vi "UHR-Fleezers Control (host) - 10.8MV_trial3.vi"() -> ()   [LabVIEW 2012]
uses:
  <vilib>/Utility/miscctls.llb/LVPoint32TypeDef.ctl
  <vilib>/Utility/miscctls.llb/LVMinMaxIncTypeDef.ctl
  <vilib>/userdefined/High Color/nirio_resource_hc.ctl
  <vilib>/Platform/TimedLoop/XDataNode/timing_clust.ctl
  <vilib>/Platform/TimedLoop/XDataNode/nitl_modes.ctl
  <vilib>/Platform/TimedLoop/XDataNode/wakeup.ctl
  <vilib>/FPGAPlugInAG/PCIe-7852R/niLvFpga_Open_PCIe-7852R.vi
  <vilib>/FPGAPlugInAG/PCIe-7852R/niLvFpga_Reset_PCIe-7852R.vi
  <vilib>/Utility/error.llb/Error Cluster From Error Code.vi
  <vilib>/rvi/errors/niLvFpgaAdjustHostInterfaceError.vi
  <vilib>/FPGAPlugInAG/PCIe-7852R/niLvFpga_Run_PCIe-7852R.vi
  <vilib>/Analysis/baseanly.llb/Mean (DBL).vi
  <vilib>/express/express analysis/Spectral/Block/exnSpectralBlock spectral measurements PSD poly.vi
  <vilib>/express/express analysis/Spectral/Block/exnSpectralBlock spectral measurements PSD WFM.vi
  <vilib>/Waveform/WDTOps.llb/WDT Append Waveforms DBL.vi
  <vilib>/FPGAPlugInAG/PCIe-7852R/niLvFpga_Abort_PCIe-7852R.vi
  <vilib>/FPGAPlugInAG/PCIe-7852R/niLvFpga_Close_PCIe-7852R.vi
  openfpgaref.8.6.ctl
  <vilib>/Platform/TimedLoop/XDataNode/XDataNode.xnode
  <vilib>/rvi/interface/nirviOpenFPGA/nirviOpenFPGA.xnode
  FPGA Bitfiles/UHR-FleezersInst_FPGATarget_UHR-FleezersCont_0F5B06C4.lvbitx
  UHR-Fleezers Control (fpga) - 10.3.vi
  <vilib>/rvi/interface/nirviMethod/nirviMethod.xnode
  <vilib>/rvi/interface/nirviReadWriteControl/nirviReadWriteControl.xnode
  <vilib>/express/express analysis/Spectral/XNode/ExpressSpectralMeasurementsBlockNode.xnode
  <vilib>/rvi/interface/nirviCloseFPGA/nirviCloseFPGA.xnode
  <vilib>/Analysis/NI_AALBase.lvlib
  <vilib>/Platform/TimedLoop/XDataNode/XDNodeRunTimeDep.lvlib
  <vilib>/vision/NI_Vision_Development_Module.lvlib
  NiFpgaLv.dll
  <vilib>/FPGAPlugInAG/PCIe-7852R/niLvFpga_ConfigureFifo_PCIe-7852R.vi
  <vilib>/rvi/errors/niLvFpgaMergeErrorWithErrorCode.vi
  <vilib>/FPGAPlugInAG/PCIe-7852R/niLvFpga_ReadFifo_PCIe-7852R.vi
panel:
  out "Location path":path=path "D:/UnifiedHighRes_VIs/Locations.txt"
  out "Location Matrix":string[][](array[string])=[["N.D.\r\n", "N.D.\r\n", "N.D.\r\n"], ["0.19233\r\n", "0.00156\r\n", "0.20615\r\n"], ["N.D.\r\n", "N.D.\r\n", "N.D.\r\n"], ["N.D.\r\n", "N.D.\r\n", "N.D.\r\n"]]
  in  "radius":i32=10 min=1 max=20
  in  "clear markers":bool
  in  "trap\nmarkers?":bool
  in  "Sample Channel Flow":bool
  in  "Pump 3 contents":string="Bottom: ADig beads" caption="contents"
  in  "Pump 1 contents":string="Top: DNA beads" caption="contents"
  in  "Scripts":T1(tab)
  in  "Take Stepping Data":bool
  in  "Got DNA bead":bool
  in  "Got ADig bead":bool
  in  "Cap 1 Flow ON":bool=TRUE
  in  "Move Cap. 1 (DNA Top)":bool
  in  "Cal/Data Acq. Spot":bool
  in  "Dump Beads":bool
  in  "Cap 1 T ON":bool=TRUE
  in  "Cap 1 Samp Flow ON":bool=TRUE
  in  "Offset 2 Set":dbl=2.0
  in  "Offset 1 Set":dbl=1.0
  in  "Cal @ (MHz)":dbl=20.0
  in  "W/ Offset 1":bool=TRUE
  in  "Offset 1 Start (MHz)":dbl=13.0
  in  "W/ Offset 2":bool
  in  "Offset 2 Start (MHz)":dbl=16.0
  in  "Pause at Closest Delta (s)":dbl
  in  "Move to Delta 2 (MHz)":dbl=41.0
  in  "Attempt Limit":dbl=30.0 caption="Limit"
  out "Attempts":dbl=1.0
  in  "Wait Before Save (s)":u32=1
  in  "Fish for Tether":bool
  in  "Closest Delta (MHz)":dbl=13.0 step=0.25
  in  "Stop F (pN)":dbl=10.0
  in  "Then...":string(combo)="2"
  in  "Move to Delta 1 (MHz)":dbl=15.0
  in  "Tether Alarm?":bool=TRUE
  out "Tether":bool
  in  "TA Cancel Save?":bool=TRUE
  in  "TA Green Off?":bool=TRUE
  in  "Raster Set Upon Tether":u32=1
  in  "Save at end (5, 6)":bool
  in  "N Steps":dbl=20.0
  in  "Step Size (nm)":dbl=0.34
  in  "Save ave factor":dbl=1.0
  in  "Dip Trap Delta 1 (MHz)":dbl=15.0
  in  "Move Trap Before?":bool
  in  "Save Data After?":bool
  in  "Green ON After?":bool
  in  "Dip Trap Delta 2 (MHz)":dbl=15.0
  in  "Move Trap After?":bool
  in  "Duration (s)":dbl=1.0
  in  "Dip for Protein":bool
  in  "APD to Watch":bool
  out "Duration (s)":dbl
  in  "Action":string(combo)="Yank"
  in  "Fl. Triggered...":bool
  in  "Fl. Delta Thresh. (kHz)":dbl=0.6
  out "Waiting":bool
  out "Fl. High":bool
  in  "N pts to average":u16=6
  in  "Yank Delay (s)":dbl=3.5
  in  "Yank to Delta Array (MHz)":dbl[](array[numeric])=[16.3, 15.85, 14.85]
  in  "N Array El":u8=3 min=1 step=1
  in  "Random Choice":bool=TRUE
  in  "Force Yank":bool
  in  "Force Reset":bool
  in  "Y change (mm)":dbl
  in  "Profile":bool
  out "Sigma/Mean 2":dbl=nan caption="Sigma/Mean" format="%#_2g"
  out "Rate sigma (Hz) 2":dbl caption="Sigma (Hz)" format="%0.2f"
  out "APD 2 Rate (Hz)":dbl format="%#_3p"
  out "Primary Video Display":T2(plugin-control)
  out "Waveform Graph":dbl[](graph) caption="APD Line Scan"
  in  "Inject Top":bool caption="Inject Pump 3"
  in  "Inject Bottom":bool caption="Inject Pump 1"
  out "Messages":string="7:59 AM\tUHR-Fleezers ready.\r"
  in  "APD Ave N":dbl=10.0
  out "Int. Time (s)":dbl=3.0
  in  "Stop All":bool=TRUE
  out "Sigma/Mean":dbl=nan format="%#_2g"
  out "Rate sigma (Hz)":dbl caption="Sigma (Hz)" format="%0.2f"
  in  "Tab Control 6":T3(tab)=enum."Imaging"
  in  "APD 2 Offset":dbl
  in  "APD 1 Offset":dbl
  out "RMS (Ang)":dbl=nan format="%_2g"
  in  "Bead Sep. Int. Time (s)":dbl=5.0 caption="Int. Time (s)"
  in  "Below (kHz)":dbl=0.5
  in  "Above (kHz)":dbl=2.0
  in  "Adjust Scale\nto Mean":bool
  in  "Rescale on Mean":bool
  in  "Offset (nm)":dbl
  out "Mean":dbl=nan caption="Mean (pN)" format="%#_3g"
  out "Force":waveform(dbl)[](graph)=[{"t0"=timestamp(12.90000000000001 s since 1904-01-01), "dt"=0.15, "Y"=[nan, nan], "attributes"=variant("NI_ChannelName"=variant(string "T1 X"))}, {"t0"=timestamp(12.90000000000001 s since 1904-01-01), "dt"=0.15, "Y"=[nan, nan], "attributes"=variant("NI_ChannelName"=variant(string "T2 X"))}]
  out "APD Chart":waveform(dbl)[](graph)=[{"t0"=timestamp(12.90000000000001 s since 1904-01-01), "dt"=0.02, "Y"=[0.0, 0.0, 0.0, 0.0, 0.0, 0.0, 0.0, 0.0, 0.0, 0.0, 0.0, 0.0, 0.0, 0.0, 0.0], "attributes"=variant("NI_ChannelName"=variant(string "APD 1"))}, {"t0"=timestamp(12.90000000000001 s since 1904-01-01), "dt"=0.02, "Y"=[0.0, 0.0, 0.0, 0.0, 0.0, 0.0, 0.0, 0.0, 0.0, 0.0, 0.0, 0.0, 0.0, 0.0, 0.0], "attributes"=variant("NI_ChannelName"=variant(string "APD 2"))}]
  in  "Calibration":u16(ring) items=["None", "Position", "Force"]
  out "T1 X":dbl=nan caption="T1 X (pN)" format="%0.2f"
  out "T2 X":dbl=nan caption="T2 X (pN)" format="%0.2f"
  out "Bead Separation":waveform(dbl)(graph)={"t0"=timestamp(12.90000000000001 s since 1904-01-01), "dt"=0.15, "Y"=[nan, nan], "attributes"=variant("NI_ChannelName"=variant(string "T1 X"))}
  in  "Amplitude (nm)":dbl=3.0
  out "Bead Mean (nm)":dbl=nan caption="Mean (nm)" format="%0.2f"
  out "Difference":dbl=nan caption="Difference (pN)" format="%.2g"
  in  "Take Detection Laser\nImage":bool
  out "APD 2":T2(plugin-control) caption="APD 2 (Cy5)"
  in  "Flip Green Filter":bool
  in  "Set X Only":bool
  in  "Set Y Only":bool
  out "APD 1":T2(plugin-control) caption="APD 1 (Cy3)"
  out "Detection Laser Y":T2(plugin-control)
  out "Pointer Y (V)":dbl format="%_3g"
  out "Pointer X (V)":dbl format="%_3g"
  in  "Set Confocal Spot (X-Y)":bool
  out "Detection Laser X":T2(plugin-control)
  out "Saved APD":dbl[][](graph) caption="Most Recent Time Trace"
  out "Trap Delta Graph":dbl[](graph) caption="Most Recent Time Trace"
  out "Save APD Deriv":dbl[][](graph) caption="Most Recent Time Trace"
  out "Delta Fl. 1":dbl
  out "Delta Fl. 2":dbl
  out "All Signals":waveform(dbl)[](graph)=[{"t0"=timestamp(12.90000000000001 s since 1904-01-01), "dt"=0.02, "Y"=[0.0, 0.0, 0.0, 0.0, 0.0, 0.0, 0.0, 0.0, 0.0, 0.0, 0.0, 0.0, 0.0, 0.0, 0.0], "attributes"=variant("NI_ChannelName"=variant(string "APD 1"))}, {"t0"=timestamp(12.90000000000001 s since 1904-01-01), "dt"=0.02, "Y"=[0.0, 0.0, 0.0, 0.0, 0.0, 0.0, 0.0, 0.0, 0.0, 0.0, 0.0, 0.0, 0.0, 0.0, 0.0], "attributes"=variant("NI_ChannelName"=variant(string "APD 2"))}, {"t0"=timestamp(12.90000000000001 s since 1904-01-01), "dt"=0.15, "Y"=[nan, nan], "attributes"=variant("NI_ChannelName"=variant(string "T1 Y"))}, {"t0"=timestamp(12.90000000000001 s since 1904-01-01), "dt"=0.15, "Y"=[nan, nan], "attributes"=variant("NI_ChannelName"=variant(string "T1 X"))}, {"t0"=timestamp(12.90000000000001 s since 1904-01-01), "dt"=0.15, "Y"=[-0.0004235663930173644, -0.0004722739341410556], "attributes"=variant("NI_ChannelName"=variant(string "T1 Sum"))}, {"t0"=timestamp(12.90000000000001 s since 1904-01-01), "dt"=0.15, "Y"=[nan, nan], "attributes"=variant("NI_ChannelName"=variant(string "T2 Y"))}, {"t0"=timestamp(12.90000000000001 s since 1904-01-01), "dt"=0.15, "Y"=[nan, nan], "attributes"=variant("NI_ChannelName"=variant(string "T2 X"))}, {"t0"=timestamp(12.90000000000001 s since 1904-01-01), "dt"=0.15, "Y"=[-0.0005883053071687949, -0.0006281319620349712], "attributes"=variant("NI_ChannelName"=variant(string "T2 Sum"))}, {"t0"=timestamp(12.90000000000001 s since 1904-01-01), "dt"=0.15, "Y"=[nan, nan], "attributes"=variant("NI_ChannelName"=variant(string "T1 FB X"))}, {"t0"=timestamp(12.90000000000001 s since 1904-01-01), "dt"=0.15, "Y"=[-0.0004680013428144157, -0.0005167699209570592], "attributes"=variant("NI_ChannelName"=variant(string "T2 FB Sum"))}, {"t0"=timestamp(12.90000000000001 s since 1904-01-01), "dt"=0.15, "Y"=[nan, nan], "attributes"=variant("NI_ChannelName"=variant(string "T2 FB X"))}, {"t0"=timestamp(12.90000000000001 s since 1904-01-01), "dt"=0.15, "Y"=[-0.0006226691488387671, -0.0006504715109714008], "attributes"=variant("NI_ChannelName"=variant(string "T2 FB Sum"))}, {"t0"=timestamp(12.90000000000001 s since 1904-01-01), "dt"=0.15, "Y"=[-0.0007901852473525123, -0.0008601641895809732], "attributes"=variant("NI_ChannelName"=variant(string "PSD Y"))}, {"t0"=timestamp(12.90000000000001 s since 1904-01-01), "dt"=0.15, "Y"=[0.00031556138798181086, 0.0002525101474044007], "attributes"=variant("NI_ChannelName"=variant(string "PSD X"))}, {"t0"=timestamp(12.90000000000001 s since 1904-01-01), "dt"=0.15, "Y"=[-0.00019678334910122974, -0.0002453993346964931], "attributes"=variant("NI_ChannelName"=variant(string "PSD Sum"))}]
  in  "Signals to Plot":i32(listbox)
  out "Trap Disp. Freq. (Hz)":dbl=6.666666666666667 caption="Freq. (Hz)" format="%#_6p"
  out "Display Period (s)":dbl=0.15 caption="Period (s)" format="%#_6p"
  in  "Trap Disp. Downsample":dbl=10000.0 caption="Downsample" max=20000.0
  in  "APD Disp. Scale":dbl=0.1 caption="Scale (Divide,\nfor above plot only)"
  in  "APD Disp. Downsample":dbl=2.0 caption="Integrate" min=1.0 max=30.0 step=1.0
  out "APD Display Freq. (Hz)":dbl=50.0 caption="Freq. (Hz)"
  out "APD Display Period (s)":dbl=0.02 caption="Period (s)"
  out "FFT 1":cluster{"f0":dbl, "df":dbl, "magnitude":dbl[]}[](graph)=[{"f0"=0.0, "df"=16.666666666666668, "magnitude"=[-331.1367572010275, -79.05506245821404, -86.61411242440559, -88.4728176091699, -90.3181253945935, -94.12566333707997, -92.52740723119955, -94.92192587982518, -99.60936585245742, -96.87568627870715, -94.02570383337763, -83.8058550151726, -97.57441397235512, -101.59968530846606, -101.523049255742, -103.35038532190343, -101.58594091014982, -102.96098031851216, -91.39759462745924, -103.75019963279499, -104.45030075054324, -103.04245334279298, -104.0720279134107, -106.06482372394834, -103.69131867828104, -104.40395035115309, -105.96420043276396, -107.6735556337804, -106.673030006608, -107.34889066208132, -108.05626565233933, -106.25659018850432, -105.29934513380842, -105.43096056709592, -108.3728498841465, -106.0555440144992, -105.78001282181421, -107.48741857324953, -108.67624970548897, -105.39976667156175, -105.91413119232612, -109.4222808198164, -107.0898971593174, -107.91164191890915, -108.26032038855709, -107.58332347164534, -108.23559688234297, -108.01271040303237, -107.66511723652701, -106.51901583170391, -109.27249501469946, -108.55647681594805, -107.93499259231463, -107.05068166453935, -109.13641475410455, -109.29679733781423, -108.19360835527803, -109.57747591546632, -109.58364591011674, -110.47061433372711, -109.8144340420426, -108.79067462293897, -107.54887553357234, -107.99559866705923, -108.85023923652685, -109.68733225238618, -108.51101278437793, -108.51620475114115, -108.22212402200637, -104.63726950302143, -110.2989919678048, -107.61796444414897, -108.68882962798736, -104.79193983043893, -103.59504263746938, -93.64633660288543, -101.9191640501395, -105.73717393151816, -108.92572458793902, -107.43962662800902, -107.79595323081325, -107.0923101993207, -108.17603277205289, -107.87074270713183, -109.20899066381877, -108.61832060412445, -109.10072003106593, -105.76480632823524, -108.60877649218978, -109.67541158970121, -110.2286232768028, -109.84952155309578, -109.33772024076384, -109.95251642394683, -110.14777282585466, -109.13825677905699, -110.05989365698167, -109.39359990189426, -110.56255614635295, -109.66477183197163, -108.9397158528824, -110.26529907650465, -109.20049464984628, -108.20183857013548, -109.09752250184418, -108.00440442238454, -108.35465963524055, -111.16774134451799, -110.34812550238405, -108.94506763426756, -108.72845542102493, -109.41512344014713, -112.44661664432377, -110.35437330889101, -111.32939440655925, -109.42989530434981, -110.98084669076195, -111.92160561143541, -108.57755551751093, -111.40042616180912, -110.15284955891853, -112.21455132279115, -111.40787773511747, -108.82949641635288, -110.13442122547907, -111.42229298204664, -112.06314940885191, -110.6015308813694, -109.51144097251623, -111.15989713761475, -110.25535755335385, -109.65868178057926, -110.51649885452997, -109.77194745285269, -108.4234206864394, -109.50892632093968, -109.46471287444389, -107.92241289271415, -109.72283805386196, -108.63426821579918, -110.37316681536255, -111.09713996884652, -110.32903619589223, -105.32012665515045, -107.36858557554393, -108.00382215905725, -110.06430686942338, -108.81666625979916, -110.01277074453823, -110.94194741225512, -109.65934609082873, -107.80979136006962, -112.81333866824724, -111.61474300955487, -109.83998277184975, -109.45953946904639, -109.79640584952526, -108.19172301667324, -109.28894656674316, -107.61471301278785, -108.83814006090513, -109.08866847726084, -108.20250571862371, -107.96222236861584, -107.03811197900873, -108.93533000393974, -107.74482548035408, -110.79811544577694, -111.1387476496877, -107.42970105883512, -109.18442281176472, -108.73546184641192, -108.71800246690864, -108.51945944378063, -108.06825856571285, -107.27210712368412, -108.12304695877637, -107.84933283677306, -109.73682373154998, -109.32284761503395, -109.31328817453769, -106.68762108642842, -109.79203616876461, -109.9020278896408, -110.27080024357275, -108.54152101558762, -111.00464391726017, -112.42244020766577, -110.82707315747889, -111.00344011890857, -109.90461839395674, -109.42877207451863, -109.73549298167016, -111.67494793393293, -108.85799077901427, -108.5348443278263, -109.803781083881, -108.30644755543659, -108.5079527456017, -111.2055351312823, -108.53089994340155, -108.01739789012176, -108.70360662855235, -107.95873456794631, -109.58297170693093, -108.9372401694271, -110.15921663527153, -109.22399119911955, -110.89883651739237, -108.92840112258382, -110.0545300523626, -109.05961065387005, -109.45831398589371, -108.61239387653227, -110.13001256174265, -108.80060224137931, -109.46327400696283, -108.0177965824709, -109.29727944627197, -110.3237255895986, -109.03258262543821, -110.97880178489321, -109.70034895077919, -111.16405638194153, -109.17324451464711, -109.65698250854277, -108.96750235822178, -112.00534231585624, -108.69274607723942, -108.98110446396657, -108.40723795464795, -111.44459094807324, -111.74799245277113, -111.1601960491512, -108.92048232753773, -110.30506377784799, -111.33145973979093, -110.91850998672503, -110.33684985776448, -108.90206518366908, -109.28458878227542, -108.98773986023751, -110.85813863075646, -109.00041591105906, -110.84543686681204, -109.84382395806176, -109.69722434763266, -108.50915601095721, -107.80829925826895, -110.59736107582401, -109.75377770317087, -109.3992084496136, -110.51151565846742, -112.49753959826434, -109.7299632589479, -109.54070743868353, -109.90314341132164, -111.05974202976806, -109.03766862152392, -109.46667095459878, -109.52800799036197, -111.3163121356807, -110.07817134522178, -108.69251657453547, -109.40472158898045, -109.71400709815576, -110.60534468715097, -109.46937396724682, -107.70342491418788, -109.86331122597839, -108.64971387994616, -110.90117371097081, -108.34928840565928, -110.04172889660904, -111.52979926554961, -110.34759300823305, -109.62712781837159, -109.24131154553284, -110.23196152450447, -108.68509612326807, -108.0246905483419, -106.61876139289784, -101.5519630114271, -80.57695480953835, -102.03744443354402, -107.1449217193017, -110.0695213407169, -106.61597783999268, -110.79221011808191, -109.58974545931426, -109.1149802216988, -109.20993813088597, -109.63768480465863, -110.10428394219181, -109.08445084271477, -108.83472375362581, -109.69508502050168, -108.05588796178941, -110.62586360101581, -109.95315261676905, -107.52208264977473, -108.80708007514875, -110.43484881098874, -110.45942171588936, -107.83804717866751, -109.98973910294193, -109.3496496054193, -108.425252911127, -110.94579264380809, -108.54181722177951, -108.67696070083541, -108.4150202151644, -109.24973583101504, -112.0454922608961, -111.29046597340738, -110.75018248960077, -109.38326363603683, -109.2033340336957, -109.45076170874889, -109.52878049853727, -109.32340869724774, -110.98123395128233, -110.75736340635505, -109.7218385823809, -107.97422606064993, -109.77313701758703, -110.95948744392717, -110.08996774172691, -108.51011830110778, -109.78063140243836, -110.65996628628228, -109.83684298615616, -110.33329049188029, -110.13755118968292, -110.3717925645783, -108.55302219178951, -106.86811628734195, -108.6302156589162, -108.75341391045045, -108.32589578384841, -108.70061474734084, -112.30742263527534, -109.16842570592085, -109.29767035534508, -108.87829025017463, -108.2255616391397, -108.4316108616088, -108.82995906929271, -110.40135575415563, -109.51623498946435, -109.79409808792403, -107.03832759632121, -108.36534528684132, -109.72010868372905, -107.90933028179892, -106.95643597294047, -111.29929166165778, -110.23001135794706, -108.98838015381585, -109.79115357104436, -108.18627479511115, -108.14988122174307, -109.12074063466532, -109.41904850488358, -111.40409873721113, -108.83156790193294, -108.77032248953847, -108.88363158686694, -108.47515048290681, -105.94172147874599, -109.38146940214403, -109.21277078848794, -108.11309390545507, -110.70840012427504, -109.5504457849329, -109.52330684534209, -110.06776026911132, -108.21949434182314, -111.21266686269992, -108.78581501170974, -108.43115799297222, -109.63260325780062, -109.84070220619535, -109.72041980780126, -110.29615941882527, -110.60316734262464, -108.79165446414692, -110.95840439895592, -109.64926233107009, -109.16526769544322, -108.65292362430982, -109.56113898129935, -109.85693046339026, -108.92316027325207, -109.79492493553914, -109.38157962945887, -110.24545136266825, -109.30031463492487, -109.0795429936869, -111.4091719525013, -108.63499083917162, -108.43863465339358, -109.23207864880891, -111.21947487191643, -109.24525201480154, -109.56842406077318, -109.46711940800672, -111.91389548262572, -108.15655736690546, -108.71882059966947, -111.26328503478568, -110.95027143873176, -108.4853106242357, -110.36902802777546, -109.9314203579182, -108.77686164101732, -108.71871020068312, -111.04829661168574, -109.95072655339462, -109.88221342875462, -109.53241732756136, -108.2625005404823, -108.00677030040697, -110.19659317581693, -108.93858924796267, -109.46817875483995, -110.78063992017232, -111.11066570318451, -110.78774336696706, -109.19199744617812, -108.54914256407436, -109.28414960420909, -110.64143585101183, -110.5855350821307, -109.47578632252726, -108.89705360836223, -109.89214013612292, -107.93271261027171, -109.32631601340563, -108.60274611341092, -109.40110159872573, -110.889237682208, -110.01391165813328, -109.99747108785071, -108.65542819213674, -110.37211847668736, -110.44656500845738, -110.8128133834973, -108.8909299260433, -110.19551227077532, -111.37647266643523, -110.83802189730321, -109.98519377913681, -110.52378970770522, -108.16970420057817, -110.70974729773344, -110.76836765494402, -110.26884275594577, -109.22041044268806, -109.87809744746195, -107.76823252107832, -109.12119474042969, -110.28066108731146, -108.55000033509207, -110.18152097767907, -110.73030521152278, -111.49470908029893, -110.2320929919509, -110.03370979233021, -109.79181668155233, -108.6673501209991, -109.86695766650877, -107.88926518046961, -110.95525003776572, -109.18130359755742, -110.42618009658618, -107.90341931158893, -111.44736855661769, -110.72634267386593, -109.29945988519303, -107.67889101961411, -108.81148059987765, -109.13375212757057, -109.8122873383549, -109.80176697684155, -109.96342275204768, -109.90406635707086, -108.75674342748256, -110.12362902701081, -109.82151095527837, -108.62543344241836, -110.09171852771195, -110.21434637862887, -109.97254504855631, -109.27043209093468, -111.35149588204125, -110.12399876776051, -111.65983675538546, -109.28788875768564, -110.86554069990251, -111.26990906470603, -108.60956517491746, -111.49613890850938, -111.79685722966795, -109.26269485364045, -110.38555615546439, -109.40641023162068, -110.966136593156, -108.78892524584494, -110.29340727375603, -111.44032043281035, -109.95212021173755, -109.79233511584334, -112.41184021118175, -109.73687851881148, -108.65493879781806, -110.76132988919045, -108.43230346094671, -110.32968175895853, -110.29890782023821, -108.77609076424456, -110.3298662333555, -109.47734504217333, -108.2677295732245, -109.21234363352882, -107.83278941978479, -108.85136784424789, -108.43241251530755, -109.76609391460555, -108.53204373005357, -110.9660641972934, -110.3152512161094, -110.72570499399905, -109.23877906286317, -111.72407743101837, -109.20311421918561, -108.06021800233717, -109.29288625761943, -108.78395253409145, -111.85250172876302, -108.78827588901797, -109.79775055719482, -109.12089297455859, -109.49896359356035, -110.34432647103819, -107.94700097960238, -109.30489238477631, -108.89170290869342, -108.82574563272509, -110.11024077194833, -107.37946433552314, -109.60167933458756, -107.80625057819019, -110.11489057210264, -107.35436859378505, -105.69819484613895, -109.11280625683739, -109.27770293057978, -107.7053735252589, -109.75022444894368, -109.3310543596577, -107.87683693707739, -108.19931495338068, -109.26462246191564, -106.71885779297867, -100.00018022217961, -92.54434511397295, -107.20472143807373, -107.39203415155283, -110.04461177268398, -108.48860496315312, -109.0057168110333, -108.37627790492552, -108.4108380728248, -109.65509454313073, -109.64243000632982, -97.04219069306761, -109.0928856629964, -107.9760697315632, -107.52611064047497, -108.87702814778996, -109.08437599027614, -110.70097118837974, -109.00969860961283, -110.38275386163214, -110.0699155421545, -106.91498895181175, -106.22178738309017, -109.36827866896039, -107.59953130968307, -109.19516217272808, -108.31502495393616, -109.384158926223, -107.11670654202719, -108.09436312738853, -110.14559230873704, -109.84997663447679, -107.83465335309926, -108.60947100624459, -108.9932479423645, -109.17174810371898, -108.79457339828916, -109.40909327982367, -109.6328723628302, -109.51081854476179, -107.63054408568418, -109.63728404010122, -108.51163794839918, -107.55002282725216, -108.97796212764939, -107.24648164623483, -112.21470452291085, -108.74294024554423, -109.62070777514892, -108.05768666239368, -109.8224946685739, -109.34575507446003, -108.53536952609525, -109.60789300457671, -107.56681538208278, -109.22777325016398, -108.79047910308894, -110.10332477250668, -108.00206387955672, -108.45604004720035, -109.00645795765472, -109.81039564269616, -108.92785144634745, -108.3978471520567, -107.94411095685999, -110.53486519304262, -108.8773780319227, -109.03345093296107, -107.30746693745031, -108.54277704832029, -108.77629108166091, -108.91111762599647, -107.74965195880401, -109.97375370738439, -109.76326492689246, -107.91717581777407, -109.0730556927617, -107.66804873204664, -110.40438871064791, -108.05794247751498, -108.80206615156494, -107.51329354700796, -108.83687012994949, -107.57713176895379, -107.94774159581414, -109.41894615439651, -107.10869425078764, -110.51480854078629, -108.92221367099775, -109.91358786461535, -110.1744263092835, -109.30795472883494, -107.91359710691006, -109.77888185049835, -109.52060975706438, -108.66686651982212, -108.71041801553639, -110.13619546359467, -108.87957097273856, -109.72150387215271, -109.00776068810654, -109.70251113927438, -110.75769213896399, -108.53234896741436, -109.69439526582246, -110.15412541604617, -108.25183374628219, -107.97402569656481, -110.34920156998648, -108.45106995186384, -108.82031145748209, -111.38690005057539, -107.01968459818563, -110.3044500039584, -110.8755481852125, -111.08915057663255, -107.94824988655199, -110.21669144934839, -109.90539774633154, -109.58985438756767, -110.12258796623348, -109.41689951612143, -109.31128210476795, -109.00258476567323, -109.11093063041056, -108.83347064311234, -108.32685287566952, -109.44770946560935, -108.40145063144861, -109.68448193892085, -108.76525439243828, -107.62837139034596, -107.39300298848994, -109.36993934990318, -109.2465218489418, -106.66307369796812, -110.15891092764934, -109.57151745419041, -108.92425698310808, -109.8036704717834, -108.79751146756549, -109.25926431818017, -108.46260574057584, -109.1967554647261, -110.63319560262356, -109.02343067385144, -111.22073171487528, -109.4731095097105, -109.69335000085164, -109.48782989577005, -107.95204227683271, -108.19468255763758, -111.36195112053247, -109.55696116543685, -110.3130767640534, -108.9621824253354, -109.99735074896789, -109.20198058456344, -108.12100614259485, -111.27227490807289, -110.09248554008288, -109.14395535060149, -110.80882692379708, -109.22632926901655, -108.64497210802793, -111.00030482190711, -111.1317849358033, -107.43140429257826, -107.9783302193555, -109.2639893652291, -108.97008485446163, -108.66556668859064, -108.12995785876932, -109.73001061107855, -108.09691302413727, -110.68391499215569, -112.78583642012705, -108.7093037763389, -110.67868795924797, -109.0190959349128, -108.36247198231372, -109.82829353258869, -108.24916379311045, -109.84154533905823, -108.55470160833775, -109.75438989348815, -108.82865632118325, -107.63622268162582, -111.00943492886312, -110.81824358463759, -109.46028423652966, -107.52479398900992, -108.99087806823736, -109.94494831750349, -110.26788355564504, -109.8954055022304, -106.9478122391182, -108.91705388158901, -107.76095584490312, -109.28456723055147, -109.7982307261767, -108.98552661346622, -109.98937979783426, -110.57907422426224, -108.68113463944836, -108.06257240208589, -110.0707224529617, -109.19515280354733, -109.35868842818849, -110.37311467065695, -109.0404734478992, -108.16686395270187, -108.61859220485148, -109.19986437876149, -108.19707189725302, -110.06564239663074, -108.87850403465154, -110.63824157544798, -107.36918104067212, -108.7008736325543, -110.9359398265406, -111.08529123080929, -108.44209934821818, -109.79529621208783, -108.38917887958179, -108.169117639508, -109.24332926356216, -110.50584058811704, -109.63592524002665, -109.32261039377495, -109.16720880524552, -109.3084314664462, -109.5812223978583, -107.70213196487856, -108.0557884982431, -110.67058020007828, -111.68459781023608, -109.66270627185824, -110.52536245663693, -109.70208409132103, -108.78645420809342, -109.23122088059863, -109.24601474121832, -111.25604763816514, -109.50225851581177, -107.32434217163818, -109.28548556764925, -107.59972621660836, -110.46928774723048, -109.25950101547609, -110.32016453935465, -107.78482761561703, -107.89462895091089, -107.51366154391481, -108.08036891159172, -109.53371809947035, -101.2452927166745, -109.32763325689056, -107.52166868423687, -109.89648659445174, -109.11350200980485, -109.81336712738089, -110.02799517445062, -108.02767143538516, -107.97850220501483, -109.50772934896838, -109.31069875721964, -108.49991657749598, -105.60880911233095, -109.79128597340213, -106.91084537903113, -107.84880087118997, -109.63628170511824, -109.03203967193224, -110.64186113413658, -110.98027990365594, -112.33841002907062, -111.01793075565425, -108.58025797022215, -110.4259296883756, -110.38643255981424, -108.93051671115133, -110.97544177116494, -108.63883100482677, -108.37581711765226, -108.90240163126536, -107.94688047875466, -109.9482937437732, -110.09097112364414, -110.09805032265376, -111.44307114024532, -109.15483789122554, -110.9713708217832, -107.8548737634672, -111.41418477109195, -109.45699779859628, -97.03595099331734, -109.16746744169623, -109.66209204485918, -112.57048704774604, -109.73989735035725, -108.16252575067017, -110.7546980664636, -108.91536673403449, -109.20509151422344, -111.0260632167785, -109.62924582406518, -110.45466277291722, -110.2973970018937, -109.67550222925419, -108.84481022020094, -107.23686414357573, -111.79004633370906, -109.85453094194085, -109.45617270081004, -110.73920606732504, -108.90879956851099, -109.67774425528265, -109.4745715721361, -110.18080454693559, -109.26079184315502, -109.41692499885505, -109.02240975088358, -107.80833423058168, -109.32657361431549, -107.87138278655101, -110.910364670719, -109.70067156846706, -108.55301754282077, -109.4243252157005, -109.77567725161107, -107.83737232063925, -110.36509412773016, -109.6371048811367, -109.49430894422814, -108.55509251499753, -108.03996302911446, -110.4385715838736, -110.08864436068788, -109.48922484379962, -109.90865554258562, -109.7491963238264, -110.04796094537969, -107.413043439116, -108.54229076126079, -108.2522516728666, -109.75464941327974, -110.26795832300996, -109.28073673851144, -108.62990200974927, -109.89408067552287, -109.09160284731726, -109.90740624925795, -109.92534708896517, -109.79578862362752, -109.97278346890566, -107.80679350393824, -112.81728446281548, -108.09689504419987, -109.89549991422173, -108.43930976031248, -109.95153099843282, -108.18277483720716, -111.89607792605433, -109.52567003805, -109.17125106979698, -109.64300739407085, -108.21045178846524, -109.64036472149706, -109.02324448538845, -109.039163008889, -110.41006510134076, -109.50289952116489, -110.4732620447796, -110.08777181504614, -110.15589511434341, -109.55705089158471, -109.2547682932589, -110.86823885471617, -109.96330502176939, -109.85995369810554, -110.63211290903473, -112.08007783432191, -110.24725218052279, -107.62861148917592, -110.08691795849435, -108.89793794632287, -111.07702220466341, -109.46946126482341, -109.19747345337464, -110.70018609416007, -109.66366205691908, -110.78032312133551, -108.05724200456513, -108.195661625627, -110.90724508408255, -110.08307674771669, -110.76863516643007, -110.46620425061583, -109.16986788877276, -109.61921294239114, -108.51159432329543, -109.96308336765689, -107.38178944242856, -111.95930944846394, -109.3329826827624, -109.59119636368249, -108.83148571828912, -110.46194288788257, -105.87694286145472, -107.985886302892, -109.2975019660806, -111.05138725716857, -109.60005889204612, -110.92871351729086, -110.73480546964537, -108.41587420326718, -109.84275465824477, -108.8249071047676, -107.65358887817105, -108.3254150042995, -111.47362100321767, -112.7287536850025, -108.8217125660507, -109.50232320231771, -110.29587061625348, -109.30644535112089, -107.69178032077258, -110.84522325672016, -109.3735891463141, -109.12506388923123, -109.65582307934665, -111.11427272192576, -112.19827973435466, -109.11306367925813, -108.19203577968261, -107.89831568266465, -108.85805249169313, -109.51100049661844, -111.71546684086955, -109.53880495724334, -107.07739286222231, -110.66836728754211, -111.5415170557177, -110.16051267940297, -110.6107546662698, -111.36389129556191, -107.77888179117923, -110.34160392509817, -109.61287125994414, -110.23791773883013, -111.00669159903549, -110.97165069538953, -109.43965413392434, -110.6813161690388, -110.31441293654314, -111.96129906273796, -108.15998218707462, -110.08095912053633, -109.41084567452768, -109.28774416263552, -110.80159950384204, -110.41956747809755, -108.85005186267244, -107.9069227847757, -108.84249369063123, -109.92569208845894, -109.34109797584448, -109.41334788055491, -108.76462023086997, -108.22069272136177, -107.0786679601274, -108.30206755098202, -108.57613406368954, -110.83330887636482, -111.93966942736989, -109.76373713473264, -108.25782074884941, -108.16490627215555, -109.93351470267982, -110.75525684428368, -108.22814762283093, -109.73442331991602, -107.53145627482685, -108.27195221226805, -110.33032779278457, -109.48951857415828, -108.12599093700939, -107.97627415508097, -108.81426859968796, -111.21764717894752, -109.80856212352333, -110.92658779118501, -109.71551885834796, -110.38682741010847, -108.87671328341361, -109.68368600774755, -108.35359806351899, -111.7519400010676, -109.89407081573103, -108.24301180922755, -110.00646944788126, -108.6685299083706, -107.52856885980722, -111.7622363038509, -111.0025144494897, -108.64719599357296, -110.62968467177518, -108.821509935539, -107.94915453463719, -111.53070432277694, -109.87282048586256, -110.71167589371663, -109.79225006081626, -109.96203471712074, -110.29921092232489, -110.10644439440416, -111.28815007382043, -111.19165661703703, -108.46024117100558, -110.22528296512183, -110.32184972386672, -110.05120383416072, -109.78792549362107, -109.00355659956696, -108.85989369286315, -113.00899556732638, -110.91756826567867, -111.25016866167897, -111.84225040552181, -110.54451635944174, -110.72722829912917, -109.60759702177283, -110.49362602516815, -108.74419542915284, -110.3379671069179, -109.66259088220754, -110.45956400953156, -109.13956157147233, -109.27130155486806, -110.83015602667983, -109.17970724944131, -109.09662765889193, -108.0447366108107, -108.9536269357457, -110.35663108940085, -108.73418835472056, -113.42965806805827, -111.81270536656905, -110.06155590173537, -108.76582224646269, -106.7488061675813, -108.5700320158723, -111.11038264410035, -110.41435767488723, -109.12763443489911, -109.30517580756394, -111.61251165371237, -109.8116632664339, -109.36845864976851, -109.00390009629231, -110.54359197165573, -109.52629258465976, -110.75932197632896, -109.50903215359567, -107.42652056246085, -107.81146496533543, -103.22224383145215, -108.53803076819163, -109.78623360072066, -109.66306634612869, -110.80245829141279, -111.87835085452016, -102.27372781471168, -111.27763038431458, -108.45838423437681, -108.79077917058028, -109.31951755762685, -110.05415097017186, -109.5535934823387, -111.62732254641111, -110.73478247119641, -109.9468722686683, -110.39698367573979, -109.30612942398305, -109.7578384694043, -109.34817295524313, -105.56944757301993, -110.1940418750125, -109.27076023513962, -111.03491935225027, -112.2980497521063, -110.65725497955563, -109.0567530102422, -110.31700596563523, -109.64508026365678, -109.6190471404421, -110.52566833759428, -109.68595899227789, -109.7431160985074, -110.4798230300751, -109.45506977604765, -110.69504157940786, -110.63067849573177, -108.06456949500138, -107.99354148885966, -108.11349194720599, -109.15944121207349, -110.61766925164031, -110.14145801314527, -110.67420842201165, -111.91532881806512, -112.15901550030345, -109.94774413630104, -109.2819568305201, -110.94623189179737, -110.17685430287735, -110.39082916961016, -109.53953238698966, -110.76940623620611, -109.89327922318515, -109.10275695043765, -110.21445972656734, -110.58968777252528, -110.57016757660259, -109.59208496373341, -109.07946946465374, -109.10762003745964, -110.36892993974607, -109.81864495218393, -112.12972189864566, -109.26185849434863, -111.56305819991357, -111.36019621828058, -110.3397604159226, -109.58675612753163, -110.58041217474447, -106.34739062044932, -108.6722699609389, -110.03906060709869, -109.16794717548382, -109.65012481802809, -109.35377624077988, -110.51889143862303, -110.03397458059777, -110.7981307056636, -110.56653507062292, -107.61367005067231, -109.99279736988825, -111.79875182878175, -108.60382315996031, -109.71381533228038, -108.60388131505613, -107.0933685540362, -107.86037690830757, -108.40980028847238, -108.83869602763895, -110.76921375395764, -109.96766364716046, -110.8256171465781, -110.13805084291067, -108.5349140035878, -110.57158437465219, -110.8920694413417, -108.71646695477324, -108.33274238445665, -108.96152108305608, -111.03750932994224, -109.48915027983756, -110.29725207211165, -110.79527247268442, -109.47969936716117, -109.79306701834035, -110.16840035577498, -110.29840230783668, -109.15306387075587, -110.72651274964761, -109.08881658764956, -110.8349724030761, -110.64653625576447, -111.40392562616867, -109.94581588927414, -108.85136340231294, -109.77228546607624, -111.48297395390018, -109.7334001251941, -109.30537415590783, -109.63937411233408, -109.69785848648013, -109.3523781030017, -112.04667421182404, -111.56311816195343, -108.18548447362308, -110.63388993686104, -111.39768634137992, -109.87157345395542, -108.6734208287271, -109.46213300216168, -111.75774769437145, -110.10245994173216, -109.52385139033495, -110.96513097775451, -111.8709319163154, -111.54948269614047, -110.29760900080463, -108.52168175904663, -111.09033925738258, -111.14752744054172, -108.83074523709202, -109.05704141259113, -111.74377805749482, -109.57200906899736, -108.84121318623825, -110.86657990204343, -109.54363603755047, -110.89448416316372, -109.58965570570145, -110.21012263847972, -110.4063470702923, -109.5021950342969, -110.33648801598177, -110.90551031296536, -109.69205870504638, -109.8648503154861, -110.28183391384131, -109.65970942950766, -108.43615680946908, -111.11790511866548, -110.89043476451553, -113.64898442872548, -113.08004494963895, -110.81525412051718, -113.91009875719509, -110.95802128672312, -110.40944585634135, -110.33464695414992, -109.98984645778987, -110.18795067005652, -110.62364351231234, -110.44029833291248, -109.01598585569788, -110.95430216511514, -109.77987141110621, -108.54452361812068, -111.41780266439777, -110.47172771858405, -109.06084635984516, -109.30794593246578, -108.8764083815745, -108.18222749506985, -110.31330487887435, -109.04176821738014, -108.8558386035048, -109.47888284507395, -110.01459604573937, -110.48596659065309, -112.6781342298378, -109.85522803775775, -109.0569534499285, -109.08991286548698, -110.89485727880403, -109.18715778948663, -111.50381433568144, -111.3545424730884, -110.07710926239977, -111.99977850157067, -109.47444853853723, -109.81605328527645, -110.74995213151195, -112.56834665925544, -108.52052472391404, -110.89121213995557, -112.02004142355113, -108.66413739656008, -111.10053848695652, -110.41241079991636, -111.80152991764473, -110.21746151515111, -110.63265128607344, -109.483042128511, -112.78639954059729, -109.47114195846122, -109.23309637902875, -108.97133643967169, -110.08909147812822, -111.01105271457081, -111.18602432128249, -110.04633990216801, -109.53453538673071, -108.81939452082017, -111.13486114285661, -111.65877073200598, -111.63763706753498, -112.14107810664572, -113.6231865196724, -109.31743865878806, -109.18551713085722, -108.74951309653638, -109.28206426212142, -112.36687029711229, -110.10933061193728, -111.29501093502684, -108.19021080564794, -109.34497312126749, -110.37228033937312, -108.63277512903049, -110.61033993911002, -111.2975761598062, -111.49780004751436, -109.91019436685814, -109.32789992989028, -111.4482538110117, -110.1538439123475, -110.66347034043578, -110.05055133068794, -108.53002033538341, -111.7522199783972, -113.49108651193104, -108.03793940563418, -110.07108694011555, -110.83958739865201, -109.62805629409038, -112.69637731014087, -109.57996950503268, -110.104850643722, -108.83376203949506, -108.69400304840181, -110.59434352922563, -110.69121011800921, -110.18694553784364, -111.90598571547098, -110.30230802494223, -109.66810649416752, -112.6017099000434, -111.00296745333219, -110.64462650261785, -111.4775358707403, -111.98753241268494, -112.26574909791167, -112.04796822399412, -110.65853064447325, -109.6623218025264, -109.40559579075378, -110.42174451813142, -109.18991987957241, -111.02050178263048, -112.77950487440032, -110.42443751566815, -111.35440372400903, -108.5263524245987, -105.07498063939795, -107.15444425741984, -110.4508720018025, -110.25163264819463, -111.1383261104107, -109.91171620173931, -110.52200560606038, -110.5299174299573, -109.34628087255733, -110.26101817411786, -109.65071853372183, -109.66953335961068, -110.83590602054682, -110.980546313788, -109.4110066989163, -111.47223607390256, -110.00281523859483, -109.4088722967626, -109.00401922839337, -109.59655302543185, -109.7359970854586, -111.46016206343049, -110.23478747568004, -109.29441275295858, -109.82941912510167, -110.43088525283673, -108.21649744751299, -108.70220592702613, -105.2334473604296, -110.60620657984927, -107.97533820921146, -110.7664079806058, -110.56406610911355, -111.76465470250328, -108.84172809688911, -111.03661078143631, -109.85351980370237, -110.70091167176791, -109.52380717508088, -108.4356492672842, -112.25498760397127, -110.69648730540193, -110.36748838594507, -109.99090797924349, -111.2678642544111, -110.42541694325627, -111.4575545259775, -109.3211175669008, -112.7465573314208, -109.56208667784249, -111.59733497772172, -109.42295730962105, -108.55804089331346, -108.71397903286748, -110.09188290952392, -108.90810063278326, -110.31333217069538, -109.69794714542728, -109.06210020835357, -112.42465112160288, -111.74630553904855, -109.99304310093493, -108.93867687355595, -113.1669287525049, -109.09193568851137, -109.27500368450697, -108.99643325722404, -110.53962759110647, -111.2052088429852, -110.05855563908841, -110.30763723153481, -110.03411001268613, -109.6161415052669, -110.6304714466923, -110.17116005754627, -109.0753171640551, -110.92564270851628, -109.60831770517053, -110.25913363817017, -107.76644895378317, -109.2619309023068, -107.64198246311884, -107.37056168314048, -107.31978563121643, -107.68171928702894, -104.57515288104209, -104.75187637758803, -105.27246893266054, -106.96524396060869, -105.93920355631757, -103.66449995825586, -104.08476660009461, -104.53081578265315, -103.0148493379086, -106.74751670818362, -104.92309629919443, -103.98320340724693, -104.81633219413234, -105.77996356028235, -107.12559309216644, -107.28196039053535, -108.84583578337953, -109.4494696919565, -109.15525441177898, -109.7634811359225, -110.79433338587495, -108.44440079452527, -108.79597700117748, -109.98590735173822, -110.72144284267539, -109.30550753718086, -109.70072152916897, -109.65801130162137, -109.65949265997646, -109.82238573025273, -110.30669821947491, -109.83394128869384, -108.90433312205332, -110.664046708231, -110.39926453734134, -110.37725911098757, -112.12508639032839, -110.26795666332589, -108.98741993218054, -107.76168841100478, -109.82334992872889, -110.83516363498563, -112.60649745671253, -111.1960726449926, -111.03919163866381, -112.05129034965563, -108.83187987662883, -109.57240688505179, -109.32857861150738, -109.54934849013647, -108.29359879300195, -111.5179112931669, -109.52702486426027, -109.95429980789645, -110.7011078611564, -109.43204524997455, -105.56031249677113, -107.70609254346495, -108.78303653454363, -108.11457060956113, -110.44215460317537, -110.78267897406572, -110.33119812901934, -109.34449539666907, -108.82636558484161, -107.1834151347969, -108.83808254322192, -108.2542825327446, -108.80298057862501, -107.59922121598055, -108.9131916496929, -109.51519107961856, -107.7704986323755, -108.79678029009878, -111.13791068210752, -110.402746275919, -111.31702623823912, -108.49812727557243, -110.63723264798182, -109.32890666586829, -110.29721723278237, -111.66560929315017, -111.04227698307153, -111.36927505376269, -112.5203298417673, -109.93967930487354, -110.14533835678606, -110.3868348991775, -110.85413569165249, -108.44519725537315, -107.93391978795047, -109.82778679299085, -109.79311153223738, -109.25261055399044, -111.47738679135526, -111.11775495397512, -108.65898844492045, -110.26505495390529, -111.02017977446526, -110.34817965403467, -107.55161094495372, -110.21667403085983, -112.43970497917284, -110.70535338255132, -110.79438078890512, -109.81809822502822, -108.99167960596515, -106.5556893069368, -97.51736665041192, -105.29926513345109, -108.72453297392224, -108.23203912463346, -109.50324111400698, -110.9939986929772, -108.05367524487318, -108.37339392211176, -109.8553291283933, -110.46179639493138, -112.48795697163695, -111.88145079973545, -110.8678969738583, -110.62677605624849, -111.83824818603244, -109.76798658735359, -109.6654742351465, -112.58543522753767, -110.3406716250781, -109.55013159400883, -108.00481229232405, -109.90793236599207, -111.28597960985334, -110.54144527494444, -110.14704702870655, -111.2652554338908, -110.97520848958668, -108.63647576273343, -110.52472680617548, -113.16137826273847, -109.62457037485827, -109.53869420402964, -110.71399284283449, -108.55435337782664, -108.09492728294455, -112.2373886856363, -110.3693019226993, -111.65116752865308, -111.3223986412311, -109.67734725401074, -111.36420709226297, -109.14293108556625, -110.5982939020188, -110.29596476096043, -112.69847120697035, -108.39052787054206, -109.06205229490357, -110.00045399262885, -110.71775009467346, -110.69530760167493, -112.54144940754935, -109.55755373438097, -107.88943697845929, -109.98578587243783, -110.14202980613851, -110.80051915904802, -109.11327182471621, -109.50637030500913, -109.77023677605327, -109.98552825925917, -110.40235854896, -109.37603004890141, -111.36989177909379, -110.8399811877331, -109.30394670937987, -112.2769814990538, -109.10893172594731, -109.17733972841754, -108.35968166480572, -112.64492569586005, -110.13779257328873, -110.64439690778532, -108.45446935516622, -108.97325006911116, -110.54637968933774, -110.66412364132371, -111.38627695224784, -109.8942998516069, -110.36392017322382, -109.92355133054227, -109.61886697310419, -109.71969465343778, -109.85627196259388, -112.1407808286419, -111.1013489416651, -110.70428953307596, -109.3454280179969, -110.22984684615578, -109.53826801613613, -107.83673208330934, -108.72742563398342, -109.5745872123195, -108.83031823548816, -110.89059911076627, -109.87842545384129, -109.21980161063786, -109.07140273870678, -109.04628915564135, -108.79255665097845, -105.20875397856382, -110.0838008881032, -109.68293832806683, -111.24644641302518, -110.01257579497496, -110.99281477454484, -108.99296184719546, -110.96495665514604, -110.70404386182749, -108.25078498739035, -100.77667501455139, -107.61479263900088, -110.06600976399395, -110.02035637581871, -111.45524052052504, -109.975541184397, -111.07333860975358, -108.4808974233161, -109.59513524582242, -110.74711589861774, -109.50005300854993, -105.23071652566294, -111.81094849223531, -109.0168079712372, -111.89029991620679, -109.90672274216391, -109.30959446424889, -108.23718655264584, -110.10868108588909, -109.21139771899594, -110.33333323577992, -110.25792318324204, -110.67825932924109, -112.33148517950511, -108.9724848367048, -110.78371843797613, -111.40913868573313, -110.2930522718577, -111.9538408094371, -108.63639312641844, -112.4462941079034, -110.40266356498321, -108.66617580940074, -109.44306834729083, -111.08962916641603, -110.52132608161017, -110.53757698855654, -111.5587344449704, -109.77722315102946, -110.40060629757771, -109.45395807961631, -108.77558572395142, -109.0151938598724, -109.80739619986889, -108.9332873172888, -112.49933978358132, -111.28667321897437, -110.40629082858706, -109.9829216820938, -108.85102919990373, -110.84179127037925, -110.27309817549309, -109.88857884367955, -112.24517967927224, -110.23377125710859, -111.26951227953063, -110.09782138347559, -109.77508406986834, -110.55359722398646, -110.09534729906368, -109.96333904888587, -110.29372855476366, -111.36651812163072, -109.97141184588116, -110.16701683369045, -112.8562627359291, -110.66651146857079, -108.78873821095968, -108.59208174618087, -110.31784275318834, -109.43177042415276, -112.80272887161644, -111.79874205007107, -111.08216899537892, -110.73699224045636, -111.04738767291953, -110.43395896705012, -111.62106163510778, -111.32599933330843, -110.29360981749807, -109.66562228449096, -109.21316193790335, -110.06363162177448, -110.54480468587292, -109.31791670875509, -112.65386492377107, -109.91857609999171, -110.57233605624137, -110.7597333064856, -111.49767138733276, -109.36548654843229, -112.34145274183716, -110.52831153822652, -111.55802243871352, -111.81399803046556, -110.17680125962372, -111.23811621944807, -110.48042049674514, -112.43786993562033, -109.56507357271987, -110.67030752598993, -110.86377249100713, -109.06001892813467, -111.37023727930494, -109.52881096984436, -112.95107295160436, -110.49467818026214, -109.29804210589607, -109.89270706931751, -109.46354468058833, -112.10350702955014, -111.06083529077077, -110.49996587015904, -111.1617248913634, -108.84725633199014, -111.42852695852422, -110.01433866707184, -109.11616968390972, -110.76961079765468, -111.80403513904453, -109.84442686379181, -109.65447921666167, -111.3378640555306, -110.8882647652338, -112.58014202075226, -109.67128881545659, -111.73429980763389, -110.82258070774773, -110.71895931098041, -112.5117489008152, -109.16182299471309, -109.71651258790612, -109.7770618808562, -111.94294809571427, -111.1629115541574, -109.57489224865171, -109.8402445779754, -111.17931450307283, -110.09045865447595, -109.23658206733491, -112.54929616847242, -110.5150381158864, -111.32296447909377, -111.64472156295191, -111.65832771066007, -111.03359562742956, -110.85303206770837, -110.80655337650862, -109.3712696310075, -110.57313454785879, -111.18525355670417, -111.67423695430561, -112.00829831274282, -111.08915434609605, -110.3298290221436, -108.68552957386795, -112.11377370993225, -110.80288297661977, -110.33640536217185, -109.5907971201988, -107.9195263775506, -108.50223113159429, -111.91191347156142, -110.29585599512956, -109.50902788911351, -110.76819145749467, -108.86899533416589, -112.09963049260891, -110.13374376572433, -110.15881393584463, -110.87392107947531, -109.18658540731009, -109.72734703956934, -110.18732487568724, -108.76554115185057, -109.94122289815374, -110.39583285609643, -111.09540935727229, -110.6618176357367, -111.6281345666718, -109.69686483639367, -110.31633402076315, -110.61246951748903, -111.73300235294965, -111.34221378834899, -109.46708370903485, -110.70412671997354, -110.7007891485379, -110.31685483435038, -111.03016917417074, -110.94517365625376, -109.46580797053619, -111.20935248224806, -109.20661126636224, -109.50147037097533, -110.14241781654353, -109.8510950344643, -111.3794198224028, -111.28966889207122, -110.43347441663424, -109.86759980279523, -111.92101892013198, -109.31594011390644, -112.92253433794441, -110.74000829597605, -110.3690783911604, -111.9386136764295, -111.04196305034188, -110.41800427558245, -110.94287511448232, -111.66035388807579, -107.53723747644062, -110.68014818358719, -111.86628806511304, -110.12097497430523, -109.69880468221378, -111.4312783987915, -109.18240866486639, -111.45649839248873, -110.1242345454651, -113.75911576151633, -112.71747598882953, -110.9614554157337, -110.92294419716129, -110.87229098694876, -111.09943759113875, -109.48107247947176, -108.62783006742795, -110.8108025857779, -111.63342408317932, -112.0221522906341, -109.96411229549527, -111.29821085030613, -110.04566676239914, -108.41674583097112, -107.50256474992416, -108.68086611003493, -110.3738906060137, -108.86763212826641, -109.81681043446049, -111.04539822346567, -111.73290882980949, -109.75238769150758, -110.55268275367449, -110.48423701377924, -112.1116140908134, -109.53952175199518, -108.538611608547, -111.3788321484912, -110.36378736224961, -110.37712171023523, -109.82150687920334, -109.17046632238393, -105.1169578108227, -110.84067642540583, -112.91626789016587, -111.32030958133453, -108.93375913686056, -112.44450956563915, -111.1596840012794, -110.17380444915341, -109.634859036508, -110.68819277718731, -110.0648098825346, -108.87385575091399, -111.99676414571755, -111.32585405719519, -110.59892045991457, -110.32589048340424, -111.1172696292077, -109.79946399891651, -110.10030723919304, -110.71841081343656, -112.23013150012054, -108.94400401141407, -109.71044551701596, -111.77560214164039, -109.68779520039777, -110.96119601299907, -113.66477058855787, -110.17794649102234, -110.30159876509862, -110.11953836266514]}, ...(2 in all)]
  out "FFT 2":cluster{"f0":dbl, "df":dbl, "magnitude":dbl[]}[](graph)=[{"f0"=0.0, "df"=16.666666666666668, "magnitude"=[-324.19011195451765, -78.1272953812706, -85.85545438627958, -89.30587144190069, -92.90590394398903, -93.63083388385274, -91.8644929119412, -95.26924857401164, -97.0710469181336, -98.01148078956652, -99.33043660296804, -95.58776817681839, -99.9570097527269, -101.45494093095093, -101.51838334751548, -101.00386616525799, -103.01963069818913, -103.20223925731209, -103.53783076500916, -103.48065647812659, -103.97797518531912, -104.58942778240602, -104.46991277190502, -104.59813972158683, -104.56685024229951, -104.69893799348945, -105.05669000016238, -106.17061117835001, -106.43303821862656, -107.39468286383597, -106.2899368267905, -105.7863846168199, -105.17170638885071, -104.53818172761852, -106.70340956723133, -106.55444321137247, -106.67654843051936, -107.79888413750199, -107.86424326005849, -106.09722609215336, -107.71648639013972, -107.79500725395155, -106.17330953637067, -105.43663624517525, -108.04970689199158, -109.92106271611999, -106.2505251183406, -110.60221373795562, -107.11377887451098, -108.4126937286195, -108.37794745021417, -113.22457316369011, -106.38281814065472, -107.55385617652075, -108.93026538982782, -106.19334142366085, -108.90462602264525, -107.63084712174981, -109.12192537022624, -107.90627042480016, -109.44472079190832, -108.91731458372392, -105.74102972706788, -105.74407510394178, -107.5989477192235, -106.2838630137392, -107.46190542725505, -107.38881299750702, -109.08024783239452, -104.97871836903269, -106.65424712290651, -107.04966019632134, -106.16202578092883, -102.98374199247179, -99.1568704142098, -87.07383781389657, -96.41471411313154, -102.65176579899618, -107.65674867775193, -102.85397890306213, -107.58658613411464, -104.79044898833125, -106.65282019869865, -108.65027966345534, -109.46169054950127, -108.69969979291741, -110.4048706652988, -108.81020193837274, -109.42808902484134, -108.85398463561398, -108.3849716744813, -109.1844457168716, -109.32787859535676, -111.01992124870878, -106.64843449415699, -108.9926343573667, -111.59837822080355, -110.57121677672183, -111.17280164669164, -110.68901970586144, -111.69013245592781, -109.90200577018311, -109.3554172126163, -110.7515368822992, -109.2863324212524, -109.66209701262974, -108.50795548698007, -110.58126481096504, -112.36093896766921, -109.78612141282203, -108.85120530917233, -109.91424431080952, -109.84698632196245, -110.93960894966105, -109.77214706089354, -110.30762971422381, -108.77791302937449, -110.79522659679036, -108.47242514643455, -111.20629758187835, -109.05996769621125, -111.13574821570619, -107.79388178889101, -111.5768481279296, -110.52058839597171, -111.58729762739313, -108.99000864386126, -111.6585121505227, -110.50715371958135, -108.87151956974363, -110.30486244367107, -108.32392040018144, -108.1769507919999, -110.43198471512189, -109.81454097966842, -110.26717009815644, -110.82924135076777, -110.34103661156989, -110.0692667126265, -109.34555682020833, -109.1694484721415, -109.9940980324044, -110.81940616215803, -108.21162003366862, -107.97087538330561, -107.55312461506225, -110.60339321606872, -110.09004629292225, -109.05860430198882, -113.1412749514818, -109.81628200948371, -108.62343219429849, -109.48172424209761, -110.85978755785311, -109.47778611557064, -108.81728552967951, -107.47864241666747, -107.61735128422292, -109.62511618983821, -110.32417726356636, -108.24287897478176, -108.60460879530194, -110.2181558494026, -107.95550802888957, -110.80234484950323, -111.09955733353904, -109.43923052503506, -108.98949130235951, -110.05778199870154, -110.36224432927585, -108.13523430027999, -110.681114579241, -110.49106131529867, -108.73493328004297, -110.07663907252234, -109.9968931372618, -112.10715231091008, -108.80994125105168, -111.63774865669372, -111.54355694032755, -111.64024217585788, -109.34986300492378, -108.88053713185408, -111.14370830146245, -111.17327416167232, -110.36311492990576, -109.99414559884396, -112.96912007380595, -111.43191437097785, -111.71327312809349, -108.77202323682606, -110.25970374932486, -112.59574277180732, -109.77247894866957, -110.09219852365874, -111.7197662726775, -109.85454092697009, -110.06789440397942, -110.38055758638309, -111.04251386932805, -111.54279434240568, -109.74385329575985, -110.98924544863415, -111.17898077762852, -110.98364252730245, -110.75024385843372, -109.24766708578407, -109.67753987004863, -110.6537235844391, -111.84436313010086, -109.12654337292446, -109.65519521121124, -111.1845162935778, -110.5009101465602, -110.22980642268818, -110.88540043278346, -110.29249073109453, -108.80459864528464, -107.49372141121728, -108.50353962704821, -110.00730069533373, -112.012876492648, -109.01283702976382, -109.07442203290057, -108.2961442983685, -111.60962842680907, -108.84312815413224, -108.6276642979969, -108.75132871638827, -109.30004903844721, -107.20359872252604, -109.12175943862074, -110.43914247337625, -109.55954680842791, -110.37116786618797, -108.55907813251434, -110.19249995041955, -106.95269845697632, -111.07027929458712, -110.1073996792702, -110.61729280468039, -109.6419175310234, -109.47995019876329, -109.66602827275211, -110.01953864498805, -108.45989120418268, -109.79778555296474, -109.94663827736616, -109.52410616839379, -110.58014441463794, -110.09182359045897, -111.0487262011397, -110.49609187214915, -110.6114701312941, -111.17752423063314, -109.74965389041003, -108.58973724447526, -108.84292130035902, -108.90689510645983, -110.69840140049361, -111.30494362640982, -111.00224390075273, -110.50848328538423, -111.59232911931113, -109.30826761863756, -108.44510893127558, -109.63744704504391, -108.95037574307332, -111.36486409910674, -112.74508631930381, -111.03952454593811, -110.57133212903979, -110.59969855145111, -108.25570461975128, -110.44617635200193, -110.32190307214704, -110.95204704643322, -112.0595421753479, -110.45342552693265, -112.50183987758867, -110.08217804938009, -108.90353583389084, -107.02032313792242, -88.3334978919524, -107.92027625495886, -109.83148570028482, -110.30427997450572, -110.92855407802753, -109.67404674397338, -111.03606345823586, -110.58277018943096, -109.77692362669393, -109.39170901729935, -110.20711662408928, -109.41601946806779, -110.34213214925832, -111.2283900972803, -111.51682597931386, -110.47069117801351, -110.93808974285523, -111.11277478000933, -112.50698886748012, -112.12918507523611, -110.46316790252011, -109.9387334819968, -109.78723249688426, -107.13037722044297, -108.16132376075751, -109.07255491017162, -108.85068428558272, -110.28038153100799, -107.77611023481016, -110.69754506886444, -110.09495581837979, -109.21214884561816, -112.62718526248648, -109.22048725312992, -109.17793923163308, -110.87372121410577, -109.71902632604333, -112.61041177225496, -109.6374750969677, -110.74738952366951, -108.93404661877067, -109.84938675700889, -112.25316361679832, -110.30788094875312, -109.26929069321925, -111.20853536783942, -110.05212566057608, -111.72448131932816, -111.55474439772887, -111.81988954424324, -108.44452452934028, -109.21897824914645, -109.55634869894358, -111.36318572800242, -110.05777399011298, -109.64458567712875, -108.73315084760529, -108.93332091319675, -108.4816455312154, -108.80120578498936, -108.1804470361839, -109.7177707524778, -109.31977709844544, -109.33603116022124, -111.46120546572519, -111.7480378245176, -109.17907150677627, -110.47970652472505, -109.73718750984082, -109.7935026884937, -110.40458408612054, -110.91781389491092, -108.39352075861481, -108.27512197925346, -109.59155075404814, -110.40183121737397, -109.25423373270381, -108.37769008625712, -107.91335995938509, -109.5576520703013, -107.27392145737491, -110.98592762117059, -108.41809950647861, -111.48163889400448, -109.70961684769624, -109.22952568656495, -109.76504719131209, -108.86928627177666, -107.97855299877004, -109.8412204399902, -109.6690048999326, -112.28329030175193, -111.54977099314607, -109.55689540119126, -107.93716711232997, -109.84247640855929, -111.5098351445789, -109.14317615215809, -110.28319116384824, -110.57901069942578, -107.2890252845352, -109.66754569546274, -110.15708115946433, -108.83782190109405, -111.60783857760667, -111.46884385151185, -109.21985333366634, -109.63605494317056, -110.87999187262697, -112.26992029775087, -111.05491095860552, -109.22795442529183, -108.99135781712076, -110.46475190704264, -109.35746113713218, -109.29125989270668, -107.40922407684049, -109.24391685563656, -110.41554602144217, -110.68952735085914, -110.62457364102458, -110.39856310555466, -108.84256124354566, -110.01614601335088, -109.8071306678428, -110.2804500736802, -108.76205061238203, -110.3962440297242, -108.98253716257014, -109.32990745926702, -111.17276766165281, -110.41113652364085, -110.36616199963426, -112.09767002991742, -108.43599666470733, -110.91876588140981, -109.05329272502944, -107.07198690769708, -108.72934463903034, -108.6666471996132, -108.97529973794413, -109.68895260146817, -109.2658844652487, -109.75690097249196, -109.38585024123027, -110.17593039468063, -107.87223111061134, -108.15261097418302, -110.09277437980633, -110.8665497655964, -108.43061614348413, -110.3052458526819, -109.22446919161898, -110.51909692711594, -110.06620699121913, -109.53439413051383, -110.31952463872884, -111.4732125902982, -110.41443606663168, -109.9579358088152, -109.930778061577, -108.5473214465574, -109.34719220288939, -109.16964653934396, -110.04824158176345, -109.42616539603762, -108.3556027482992, -110.62331917617789, -111.3652147859356, -110.12362012120938, -110.13175448595814, -111.20110099151856, -111.50643914621541, -108.11659117128028, -111.06037600347967, -109.03822892917451, -108.25678204604324, -110.82608024151122, -109.15887945314851, -109.88255674562845, -111.18322672526185, -110.95836040044516, -107.91535345885436, -110.66285812468733, -109.61906549925033, -109.58059721670746, -109.65198009505977, -109.65950565672951, -108.95264505276342, -109.23343669003113, -110.74308548011575, -106.39170014998685, -109.61471203101753, -108.24258770956924, -109.84609566640096, -107.83834185503922, -108.93052854090027, -107.55568820082641, -109.758551082242, -110.65892780872205, -111.99907420485852, -110.71043004141137, -110.62257237494617, -109.15610413532767, -106.87403836327807, -108.19175324576331, -110.27819583792918, -110.23918003777561, -108.29703377268754, -110.07182881114713, -109.60256111108491, -111.00394752430006, -110.30750337485472, -108.78309624082331, -109.24103013025798, -108.76979253891403, -109.91618737478264, -108.83915940855513, -110.92536150834754, -109.72250903746432, -108.96533939688658, -111.08949280651164, -109.20335070860871, -109.37826578362439, -109.77953166722301, -110.1867310744785, -110.07114559821346, -110.7003631567182, -107.86455899696074, -108.94113264174617, -109.35999427135138, -109.33627364788704, -108.96588828808375, -109.08716536982254, -108.73575375369026, -109.47770132070654, -109.83726171472907, -110.73516506891792, -110.56827134787686, -107.65667508354096, -109.30200115708924, -109.28406803847896, -110.55374624323233, -111.2017766725333, -108.50851279608973, -109.79494403619485, -109.08320018013063, -110.21850624918747, -108.4652936555984, -108.74837610538873, -108.81326140648238, -108.83830180036702, -108.785270477003, -110.01845876259073, -108.76030368637825, -108.57879884880157, -110.6610608456059, -108.74669367794318, -111.55956030460833, -110.22906685783455, -110.48411613865359, -109.48060880085136, -112.77556331479562, -108.2676071206087, -108.8571136162698, -108.56944905160177, -109.16406757131058, -111.42259299295839, -108.25216316582294, -110.48487127684025, -109.69532331373831, -108.13992755196784, -109.2987762526628, -109.82536192480795, -111.28650061088359, -109.12820736404241, -109.37960655471406, -108.96014976926716, -107.97535047619023, -112.31953123574708, -109.06198330523004, -107.52722515967098, -107.31555373665437, -99.89671790804692, -107.44442600896275, -110.6549218761941, -108.02265794322076, -109.63582761762919, -110.00574746987859, -109.51565124961209, -109.3550083591902, -110.4541529175301, -107.85799722437162, -105.1197113090786, -110.25038075579738, -110.39710812865657, -109.3618876098789, -107.6131301952152, -109.21529527621463, -108.7995754403799, -108.48347353145697, -106.45678488065816, -109.60427918561142, -110.81194387812535, -109.52215044127382, -109.88751598659705, -109.30205143590227, -110.74984456751768, -109.03952092986351, -110.69170786328897, -110.39236248162467, -108.65456161733339, -107.60439764386904, -109.97367926606955, -110.2754359970249, -108.81546418006434, -106.99691398176165, -108.42047325825182, -107.24499915944605, -109.28116135603187, -108.70650358781573, -108.05516916105047, -107.20893100196241, -112.07029265690055, -109.38099990478445, -111.53461820465232, -108.11312509555277, -108.76714028655223, -109.89565008459624, -107.71879172001115, -108.08434857420214, -108.79142773619792, -107.25153085963885, -110.05595039449301, -109.31604222314259, -109.94405791565286, -109.04715370361387, -108.89278831045846, -108.84682466376424, -110.0067927716526, -107.63768959294084, -108.98109382020348, -111.4720219575084, -110.76023788797733, -108.78599647633777, -106.59726674064618, -108.66715709719243, -107.99134359630926, -110.11396713841884, -107.21091759882775, -108.08576824949941, -108.80217666857972, -111.72949572713338, -107.33126296136014, -107.33731660097102, -108.04470462977443, -109.42963925921418, -111.03517778720736, -109.55293581015796, -107.99948151285162, -106.59480934999681, -107.63777243313498, -108.96490626068824, -108.8948210299064, -108.30870516747477, -109.13612869658097, -109.59971429402015, -110.2571461001396, -108.7655464686992, -109.81144209568883, -109.80796806645141, -109.20948481699544, -108.68653880881129, -109.26329796696166, -109.22428132233863, -110.12571678351438, -109.14615461144786, -107.08261621308327, -109.11338327144382, -107.75421565039201, -107.45291780756361, -109.00477000647248, -107.41031480478154, -109.98948062864928, -107.45953654921264, -106.37522884807879, -107.7786128523167, -108.03610987358499, -108.05926797128022, -108.59400205554164, -109.89620453365603, -109.03811240487515, -109.96909236705363, -109.28212981785472, -109.6772152101994, -108.26493868190678, -110.55558039199732, -106.6252818398841, -110.19075011176416, -109.56520012524705, -109.8023423576176, -111.2697570480663, -108.26752571816566, -112.00337375484828, -109.85709226796116, -109.36922081321148, -108.8424844298318, -111.2512302139209, -110.61775974680471, -110.22501328999012, -107.76874906708105, -110.71023653476604, -109.4025656165291, -107.66667684986125, -107.59759854092948, -107.94763263251238, -107.3888591871119, -108.62692803125044, -109.18012867988286, -107.78662871481455, -108.5072814073944, -109.50348958982907, -109.95177634938378, -107.78756251182895, -108.03865042797304, -110.1814993556385, -109.34937567548833, -109.52162025123161, -109.50819015441117, -108.20953105254624, -110.52154040214435, -109.3324404469266, -109.2696617050831, -109.54675609195674, -108.5940367000989, -109.40184828664549, -108.2518305610941, -108.55972691669434, -109.03647225394408, -108.48166656251695, -107.42023429066523, -109.42453054302521, -110.09532345960083, -108.78315822119662, -109.97508586102265, -108.22687406536997, -109.17110028890058, -110.15390449992647, -107.88577458651508, -108.28851074361447, -108.52030295163331, -110.03496861709483, -109.40014319167584, -107.73048113044877, -108.17571683963915, -110.34839852994926, -108.55894048192191, -108.74107339998285, -111.17734138993401, -110.22946440841412, -109.45511941802884, -108.0657300641843, -109.33797363184166, -106.95974095511333, -107.93068343723691, -109.78867669512647, -107.2087297624043, -109.542665021243, -110.05035859052961, -110.30235238883523, -109.20586170783808, -109.2796396673401, -109.14260673746566, -108.22019460542734, -109.99011886871159, -109.89103038547285, -110.36964772493243, -108.62340319923602, -109.06779821699769, -109.21830861066148, -107.7402395759509, -107.7178850938205, -113.45665085929117, -109.24039191621704, -109.30387033426037, -107.61849760982835, -109.41430582703529, -109.11482836392241, -111.89328423764577, -111.84653367963301, -109.00674896486915, -109.84488648739638, -109.41914760797953, -108.53442910169935, -109.66883322968232, -107.68762956301386, -109.82583101109167, -107.83405397804887, -108.78052031141966, -107.37842078941692, -105.40843158543845, -108.81430898189338, -109.57374640194516, -109.41111270322058, -108.82621700188898, -110.2552502368822, -110.23903890097205, -110.52171662278697, -108.21249857906324, -109.97268479379733, -108.20088823960992, -108.85682002802234, -110.11642849164285, -109.94087886999255, -111.63180946270296, -108.20899499456195, -106.73341567332112, -109.90003508676807, -110.14688274481229, -109.62259307329889, -107.57811196819495, -106.88584597822792, -109.16132624528932, -109.78677836397806, -108.59319344451784, -108.55877448618652, -109.46883711353044, -108.47309455543844, -108.09487065732198, -109.82219079158135, -109.63780237877428, -109.28348848877269, -107.62893405379826, -109.46986737961593, -108.03089712610223, -110.3931917410696, -106.06970126043262, -109.41866550703786, -105.31710372440419, -109.20218082282653, -108.28467118008108, -108.80026326744611, -107.40729224715713, -111.07322915141532, -107.1057186510818, -107.98286374205958, -108.51298722989311, -108.69632670891366, -107.96509231988331, -108.15882223414738, -106.85862416470376, -109.70705792539056, -108.64519930633055, -106.78708421443504, -109.43552377900174, -109.4474526498122, -109.10135248755788, -111.43316642580763, -109.33457343739448, -110.23547887071898, -108.95690647379442, -109.21159903769149, -108.12969562680841, -110.82751409340537, -108.55724349027832, -109.8796329603075, -108.50369978374582, -107.43145467247209, -108.60003323209516, -108.77155705999647, -109.33806063660796, -108.37500858898439, -109.65641721611547, -109.81905873737344, -108.03483220769625, -110.48028107566635, -108.60527372219985, -109.28768201151478, -99.8804125587218, -108.8913334544964, -108.23534920737794, -111.07646463287153, -108.59029790589766, -110.3405916586831, -107.66387718565608, -108.73793152614131, -110.61440166477816, -108.76211382544581, -110.23236978486065, -109.10669297094852, -109.15247609779597, -109.00539004923506, -110.14424353412238, -110.55445060661157, -109.48721312920799, -108.17040942305823, -108.77592227268228, -108.77130256578067, -107.82494496098512, -109.57266989523707, -108.75767497229612, -108.13688624150026, -107.8280716764963, -105.676279602552, -107.6370316684844, -109.73508547021689, -109.25365178573009, -108.86767843317584, -109.70969944273735, -108.91917504090888, -109.97734866522867, -112.17308993943783, -110.28356299479682, -110.7927103729386, -110.30837645846702, -107.56364161860179, -109.50188349731121, -109.36065627483853, -109.75389877587511, -109.81713476007774, -108.14524057525358, -109.43832376796216, -110.89342891210596, -108.15657882822792, -106.84106061627887, -107.83091759905821, -108.61794662682962, -109.57142366843581, -109.85402645528154, -110.12877022469837, -109.19414429724044, -110.56168468006764, -108.74720588273881, -107.90448559921305, -108.54421401507743, -105.06700039841249, -109.17937358052484, -108.94317576365822, -107.79410219455083, -109.24955437598658, -108.23334395173994, -108.98759227946937, -107.05986359444529, -107.20956512998849, -109.00295831471958, -109.43119556916457, -108.93348410522628, -108.99932477701081, -106.6448790859128, -109.06877251308666, -107.67053918439544, -109.15052780608639, -110.16878033319385, -106.55101141640301, -108.02811045752685, -111.52173447126572, -110.16854119242062, -110.93164036911654, -111.25979320890855, -108.82629030379024, -108.52004501839738, -107.09697056562636, -108.94233383169858, -107.37962568194772, -109.1239201710643, -108.93949898577122, -110.62573772949195, -110.09592372075662, -107.56136391005947, -110.45600430869621, -108.79481000016084, -109.41462449554598, -109.30248158488335, -108.70735295493108, -109.9174743694956, -109.94232543385962, -110.71725446170196, -110.0346196158573, -110.34814317845934, -110.6651078322521, -107.55409880424479, -108.71734776861287, -109.50902203986271, -110.40207542979611, -108.7847687630861, -111.10599488129682, -109.30824728923263, -108.20134064331717, -110.55959112431609, -107.77099734327174, -110.23862843385446, -108.48520797666865, -108.54205896654946, -107.79288769037599, -109.84022250170581, -108.02758364115576, -109.35132492327935, -108.87009749667932, -109.86905123364855, -109.19826752168308, -106.835240323691, -109.37910022114056, -110.80633973102931, -109.12703823829597, -111.07432699570984, -111.8064506085314, -110.09349947650527, -108.66467295777367, -108.75119108236053, -112.63983351316729, -110.90940743670113, -110.27973159222081, -109.57141664526549, -108.61645363771719, -109.31742355616147, -109.5839599160637, -110.01188998365383, -110.01923429741011, -108.94779759137936, -108.26169431000017, -109.24553201026085, -109.95709526422822, -110.68677343596859, -108.7678734483002, -110.47090469179284, -110.31604700116512, -110.10256600741997, -109.76634647265719, -110.8830805828562, -109.94609564072982, -109.20662382740542, -108.12492970530919, -110.5274435478767, -108.02351960398035, -110.6264936805739, -107.14559226383577, -109.13821777857531, -111.05324489472586, -110.15190797512811, -107.96366234783144, -110.03950681967147, -109.17476300510336, -110.41251816187909, -111.39219865477246, -111.32530426869943, -109.97369363558423, -108.98666403063845, -109.62049358645565, -109.58130494498671, -111.72738873188874, -110.39825891106616, -108.57430325757545, -111.28625510212446, -108.77421250595326, -109.75025415031793, -109.51948456745635, -108.82129398637998, -109.81362137198361, -107.86292494316123, -107.49318292857053, -109.66948564589373, -109.54288390056654, -107.99912445612077, -110.3497559614379, -108.00549349666127, -110.01361420523357, -108.4977916421456, -109.67078387286976, -109.85678367732866, -112.01237658746248, -108.4855625950998, -110.84880875737286, -110.9178674382154, -110.44187536727453, -108.75076921971127, -110.04946286646651, -109.99780941000827, -110.14242932305507, -109.56343773672316, -109.6278993388131, -108.77419573790174, -109.10543670530926, -109.7801848627463, -110.30733124104881, -113.13440550301436, -109.32709134514755, -109.74136656933283, -110.01525283266193, -109.43924662938396, -110.25325289253, -107.75460576671303, -110.60057027395933, -110.71458404922404, -110.15788509050662, -110.69167485018224, -110.96006652476157, -111.01156633983031, -111.6058448010008, -109.51364005052672, -109.76058205940885, -108.43421621088261, -109.47973949170208, -109.25533250208288, -109.47422603921065, -111.36411644613841, -107.27566171102698, -110.45098686173688, -109.93589296291184, -109.03803734663714, -110.53118128434016, -110.2408872254969, -110.0532234862915, -109.94185495614619, -110.2662004220774, -109.51094016962288, -108.5210104215432, -108.13691752270934, -110.18460088390265, -108.32609309150783, -109.89652230508281, -109.80923900768477, -109.01917388968883, -110.01248300968739, -109.43415605440147, -108.09823485138017, -107.40637725320931, -109.40632232658412, -111.97981999127656, -111.16609811629485, -111.64500793960192, -110.99793748693381, -109.55531276386903, -110.2535662621666, -108.17429802469516, -109.09425673355422, -110.23187110421917, -110.55358397926925, -109.93461124753053, -109.55604345832225, -109.44569510408274, -109.72185151080762, -109.52963702944834, -109.2303630328152, -109.74819502244243, -109.3932530349457, -109.17096788339686, -110.46153727064616, -113.1073731246639, -109.43753070459397, -108.13332547768168, -109.42294574929969, -108.45798401969856, -110.29453435046327, -112.66249403705643, -108.78314667434937, -105.9634478773668, -109.14327524669528, -108.50645190860273, -100.81571594994128, -104.4482859840643, -110.68926237051092, -109.12362553230196, -109.45234390564677, -107.91461416156068, -110.67788819353727, -110.05744935668449, -111.78333392154664, -106.83628914455993, -110.11115457346548, -109.13434608275826, -110.80006861194663, -110.35323502651462, -112.29149906501372, -109.01656376530778, -109.30871662948859, -109.79736315392456, -109.17848983603582, -108.09752397056482, -111.6039030763455, -109.27008844877828, -110.84475733314184, -109.72393917557073, -111.31060762894991, -110.78858793807466, -107.12841545099752, -109.54510865218204, -105.2805426080281, -106.28514149354733, -109.50656759582803, -110.14700878401054, -110.49737016725709, -109.19811547071924, -109.92527399676051, -110.7961615015146, -109.7447227818197, -109.49432012009893, -108.714081576733, -110.09766801550917, -109.08448507943001, -110.36154838733857, -109.86328656267403, -109.21144237434696, -112.4145136888034, -108.57567151011159, -109.66748589540896, -109.72985837578446, -109.29989238126763, -109.85868902806475, -111.01778182304162, -111.23625326328558, -110.01270868104203, -109.27067928081415, -109.71171312410247, -109.28697459293629, -110.67868067201007, -110.91353786857455, -111.21479955051575, -109.11315965407708, -109.40418681804496, -107.80511819596003, -107.37201025889816, -111.81969609169838, -109.89875624306032, -110.29328043898657, -109.74853280072202, -111.39527865400605, -109.47746221101964, -111.75141177452517, -109.31325306583483, -109.30117448911659, -109.3997781364162, -109.45356931295724, -109.60585285774386, -111.33951689512735, -107.74187210470228, -109.62706021606415, -108.72139655505221, -109.79552836110567, -110.64354037499807, -110.96138240913136, -110.02215059889615, -110.92978442698893, -110.0620778287114, -110.85019647293322, -111.77397403227091, -109.81257196800128, -109.15643451383403, -110.72777566469594, -108.7463769025616, -109.80959395914073, -111.24500986151126, -110.48863498350322, -110.30863780110901, -109.79331354195703, -110.34087081762074, -109.45183222569266, -109.6440990067103, -111.15034876658994, -112.14912485578341, -111.8886180186196, -110.57054820211916, -111.07556239924551, -110.5872832735073, -110.28912501038172, -108.91501133754849, -111.44575118962761, -109.90799859177967, -109.74421995550023, -108.70941446115883, -110.28822893097275, -109.70039554000401, -110.33701797570251, -110.79445894683306, -109.57694314608153, -108.816904416038, -109.66517126767175, -109.39501469321644, -110.85775022889956, -109.3689402795614, -112.09107318723095, -110.67985626248422, -110.32971146814747, -112.08166943494875, -109.93955548712543, -109.31722953035252, -110.2062913031861, -108.22565380081006, -110.680898028151, -111.95386604441454, -110.83354130587097, -108.5873626748948, -111.97536144124408, -109.23944159551515, -111.57859477689586, -110.80135186615524, -110.4800953731021, -110.14040729648133, -109.25873050390551, -108.87000960474569, -110.97091597211167, -110.15787270199012, -111.62434537618091, -108.5421625277294, -110.42258666403919, -110.96896115868603, -108.98253068925274, -109.54245055160168, -110.28051096122468, -109.48060498658319, -109.77618362117276, -111.64513838754992, -111.13945484239875, -110.18094280356001, -110.43757222770748, -110.81588360154201, -110.11656805555333, -108.47936291282355, -109.16476249859961, -109.3549985917136, -110.77753190334253, -111.46065694661178, -110.40387985996301, -109.95673803226478, -111.58660981285446, -108.59894875229345, -109.37333363882607, -110.26849699991793, -109.30500469266264, -109.23789020998296, -110.82000706486865, -109.25927538839868, -111.03285659417519, -111.08899832832414, -110.69361682858042, -109.45187168573815, -109.9614018482838, -109.70209527974106, -112.11903952100165, -109.59713611623246, -110.70292028698111, -110.12743849746808, -110.63315585514292, -108.60450276298175, -109.32832664986026, -109.99753023477764, -109.46644696130294, -109.1781290160558, -111.58830180575129, -111.67229040267557, -111.3750024136205, -108.33616679452298, -109.99797067800029, -110.50892429124391, -108.66074740829372, -111.17094662568759, -109.87538933985836, -109.152526628291, -110.44623159817101, -110.21603106403009, -110.64376935639365, -109.36897426842583, -108.67303022227141, -109.89327693080823, -111.50442955563923, -111.37532237834381, -109.38132821290205, -109.73509680539144, -110.53918379735906, -111.22869870340647, -109.39977573957616, -110.3674665334106, -110.5366125953241, -109.99025356764304, -109.97300035646616, -109.87631077033762, -109.64608829594286, -113.02486102973394, -108.26250283140733, -109.62234918138763, -111.18766216512655, -110.33666026406992, -110.5808115327039, -108.2971671321189, -110.10964334161903, -110.61254021379767, -109.89852549557533, -110.16562049054073, -109.41433790018287, -111.2453823439446, -110.45554802599901, -113.11454453784393, -110.7333866145056, -110.00858191882439, -108.54745315874294, -110.08430415376903, -111.9006972727596, -110.3031506154679, -110.26331790366497, -109.36797925566673, -109.04860552478912, -111.83514212681175, -111.38960737633833, -109.01429665187288, -110.96404839103826, -108.95488871107163, -109.09652004914592, -111.884304581971, -110.57566691021339, -111.95113404442795, -110.13677174050159, -108.10078686353354, -107.69442565416006, -112.42676605669463, -109.12681161784135, -109.23120766087519, -110.57649395555585, -110.22143082743162, -108.40065951773644, -109.46923168308618, -111.39095086729745, -110.46375658526013, -111.45145283328486, -112.22610823637353, -110.61090190564383, -112.22250292674809, -111.7379343196361, -110.18530386733481, -108.93867365671692, -111.89304844956082, -109.06146134986984, -110.98405731832798, -109.76366821333497, -108.08326795663608, -109.95041147835065, -112.94140614324155, -111.79814935135965, -108.07337559063119, -109.13733403265212, -111.74906646037496, -111.12228668433455, -110.02899450462209, -110.22237716929811, -109.0224776891049, -110.18135850497721, -113.32516073881047, -111.3576490243877, -110.60510094465171, -109.6935518470342, -110.36313473154901, -111.95933240129618, -109.49625308071019, -109.18827910216122, -110.54311407822692, -108.4811035913567, -112.81280225723607, -108.86530665787413, -110.85796435061886, -110.40059714639627, -108.19250716343407, -108.96956521802292, -108.61281798886506, -109.78061525370413, -111.58885511891798, -109.06279169160345, -111.43043988466789, -111.63169336321079, -109.54702536206447, -109.62860636296405, -109.47865811135546, -108.02265793654806, -109.97461304995515, -110.72549884050886, -111.57309413919933, -110.03317891949746, -110.39570411598524, -110.27606115470397, -110.63294457306095, -110.71821689302902, -110.38076268941819, -111.51223508887897, -110.40703572670697, -112.24933273737743, -109.74954300082398, -108.46020292937696, -111.05315219575881, -110.38635148390118, -109.58268303790976, -112.34211536832117, -108.45894118755307, -108.96463982695337, -110.56040438523046, -110.67803313671729, -111.07349872375121, -110.42184162876096, -111.82081126435692, -108.85923651136297, -112.57723799596502, -113.65690874668172, -112.62314325834605, -110.70357529341362, -110.959925221544, -111.26336183001875, -108.1350700630152, -107.94545932312926, -111.17610778209841, -110.20386728310686, -108.55646511121591, -109.8400922569145, -111.73466587035968, -110.47272877573613, -108.33011124048193, -107.93042857580332, -108.60928277989103, -109.25240966798974, -108.96403833602028, -106.94222615757475, -109.37086694261907, -106.72743097285155, -109.03160193412796, -107.3549903889451, -106.8543848510082, -107.83503929060929, -106.30745467433752, -108.36915807168845, -107.13065938379303, -107.84769200880969, -106.08004345082777, -108.15244601930225, -108.37254117816573, -106.57863034819223, -108.1283698227614, -108.19776505569902, -107.58283412238643, -108.17365133196301, -108.6794309781181, -107.91552140588759, -111.60122989270022, -107.04360635941174, -111.55535949001795, -109.39870426166594, -109.55937904851662, -111.81389508925734, -109.88957041098786, -110.84764586896561, -110.59130246272693, -111.15944135223884, -110.19496154041607, -111.51861903129362, -110.74798816525838, -111.37312965175558, -110.10842817220238, -110.73198099204856, -111.36708667993291, -110.30840247819665, -110.11744489669044, -110.55237850846444, -108.2073528237766, -112.70750856801911, -110.99917956040802, -109.84949484779976, -111.3403161887679, -110.08924435263565, -110.17749213365616, -112.10849123224503, -110.94270741299202, -109.29350963424746, -110.33477486966507, -112.19620157705627, -111.45484078395934, -111.86858843505124, -110.22491147345858, -108.96177661263177, -108.67862820579893, -107.55155410582937, -108.27984439169573, -108.72682528077233, -110.64231212183269, -109.32873093119183, -112.98564364754564, -110.78933114228725, -108.50921025910479, -107.91087245586935, -112.57350030929283, -111.75871577457525, -108.42095298945462, -112.31266064114303, -110.1295657579673, -109.67444664474456, -110.33749884929306, -109.16098218724147, -109.63554874360221, -109.15892392675141, -111.90580809179818, -108.81196712336858, -111.42223552606656, -109.90571484965518, -109.99739812086352, -111.64103850263211, -111.31463957090885, -110.61247447444549, -110.20960333715526, -110.1707327818923, -109.70412636554525, -110.97278093107532, -110.24386747740314, -109.81378546061525, -110.83784085086458, -109.77357954318757, -111.22663832948885, -111.14563050139252, -110.87152231402447, -110.34246044319893, -109.97174570657546, -110.23599592972218, -111.08206161770731, -110.0073315341242, -111.11748366902188, -112.04005964728601, -109.81290191679287, -109.68543639040858, -112.01143296194752, -110.13641850530031, -108.19348942447623, -109.7534468948808, -109.36697824644176, -97.56454580435337, -104.97829040517887, -108.1539132982256, -110.048991273122, -107.46172505860011, -110.49269280640675, -109.94209901400029, -109.38576869679022, -111.43699124347364, -110.89973083498887, -111.2994445418276, -109.25144782032437, -113.25676258473536, -110.82078737428088, -109.97779571182073, -113.36294799183014, -111.38584551238931, -112.17267897274873, -108.56430946159155, -112.06841286528645, -110.36822473102735, -109.54758527532016, -110.48190506674653, -110.03535695860182, -109.3951469796576, -112.41910682256774, -111.38124138857238, -109.37850389100952, -111.65544568836181, -111.55876881606889, -109.3029209617236, -109.20030046194076, -108.82610577621037, -110.53329453526098, -109.96090595542142, -109.67834229432077, -110.62303603007352, -109.8388817181171, -109.22430039793213, -108.92749786663613, -110.05794249283548, -109.58534943218437, -110.50493887507297, -109.96373022997366, -111.0645036323456, -111.28501675364454, -109.77386932343008, -108.8952247140968, -110.09242801628717, -112.90943444063141, -110.72299296247249, -109.39094335967056, -110.95165384057718, -109.59809519359453, -110.4978602309597, -109.67109981692639, -111.2489619905986, -110.0937750887109, -109.76771021128954, -108.32976315018955, -111.3058145792439, -111.09464974601362, -110.99797900696136, -109.174315000222, -109.630351559617, -110.26289147175856, -110.22688407202517, -109.96748050100612, -112.13247633583758, -110.59994952890855, -110.93023020153811, -109.22457750926695, -110.26162558926984, -110.09713110375579, -111.73858994918328, -109.78183160058515, -109.7603471824367, -110.96016892586911, -111.23309626937036, -109.83093663960678, -114.05354944347246, -111.58202863059464, -110.42281828744524, -110.9521484732059, -112.5120328206343, -111.614891937737, -109.84428787405484, -111.61119567831453, -110.43095563229411, -111.71833448430398, -110.01132196809407, -109.37558169247951, -109.14091380022785, -110.42663661754088, -110.3598013572826, -109.78207135281417, -109.94058843992468, -109.88210328447205, -108.6217811850147, -107.17834387173707, -110.6447226986756, -111.10704778101115, -111.24396771977769, -110.47849395539598, -110.75150631628034, -109.67662689396347, -109.23145032835053, -108.83780193265358, -109.43468321661163, -102.22521103859944, -106.90009867479111, -108.91580608784525, -109.58671397003187, -110.56692028436989, -108.75103142680105, -111.00795573084157, -110.75039085328763, -109.48222099288613, -111.8621134816908, -110.26507966786443, -108.885924716389, -109.30841399453053, -112.3188631425597, -111.05677697153163, -108.8268571902449, -109.63028152237679, -114.82339015806369, -107.03435216376964, -111.34847692589166, -109.61354114874855, -112.32687758049907, -109.59816404231358, -111.64248480241805, -111.84075757907273, -110.44017657636552, -110.15181635726277, -111.93813663582833, -109.11826378836209, -109.99779889778326, -109.927119030584, -109.4389650887841, -111.52448814187727, -111.38736268499642, -110.51920914917922, -108.64230614681055, -108.90307263595304, -110.57246891832371, -109.65575340646116, -109.80359672370373, -108.83368585528197, -111.09385004343437, -108.83430005497769, -112.37784208819113, -109.50005381621696, -109.67421750136593, -111.39664088797532, -109.70867599669316, -109.52498993629875, -111.12341349673187, -110.0484037026941, -109.55138667646308, -111.06614422098669, -109.4785941493091, -110.25724082617013, -110.93950616855716, -110.53487953881397, -111.45722057988401, -110.32393446412904, -110.34361936710438, -108.6610336097813, -109.53631603696368, -108.06930707969195, -107.68056561368934, -108.73860971027449, -108.87111384617579, -108.40433837098611, -110.55999576884835, -106.83832061167207, -108.28786975902513, -109.18482905697472, -107.81071696594883, -107.91047268802457, -108.79613111673706, -111.05361322310213, -109.97897453479862, -109.12920563729425, -111.20538391490288, -109.26286135293664, -111.31400407177502, -109.92167984752287, -110.70854322826071, -108.59406515713611, -109.69371333227458, -109.36664873267313, -110.35521729513704, -110.40667924006368, -112.0181844636846, -111.01529188207431, -110.59246505728431, -109.95068312717868, -110.75807466894047, -109.58596443762707, -111.12127793384956, -109.59041634463125, -111.56255571372793, -110.43405578864342, -108.39660324329928, -111.1420710307505, -113.64788483868595, -111.67645688353934, -111.36878760365944, -109.68523694561108, -110.11608766310304, -109.25670490330123, -110.73546181099229, -111.77855039399805, -107.9662794718261, -109.67483334602832, -109.891258579519, -110.24757768183042, -109.50202895993814, -110.07763831916637, -109.96891925839451, -110.97268925927641, -109.31698133827767, -112.27933593506792, -110.36206721075725, -109.47379463718867, -110.27836850941338, -110.63738280998388, -111.3611682777485, -110.72689155959884, -111.55480904927032, -111.16689658479412, -110.35555645743601, -111.56609319131051, -110.88279459952174, -114.73607246523177, -109.95813757295693, -107.64639932425493, -111.26486783320321, -112.03946356928121, -111.8915972448334, -110.35245920812773, -110.83155104803564, -110.67437747473863, -110.9959682920065, -110.7815352345103, -111.13722283763049, -112.54797265493127, -110.06894780898469, -111.65186554925783, -111.83545188116254, -110.65894756123697, -108.48458025065264, -112.43760714427981, -114.1368408201927, -110.40065777895025, -110.1066998945526, -108.60654239598591, -110.5716060205154, -110.74257357180736, -111.1136089342442, -111.53539811075092, -113.2559601458872, -109.2003227548348, -110.42285840441025, -111.4086884998834, -111.61503050693868, -110.8194303494779, -108.9701587059964, -112.58521089509063, -110.10873915265242, -112.43440038319561, -110.03468788439882, -111.57896603236308, -110.21939233582523, -109.03614470500777, -110.11738923539659, -109.55359574898291, -110.416473622654, -109.4626868574157, -111.17164025076731, -110.3579689035081, -109.04338716157822, -112.36157114517567, -109.32125615922843, -112.71105693789394, -110.11019129547768, -108.96439402555632, -111.107663418839, -111.48306369859839, -110.9317530461794, -107.98628540532181, -111.1636972328743, -110.47837837583148, -109.04649309175733, -110.27110334963734, -111.35803630614352, -110.77259078859605, -111.46352820533895, -111.16789261049541, -109.2376344776325, -111.6795794983659, -111.74292205167644, -109.40835022991612, -111.02163652600731, -108.79482078001607, -110.6718658416566, -111.08747067599332, -112.15383726791498, -109.47049126158717, -109.061574046483, -111.23993049318979, -111.02521156588335, -109.46012868444186, -110.13918914826291, -112.08180381836377, -110.61929875223015, -111.4424805369965, -111.43420275069585, -109.71347556238717, -110.24726273025648, -109.7860268673935, -109.94126895018422, -111.41948668868926, -108.90555991781676, -110.81242861886172, -109.65007052722677, -112.12672329335953, -110.01123170946096, -111.13980448279096, -113.92013682657084, -108.6000853867411, -110.66793592761913, -110.61237681642844, -110.00839105230496, -109.38083187034974, -109.46119372195675, -110.3708067287448, -108.55518656223285, -113.33935987443276, -111.92184778392033, -111.80820718236087, -107.36852757311246, -109.51077803361602, -110.066791721019, -108.756710558672, -107.91391289865918, -110.72851430959301, -111.39074956442978, -112.928843679455, -109.87348280521556, -112.21371750380071, -110.82495902297394, -109.94006136010094, -110.58757785050143, -110.2790091349881, -111.43884888223081, -108.09540986530712, -109.63783244641691, -110.19577975613292, -110.01690033746098, -112.75938920157155, -109.27158857362184, -111.19519821680541, -110.14381902425255, -110.45955291199236, -111.55660330002316, -110.75604254261134, -111.02122553784838, -111.6490091060193, -110.93362819419399, -110.49033159684308, -110.70789549836027, -110.41991882034145, -110.0264093421208, -109.18432746063652, -110.15292268755287, -112.40733942236504, -111.32869665965416, -110.95418667871114, -111.14291568823575, -111.75555369152653, -112.98146297069803, -109.73870744292117, -111.33806139459435, -110.18838799491355, -112.60408243005732, -110.26112648646833, -110.58257045107274, -109.75155437454112]}, ...(2 in all)]
  in  "FFT 1 Choice 1":u16(ring) items=["T1 Y", "T1 X", "T1 Sum", "T2 Y", "T2 X", "T2 Sum", "T1 FB X", "T1 FB Sum", "T2 FB X", "T2 FB Sum", "PSD Y", "PSD X", "PSD Y Sum", "none"]
  in  "FFT 2 Choice 1":u16(ring)=3 items=["T1 Y", "T1 X", "T1 Sum", "T2 Y", "T2 X", "T2 Sum", "T1 FB X", "T1 FB Sum", "T2 FB X", "T2 FB Sum", "PSD Y", "PSD X", "PSD Y Sum", "none"]
  in  "FFT 1 Choice 2":u16(ring)=1 items=["T1 Y", "T1 X", "T1 Sum", "T2 Y", "T2 X", "T2 Sum", "T1 FB X", "T1 FB Sum", "T2 FB X", "T2 FB Sum", "PSD Y", "PSD X", "PSD Y Sum", "none"]
  in  "FFT 2 Choice 2":u16(ring)=4 items=["T1 Y", "T1 X", "T1 Sum", "T2 Y", "T2 X", "T2 Sum", "T1 FB X", "T1 FB Sum", "T2 FB X", "T2 FB Sum", "PSD Y", "PSD X", "PSD Y Sum", "none"]
  in  "Compute FFT":bool
  in  "Reset FFT":bool
  in  "# Spectra to Ave.":dbl=25.0
  out "Ave. Time (s)":dbl=1.5
  out "1 Channel":waveform(dbl)(graph)={"t0"=timestamp(0 s since 1904-01-01), "dt"=1.4999999999999999e-05, "Y"=array[20000 elements], "attributes"=variant("NI_ChannelName"=variant(string "T1 Y"))}
  out "Slow mean":dbl=nan format="%0.2f"
  in  "Slow mean N ave.":dbl=1.0 min=1.0 step=1.0
  out "Mean Intensity":dbl=nan
  out "Sigma":dbl=nan
  out "Sigma/Mean":dbl=nan
  in  "Subtract mean":bool
  in  "High Res. Display":u16(ring) items=["T1 Y", "T1 X", "T1 Sum", "T2 Y", "T2 X", "T2 Sum", "T1 FB X", "T1 FB Sum", "T2 FB X", "T2 FB Sum", "PSD Y", "PSD X", "PSD Y Sum"]
  out "APD 1 Rate (Hz)":dbl format="%#_3p"
  in  "Tab Control":T4(tab)
  out "Stage Moving":bool
  in  "Read Cal":bool
  in  "Confocal Linescan":bool
  in  "Speed (nm/s)":dbl=100.0
  in  "Furthest Withdraw (MHz)":dbl=15.0
  in  "Confocal Image":bool
  in  "Round T1 X":bool caption="Round"
  in  "T1 offset_x (mV)":dbl=nan format="%#_2g"
  in  "T1 kappa_x (pN/nm)":dbl=nan min=0.0 step=0.001 format="%#_2g"
  out "Time (s)":dbl=6.12
  out "Total Time (s)":dbl=60.0
  in  "Start Saving":bool
  in  "Cal sets to save":u32=50 min=1 step=1
  in  "Comment (data description)":string="testing confocal setup"
  out "Calibrating Trap...":bool
  in  "Trap 2 (ON/OFF)":bool=TRUE
  in  "Trap 1 (ON/OFF)":bool=TRUE
  in  "Save Calibration":bool
  in  "N sets to save":u32=200 caption="N Sets"
  in  "Save N Sets":bool
  out "Save file name":path=path "C:/Data/110526/110526_022.dat"
  in  "Save ave N":dbl=500.0 caption="Averaging Factor"
  out "Saving...":bool
  in  "Stop Saving":bool
  out "Progress":u16(slide) scale=0.0..100.0
  out "Manipulating Trap":bool
  out "Buffer Status":dbl(slide) scale=0.0..1.0
  out "Overflow (data lost)":bool
  in  "Reset":bool
  out "Data Rate (Hz)":dbl=66666.66666666667 caption="Trap Data Rate (Hz)" format="%#_3p"
  out "Data Period (s)":dbl=1.4999999999999999e-05 caption="Trap Data Period (s)" format="%#_6p"
  out "Save Data Rate (Hz)":dbl=133.33333333333334 caption="Rate (Hz)" format="%#_6p"
  out "Save Data Period (s)":dbl=0.0075 caption="Period (s)" format="%#_6p"
  in  "T1 alpha_x (nm/V)":dbl=nan step=10.0 format="%#_3g"
  in  "T2 alpha_x (nm/V)":dbl=nan step=10.0 format="%#_3g"
  in  "T2 kappa_x (pN/nm)":dbl=nan min=0.0 step=0.001 format="%#_2g"
  in  "T2 offset_x (mV)":dbl=nan format="%#_2g"
  in  "BD 1 Frequency 2 (MHz)":dbl=80.0 caption="T2 X (MHz)" min=50.0 max=100.0 step=1.0 format="%#_6p"
  in  "Green Laser ON/Interlacing":bool=TRUE
  in  "Round T2 X":bool caption="Round"
  in  "AO1":dbl(slide) caption="Confocal Y (V)" min=0.0 max=10.0 step=0.01 scale=0.0..10.0 scale format="%_1f"
  in  "AO2":dbl(slide) caption="Confocal X (V)" min=0.0 max=10.0 step=0.01 scale=0.0..10.0 scale format="%_1f"
  in  "Trap Raster Scan":bool
  out "Raster Scanning...":bool
  in  "Trap Delta (MHz)":dbl=20.0 step=1.0
  in  "Trap Intensity\nSetpoints (V)":cluster{"Set 1":dbl, "Set 2":dbl}={"Set 1"=5.2, "Set 2"=6.6}
  in  "Index":dbl=1.0 caption="Save File Index" min=1.0 step=1.0
  in  "BD 1 Frequency 1 (MHz)":dbl=65.0 caption="T1 X (MHz)" min=50.0 max=100.0 step=1.0 format="%#_6p"
  out "Current Position":dbl[](array[numeric])=[4.2944, 4.91027471, 2.9278058] format="%7_7g"
  in  "Position Label 5":string="upper flow spot" caption="5"
  in  "Position 1 Label":string="Top capillary (SA beads)" caption="1"
  in  "Position 2 Label":string="Bottom capillary (AD) beads)" caption="2"
  in  "Position 3 Label":string="lower flow spot (ATP)" caption="3"
  in  "Position 4 Label":string="Dump beads" caption="4"
  out "Pump 3 cont disp":string="Left: ADig beads"
  out "Pump 1 cont disp":string="Right: DNA beads "
  in  "Ch 1 Inject Rate (ul/h)":dbl=50.0
  in  "Pump write delay (ms)":dbl=300.0
  in  "All Pump Parameters":T5={"Pump 1"={"Diameter (mm)"=4.61, "Units"=4.0, "Volume"=100.0, "Rate"=50.0}, "Pump 2"={"Diameter (mm)"=4.61, "Units"=3.0, "Volume"=0.0, "Rate"=0.0}, "Pump 3"={"Diameter (mm)"=4.61, "Units"=4.0, "Volume"=100.0, "Rate"=250.0}}
  in  "Ch 2 Inject Volume (uL)":dbl=100.0
  in  "Pump pause delay (ms)":u32
  in  "Ch 3 Inject Volume (uL)":dbl=100.0
  in  "Ch 3 Inject Rate (ul/h)":dbl=250.0
  in  "Flush Center Ch Volume (uL)":dbl=15.0
  in  "Flush Center Ch Rate (ul/m)":dbl=100.0
  in  "Inject Valve B":bool caption="Inject Pump 2\n(Flush Center)"
  in  "Total Volume\nFlushed (uL)":dbl
  in  "Tab Control 2":T6(tab)=enum."Feedback on Trap Intensity"
  in  "Restart RF":bool
  out "Total Counts (ticks)":u32=600
  in  "Trap ON/OFF X or Y Amp?":bool=TRUE
  in  "Oscillate Set 2":bool
  in  "Trap 1 ON":bool=TRUE
  in  "Number Interlace Sets":u8=3 min=1 max=3
  in  "DIO count 3 (ticks)":u32=200
  in  "DIO count 2 (ticks)":u32=200
  in  "DIO count 1 (ticks)":u32=200
  in  "BD 2 Amplitude 3 (%)":dbl min=0.0 max=75.0 step=1.0
  in  "BD 2 Amplitude 2 (%)":dbl min=0.0 max=75.0 step=1.0
  in  "BD 2 Amplitude 1 (%)":dbl min=0.0 max=75.0 step=1.0
  in  "BD 1 Amplitude 3 (%)":dbl min=0.0 max=75.0 step=1.0
  in  "BD 1 Amplitude 2 (%)":dbl=30.0 min=0.0 max=75.0 step=1.0
  in  "BD 1 Amplitude 1 (%)":dbl=30.0 min=0.0 max=75.0 step=1.0
  in  "BD 2 Frequency 3 (MHz)":dbl=26.0 min=50.0 max=100.0 step=1.0 format="%#_6p"
  in  "BD 1 Frequency 3 (MHz)":dbl=70.0 min=50.0 max=100.0 step=1.0 format="%#_6p"
  in  "BD 2 Frequency 2 (MHz)":dbl=26.0 min=50.0 max=100.0 step=1.0 format="%#_6p"
  in  "BD 2 Frequency 1 (MHz)":dbl=26.0 min=50.0 max=100.0 step=1.0 format="%#_6p"
  in  "Not-Interlacing Set":enum32{"Set 1", "Set 2", "Set 3"}(radio)
  in  "Interlace":bool=TRUE
  in  "Trap 2 ON":bool=TRUE
  in  "Trap 3 ON":bool
  in  "Scan axis 2":bool=TRUE
  in  "Osc. freq. (Hz)":dbl=0.25
  in  "Osc. amp. (MHz)":dbl=2.0 format="%1_3g"
  out "Coords":T7
  in  "Manipulation Scaling":cluster{"Horizontal":dbl, "Vertical":dbl}={"Horizontal"=0.075, "Vertical"=0.01}
  in  "Freq or Amp switch first":bool=TRUE
  in  "Swap F1 and F2":bool
  in  "Freq switch delay":u16
  in  "Amp switch delay":u16=5
  in  "Period":i64=2
  in  "MCL Step Increment (V_int)":dbl=3.0
  out "Time to Finish All (min)":dbl=0.122877 format="%#_2p"
  in  "Scan Speed (nm/s)":dbl=100.0
  in  "Scan Range (nm)":dbl=369.00000000000034
  in  "Step Size (nm)":dbl=1.0
  in  "MCL/AOM Scale Tweak":dbl=1.0
  in  "MCL Step Position Ratio":dbl=0.5
  in  "Move MCL Also?":bool=TRUE
  out "Final sep (nm)":dbl=4587.0
  out "Initial sep (nm)":dbl=4218.0
  out "Save index":dbl=22.0
  out "Final delta (MHz)":dbl=44.0
  out "Initial delta (MHz)":dbl=41.0
  out "Final freq. (MHz)":dbl=50.0
  out "Initial freq. (MHz)":dbl=53.0
  in  "Saved AOD Raster Scan Parameter Sets":T8(array[cluster])=[{"Scan Range AOD (nm) 2"=500.0, "Step Size AOD (nm) 2"=1.0, "Scan Speed AOD (nm/s) 2"=100.0, "Number of scans (AOD) 2"=1, "Label"="offset curve"}, {"Scan Range AOD (nm) 2"=420.0, "Step Size AOD (nm) 2"=1.0, "Scan Speed AOD (nm/s) 2"=100.0, "Number of scans (AOD) 2"=1, "Label"="hp raster check"}, {"Scan Range AOD (nm) 2"=6.8, "Step Size AOD (nm) 2"=0.34, "Scan Speed AOD (nm/s) 2"=0.34, "Number of scans (AOD) 2"=1, "Label"="3.4 kbp - 1 bp steps"}]
  in  "Load parameters":bool
  out "Scan Range (MHz)":dbl=-3.0000000000000027
  in  "Restart DMA? (AOD)":bool=TRUE caption="Restart DMA?"
  out "Incr. int (AOD)":i64=-7759651845
  out "Time/Scan (s) (AOD)":dbl=3.68631 format="%#_2p"
  out "Data points/scans":dbl=491508.0
  out "Data points/scan (f/b)":dbl=491508.0
  in  "Save scans":bool=TRUE
  out "AOD Scan I":u64 caption="Scan I"
  in  "Continuous AOD Scanning":bool caption="Continuous Scanning"
  in  "Abort AOD Scan":bool caption="Abort Scan"
  in  "Scan BD":bool=TRUE
  out "Cycles/step (AOD)":u64=666 format="%.3p"
  in  "Number of F/B Scans (AOD)":u16=1 min=1
  out "Scan steps (AOD)":u64=369
  out "Scan Increment (MHz)":dbl=-0.008152173913043485
  out "AOD Scanning":bool caption="Scanning"
  in  "Start AOD Scan":bool caption="Start Scan"
  out "N sets should be saved":dbl=24.5754
  out "Progress 2":u16(slide) caption="Progress" scale=0.0..100.0
  in  "Abort save 2":bool caption="Abort save"
  in  "Trap 1 Bead Size (nm)":dbl=2100.0
  in  "Trap 2 Bead Size (nm)":dbl=2100.0
  out "MCL Count":dbl=230502201.82069838
  in  "All FB On/Off":bool
  in  "AI2 to Setpoint":cluster{"Set 1":bool, "Set 2":bool}
  out "AI2 (V)":cluster{"Set 1":dbl, "Set 2":dbl}={"Set 1"=-0.0012207403790398877, "Set 2"=0.004577776421399579}
  in  "Reset Feedback":cluster{"Set 1":bool, "Set 2":bool}
  in  "PID Gains":T9={"Set 1"={"proportional gain (Kc)"=0, "integral gain (Kc*Ts/Ti)"=5, "derivative gain (Kc*Td/Ts)"=0}, "Set 2"={"proportional gain (Kc)"=0, "integral gain (Kc*Ts/Ti)"=5, "derivative gain (Kc*Td/Ts)"=0}}
  in  "Feedback On/Off":cluster{"Set 1":bool, "Set 2":bool}={"Set 1"=TRUE, "Set 2"=TRUE}
  in  "Set SP to Reading":bool
  out "Trap X (AI1)":T10={"Trap 1"=-1.0, "Trap 2"=0.899993896484375}
  in  "Trap Pos FB SP":fxp<+/-,16,1>=-0.092803955078125 caption="Setpoint"
  in  "Trap Pos. FB ON":bool
  in  "Reset Trap Pos. FB":bool
  out "Trap Positions":waveform(dbl)[](graph)=[{"t0"=timestamp(12.90000000000001 s since 1904-01-01), "dt"=0.15, "Y"=[-1.7479351299698465e-12, -1.7479351299698465e-12], "attributes"=variant("NI_ChannelName"=variant(string "Trap 1 Pos."))}, {"t0"=timestamp(12.90000000000001 s since 1904-01-01), "dt"=0.15, "Y"=[6.991740519879386e-12, 6.991740519879386e-12], "attributes"=variant("NI_ChannelName"=variant(string "Trap 2 Pos."))}]
  in  "Tab Control 8":enum32{"Main Setting", "Details"}(tab)
  in  "Trap Pos FB Int Count":u16=100
  in  "Trap Pos. FB Gains":T11={"proportional gain (Kc)"=10.0, "integral gain (Kc*Ts/Ti)"=10.0, "derivative gain (Kc*Td/Ts)"=0.0} {"proportional gain (Kc)" format="%.11g"; "integral gain (Kc*Ts/Ti)" format="%.11g"; "derivative gain (Kc*Td/Ts)" format="%.11g"}
  in  "Trap Pos. FB Offset Factor":i64
  in  "Trap Pos FB Negate Action":bool
  in  "Trap Pos. FB Mult Factor":i64=33554432
  in  "Trap Pos. AI1 X Pre-scale":u16
  in  "Trap Pos. FB Range":T12={"output high"=0.999969482421875, "output low"=-1.0}
  out "Trap Pos FB Int Signal":fxp<+/-,24,9> format="%.18g"
  out "Trap Pos FB Int-Norm Signal":fxp<+/-,16,1> format="%.16g"
  in  "Set SP Using...":bool
  in  "Trap Pos FB Monitor\nT1 or T2":bool
  out "Trap X AI1 (DMA)":T13={"Set 1"=0.999969482421875, "Set 2"=0.999969482421875}
  in  "N El. to Ave.":dbl=10000.0
  out "Trap Pos FB Action":i64
  out "Action (%)":dbl(knob) scale=-100.0..100.0
  in  "Trap Pos. FB Out Scale 2^n":u8=23 caption="Action Scale"
  out "Mean T1 Position (nm)":dbl=-1.7479351299698465e-12 caption="Mean T1 (nm)" format="%0.2f"
  out "Trap 1 Position RMS (A)":dbl caption="RMS (Ang)"
  in  "Tab Control 3":enum32{"Timing", "MCL Scan", "Analog Out"}(tab)
  out "APD 2 Gate Late Counter":u32
  out "APD 2 Gate Relative Phase":i16
  in  "Phase Adj. (APD 2 Gate)":i16=20
  in  "Initial Phase Adjustment (APD 2 Gate)":i16=55
  out "APD 1 Gate Late Counter":u32
  in  "- phase (APD 1 Gate)":bool
  in  "+ phase (APD 1 Gate)":bool
  out "APD 1 Gate Relative Phase":i16
  in  "Phase Adj. (APD 1 Gate)":i16=20
  in  "Initial Phase Adjustment (APD 1 Gate)":i16=60
  in  "Save APD Data\nwith Trap Data":bool=TRUE
  out "APD FIFO Elements Remaining":u32
  in  "- phase (APD Acq)":bool
  in  "+ phase (APD Acq)":bool
  out "APD Acq Late Counter":u32
  out "APD Acq Relative Phase":i16
  in  "Phase Adj. (APD Acq)":i16=20
  in  "Initial Phase Adjustment (APD Acq)":i16
  in  "Invert APD Gate":bool caption="Invert Gate"
  in  "APD Gate OFF Count":u32=450 caption="Gate OFF Count"
  in  "APD Gate ON Count":u32=150 caption="Gate ON Count"
  in  "APD Gate":enum32{"ON", "OFF", "Interlace"}(radio)=enum."Interlace"
  in  "APD Integration Time (s)":dbl=0.01 caption="Integration Time (s)"
  out "APD Acq Rate (Hz)":dbl=100.0 caption="Rate (Hz)"
  out "APD Samples/FIFO Acq.":dbl=30.0
  out "APD Elements/DMA read":u32=60
  out "APD Int. Count":u32=400000 format="%.0p"
  in  "+ phase (APD 2 Gate)":bool
  in  "- phase (APD 2 Gate)":bool
  in  "Tab Control 5":enum32{"PSD X", "PSD Y", "Other Data Channel"}(tab)
  out "Data map":dbl[][](graph)
  in  "Channel":i32=4
  in  "Abort MCL Scan":bool
  out "MCL Scan I":u64
  out "MCL Scanning":bool
  in  "Start MCL Scan":bool
  out "wait to reset values":bool
  in  "Tab Control 4":enum32{"Scan Settings", "MCL FPGA Loop Timing"}(tab)
  out "Total Time (s)":dbl=48.0
  in  "Scan lines (y)":u64=20
  in  "Fast Scan Dir":bool=TRUE
  in  "2D or 1D Scan":bool=TRUE
  out "Initial X":dbl
  out "Initial Y":dbl
  out "Time/f+b scan (s) (MCL)":dbl=2.4 caption="Time/scan (s)"
  in  "Number of scans (MCL)":u64=1 caption="Scans"
  in  "Scan steps (MCL)":u64=40 caption="Scan steps (x)"
  in  "N APD Samp/step":dbl=3.0
  in  "Scan Range (V)\n(of steps)":dbl=3.5
  in  "Restart DMA? (MCL)":bool=TRUE caption="Restart DMA?"
  in  "Continuous MCL Scanning":bool caption="Cont. Scanning"
  in  "Center Scan":bool=TRUE
  in  "Save Data (MCL)":bool=TRUE caption="Save Data"
  out "Actual Incr. int (MCL)":i16=294 caption="Incr. int"
  out "Desired incr (int)":dbl=294.0628205128205
  out "Desired Scan Incr (V)":dbl=0.08974358974358974
  out "N sets should be saved (MCL)":dbl=160.0 caption="N sets should be saved"
  out "Data points/scans (MCL)":dbl=4800.0 caption="Data points/scans"
  out "Data points/scan (f+b)":dbl=240.0 caption="points/scan (f+b)"
  out "Cycles/step (MCL)":u64=2000 caption="Cycles/step" format="%.0p"
  out "Actual MCL Inc (V)":dbl=0.08972441785943175
  in  "Phase adjust (MCL)":i16 caption="Phase adjust"
  out "Relative Phase (MCL)":i16 caption="Relative Phase"
  in  "Initial Phase Adj. (MCL)":i16 caption="Initial Phase Adj."
  in  "Update Count (MCL)":u32=600
  in  "+ phase (MCL)":bool
  in  "- phase (MCL)":bool
  out "MCL Late Counter":u32
  in  "APD 1 AO Mult.":i16=1 min=1
  in  "APD 2 AO Mult.":i16=1 min=1
  in  "Tab Control 7":enum32{"Green FB Signals", "Slow MCL Scan"}(tab)
  out "Green FB Plot":dbl(graph)=10.0
  out "MCL Scan 2":cluster{"Begin (V)":dbl, dbl, dbl[]}(graph)
  out "MCL Scan":cluster{"Begin (V)":dbl, dbl, dbl[]}(graph)
  in  "Green laser mode":enum32{"Laser ON", "Laser OFF", "Interlace"}(radio)
  in  "GI Frequency, ON count":u32=150 min=1 step=1
  in  "Invert GI":bool
  out "GI Late Counter":u32
  in  "Phase adj. (GI)":i16=5
  out "GI relative phase":i16
  in  "+ phase (GI)":bool
  in  "Initial Phase Adjustment (GI)":i16=19
  in  "GI Frequency, OFF count":u32=450 min=1 step=1
  in  "- phase (GI)":bool
  out "Green FB Signals (V)":cluster{"Y":dbl, "X":dbl, "Sum":dbl}={"Y"=1.0, "X"=1.0, "Sum"=10.0}
  out "Relative phase (Green FB)":i16
  in  "+ phase (Green FB)":bool
  in  "- phase (Green FB)":bool
  in  "Green FB Count":u32=600
  in  "Phase adj. (Green FB)":i16=10
  in  "Initial Phase Adjustment (Green FB)":i16=50
  in  "Green FB On/Off":bool
  in  "Current When FB OFF (%)":dbl=10.0 min=0.0 max=100.0 step=1.0
  in  "Green int current ON count adj":u32=150
  in  "Green FB Gains":T14={"proportional gain (Kc)"=10, "integral gain (Kc*Ts/Ti)"=5, "derivative gain (Kc*Td/Ts)"=0}
  in  "Green FB Setpoint (mV)":dbl=100.0
  in  "- phase (GI) 2":bool
  in  "Initial Phase Adjustment (GI) 2":i16=-100
  in  "+ phase (GI) 2":bool
  out "GI relative phase 2":i16
  in  "Phase adj. (GI) 2":i16=20
  out "GI Late Counter 2":u32
  in  "Trap Position FIFO Depth":u32=300000 format="%.0p"
  in  "# Samples/trap":u32=20000 format="%.0p"
  out "Trap AI Elements/DMA read":u32=320000 format="%.0p"
  out "Ave. Rate (Hz)":dbl=200000.0 format="%#_6p"
  out "Trap AI FIFO El. Rem.":u32 format="%.0p"
  in  "Phase adj. (AI1)":i16
  out "Relative phase (AI1)":i16
  in  "+ phase (AI1)":bool
  in  "- phase (AI1)":bool
  out "Late Counter (AI1)":u32
  in  "Initial Phase Adjustment (AI1)":i16=180
  out "AI rate (Hz)":dbl=200000.0 format="%#_6p"
  in  "AI Count (ticks)":u32=200
  out "# Samples/channel":u32=40000 format="%.0p"
  in  "Trap AI FIFO Depth":u32=340000 format="%.0p"
  in  "Detector Type":string(combo)="UCB Fleezers 052511"
  in  "N Acq Sets (Traps + Fl.)":i16=3
  in  "Sets to FIFO (Traps)":T15={"Set 1"=TRUE, "Set 2"=TRUE, "Set 3"=FALSE}
  in  "FPGA Ave.":dbl=1.0 min=1.0 step=1.0
  out "Ave. Period (s)":dbl=5e-06 format="%#_6p"
  out "DMA Update Period (s)":dbl=0.3
  out "FPGA Averaging":bool
  out "Trap Sets":u32=2
  out "Counts/DMA":dbl=12000000.0 format="%#_6p"
  out "Trap Pos FIFO El Remaining":u32=141
  out "Trap Pos Elements/DMA read":u32=120000 format="%.0p"
  out "Trap AI FIFO Timeout":u16
  out "Trap Pos FIFO Timeout":u16
  out "Waveform Chart":i32(graph)=320000
  out "error out 2":errorcluster
  in  "Lost Tether Alarm Threshold (pN)":dbl=0.5
  in  "AOM X Cal (nm/MHz)":dbl=168.33
  in  "MCL X Cal (nm/V)":dbl=1070.0
  out "X RF Amplitude Limits (%)":T16={"Minimum"=0.0, "Maximum"=50.0, "Increment"=1.0}
  out "X RF Frequency Limits (MHz)":T16={"Minimum"=50.0, "Maximum"=100.0, "Increment"=1.0}
  out "Y RF Frequency Limits (MHz)":T16={"Minimum"=50.0, "Maximum"=100.0, "Increment"=1.0}
  out "Y RF Amplitude Limits (%)":T16={"Minimum"=0.0, "Maximum"=50.0, "Increment"=1.0}
  in  "Manip. X?":bool=TRUE
  in  "Manip. Y?":bool
  in  "Force Manip Abort":bool
  out "Read cal error":errorcluster
  in  "DAQ Delay (ms)":u32=1000
  in  "Start Scan":bool
  in  "Scan axis":bool
  in  "Osc. amp. (V)":dbl=5.0
  in  "Osc. center (V)":dbl=5.0
  in  "Osc. freq. (Hz) 2":dbl=1.0
  in  "MCL Mode":u16(ring) items=["Manual Positioning", "Sinusoidal Wave", "Linear Scan"]
  in  "Begin (V)":dbl
  in  "End (V)":dbl=10.0
  in  "N Points":dbl=20.0
  in  "Delay to Interlace (s)":dbl
  in  "Delayed Interlace Start":bool
  in  "Read Lateness and Rel Phase":bool
  out "Vec Mean of T1 T2":dbl[](array[numeric])=[nan, nan]
  in  "Cal read wait (s)":u32=5
  out "Time tether formed":timestamp=timestamp(3371146929.513132 s since 1904-01-01)
  in  "Chemyx Syringe Pump Serial Port":refnum<visa-resource-name>="ASRL3::INSTR"
  in  "Limit Min (MHz)":dbl=10.0 caption="Min (MHz)"
  in  "Limit Max (MHz)":dbl=16.0 caption="Max (MHz)"
  in  "Limits Enable":bool=TRUE caption="Enable"
  out "AI labels":string[](array[string])=["T1 Y", "T1 X", "T1 Sum", "T2 Y", "T2 X", "T2 Sum", "T1 FB X", "T2 FB Sum", "T2 FB X", "T2 FB Sum", "PSD Y", "PSD X", "PSD Sum"]
  in  "Save Trap Pos. Data":bool=TRUE
  in  "ESP Port":refnum<visa-resource-name>="COM22"
  in  "Locations":i32(listbox)=1
  out "Selected Location":cluster{"x":string, "y":string, "z":string}={"x"="0.19233\r\n", "y"="0.00156\r\n", "z"="0.20615\r\n"}
  in  "Capture":bool
  in  "Save":bool
  in  "Goto Top (F6)":bool
  in  "Goto Exp (F8)":bool
  in  "Goto Bottom (F7)":bool
  in  "Axis 3":string="0.00500\r\n"
  in  "Axis 2":string="0.00500\r\n"
  in  "Axis 1":string="0.00500\r\n"
  in  "Axis 3":string="0.20000\r\n"
  in  "Axis 2":string="0.20000\r\n"
  in  "Axis 1":string="0.20000\r\n"
  in  "Activate Joystick":bool
  in  "ESP ZL-Limit":string="-0.09900"
  in  "ESP ZR-Limit":string="0.09900"
  out "Z Pos Pos":string="0.21899\r\n"
  out "Y Pos":string="0.00713\r\n"
  out "X Pos":string="0.20503\r\n"
  in  "error in":errorcluster
  out "error out":errorcluster
  out "Z motion":string
  out "Y Motion":string
  out "X Motion":string
  # "After"
  # "During"
  # "Trap On?"
  # "BD Flow ON?"
  # "Samp Flow ON?"
  # "1"
  # "2"
  # "Trap Display:"
  # "APD Display:"
  # "originally 10k"
  # "Trap Manipulation"
  # "DAQ"
  # "Data Saving"
  # "F9"
  # "Bead Calibration"
  # "F10"
  # "F4"
  # "Press F12 to move stage\nwith the mouse. F12 to cancel."
  # "F5"
  # "F6"
  # "F7"
  # "F8"
  # "Harvard Pump\n(sample channel for flow exp)"
  # "Chemyx Pump 2"
  # "Units: \n1 = ml/m\n2 = ml/h\n3 = ul/m\n4 = ul/h"
  # "Rate param is ul/h\nVolume param is ul"
  # "X"
  # "Y"
  # "Oscillate Set 2 freq. (debugging)"
  # "BD 1"
  # "BD 2"
  # "AOD Raster Scan"
  # "Approx. trap separations"
  # "X"
  # "Y"
  # "DON'T TURN ON\nUNTIL YOU CLOSE\nTHE LOOP"
  # "FPGA\nreading"
  # "DMA\ntransfer"
  # "APD Gates"
  # "APD 2"
  # "APD 1"
  # "X"
  # "2D"
  # "Y"
  # "1D"
  # "Green Laser Interlacing"
  # "Green FB Measurement"
  # "Digital Gate"
  # "Current Analog Control"
  # "was 87"
  # "originally 600k"
  # "Total AI Rates (NOT rates/trap)"
  # "originally 20k"
  # "(Samples/trap x Trap Sets)"
  # "(Samples/channel x\n8 if averaging (8 channels)\n4 if no averaging)"
  # "Trap 1"
  # "Trap 2"
  # "Flour./Trap 3"
  # "External Video Window"
  # "MCL Position Debugging"
  # "Temporary Control Storage\n(these used to be somewhere else, still want to keep them)"
  # "Y"
  # "X"
  # "Trap Position Difference Limits"
  # "Joystick Control"
  # "Setting Limit for the z-axis"
  # "Current Location"
  # "Save Positions of Cambers"
  # "Errors detected in determing Current Location"
  # "High Jog Velocity"
  # "Low Jog Velocity"
  # "Select the chamber to go to"
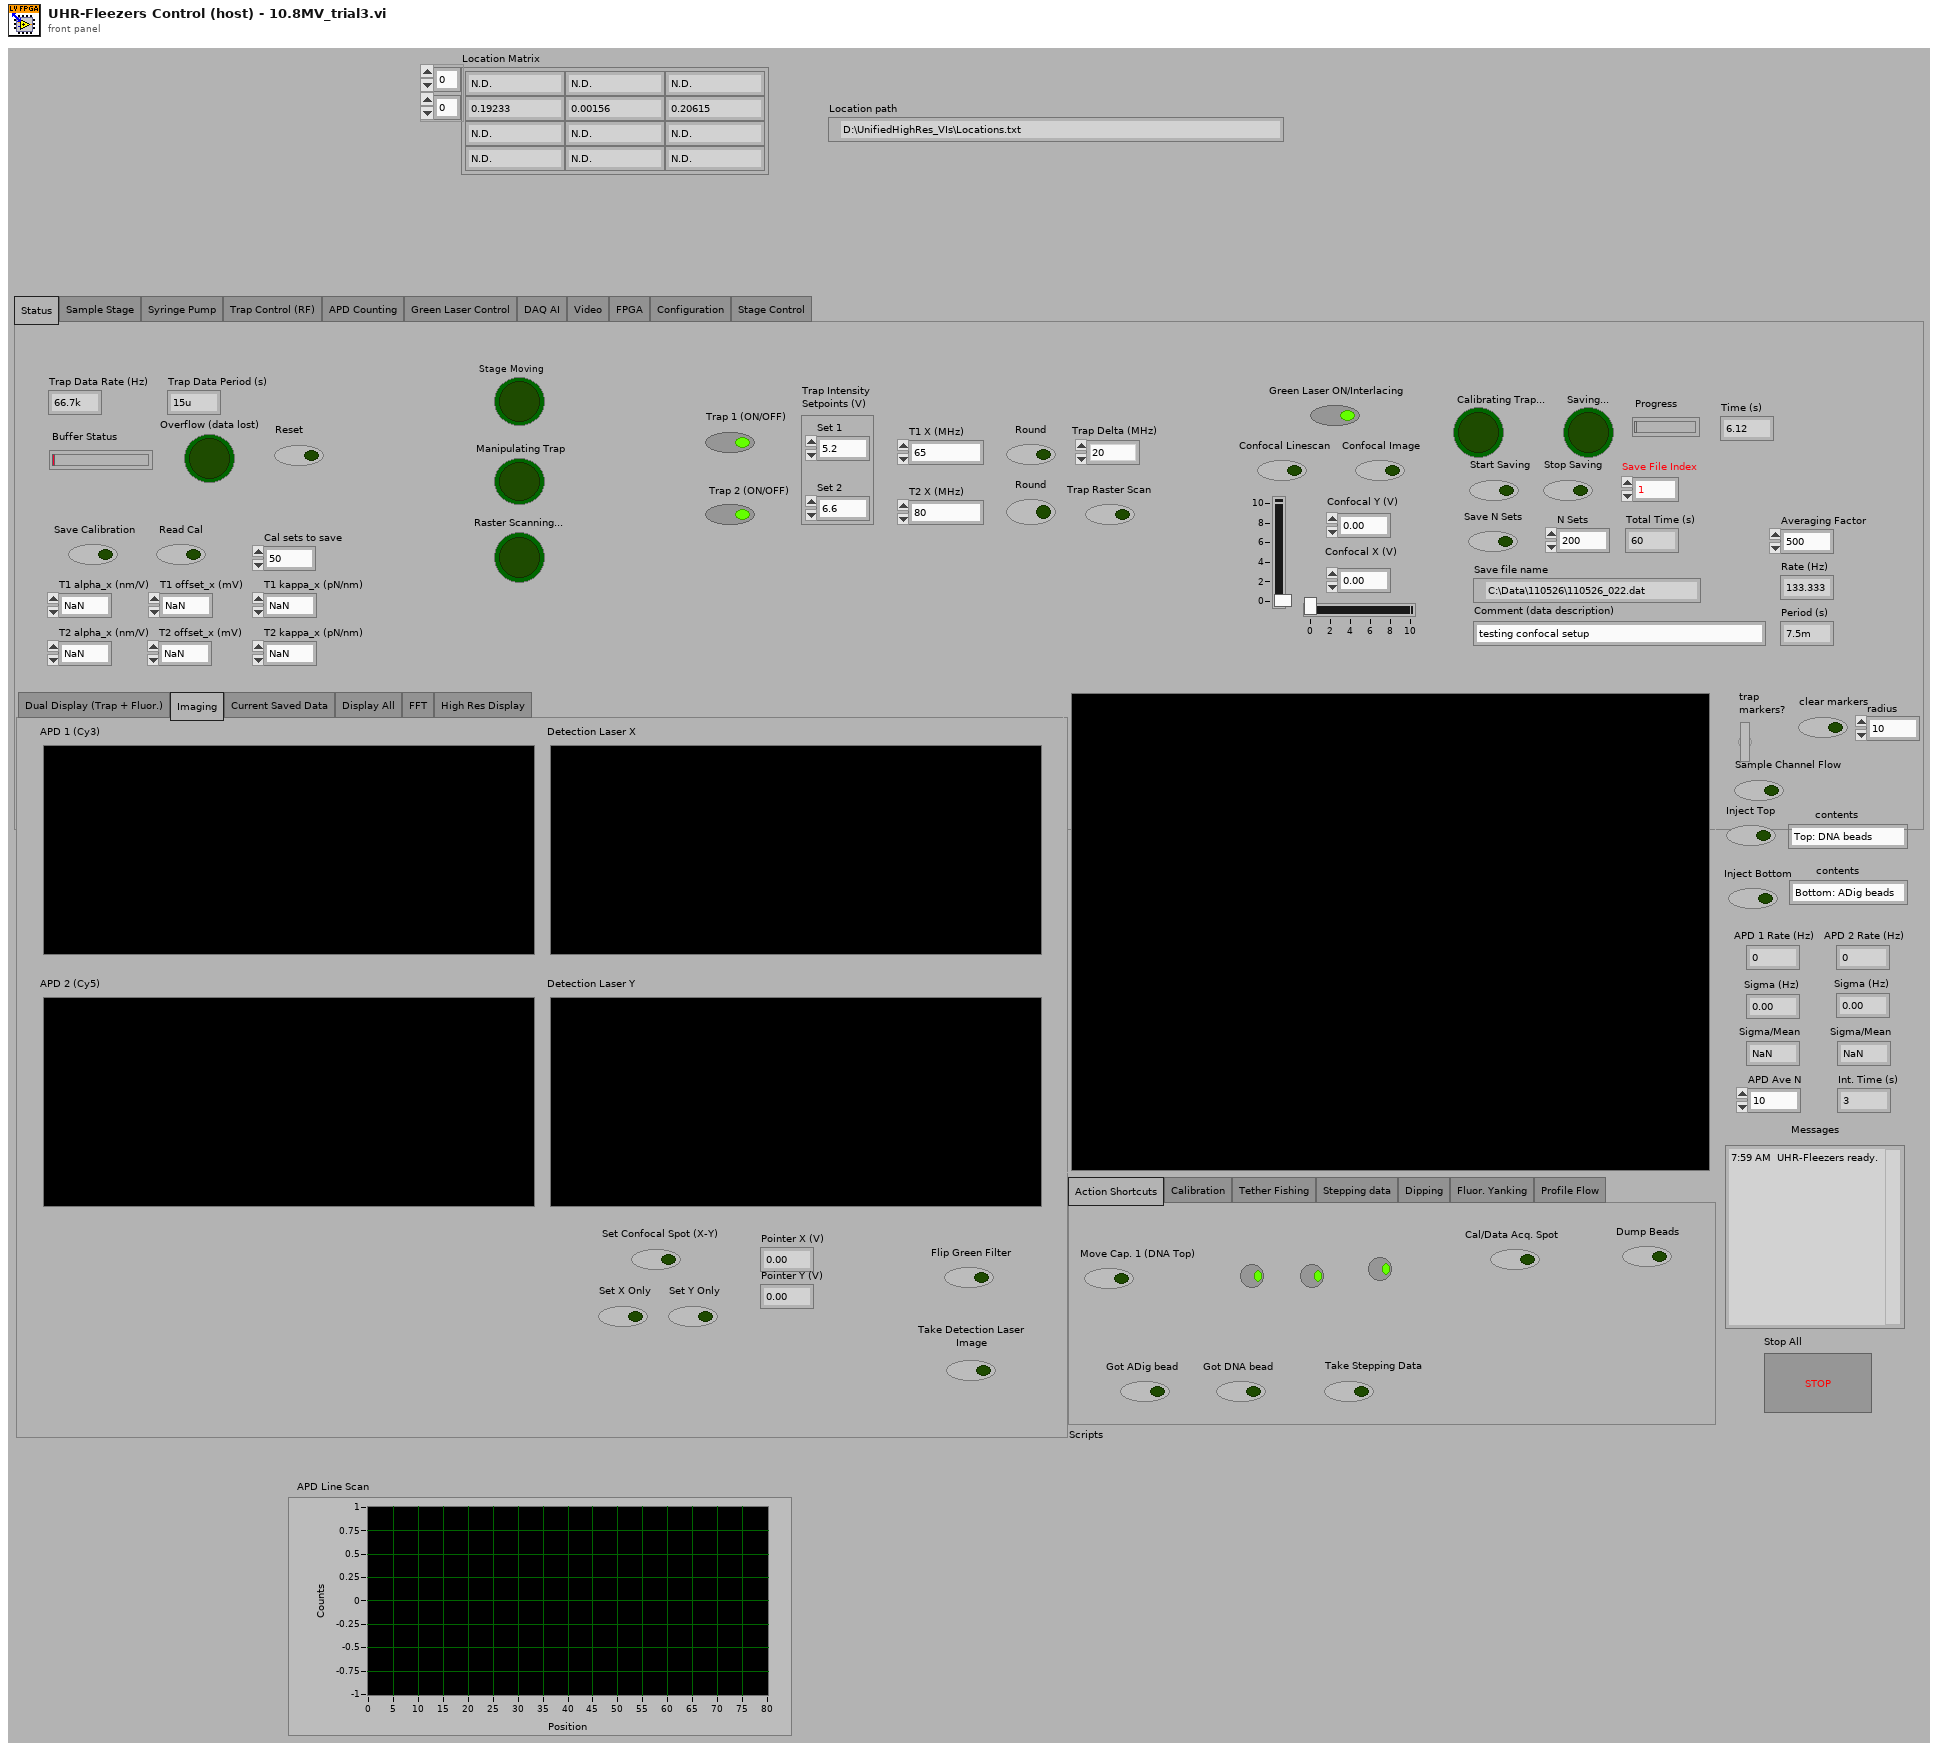
[diagram p1: front panel]
types:
  T1 = enum32{"Action Shortcuts", "Calibration", "Tether Fishing", "Stepping data", "Dipping", "Fluor. Yanking", "Profile Flow"}
  T2 = typedef "IMAQ Image.ctl" = refnum<image>
  T3 = enum32{"Dual Display (Trap + Fluor.)", "Imaging", "Current Saved Data", "Display All", "FFT", "High Res Display"}
  T4 = enum32{"Status", "Sample Stage", "Syringe Pump", "Trap Control (RF)", "APD Counting", "Green Laser Control", "DAQ AI", "Video", "FPGA", "Configuration", "Stage Control"}
  T5 = cluster{"Pump 1":cluster{"Diameter (mm)":dbl, "Units":dbl, "Volume":dbl, "Rate":dbl}, "Pump 2":cluster{"Diameter (mm)":dbl, "Units":dbl, "Volume":dbl, "Rate":dbl}, "Pump 3":cluster{"Diameter (mm)":dbl, "Units":dbl, "Volume":dbl, "Rate":dbl}}
  T6 = enum32{"IR Laser Interlacing (Direct RF Board Control Method)", "AOD Raster Scan", "Feedback on Trap Intensity", "Feedback on Trap Position"}
  T7 = typedef "LVPoint32TypeDef.ctl" = cluster{"Horizontal":i32, "Vertical":i32}
  T8 = cluster{"Scan Range AOD (nm) 2":dbl, "Step Size AOD (nm) 2":dbl, "Scan Speed AOD (nm/s) 2":dbl, "Number of scans (AOD) 2":u16, "Label":string}[]
  T9 = cluster{"Set 1":cluster{"proportional gain (Kc)":i16, "integral gain (Kc*Ts/Ti)":i16, "derivative gain (Kc*Td/Ts)":i16}, "Set 2":cluster{"proportional gain (Kc)":i16, "integral gain (Kc*Ts/Ti)":i16, "derivative gain (Kc*Td/Ts)":i16}}
  T10 = cluster{"Trap 1":fxp<+/-,16,1>, "Trap 2":fxp<+/-,16,1>}
  T11 = cluster{"proportional gain (Kc)":fxp<+/-,16,8>, "integral gain (Kc*Ts/Ti)":fxp<+/-,16,8>, "derivative gain (Kc*Td/Ts)":fxp<+/-,16,8>}
  T12 = cluster{"output high":fxp<+/-,16,1>, "output low":fxp<+/-,16,1>}
  T13 = cluster{"Set 1":fxp<+/-,16,1>, "Set 2":fxp<+/-,16,1>}
  T14 = cluster{"proportional gain (Kc)":i16, "integral gain (Kc*Ts/Ti)":i16, "derivative gain (Kc*Td/Ts)":i16}
  T15 = cluster{"Set 1":bool, "Set 2":bool, "Set 3":bool}
  T16 = typedef "LVMinMaxIncTypeDef.ctl" = cluster{"Minimum":dbl, "Maximum":dbl, "Increment":dbl}
  T17 = typedef "Image Type" = u32
  T18 = typedef "nirio_resource_hc.ctl" = tag
  T19 = typedef "openfpgaref.8.6.ctl" = refnum<k20>
  T20 = enum16{"CONNECT", "INITIALIZE VALVES", "DISCONNECT", "MOVE VALVE"}
  T21 = cluster{"New Image":T2, "New Image":T2, "New Image":T2, "New Image":T2}
  T22 = cluster{"Location Matrix[0]":string, "Location Matrix[1]":string, "Location Matrix[2]":string}
  T23 = enum16{"open", "replace", "create", "open or create", "replace or create", "replace or create with confirmation"}
  T24 = typedef "XDNodeRunTimeDep.lvlib/timing_clust.ctl" = cluster{"Expected End [f-1]":u64, "Actual End [f-1]":u64, "Finished Late? [f-1]":bool, "Expected End [i-1]":u64, "Actual End [i-1]":u64, "Finished Late? [i-1]":bool, "Expected Start [i]":u64, "Actual Start [i]":u64, "Expected Start [f]":u64, "Actual Start [f]":u64, "Source Name":string, "Structure Name":string, "Period":i64, "Deadline":i64, "Offset":i64, "Start":i64, "Priority":i32, "Timeout":i32, "Mode":T25, "Wakeup Reason":T26, "Error":errorcluster, "Source Type":string, "Secondary Source Type":string, "Global End Time":u64, "Global Start Time":u64, "Frame Duration":u64, "Iteration Duration":u64, "Assigned CPU":i32, "I/O Scan Engine Mode":u32}
  T25 = typedef "XDNodeRunTimeDep.lvlib/nitl_modes.ctl" = enum32{"No Change", "Process missed periods, maintain original phase", "Discard missed periods, maintain original phase", "Process missed periods, ignore original phase", "Discard missed periods, ignore original phase"}
  T26 = typedef "XDNodeRunTimeDep.lvlib/wakeup.ctl" = enum32{"Normal", "Aborted", "Asynchronous wakeup", "Timing source error", "Timed loop error", "Timeout"}
  T27 = cluster{"[0]":i32, "[1]":i32, "[2]":i32, "[3]":i32}
  T28 = cluster{"[0]":i32, "[1]":i32, "[2]":i32, "[3]":i32}[]
  T29 = enum16{"big-endian, network order", "native, host order", "little-endian"}
  T30 = cluster{"Scan Range AOD (nm) 2":dbl, "Step Size AOD (nm) 2":dbl, "Scan Speed AOD (nm/s) 2":dbl, "Number of scans (AOD) 2":u16, "Label":string}
  T31 = cluster{"[0]":dbl, "[1]":dbl, "[2]":dbl, "[3]":dbl, "[4]":dbl, "[5]":dbl}
  T32 = cluster{"Diameter (mm)":dbl, "Units":dbl, "Volume":dbl, "Rate":dbl}
  T33 = cluster{"Left":i32, "Top":i32, "Width":u32, "Height":u32}
  T34 = cluster{cluster{"Left":i32, "Top":i32, "Width":u32, "Height":u32}}[]
  T35 = enum32{"Normal Display", "Dual Display (APD)", "FFT", "High Res Display"}
  T36 = cluster{"Origin Pixel":cluster{"X":sgl, "Y":sgl}, "Angle Relative to Horizontal (deg)":sgl, "Axis Reference":u32}
  T37 = typedef "Simple Grid Descriptor" = cluster{"X Step":sgl, "Y Step":sgl, "Unit":T38}
  T38 = typedef "Image Unit" = enum32{"Undefined", "Angström", "Micrometer", "Millimeter", "Centimeter", "Meter", "Kilometer", "Microinch", "Inch", "Feet", "Nautical miles", "Standard miles", "Steps"}
  T39 = cluster{"averaging mode":u16, "weighting mode":u16, "number of averages":u32}
  T40 = cluster{"dB On (F)":bool, "unwrap phase (F)":bool, "convert to degree (F)":bool}
  T41 = cluster{string, string, string, string, string, string, string, string}
  T42 = cluster{string, string, string, string, string, string, string, string, string, string, string, string}
  T43 = cluster{string, string, string, string, string, string, string, string, string, string, string, string, string}
  T44 = cluster{string, string, string, string, string, string, string, string, string, string, string, string, string, string}
  T45 = cluster{"BD 1 Frequency 1 (MHz)":dbl, "BD 1 Frequency 2 (MHz)":dbl}
  T46 = cluster{"f0":dbl, "df":dbl, "magnitude":dbl[]}[][]
  T47 = cluster{"Green FB Ch 0":i16, "Green FB Ch 1":i16, "Green FB Ch 2":i16}
  T48 = cluster{"Green FB Ch 0":dbl, "Green FB Ch 1":dbl, "Green FB Ch 2":dbl}
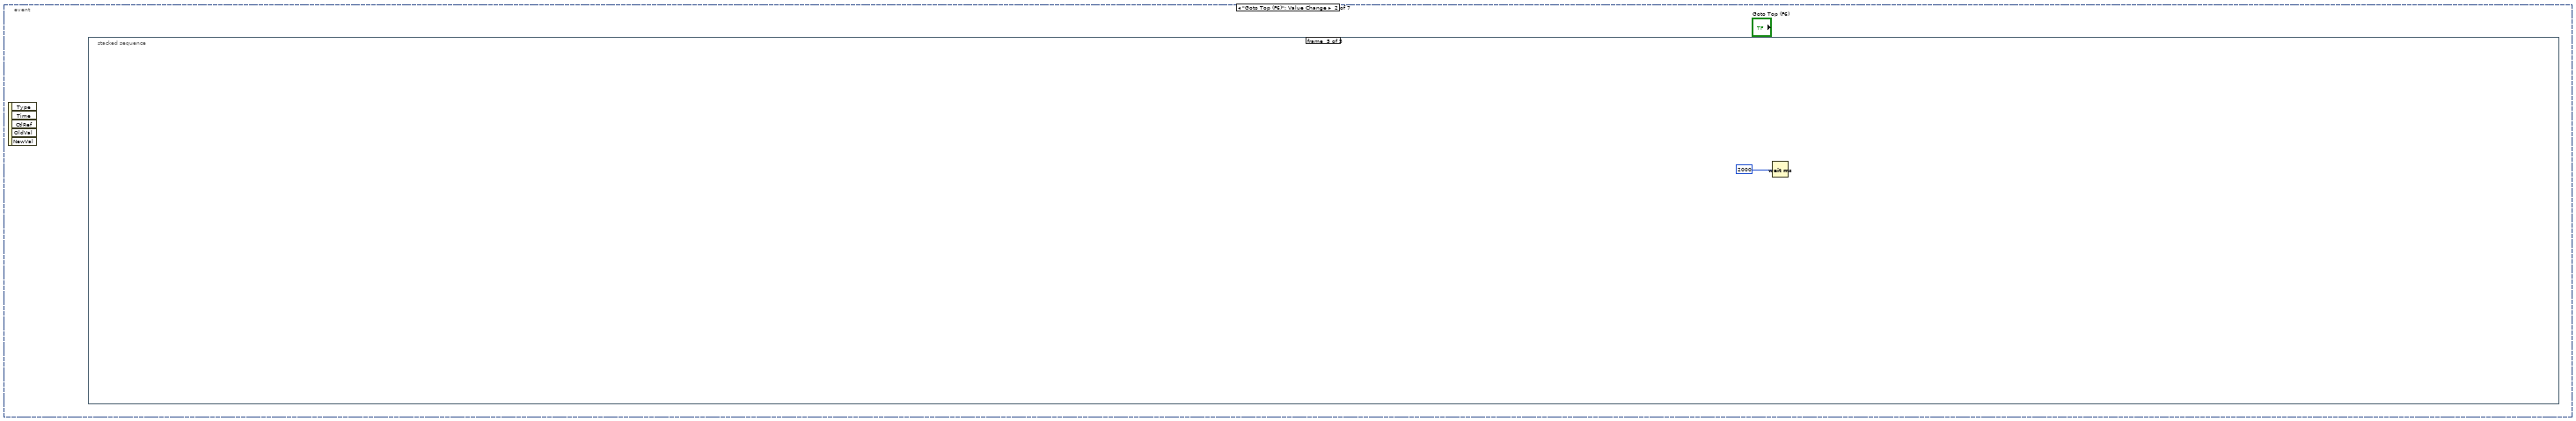
[diagram p4: hidden frame]
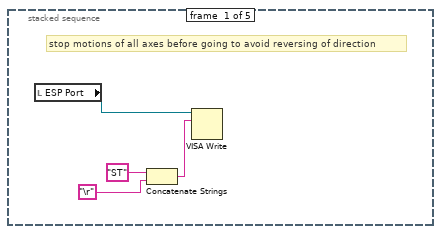
[diagram p5: hidden frame]
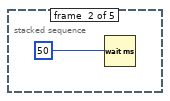
[diagram p6: hidden frame]
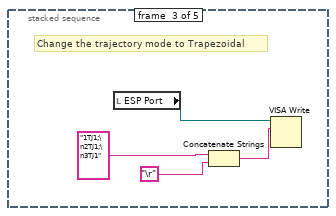
[diagram p7: hidden frame]
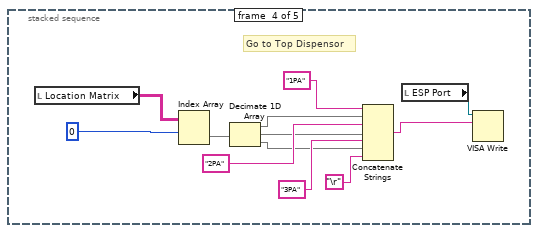
[diagram p8: hidden frame]
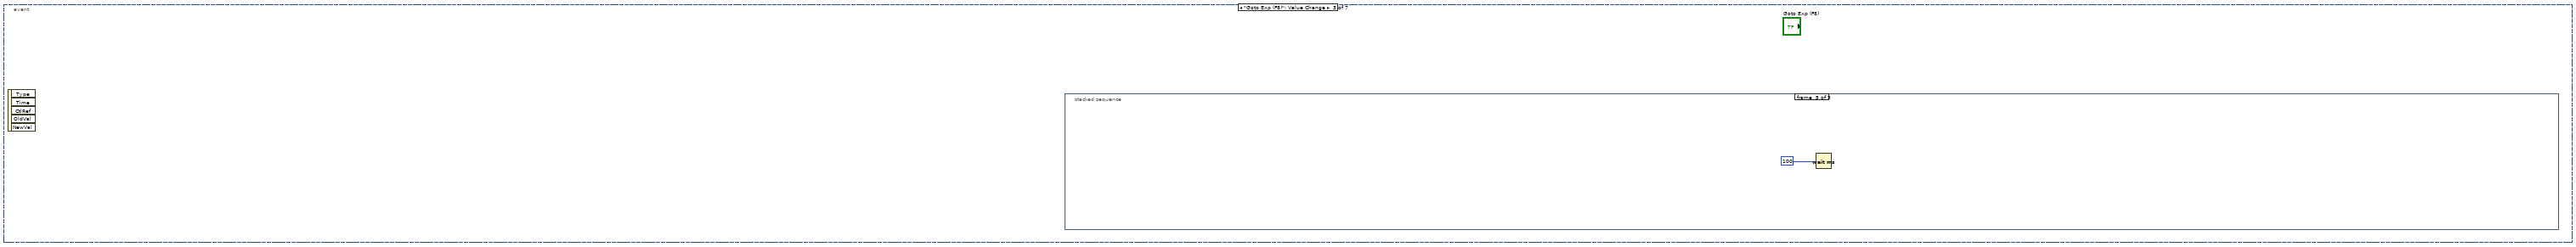
[diagram p9: hidden frame]
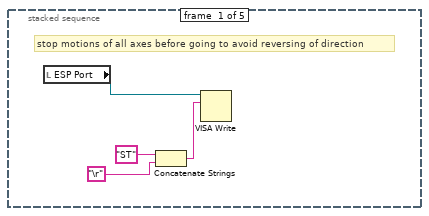
[diagram p10: hidden frame]
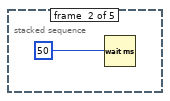
[diagram p11: hidden frame]
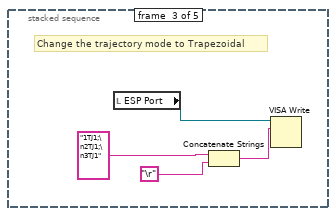
[diagram p12: hidden frame]
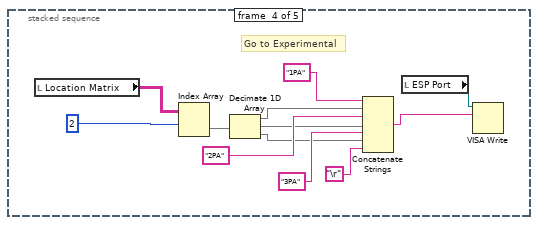
[diagram p13: hidden frame]
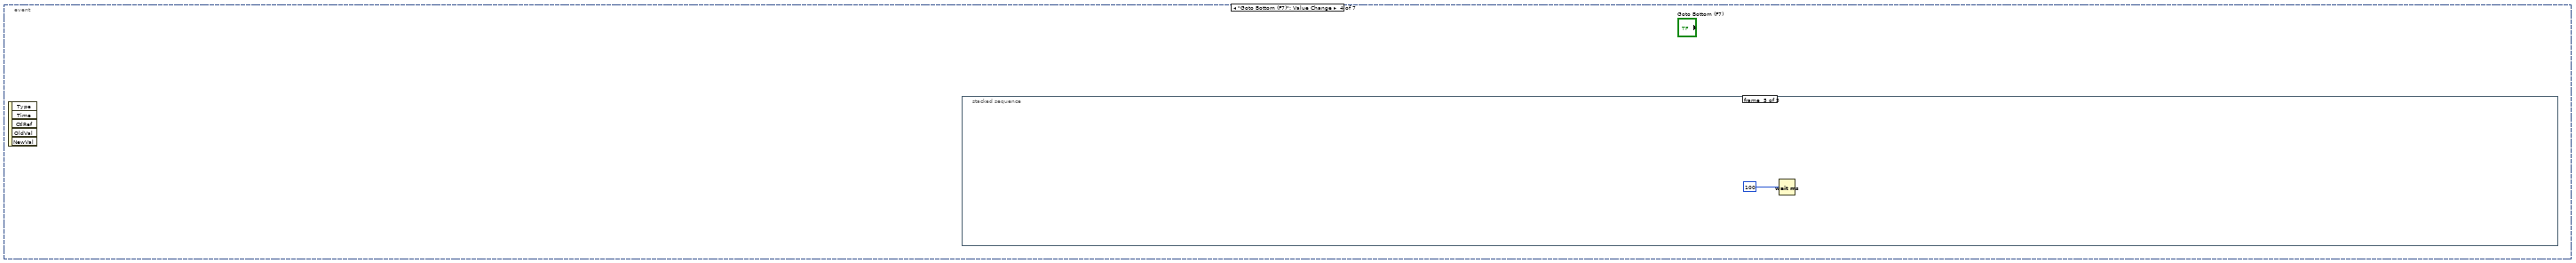
[diagram p14: hidden frame]
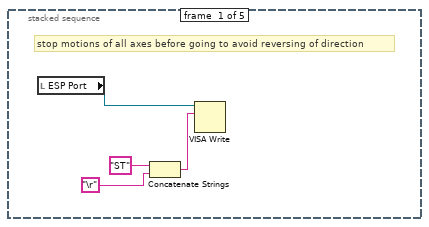
[diagram p15: hidden frame]
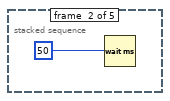
[diagram p16: hidden frame]
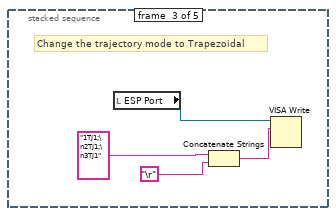
[diagram p17: hidden frame]
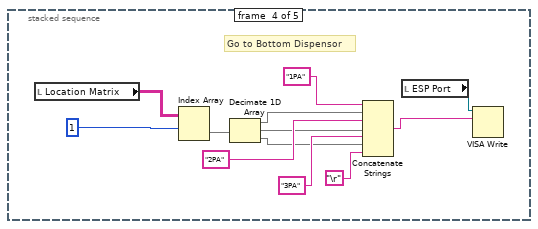
[diagram p18: hidden frame]
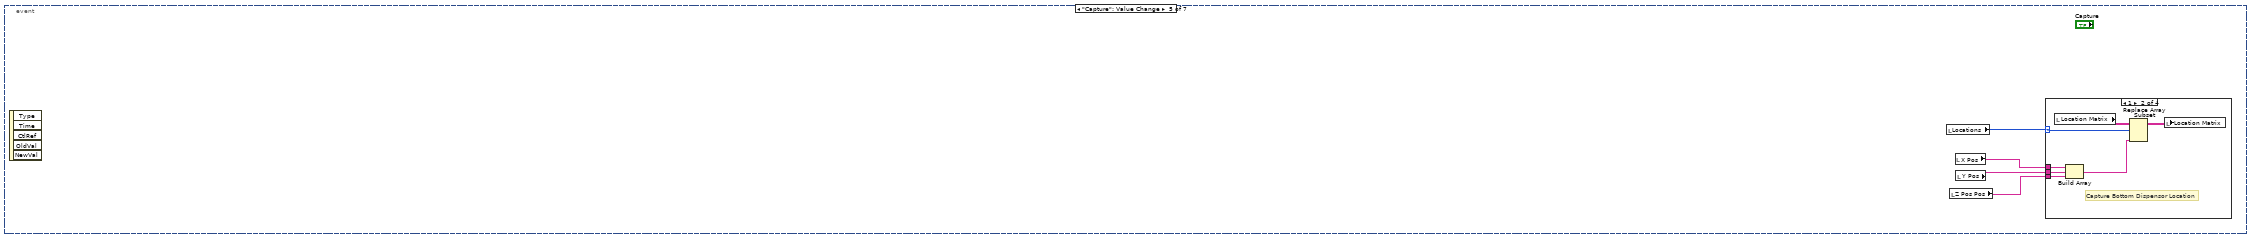
[diagram p19: hidden frame]
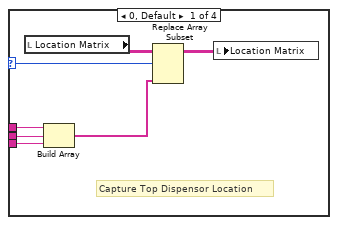
[diagram p20: hidden frame]
diagram:
  w64 = T17 2 items=["Grayscale (U8)", "Grayscale (I16)", "Grayscale (SGL)", "Complex (CSG)", "RGB (U32)", "HSL (U32)", "RGB (U64)", "Grayscale (U16)"] ("Image Type")
  w121 = cluster{"output high":i16, "output low":i16} {"output high"=3000, "output low"=0} ("FB output range 1")
  w196 = 10.0 ("y")
  w195 = 32767.0 ("y")
  w211 = 6.0  # clock mult.
  w212 = 49152000.0  # TCXO frequ.
  # "Initialize location matrix"
  n1 = Build Array("DIO count 1 (ticks)", "DIO count 2 (ticks)", "DIO count 3 (ticks)") -> (w110:u32[])
  n2 = Multiply(x="APD Integration Time (s)", y=40000000.0) -> (x*y=w128:dbl)
  n3 = Reciprocal(x="APD Integration Time (s)") -> (1/x=w125:dbl)
  n4 = local write "APD Acq Rate (Hz)"(w125) -> ()
  n5 = local read "AO1"() -> (w190:dbl)
  n6 = local read "AO2"() -> (w189:dbl)
  n7 = To Unsigned Long Integer(number=w128) -> (unsigned 32bit integer=w127:u32)
  "APD Int. Count" <- w127
  n8 = local read "Scan Increment (MHz)"() -> (w207:dbl)
  n9 = local read "Continuous MCL Scanning"() -> (w177:bool)
  n10 = local read "Fast Scan Dir"() -> (w176:bool)
  n11 = local read "Trap Intensity\nSetpoints (V)"() -> (w226:cluster{"Set 1":dbl, "Set 2":dbl})
  n12 = local read "Number of scans (MCL)"() -> (w178:u64)
  n13 = Multiply(x=w190, y=w195) -> (x*y=w192:dbl)
  n14 = Multiply(x=w189, y=w195) -> (x*y=w194:dbl)
  n15 = Divide(x=w192, y=w196) -> (x/y=w191:dbl)
  n16 = Divide(x=w194, y=w196) -> (x/y=w193:dbl)
  n17 = To Word Integer(number=w191) -> (16bit integer=w188:i16)
  n18 = To Word Integer(number=w193) -> (16bit integer=w187:i16)
  n19 = Not(x=w176) -> (.not. x?=w171:bool)
  n20 = local read "Cycles/step (MCL)"() -> (w179:u64)
  n21 = Multiply(x=w207, y=1000.0) -> (x*y=w214:dbl)
  n22 = local read "Scan steps (MCL)"() -> (w180:u64)
  n23 = local write "Trap Pos FIFO Timeout"(u16 0 ("Trap Pos FIFO Timeout")) -> ()
  n24 = local read "Desired Scan Incr (V)"() -> (w182:dbl)
  n25 = Scale By Power Of 2(n=48, x=w214) -> (x*2^n=w215:dbl)
  n26 = Multiply(x=w212, y=w211) -> (x*y=w210:dbl)
  n27 = Divide(x=w215, y=w210) -> (x/y=w209:dbl)
  n28 = local read "Number Interlace Sets"() -> (w103:u8)
  n29 = Split 1D Array(array=w110, index=w103) -> (first subarray=w112:u32[])  [unwired: 1 out]
  n30 = Add Array Elements(numeric array=w112) -> (sum=w111:u32)
  n31 = property on="AI Count (ticks)" class="DigNum (strict)"("Val(Sgnl)"="AI Count (ticks)") -> ()  [unwired: 2 in, 2 out]
  n32 = local read "# Samples/channel"() -> (w199:u32)
  n33 = local read "Number of F/B Scans (AOD)"() -> (w200:u16)
  n34 = To Quad Integer(1:w209) -> (0:w206:i64)
  n35 = local read "Not-Interlacing Set"() -> (w102:enum32{"Set 1", "Set 2", "Set 3"})
  n36 = To Unsigned Byte Integer(number=w102) -> (unsigned 8bit integer=w108:u8)
  n37 = Index Array(array=w110, index=w108) -> (element=w109:u32)
  n38 = local read "Feedback On/Off"() -> (w229:cluster{"Set 1":bool, "Set 2":bool})
  n39 = local read "PID Gains"() -> (w221:T9)
  n40 = Divide(x=40000000.0, y="AI Count (ticks)") -> (x/y=w168:dbl)
  n41 = Multiply(x=w182, y=32767.0) -> (x*y=w184:dbl)
  n42 = local read "Scan steps (AOD)"() -> (w205:u64)
  n43 = local read "All FB On/Off"() -> (w230:bool)
  n44 = local read "Cycles/step (AOD)"() -> (w204:u64)
  n45 = local write "AI rate (Hz)"(w168) -> ()
  n46 = Divide(x=w184, y=10.0) -> (x/y=w183:dbl)
  n47 = Multiply(x=w205, y=w204) -> (x*y=w203:u64)
  n48 = Multiply(x=3276.7, y=w226) -> (x*y=w225:cluster{"Set 1":dbl, "Set 2":dbl})
  n49 = To Word Integer(number=w183) -> (16bit integer=w181:i16)
  n50 = Multiply(x=w203, y=u64 2) -> (x*y=w201:u64)
  n51 = local read "Sets to FIFO (Traps)"() -> (w233:T15)
  n52 = Divide(x=w168, y="FPGA Ave.") -> (x/y=w169:dbl)
  n53 = To Word Integer(number=w225) -> (16bit integer=w224:cluster{"Set 1":i16, "Set 2":i16})
  n54 = xnode "Open FPGA VI Reference"("resource name"=T18 "750kHzDAQ") -> ("FPGA VI Reference Out"=w218:T19)  [unwired: 1 in, 1 out]
  n55 = Unbundle By Name(w221) -> ("Set 1"=w220:T14, "Set 2"=w219:T14)
  n56 = Multiply(x=w201, y=w200) -> (x*y=w198:u64)
  n57 = local write "Ave. Rate (Hz)"(w169) -> ()
  n58 = Divide(x=w198, y=w199) -> (x/y=w197:dbl)
  n59 = Unbundle By Name(w224) -> ("Set 1"=w223:i16, "Set 2"=w222:i16)
  n60 = local read "2D or 1D Scan"() -> (w122:bool)
  n61 = local write "Data points/scans"(w198) -> ()
  n62 = local read "Scan BD"() -> (w216:bool)
  n63 = And(x=w229, y=w230) -> (x .and. y?=w228:cluster{"Set 1":bool, "Set 2":bool})
  n64 = local write "Data points/scan (f/b)"(w201) -> ()
  n65 = Reciprocal(x=w169) -> (1/x=w170:dbl)
  n66 = local read "N Acq Sets (Traps + Fl.)"() -> (w161:i16)
  n67 = local write "N sets should be saved"(w197) -> ()
  n68 = Unbundle By Name(w228) -> ("Set 1"=w232:bool, "Set 2"=w231:bool)
  n69 = local read "Interlace"() -> (w104:bool)
  n70 = Select(t=w111, s=w104, f=w109) -> (s? t:f=w101:u32)
  n71 = local write "Update Count (MCL)"(w101) -> ()
  n72 = local write "Total Counts (ticks)"(w101) -> ()
  n73 = xnode "Invoke Method"("FPGA VI Reference In"=w218) -> ("FPGA VI Reference Out"=w120:T19, "error out"=w139:errorcluster)  [unwired: 1 in]
  n74 = local write "Ave. Period (s)"(w170) -> ()
  n75 = property on="2D or 1D Scan" class="Bool (strict)"("Val(Sgnl)"=w122) -> ()  [unwired: 2 in, 2 out]
  n76 = xnode "Read/Write Control"("FPGA VI Reference In"=w119, "error in"=w139, "ai count"="AI Count (ticks)", "Interlace ON/OFF"=w104, "Number Interlace Cycles"=w103, "AI1 Sets to FIFO"=w233, "FB On/Off Set 1"=w232, "FB On/Off Set 2"=w231, "Interlace Off Parameters"=w102, "FB Setpoint Set 1"=w223, "FB Setpoint Set 2"=w222, "FB Gains Set 1"=w220, "FB Gains Set 2"=w219, "FB output range 1"=w121, "FB output range 2"=w121, "Cycles per step"=w204, "Scan BD"=w216, "Number of scans"=w200, "Scan steps"=w205, "Scan freq.  increment"=w206, "AO1"=w188, "AO2"=w187, "Scan freq.  increment (MCL)"=w181, "Scan steps (MCL)"=w180, "Cycles per step (MCL)"=w179, "Number of scans (MCL)"=w178, "MCL count"=w101, "Cont. Scan (MCL)"=w177, "MCL Scan Axis"=w171, "1D or 2D Scan?"=w122, "N of AI1 Int Acq Sets"=w161, "Freq or Amp switch first"="Freq or Amp switch first", "Freq switch delay"="Freq switch delay", "Amp switch delay"="Amp switch delay", "Swap F1 and F2"="Swap F1 and F2", "APD Acq Rate Count"=w127, "APD to FIFO"=FALSE, "APD Gate Operating Mode"="APD Gate", "APD Gate ON Count"="APD Gate ON Count", "APD Gate OFF Count"="APD Gate OFF Count", "Invert APD Gate"="Invert APD Gate", "DIO count 1 (ticks)"="DIO count 1 (ticks)", "DIO count 2 (ticks)"="DIO count 2 (ticks)", "DIO count 3 (ticks)"="DIO count 3 (ticks)", "APD 1 AO scale factor"="APD 1 AO Mult.", "APD 2 AO scale factor"="APD 2 AO Mult.") -> ("FPGA VI Reference Out"=w96:T19, "error out"=w98:errorcluster)  [unwired: 1 in]
  n77 = local read "Green Laser ON/Interlacing"() -> (w99:bool)
  n78 = local read "Green laser mode"() -> (w100:enum32{"Laser ON", "Laser OFF", "Interlace"})
  n79 = local read "GI Frequency, OFF count"() -> (w92:u32)
  n80 = local read "GI Frequency, ON count"() -> (w91:u32)
  n81 = Multiply(x="Current When FB OFF (%)", y=655.35) -> (x*y=w82:dbl)
  n82 = local read "Green FB Count"() -> (w90:u32)
  n83 = Multiply(x="Green FB Setpoint (mV)", y=3.2767) -> (x*y=w79:dbl)
  n84 = To Unsigned Word Integer(number=w82) -> (unsigned 16bit integer=w80:u16)
  n85 = local read "Invert GI"() -> (w94:bool)
  n86 = To Word Integer(number=w79) -> (16bit integer=w77:i16)
  n87 = case shown="True" w99 {
    tunnel: w100 -> [_ w253]
    tunnel: [enum32{"Laser ON", "Laser OFF", "Interlace"}."Laser OFF" ("Green laser mode") w253] -> w93
    frame False {
    }
    frame True {
    }
  }
  n88 = local read "Trap Pos. AI1 X Pre-scale"() -> (w48:u16)
  n89 = local read "Trap Pos FB Monitor\nT1 or T2"() -> (w55:bool)
  n90 = local read "Trap Pos FB Int Count"() -> (w43:u16)
  n91 = local read "Trap Pos FB Negate Action"() -> (w54:bool)
  n92 = local read "Trap Pos. FB Offset Factor"() -> (w53:i64)
  n93 = local read "Trap Pos. FB Mult Factor"() -> (w52:i64)
  n94 = local read "Trap Pos. FB Gains"() -> (w50:T11)
  n95 = local read "Trap Pos. FB Range"() -> (w51:T12)
  n96 = xnode "Read/Write Control"("FPGA VI Reference In"=w96, "error in"=w98, "Green interlace ON count 2"=w91, "Green interlace OFF count 2"=w92, "Invert GI 2"=w94, "Operating Mode 2"=w93, "Green FB Gains"="Green FB Gains", "Green FB Setpoint"=w77, "Green FB On/Off"="Green FB On/Off", "Current Out"=w80, "Green int current ON count adj"="Green int current ON count adj", "Green FB Count"=w90, "Operating Mode"=w93, "Green interlace OFF count"=w92, "Green interlace ON count"=w91, "Invert GI"=w94, "Trap Pos FB Monitor T1 or T2"=w55, "Trap Pos FB Negate Action"=w54, "Trap Pos. FB Offset Factor"=w53, "Trap Pos. FB Mult Factor"=w52, "Trap Pos. FB Range"=w51, "Trap Pos. FB Gains"=w50, "Force feedback"=FALSE, "AI1 X Scale"=w48, "Trap Pos to FIFO"=TRUE, "Trap Pos FB Int Count"=w43) -> ("FPGA VI Reference Out"=w95:T19, "error out"=w97:errorcluster)
  n97 = xnode "Invoke Method"("FPGA VI Reference In"=w95, "error in"=w97, "Requested Depth"="Trap AI FIFO Depth") -> ("FPGA VI Reference Out"=w58:T19, "error out"=w57:errorcluster)  [unwired: 1 out]
  n98 = xnode "Invoke Method"("FPGA VI Reference In"=w58, "error in"=w57, "Requested Depth"="Trap Position FIFO Depth") -> ("FPGA VI Reference Out"=w45:T19, "error out"=w44:errorcluster)  [unwired: 1 out]
  n99 = flat-sequence {
    tunnel: w120 -> [w258]
    tunnel: [w258] -> w119
    tunnel: [w257] -> w118
    tunnel: [w256] -> w117
    tunnel: [w254] -> w115
    tunnel: [w255] -> w116
    frame #0 {
      w255 = T16 {"Minimum"=50.0, "Maximum"=100.0, "Increment"=1.0} ("Min Max Inc")
      w254 = T16 {"Minimum"=0.0, "Maximum"=75.0, "Increment"=1.0} ("Data Entry Limits")
      w257 = T16 {"Minimum"=50.0, "Maximum"=100.0, "Increment"=1.0} ("Min Max Inc")
      w256 = T16 {"Minimum"=0.0, "Maximum"=75.0, "Increment"=1.0} ("Data Entry Limits")
      n100 = property on="BD 2 Frequency 1 (MHz)" class="DigNum (strict)"("Data Range"=w255) -> ()  [unwired: 2 in, 2 out]
      n101 = property on="BD 2 Frequency 3 (MHz)" class="DigNum (strict)"("Data Range"=w255) -> ()  [unwired: 2 in, 2 out]
      n102 = property on="BD 2 Frequency 2 (MHz)" class="DigNum (strict)"("Data Range"=w255) -> ()  [unwired: 2 in, 2 out]
      n103 = property on="BD 1 Frequency 1 (MHz)" class="DigNum (strict)"("Data Range"=w257) -> ()  [unwired: 2 in, 2 out]
      n104 = property on="BD 1 Frequency 2 (MHz)" class="DigNum (strict)"("Data Range"=w257) -> ()  [unwired: 2 in, 2 out]
      n105 = property on="BD 1 Frequency 3 (MHz)" class="DigNum (strict)"("Data Range"=w257) -> ()  [unwired: 2 in, 2 out]
      n106 = property on="BD 2 Amplitude 1 (%)" class="DigNum (strict)"("Data Range"=w254) -> ()  [unwired: 2 in, 2 out]
      n107 = property on="BD 2 Amplitude 2 (%)" class="DigNum (strict)"("Data Range"=w254) -> ()  [unwired: 2 in, 2 out]
      n108 = property on="BD 2 Amplitude 3 (%)" class="DigNum (strict)"("Data Range"=w254) -> ()  [unwired: 2 in, 2 out]
      n109 = property on="BD 1 Amplitude 3 (%)" class="DigNum (strict)"("Data Range"=w256) -> ()  [unwired: 2 in, 2 out]
      n110 = property on="BD 1 Amplitude 2 (%)" class="DigNum (strict)"("Data Range"=w256) -> ()  [unwired: 2 in, 2 out]
      n111 = property on="BD 1 Amplitude 1 (%)" class="DigNum (strict)"("Data Range"=w256) -> ()  [unwired: 2 in, 2 out]
      "X RF Frequency Limits (MHz)" <- w257
      "X RF Amplitude Limits (%)" <- w256
      "Y RF Amplitude Limits (%)" <- w254
      "Y RF Frequency Limits (MHz)" <- w255
    }
  }
  n112 = xnode "Invoke Method"("FPGA VI Reference In"=w45, "error in"=w44) -> ("FPGA VI Reference Out"=w22:T19, "error out"=w21:errorcluster)  [unwired: 1 in]
  n113 = flat-sequence "Initial FPGA Loop Relative Phase Adjustment" {
    tunnel: "Initial Phase Adjustment (APD 2 Gate)" -> [w260]
    tunnel: "Initial Phase Adjustment (GI) 2" -> [w261]
    tunnel: "Initial Phase Adj. (MCL)" -> [w262]
    tunnel: w21 -> [w263]
    tunnel: w22 -> [w264]
    tunnel: "Initial Phase Adjustment (GI)" -> [w265]
    tunnel: "Initial Phase Adjustment (AI1)" -> [w266]
    tunnel: [w266] -> w31
    tunnel: [w265] -> w30
    tunnel: [w264] -> w29
    tunnel: [w263] -> w28
    tunnel: [w262] -> w27
    tunnel: [w261] -> w26
    tunnel: [w260] -> w25
    tunnel: [w278] -> w145
    tunnel: [w272] -> w143
    tunnel: "Initial Phase Adjustment (APD Acq)" -> [w271]
    tunnel: "Initial Phase Adjustment (APD 1 Gate)" -> [w270]
    tunnel: "Initial Phase Adjustment (Green FB)" -> [w269]
    tunnel: w31 -> [w277]
    tunnel: w30 -> [w276]
    tunnel: w29 -> [w275]
    tunnel: w28 -> [w274]
    tunnel: w27 -> [w273]
    tunnel: w26 -> [w268]
    tunnel: w25 -> [w267]
    tunnel: w145 -> [w280]
    tunnel: [w281] -> w144
    tunnel: w143 -> [w281]
    tunnel: [w280] -> w142
    tunnel: w144 -> [w284]
    tunnel: w142 -> [w283]
    tunnel: [w286] -> w141
    tunnel: [w285] -> w140
    tunnel: [w288] -> w20
    tunnel: [w289] -> w23
    tunnel: w141 -> [w289]
    tunnel: w140 -> [w288]
    frame #0 {
      n114 = Wait (ms)(milliseconds to wait=u32 1000) -> ()  [unwired: 1 out]
    }
    frame #1 {
      n115 = xnode "Read/Write Control"("FPGA VI Reference In"=w275, "error in"=w274, "Phase count adjustment"=w277, "Phase count adjustment (GI)"=w276, "Phase count adjustment (MCL)"=w273, "Phase Count Adjustment (APD Acq)"=w271, "Phase count adjustment (APD 1 Gate)"=w270, "Phase count adjustment (APD 2 Gate)"=w267, "Phase count adjustment (Green FB)"=w269, "Phase count adjustment (GI) 2"=w268) -> ("FPGA VI Reference Out"=w272:T19, "error out"=w278:errorcluster)
    }
    frame #2 {
      n116 = Wait (ms)(milliseconds to wait=u32 1000) -> ()  [unwired: 1 out]
    }
    frame #3 {
      w282 = TRUE
      n117 = xnode "Read/Write Control"("FPGA VI Reference In"=w284, "error in"=w283, "+ phase"=w282, "+ phase (GI)"=w282, "+ phase (MCL)"=w282, "+ phase (APD Acq)"=w282, "+ phase (APD 1 Gate)"=w282, "+ phase (APD 2 Gate)"=w282, "+ phase (Green FB)"=w282, "+ phase (GI) 2"=w282) -> ("FPGA VI Reference Out"=w285:T19, "error out"=w286:errorcluster)
    }
    frame #4 {
      n118 = Wait (ms)(milliseconds to wait=u32 1000) -> ()  [unwired: 1 out]
    }
  }
  n119 = local read "Phase adj. (Green FB)"() -> (w113:i16)
  n120 = local read "Phase adj. (GI) 2"() -> (w83:i16)
  n121 = local read "Phase adjust (MCL)"() -> (w172:i16)
  n122 = local read "Phase adj. (AI1)"() -> (w174:i16)
  n123 = local read "Phase adj. (GI)"() -> (w173:i16)
  n124 = xnode "Read/Write Control"("FPGA VI Reference In"=w20, "error in"=w23, "Phase count adjustment"=w174, "Phase count adjustment (GI)"=w173, "Phase count adjustment (MCL)"=w172, "Phase Count Adjustment (APD Acq)"="Phase Adj. (APD Acq)", "Phase count adjustment (APD 1 Gate)"="Phase Adj. (APD 1 Gate)", "Phase count adjustment (APD 2 Gate)"="Phase Adj. (APD 2 Gate)", "Phase count adjustment (Green FB)"=w113, "Phase count adjustment (GI) 2"=w83) -> ("FPGA VI Reference Out"=w19:T19, "error out"=w18:errorcluster)
  n125 = call "Initialize RF boards - interlace 3.vi"("error in"=w18, "FPGA VI Reference In"=w19) -> ("FPGA VI Reference Out"=w150:T19)  [unwired: 1 out]
  n126 = call "set RF board frequency - interlace.vi"("Board 2 Frequency Limits"=w116, "Board 1 Frequency Limits"=w118, "FPGA VI Reference In"=w150, "Board 2 Frequency 3 (MHz)"="BD 2 Frequency 3 (MHz)", "Board 1 Frequency 3 (MHz)"="BD 1 Frequency 3 (MHz)", "Board 2 Frequency 2 (MHz)"="BD 2 Frequency 2 (MHz)", "Board 2 Frequency 1 (MHz)"="BD 2 Frequency 1 (MHz)", "Board 1 Frequency 2 (MHz)"="BD 1 Frequency 2 (MHz)", "Board 1 Frequency 1  (MHz)"="BD 1 Frequency 1 (MHz)") -> ("error out"=w244:errorcluster, "FPGA VI Reference Out"=w245:T19)  [unwired: 1 in]
  n127 = call "set RF board amplitude - interlace.vi"("Board 2 Amplitude Limits"=w115, "Board 1 Amplitude Limits"=w117, "error in"=w244, "FPGA VI Reference In"=w245, "Board 2 Amplitude 3 (%)"="BD 2 Amplitude 3 (%)", "Board 1 Amplitude 3 (%)"="BD 1 Amplitude 3 (%)", "Board 2 Amplitude 2 (%)"="BD 2 Amplitude 2 (%)", "Board 2 Amplitude 1 (%)"="BD 2 Amplitude 1 (%)", "Board 1 Amplitude 2 (%)"="BD 1 Amplitude 2 (%)", "Board 1 Amplitude 1 (%)"="BD 1 Amplitude 1 (%)") -> ("error out"=w16:errorcluster, "FPGA VI Reference Out"=w17:T19)
  n128 = flat-sequence {
    tunnel: w17 -> [w298]
    tunnel: w16 -> [w297]
    tunnel: [w296] -> w237
    tunnel: [w295] -> w236
    tunnel: [w302] -> w235
    tunnel: w237 -> [w302]
    tunnel: [w301] -> w234
    tunnel: w236 -> [w301]
    tunnel: w235 -> [w311]
    tunnel: w234 -> [w310]
    tunnel: [w309] -> w12
    tunnel: [w304] -> w11
    tunnel: [w314] -> w40
    tunnel: [w318] -> w24
    tunnel: w12 -> [w318]
    tunnel: w11 -> [w313]
    frame #0 {
      n129 = local read "Trap 1 (ON/OFF)"() -> (w290:bool)
      n130 = xnode "Read/Write Control"("FPGA VI Reference In"=w298, "error in"=w297, "Direct RF Box  Communication"=FALSE) -> ("FPGA VI Reference Out"=w296:T19, "error out"=w295:errorcluster)
      n131 = local write "Saving..."(FALSE ("Saving Data")) -> ()
      n132 = local write "Stop All"(FALSE ("Stop All")) -> ()
      n133 = local write "Index"(1.0 ("Index")) -> ()
      n134 = property on="Trap 1 ON" class="Bool (strict)"("Value"=w290) -> ()  [unwired: 2 in, 2 out]
      "Manipulating Trap" <- FALSE ("Manipulating Trap")
    }
    frame #1 {
      n135 = local read "Trap 2 (ON/OFF)"() -> (w300:bool)
      n136 = Wait (ms)(milliseconds to wait=u32 50) -> ()  [unwired: 1 out]
      n137 = property on="Trap 2 ON" class="Bool (strict)"("Val(Sgnl)"=w300) -> ()  [unwired: 2 in, 2 out]
    }
    frame #2 {
      n138 = local read "Scan Range (nm)"() -> (w305:dbl)
      n139 = xnode "Read/Write Control"("FPGA VI Reference In"=w311, "error in"=w310, "FPGA Controls  RF Box"=TRUE ("Direct RF Box  Communication")) -> ("FPGA VI Reference Out"=w309:T19, "error out"=w304:errorcluster)
      n140 = call "Update messages.vi"("Message to add"="UHR-Fleezers ready.", "Old message string"="") -> ("New message string"=w308:string)
      n141 = local write "Messages"(w308) -> ()
      n142 = property on="Scan Range (nm)" class="DigNum (strict)"("Val(Sgnl)"=w305) -> ()  [unwired: 2 in, 2 out]
    }
    frame #3 {
      n143 = call "hamilton_controller.vi"("error in"=w313, "action"=T20."CONNECT") -> ("error out"=w315:errorcluster)  [unwired: 9 in]
      n144 = call "hamilton_controller.vi"("error in"=w315, "action"=T20."INITIALIZE VALVES") -> ("error out"=w314:errorcluster)  [unwired: 9 in]
    }
  }
  n145 = Subtract(x="BD 1 Frequency 1 (MHz)", y="BD 1 Frequency 2 (MHz)") -> (x-y=w160:dbl)
  n146 = Subtract(x="BD 2 Frequency 1 (MHz)", y="BD 2 Frequency 2 (MHz)") -> (x-y=w159:dbl)
  n147 = Square(x=w159) -> (x^2=w157:dbl)
  n148 = Square(x=w160) -> (x^2=w158:dbl)
  n149 = Add(x=w158, y=w157) -> (x+y=w156:dbl)
  n150 = Square Root(x=w156) -> (sqrt(x)=w155:dbl)
  n151 = local write "Trap Delta (MHz)"(w155) -> ()
  n152 = Current VI's Path() -> (path=w1:path)
  n153 = Strip Path(path=w1) -> (stripped path=w2:path)  [unwired: 1 out]
  n154 = Build Path(base path=w2, name or relative path="Locations.txt") -> (appended path=→"Location path":path)
  n155 = Concatenate Strings("N.D.", "\r\n") -> (w5:string)
  n156 = Initialize Array(w5, 4, 3) -> (w8:string[][])
  n157 = local write "Location Matrix"(w8) -> ()
  n158 = call "IMAQ Create"("Image Name"="APD 1 Image", "Image Type"=w64) -> ("New Image"=w63:T2)  [unwired: 3 in, 1 out]
  n159 = call "IMAQ Create"("Image Name"="APD 2 Image", "Image Type"=w64) -> ("New Image"=w62:T2)  [unwired: 3 in, 1 out]
  n160 = call "IMAQ Create"("Image Name"="Det. X Image", "Image Type"=w64) -> ("New Image"=w61:T2)  [unwired: 3 in, 1 out]
  n161 = call "IMAQ Create"("Image Name"="Det. Y Image", "Image Type"=w64) -> ("New Image"=w60:T2)  [unwired: 3 in, 1 out]
  n162 = Bundle("New Image"=w63, "New Image"=w62, "New Image"=w61, "New Image"=w60) -> (w59:T21)  [unwired: 1 in]
  n163 = while {
    stop <- w319 stop-if-true
    n164 = event shown="[0] Timeout" {
      selector: _ -> [_ _ _ _ _ _ _]
      dyn-events: _ -> [_ _ _ _ _ _ _]
      timeout: 10 -> [_ _ _ _ _ _ _]
      tunnel: [FALSE _ _ _ _ _ _] -> w319
      event Timeout {
        # "Query and display stage positions"
        # "Setting ESP300 left and right limits for Z-axis, input in mm"
        # "Display Selected Location"
        n165 = event-data() -> ()  [unwired: 1 in, 2 out]
        n166 = local read "ESP Port"() -> (w336:refnum<visa-resource-name>)
        n167 = Concatenate Strings("3SL" ("Substring"), "ESP ZL-Limit", ";3SR", "ESP ZR-Limit", "\r") -> (w335:string)
        n168 = VISA Write(VISA resource name=w336, write buffer=w335) -> ()  [unwired: 1 in, 3 out]
        n169 = disable-structure shown="Disabled" {
          frame Disabled {
            # "Change Low Jog Velocity"
            # "Change High Jog Velocity"
            n170 = Concatenate Strings("1JH" ("Substring"), "Axis 1", "2JH" ("Substring"), "Axis 2", "3JH" ("Substring"), "Axis 3", "\r") -> (w359:string)
            n171 = local read "ESP Port"() -> (w358:refnum<visa-resource-name>)
            n172 = VISA Write(VISA resource name=w358, write buffer=w359) -> ()  [unwired: 1 in, 3 out]
            n173 = Concatenate Strings("1JW" ("Substring"), "Axis 1", "2JW" ("Substring"), "Axis 2", "3JW" ("Substring"), "Axis 3", "\r") -> (w350:string)
            n174 = local read "ESP Port"() -> (w349:refnum<visa-resource-name>)
            n175 = VISA Write(VISA resource name=w349, write buffer=w350) -> ()  [unwired: 1 in, 3 out]
          }
          frame Enabled {
          }
        }
        n176 = local read "Location Matrix"() -> (w341:string[][])
        n177 = local read "Locations"() -> (w340:i32)
        n178 = Index Array(array=w341, index (row)=w340) -> (element=w339:string[])  [unwired: 1 in]
        n179 = Array To Cluster(array=w339) -> (cluster=w338:T22)
        n180 = local write "Selected Location"(w338) -> ()
        n181 = Concatenate Strings("1TP;\n2TP;\n3TP;\n1MD?;\n2MD?;\n3MD?" ("Substring"), "\r") -> (w324:string)
        n182 = local read "ESP Port"() -> (w327:refnum<visa-resource-name>)
        n183 = VISA Write(VISA resource name=w327, write buffer=w324, error in (no error)="error in") -> (VISA resource name out=w325:refnum<visa-resource-name>, error out=w323:errorcluster)  [unwired: 1 out]
        n184 = case shown="True" TRUE ("Case Constant\n(See Context Help)") {
          tunnel: w325 -> [_ w379]
          tunnel: w323 -> [w360 w378]
          tunnel: [w360 w362] -> w329
          frame False {
          }
          frame True {
            w372 = u16 10 items=["1.0"=10, "1.5"=15, "2.0"=20] ("Serial Settings:Stop Bits")
            w373 = u16 0 items=["None", "Odd", "Even", "Mark", "Space"] ("Serial Settings:Parity")
            n185 = property class="Instr"(reference=w379, error in=w378, "Baud"=u32 921600 ("Serial Settings:Baud Rate"), "Data Bits"=u16 8 ("Serial Settings:Data Bits"), "Parity"=w373, "Stop Bits"=w372) -> (reference out=w377:refnum<visa-resource-name>, error out=w376:errorcluster, "Bytes at Port"=w361:u32)
            n186 = Wait (ms)(milliseconds to wait=u32 10) -> ()  [unwired: 1 out]
            n187 = VISA Read(VISA resource name=w377, byte count=w361, error in (no error)=w376) -> (VISA resource name out=w385:refnum<visa-resource-name>, read buffer=→"X Pos":string, error out=w386:errorcluster)  [unwired: 1 out]
            n188 = VISA Read(VISA resource name=w385, byte count=w361, error in (no error)=w386) -> (VISA resource name out=w383:refnum<visa-resource-name>, read buffer=→"Y Pos":string, error out=w384:errorcluster)  [unwired: 1 out]
            n189 = VISA Read(VISA resource name=w383, byte count=w361, error in (no error)=w384) -> (VISA resource name out=w371:refnum<visa-resource-name>, read buffer=→"Z Pos Pos":string, error out=w370:errorcluster)  [unwired: 1 out]
            n190 = VISA Read(VISA resource name=w371, byte count=w361, error in (no error)=w370) -> (VISA resource name out=w367:refnum<visa-resource-name>, read buffer=→"X Motion":string, error out=w368:errorcluster)  [unwired: 1 out]
            n191 = VISA Read(VISA resource name=w367, byte count=w361, error in (no error)=w368) -> (VISA resource name out=w366:refnum<visa-resource-name>, read buffer=→"Y Motion":string, error out=w364:errorcluster)  [unwired: 1 out]
            n192 = VISA Read(VISA resource name=w366, byte count=w361, error in (no error)=w364) -> (read buffer=→"Z motion":string, error out=w362:errorcluster)  [unwired: 2 out]
          }
        }
        "error out" <- w329
      }
      event "Goto Top (F6)": Value Change {
        n193 = event-data() -> ()  [unwired: 1 in, 5 out]
        n194 = stacked-sequence {
          frame #0 {
            # "stop motions of all axes before going to avoid reversing of direction"
            n195 = local read "ESP Port"() -> (w391:refnum<visa-resource-name>)
            n196 = Concatenate Strings("ST" ("Substring"), "\r") -> (w388:string)
            n197 = VISA Write(VISA resource name=w391, write buffer=w388) -> ()  [unwired: 1 in, 3 out]
          }
          frame #1 {
            n198 = Wait (ms)(milliseconds to wait=u32 50) -> ()  [unwired: 1 out]
          }
          frame #2 {
            # "Change the trajectory mode to Trapezoidal"
            n199 = local read "ESP Port"() -> (w396:refnum<visa-resource-name>)
            n200 = Concatenate Strings("1TJ1;\n2TJ1;\n3TJ1" ("Substring"), "\r") -> (w393:string)
            n201 = VISA Write(VISA resource name=w396, write buffer=w393) -> ()  [unwired: 1 in, 3 out]
          }
          frame #3 {
            # "Go to Top Dispensor"
            n202 = local read "Location Matrix"() -> (w408:string[][])
            n203 = Index Array(array=w408, index (row)=0) -> (element=w404:string[])  [unwired: 1 in]
            n204 = Decimate 1D Array(w404) -> (w402:string[], w400:string[], w398:string[])
            n205 = Concatenate Strings("1PA" ("Substring"), w402, "2PA" ("Substring"), w400, "3PA" ("Substring"), w398, "\r") -> (w406:string)
            n206 = local read "ESP Port"() -> (w405:refnum<visa-resource-name>)
            n207 = VISA Write(VISA resource name=w405, write buffer=w406) -> ()  [unwired: 1 in, 3 out]
          }
          frame #4 {
            n208 = Wait (ms)(milliseconds to wait=u32 2000) -> ()  [unwired: 1 out]
          }
        }
      }
      event "Goto Exp (F8)": Value Change {
        n209 = event-data() -> ()  [unwired: 1 in, 5 out]
        n210 = stacked-sequence {
          frame #0 {
            # "stop motions of all axes before going to avoid reversing of direction"
            n211 = local read "ESP Port"() -> (w413:refnum<visa-resource-name>)
            n212 = Concatenate Strings("ST" ("Substring"), "\r") -> (w410:string)
            n213 = VISA Write(VISA resource name=w413, write buffer=w410) -> ()  [unwired: 1 in, 3 out]
          }
          frame #1 {
            n214 = Wait (ms)(milliseconds to wait=u32 50) -> ()  [unwired: 1 out]
          }
          frame #2 {
            # "Change the trajectory mode to Trapezoidal"
            n215 = local read "ESP Port"() -> (w418:refnum<visa-resource-name>)
            n216 = Concatenate Strings("1TJ1;\n2TJ1;\n3TJ1" ("Substring"), "\r") -> (w415:string)
            n217 = VISA Write(VISA resource name=w418, write buffer=w415) -> ()  [unwired: 1 in, 3 out]
          }
          frame #3 {
            # "Go to Experimental"
            n218 = local read "Location Matrix"() -> (w430:string[][])
            n219 = Index Array(array=w430, index (row)=2) -> (element=w426:string[])  [unwired: 1 in]
            n220 = Decimate 1D Array(w426) -> (w424:string[], w422:string[], w420:string[])
            n221 = Concatenate Strings("1PA" ("Substring"), w424, "2PA" ("Substring"), w422, "3PA" ("Substring"), w420, "\r") -> (w428:string)
            n222 = local read "ESP Port"() -> (w427:refnum<visa-resource-name>)
            n223 = VISA Write(VISA resource name=w427, write buffer=w428) -> ()  [unwired: 1 in, 3 out]
          }
          frame #4 {
            n224 = Wait (ms)(milliseconds to wait=u32 100) -> ()  [unwired: 1 out]
          }
        }
      }
      event "Goto Bottom (F7)": Value Change {
        n225 = event-data() -> ()  [unwired: 1 in, 5 out]
        n226 = stacked-sequence {
          frame #0 {
            # "stop motions of all axes before going to avoid reversing of direction"
            n227 = local read "ESP Port"() -> (w435:refnum<visa-resource-name>)
            n228 = Concatenate Strings("ST" ("Substring"), "\r") -> (w432:string)
            n229 = VISA Write(VISA resource name=w435, write buffer=w432) -> ()  [unwired: 1 in, 3 out]
          }
          frame #1 {
            n230 = Wait (ms)(milliseconds to wait=u32 50) -> ()  [unwired: 1 out]
          }
          frame #2 {
            # "Change the trajectory mode to Trapezoidal"
            n231 = local read "ESP Port"() -> (w440:refnum<visa-resource-name>)
            n232 = Concatenate Strings("1TJ1;\n2TJ1;\n3TJ1" ("Substring"), "\r") -> (w437:string)
            n233 = VISA Write(VISA resource name=w440, write buffer=w437) -> ()  [unwired: 1 in, 3 out]
          }
          frame #3 {
            # "Go to Bottom Dispensor"
            n234 = local read "Location Matrix"() -> (w452:string[][])
            n235 = Index Array(array=w452, index (row)=1) -> (element=w448:string[])  [unwired: 1 in]
            n236 = Decimate 1D Array(w448) -> (w446:string[], w444:string[], w442:string[])
            n237 = Concatenate Strings("1PA" ("Substring"), w446, "2PA" ("Substring"), w444, "3PA" ("Substring"), w442, "\r") -> (w450:string)
            n238 = local read "ESP Port"() -> (w449:refnum<visa-resource-name>)
            n239 = VISA Write(VISA resource name=w449, write buffer=w450) -> ()  [unwired: 1 in, 3 out]
          }
          frame #4 {
            n240 = Wait (ms)(milliseconds to wait=u32 100) -> ()  [unwired: 1 out]
          }
        }
      }
      event "Capture": Value Change {
        n241 = event-data() -> ()  [unwired: 1 in, 5 out]
        n242 = local read "Locations"() -> (w454:i32)
        n243 = local read "Z Pos Pos"() -> (w455:string)
        n244 = local read "X Pos"() -> (w457:string)
        n245 = local read "Y Pos"() -> (w456:string)
        n246 = case shown="1" w454 {
          selector: w454 -> [w461 w468 w475 w482]
          tunnel: w457 -> [w464 w471 w478 w485]
          tunnel: w456 -> [w463 w470 w477 w484]
          tunnel: w455 -> [w462 w469 w476 w483]
          frame 0, Default {
            # "Capture Top Dispensor Location"
            n247 = local read "Location Matrix"() -> (w460:string[][])
            n248 = Build Array(w464, w463, w462) -> (w459:string[])
            n249 = Replace Array Subset(array=w460, new element=w459, index (row)=w461) -> (w458:string[][])  [unwired: 1 in]
            n250 = local write "Location Matrix"(w458) -> ()
          }
          frame 1 {
            # "Capture Bottom Dispensor Location"
            n251 = local read "Location Matrix"() -> (w467:string[][])
            n252 = Build Array(w471, w470, w469) -> (w466:string[])
            n253 = Replace Array Subset(array=w467, new element=w466, index (row)=w468) -> (w465:string[][])  [unwired: 1 in]
            n254 = local write "Location Matrix"(w465) -> ()
          }
          frame 2 {
            # "Capture Experimental Region Location"
            n255 = local read "Location Matrix"() -> (w474:string[][])
            n256 = Build Array(w478, w477, w476) -> (w473:string[])
            n257 = Replace Array Subset(array=w474, new element=w473, index (row)=w475) -> (w472:string[][])  [unwired: 1 in]
            n258 = local write "Location Matrix"(w472) -> ()
          }
          frame 3 {
            # "Capture Other Location"
            n259 = local read "Location Matrix"() -> (w481:string[][])
            n260 = Build Array(w485, w484, w483) -> (w480:string[])
            n261 = Replace Array Subset(array=w481, new element=w480, index (row)=w482) -> (w479:string[][])  [unwired: 1 in]
            n262 = local write "Location Matrix"(w479) -> ()
          }
        }
      }
      event "Save": Value Change {
        # "reshape Location Matrix to 1-D array to write"
        n263 = event-data() -> ()  [unwired: 1 in, 5 out]
        n264 = local read "Location Matrix"() -> (w489:string[][])
        n265 = local read "Location path"() -> (w486:path)
        n266 = Reshape Array(w489, 12) -> (w487:string[])
        n267 = Write to Text File(file (use dialog)=w486, text=w487) -> ()  [unwired: 2 in, 3 out]
      }
      event "Activate Joystick": Value Change {
        n268 = event-data() -> ()  [unwired: 1 in, 5 out]
        n269 = case shown="True" "Activate Joystick" {
          frame False {
          }
          frame True {
            # "Change the trajectory mode to Jog"
            n270 = local read "ESP Port"() -> (w494:refnum<visa-resource-name>)
            n271 = Concatenate Strings("1TJ3;\n2TJ3;\n3TJ3" ("Substring"), "\r") -> (w491:string)
            n272 = VISA Write(VISA resource name=w494, write buffer=w491) -> ()  [unwired: 1 in, 3 out]
          }
        }
      }
    }
  }
  n273 = disable-structure shown="Disabled" {
    disable-tunnel: w24 -> [w523 _]
    frame Disabled {
      w518 = T17 0 items=["Grayscale (U8)", "Grayscale (I16)", "Grayscale (SGL)", "Complex (CSG)", "RGB (U32)", "HSL (U32)", "RGB (U64)", "Grayscale (U16)"] ("Image Type")
      n274 = call <vilib>:"IMAQ Init.vi"("Interface Name"="img0") -> ("error out"=w520:errorcluster, "IMAQ Session Out"=w522:refnum<k11>)  [unwired: 9 in]
      n275 = call <vilib>:"IMAQ Grab Setup.vi"("error in (no error)"=w520, "IMAQ Session In"=w522) -> ("error out"=w516:errorcluster, "IMAQ Session Out"=w517:refnum<k11>)  [unwired: 8 in]
      n276 = call "IMAQ Create"("Image Name"="untitled", "Image Type"=w518) -> ("New Image"=w515:T2)  [unwired: 3 in, 1 out]
      n277 = call <vilib>:"Application Directory.vi"() -> ("Application Directory"=w502:path)
      n278 = Build Path(base path=w502, name or relative path="_trap_screen_positions") -> (appended path=w510:path)
      n279 = Open/Create/Replace File(file path (use dialog)=w510, operation (0:open)=T23."open or create", access (0:read/write)=enum16{"read/write", "read-only", "write-only"}."read/write") -> (refnum out=w512:refnum<file>)  [unwired: 3 in, 2 out]
      n280 = local read "Trap Sets"() -> (w504:u32)
      n281 = for "Load trap positions on video screen from file." {
        N: w504 -> [_]
        tunnel: [w530] -> w505
        tunnel: w512 -> [w529]
        tunnel: [w526] -> w501 mode=indexing
        w528 = 4
        n282 = for {
          N: w528 -> [_]
          tunnel: [w534] -> w530
          tunnel: w529 -> [w533]
          tunnel: w528 -> [w532]
          tunnel: [w531] -> w527 mode=indexing
          n283 = Read from Binary File(5:w532, 11:w533) -> (2:w531:i32, 3:w534:refnum<file>)  [unwired: 4 in, 2 out]
        }
        n284 = Array To Cluster(array=w527) -> (cluster=w526:T27)
      }
      n285 = node-c288() -> (w525:T24)  [unwired: 4 in]
      n286 = timed-loop "acquire video and stage position" {
        timing: w525 -> [_]
        timing-out: [_] -> w524
        tunnel: w517 -> [w553]
        tunnel: w516 -> [w552]
        tunnel: w515 -> [w551]
        tunnel: [w550] -> w497
        tunnel: [w547] -> w498
        tunnel: [w548] -> w496
        tunnel: w523 -> [_]
        shift-right: [w544] -> w514
        shift-left: w501 -> [w545]
        tunnel: w504 -> [w542]
        stop <- w549 stop-if-true
        n287 = node-c288() -> ()  [unwired: 1 in, 1 out]
        n288 = event shown="[2] \"Primary Video Display\": Mouse Down" {
          selector: _ -> [_ _ _ _]
          dyn-events: _ -> [_ _ _ _]
          timeout: 10 -> [_ _ _ _]
          tunnel: w553 -> [w564 w579 w588 w607]
          tunnel: w552 -> [w563 w581 w586 w609]
          tunnel: w551 -> [w562 w580 w587 w608]
          tunnel: [w561 w579 w588 w607] -> w550
          tunnel: [w554 w583 FALSE FALSE] -> w549
          tunnel: [w558 w581 w586 w609] -> w548
          tunnel: [w557 w580 w587 w608] -> w547
          tunnel: "radius" -> [_ _ w593 _]
          tunnel: w545 -> [w555 w582 w591 _]
          tunnel: [w555 w582 w592 cluster{i32, i32, i32, i32}[] []] -> w544
          tunnel: w542 -> [_ _ w584 _]
          event Timeout {
            n289 = event-data() -> ()  [unwired: 1 in, 2 out]
            n290 = call <vilib>:"IMAQ Grab Acquire.vi"("error in (no error)"=w563, "Image In"=w562, "IMAQ Session In"=w564) -> ("error out"=w559:errorcluster, "Image Out"=w560:T2, "IMAQ Session Out"=w561:refnum<k11>)  [unwired: 5 in, 1 out]
            n291 = case shown="True" "trap\nmarkers?" {
              tunnel: w555 -> [_ w572]
              tunnel: w560 -> [w566 w571]
              tunnel: w559 -> [w565 w570]
              tunnel: [w565 w569] -> w558
              tunnel: [w566 w567] -> w557
              frame False {
              }
              frame True {
                n292 = for {
                  tunnel: w572 -> [w578] mode=indexing
                  shift-right: [w576] -> w567
                  shift-left: w571 -> [w577]
                  tunnel: w570 -> [w575]
                  tunnel: [w574] -> w569
                  tunnel: u32 16711680 ("Color") -> [w573]
                  n293 = call "IMAQ Overlay Oval"("Color"=w573, "error in (no error)"=w575, "Bounding Rectangle"=w578, "Image"=w577) -> ("error out"=w574:errorcluster, "Image Out"=w576:T2)  [unwired: 6 in]
                }
              }
            }
            "Primary Video Display" <- w557
            n294 = Unbundle By Name(w559) -> ("status"=w554:bool)
          }
          event "Stop All": Value Change {
            n295 = event-data() -> ()  [unwired: 1 in, 5 out]
            n296 = local read "Stop All"() -> (w583:bool)
          }
          event "Primary Video Display": Mouse Down {
            n297 = event-data() -> ()  [unwired: 1 in, 7 out]
            n298 = Array Size(array=w591) -> (size(s)=w590:i32)
            n299 = Less?(x=w590, y=w584) -> (x < y?=w589:bool)
            n300 = case shown="True" w589 {
              tunnel: w593 -> [_ w603]
              tunnel: w591 -> [w594 w597]
              tunnel: [w594 w596] -> w592
              frame False {
              }
              frame True {
                n301 = property on="Primary Video Display" class="ImageControl"() -> ("Last Mouse Position"=w595:cluster{"X":i32, "Y":i32})  [unwired: 2 in, 2 out]
                n302 = Unbundle By Name(w595) -> ("X"=w605:i32, "Y"=w604:i32)
                n303 = Add(x=w604, y=w603) -> (x+y=w601:i32)
                n304 = Subtract(x=w604, y=w603) -> (x-y=w599:i32)
                n305 = Add(x=w605, y=w603) -> (x+y=w600:i32)
                n306 = Subtract(x=w605, y=w603) -> (x-y=w602:i32)
                n307 = Bundle(w602, w601, w600, w599) -> (w598:cluster{i32, i32, i32, i32})  [unwired: 1 in]
                n308 = Build Array (concatenate)(w597, w598) -> (w596:T28)
              }
            }
          }
          event "clear markers": Value Change {
            n309 = event-data() -> ()  [unwired: 1 in, 5 out]
          }
        }
        n310 = node-c288() -> ()  [unwired: 1 in, 1 out]
      }
      n311 = node-c288(w524) -> ()  [unwired: 1 out]
      n312 = Set File Position(offset (in bytes) (0)=i64 0, refnum=w505, from (0:start)=enum16{"start", "end", "current"}."start") -> (refnum out=w506:refnum<file>)  [unwired: 1 in, 1 out]
      n313 = for "Write trap positions to file so they can be remembered\nwhen program is removed from memory" {
        tunnel: w514 -> [w538] mode=indexing
        tunnel: [w536] -> w513
        tunnel: w506 -> [w535]
        n314 = Cluster To Array(cluster=w538) -> (array=w537:i32[])
        n315 = for {
          tunnel: w537 -> [w541] mode=indexing
          tunnel: [w540] -> w536
          tunnel: w535 -> [w539]
          n316 = Write to Binary File(file (use dialog)=w539, data=w541) -> (refnum out=w540:refnum<file>)  [unwired: 4 in, 2 out]
        }
      }
      n317 = Close File(refnum=w513) -> ()  [unwired: 1 in, 2 out]
      n318 = call "IMAQ Dispose"("Image"=w498, "error in (no error)"=w496) -> ("error out"=w495:errorcluster)  [unwired: 4 in]
      n319 = call <vilib>:"IMAQ Stop.vi"("error in (no error)"=w495, "IMAQ Session In"=w497) -> ("error out"=w499:errorcluster, "IMAQ Session Out"=w500:refnum<k11>)  [unwired: 8 in]
      n320 = call <vilib>:"IMAQ Close.vi"("error in (no error)"=w499, "IMAQ Session In"=w500) -> ()  [unwired: 9 in, 1 out]
    }
    frame Enabled {
    }
  }
  n321 = node-c288(2 ("Processor")) -> (w15:T24)  [unwired: 3 in]
  n322 = node-c288() -> (w69:T24)  [unwired: 4 in]
  n323 = disable-structure shown="Enabled" {
    disable-tunnel: [w616 _] -> w35
    disable-tunnel: w24 -> [w615 _]
    frame Enabled {
      n324 = node-c288() -> (w618:T24)  [unwired: 4 out]
      n325 = timed-loop "Rough control of MCL mirror stage (debugging)" {
        tunnel: w615 -> [w621]
        tunnel: [w620] -> w616
        timing: w618 -> [_]
        timing-out: [_] -> w617
        stop <- w620 stop-if-true
        n326 = node-c288() -> ()  [unwired: 2 out]
        n327 = case shown="1" "MCL Mode" {
          tunnel: w621 -> [_ w624 w671]
          frame 0, Default {
            # "manual positioning"
          }
          frame 1 {
            # "sinusoidal wave"
            n328 = node-c288() -> (w626:T24)  [unwired: 4 out]
            n329 = timed-loop "Oscillate MCL mirror" {
              timing: w626 -> [_]
              timing-out: [_] -> w625
              tunnel: w624 -> [w665]
              i -> [w664]
              stop <- w627 stop-if-true
              n330 = node-c288() -> (w663:i64)  [unwired: 1 out]
              n331 = Multiply(x="AO1", y=32767.0) -> (x*y=w659:dbl)
              n332 = Multiply(x="AO2", y=32767.0) -> (x*y=w654:dbl)
              n333 = Divide(x=w659, y=10.0) -> (x/y=w660:dbl)
              n334 = Divide(x=w654, y=10.0) -> (x/y=w655:dbl)
              n335 = To Word Integer(number=w660) -> (16bit integer=w652:i16)
              n336 = To Word Integer(number=w655) -> (16bit integer=w651:i16)
              n337 = Divide(x=w663, y=i64 1000) -> (x/y=w634:dbl)
              n338 = Multiply(x=w634, y=w664) -> (x*y=w645:dbl)
              n339 = Multiply(x="Osc. freq. (Hz) 2", y=6.283185307179586) -> (x*y=w646:dbl)
              n340 = Multiply(x=w646, y=w645) -> (x*y=w644:dbl)
              n341 = Sine(x=w644) -> (sin(x)=w643:dbl)
              n342 = Multiply(x=w643, y="Osc. amp. (V)") -> (x*y=w641:dbl)
              n343 = Add(x=w641, y="Osc. center (V)") -> (x+y=w639:dbl)
              n344 = Divide(x=w639, y=10.0) -> (x/y=w637:dbl)
              n345 = Multiply(x=w637, y=32767.0) -> (x*y=w632:dbl)
              n346 = Select(t=w632, s="Scan axis", f=w652) -> (s? t:f=w650:dbl)
              n347 = Select(t=w651, s="Scan axis", f=w632) -> (s? t:f=w649:dbl)
              n348 = local read "MCL Mode"() -> (w631:u16)
              n349 = Not Equal?(x=w631, y=u16 1) -> (x != y?=w628:bool)
              n350 = local read "Stop All"() -> (w629:bool)
              n351 = xnode "Read/Write Control"("FPGA VI Reference In"=w665, "AO1"=w650, "AO2"=w649) -> ()  [unwired: 1 in, 2 out]
              n352 = Compound Arithmetic op=OR(w629, w628) -> (w627:bool)
              n353 = node-c288() -> ()  [unwired: 2 out]
            }
            n354 = node-c288(w625) -> ()  [unwired: 1 out]
          }
          frame 2 {
            # "linear scan"
            n355 = case shown="True" "Start Scan" {
              tunnel: w671 -> [_ w683]
              frame False {
              }
              frame True {
                n356 = Subtract(x="End (V)", y="Begin (V)") -> (x-y=w679:dbl)
                n357 = Decrement(x="N Points") -> (x-1=w678:dbl)
                n358 = Divide(x=w679, y=w678) -> (x/y=w676:dbl)
                n359 = for {
                  N: "N Points" -> [_]
                  tunnel: "Begin (V)" -> [w696]
                  tunnel: w683 -> [w688]
                  tunnel: [w687] -> w682 mode=indexing
                  tunnel: w676 -> [w686]
                  tunnel: [w684] -> w675 mode=indexing
                  i -> [w695]
                  n360 = Multiply(x=w686, y=w695) -> (x*y=w694:dbl)
                  n361 = Add(x=w696, y=w694) -> (x+y=w691:dbl)
                  n362 = local read "Scan axis"() -> (w685:bool)
                  n363 = local read "AO1"() -> (w693:dbl)
                  n364 = local read "AO2"() -> (w692:dbl)
                  n365 = Select(t=w691, s=w685, f=w693) -> (s? t:f=w690:dbl)
                  n366 = Select(t=w692, s=w685, f=w691) -> (s? t:f=w689:dbl)
                  n367 = flat-sequence {
                    tunnel: w690 -> [w700]
                    tunnel: w689 -> [w699]
                    tunnel: w688 -> [w697]
                    tunnel: [w710] -> w687
                    tunnel: [w709] -> w684
                    frame #0 {
                      w703 = 10.0 ("y")
                      w698 = 32767.0 ("y")
                      n368 = Multiply(x=w700, y=w698) -> (x*y=w706:dbl)
                      n369 = Multiply(x=w699, y=w698) -> (x*y=w704:dbl)
                      n370 = Divide(x=w706, y=w703) -> (x/y=w707:dbl)
                      n371 = Divide(x=w704, y=w703) -> (x/y=w705:dbl)
                      n372 = To Word Integer(number=w707) -> (16bit integer=w701:i16)
                      n373 = To Word Integer(number=w705) -> (16bit integer=w702:i16)
                      n374 = xnode "Read/Write Control"("FPGA VI Reference In"=w697, "AO1"=w701, "AO2"=w702) -> ()  [unwired: 1 in, 2 out]
                    }
                    frame #1 {
                      n375 = Wait (ms)(milliseconds to wait="DAQ Delay (ms)") -> ()  [unwired: 1 out]
                    }
                    frame #2 {
                      n376 = local read "Slow mean"() -> (w710:dbl)
                      n377 = local read "Sigma"() -> (w709:dbl)
                    }
                  }
                }
                n378 = Bundle("Begin (V)"="Begin (V)", w676, w682) -> (→"MCL Scan":cluster{"Begin (V)":dbl, dbl, dbl[]})  [unwired: 1 out]
                n379 = Bundle("Begin (V)"="Begin (V)", w676, w675) -> (→"MCL Scan 2":cluster{"Begin (V)":dbl, dbl, dbl[]})  [unwired: 1 out]
              }
            }
          }
        }
        n380 = local read "Stop All"() -> (w620:bool)
        n381 = node-c288() -> ()  [unwired: 2 out]
      }
      n382 = node-c288(w617) -> ()  [unwired: 1 out]
    }
    frame Disabled {
    }
  }
  n383 = timed-loop "Control parameters (event loop)" {
    tunnel: w24 -> [w716]
    shift-right: [w715] -> _
    shift-left: errorcluster {"status"=FALSE, "code"=0, "source"=""} ("error out") -> [w714]
    tunnel: [w713] -> w37
    timing: w15 -> [_]
    timing-out: [_] -> w14
    stop <- w713 stop-if-true
    n384 = node-c288() -> ()  [unwired: 1 in, 1 out]
    n385 = event shown="[6] \"BD 1 Frequency 1 (MHz)\", \"BD 1 Frequency 2 (MHz)\", \"BD 1 Frequency 3 (MHz)\", \"BD 2 Frequency 1 (MHz)\", \"BD 2 Frequency 2 (MHz)\", \"BD 2 Frequency 3 (MHz)\", \"Trap Delta (MHz)\": Value Change" {
      selector: _ -> [_ _ _ _ _ _ _ _ _ _ _ _ _ _ _ _ _ _ _ _ _ _ _ _ _ _ _ _ _ _ _ _ _ _ _ _ _ _ _ _ _ _ _ _ _ _ _ _ _ _ _ _ _ _ _]
      dyn-events: _ -> [_ _ _ _ _ _ _ _ _ _ _ _ _ _ _ _ _ _ _ _ _ _ _ _ _ _ _ _ _ _ _ _ _ _ _ _ _ _ _ _ _ _ _ _ _ _ _ _ _ _ _ _ _ _ _]
      timeout: _ -> [_ _ _ _ _ _ _ _ _ _ _ _ _ _ _ _ _ _ _ _ _ _ _ _ _ _ _ _ _ _ _ _ _ _ _ _ _ _ _ _ _ _ _ _ _ _ _ _ _ _ _ _ _ _ _]
      tunnel: w716 -> [w754 _ _ _ w791 _ w813 _ w877 _ _ _ w920 _ _ w963 w969 w974 w980 w1016 w1034 w1041 w1059 w1070 w1081 w1092 w1103 w1114 w1132 w1138 w1232 _ w1241 w1279 _ w1314 w1318 w1329 w1333 w1337 _ w1345 _ _ _ _ w1479 _ w1496 w1499 w1508 w1511 w1515 _ w1532]
      tunnel: [w753 _ _ _ w781 _ w812 _ w840 _ w885 _ w899 _ _ w962 w965 w971 w977 w1015 w1032 w1040 w1053 w1064 w1075 w1086 w1097 w1108 w1130 w1137 w1230 _ w1239 w1277 _ w1312 w1316 w1319 w1331 w1335 _ w1343 _ _ _ _ w1477 _ _ _ _ _ _ _ _] -> w715
      tunnel: w714 -> [w752 _ _ _ w790 _ w811 _ w872 _ w885 _ w919 _ _ w961 w964 w970 w976 w1014 w1033 w1039 w1058 w1069 w1080 w1091 w1102 w1113 w1131 w1136 w1231 _ w1240 w1278 _ w1313 w1317 w1328 w1332 w1336 _ w1344 _ _ _ _ w1478 _ w1495 w1498 w1507 w1510 w1514 _ w1531]
      tunnel: [_ _ _ _ _ _ _ _ _ _ w884 _ _ _ _ _ _ _ _ _ _ _ _ _ _ _ _ _ _ _ _ _ _ _ _ _ _ _ _ _ _ _ _ _ _ _ _ _ _ _ _ _ _ _ _] -> w713
      tunnel: [_ _ _ _ _ _ _ "Round T1 X" _ _ _ _ _ _ _ _ _ _ _ _ _ _ _ _ _ _ _ _ _ _ _ _ _ _ _ _ _ _ _ _ _ _ _ _ _ _ _ _ _ _ _ _ _ _ _] -> _
      tunnel: [_ _ _ "Adjust Scale\nto Mean" _ _ _ _ _ _ _ _ _ _ _ _ _ _ _ _ _ _ _ _ _ _ _ _ _ _ _ _ _ _ _ _ _ _ _ _ _ _ _ _ _ _ _ _ _ _ _ _ "Set SP to Reading" _ _] -> _
      tunnel: [_ _ _ _ _ _ _ _ _ "Round T2 X" _ "Delayed Interlace Start" _ _ _ _ _ _ _ _ _ _ _ _ _ _ _ _ _ _ _ _ _ _ _ _ _ _ _ _ _ _ _ _ _ _ _ _ _ _ _ _ _ _ _] -> _
      event "AI Count (ticks)", "Sets to FIFO (Traps)", "Save ave N", "FPGA Ave.", "# Samples/channel", "N sets to save": Value Change {
        # "So that if 'Save ave N' is updated, the AOD scanning code updates too."
        n386 = event-data() -> ()  [unwired: 6 out]
        n387 = local read "AI Count (ticks)"() -> (w734:u32)
        n388 = Boolean To (0,1)(Boolean="Sets to FIFO (Traps)") -> (0, 1=w744:cluster{"Set 1":i16, "Set 2":i16, "Set 3":i16})
        n389 = xnode "Read/Write Control"("FPGA VI Reference In"=w754, "error in"=w752, "ai count"=w734, "AI1 Sets to FIFO"="Sets to FIFO (Traps)", "N of AI1 Int Acq Sets"="N Acq Sets (Traps + Fl.)") -> ("error out"=w753:errorcluster)  [unwired: 1 out]
        n390 = Cluster To Array(cluster=w744) -> (array=w743:i16[])
        n391 = To Unsigned Long Integer(number=w743) -> (unsigned 32bit integer=w723:u32[])
        n392 = local read "Scan steps (AOD)"() -> (w745:u64)
        n393 = Multiply(x=w734, y="N Acq Sets (Traps + Fl.)") -> (x*y=w732:u32)
        n394 = Divide(x=40000000.0, y=w734) -> (x/y=w726:dbl)
        "AI rate (Hz)" <- w726
        "Ave. Rate (Hz)" <- w726
        n395 = Add Array Elements(numeric array=w723) -> (sum=w735:u32)
        "Trap Sets" <- w735
        n396 = Reciprocal(x=w726) -> (1/x=→"Ave. Period (s)":dbl)
        n397 = property on="Scan steps (AOD)" class="DigNum (strict)"("Val(Sgnl)"=w745) -> ()  [unwired: 2 in, 2 out]
        n398 = Divide(x=w726, y="N Acq Sets (Traps + Fl.)") -> (x/y=w749:dbl)
        "Data Rate (Hz)" <- w749
        n399 = Reciprocal(x=w749) -> (1/x=→"Data Period (s)":dbl)
        n400 = local read "Save ave N"() -> (w748:dbl)
        n401 = Divide(x=w749, y=w748) -> (x/y=w747:dbl)
        "Save Data Rate (Hz)" <- w747
        n402 = Reciprocal(x=w747) -> (1/x=→"Save Data Period (s)":dbl)
        n403 = Multiply(x=w732, y="# Samples/trap") -> (x*y=w730:u32)
        "Counts/DMA" <- w730
        n404 = property on="Trap Disp. Downsample" class="DigNum (strict)"("Maximum"="# Samples/trap") -> ()  [unwired: 2 in, 2 out]
        n405 = Multiply(x=w735, y="# Samples/trap") -> (x*y=w724:u32)
        "# Samples/channel" <- w724
        n406 = Multiply(x=w724, y=u32 8) -> (x*y=→"Trap AI Elements/DMA read":u32)
        n407 = local read "APD Int. Count"() -> (w731:u32)
        n408 = Multiply(x=w724, y=u32 3) -> (x*y=→"Trap Pos Elements/DMA read":u32)
        n409 = Divide(x=w730, y=w731) -> (x/y=w721:dbl)
        "APD Samples/FIFO Acq." <- w721
        n410 = Divide(x=w730, y=40000000.0) -> (x/y=w728:dbl)
        "DMA Update Period (s)" <- w728
        n411 = Multiply(x=2.0, y=w721) -> (x*y=→"APD Elements/DMA read":dbl)
        n412 = property on="APD Disp. Downsample" class="DigNum (strict)"("Maximum"=w721) -> ()  [unwired: 2 in, 2 out]
        n413 = local read "N sets to save"() -> (w741:u32)
        n414 = Multiply(x=w728, y=w741) -> (x*y=→"Total Time (s)":dbl)
        "FPGA Averaging" <- FALSE ("FPGA Averaging")
      }
      event "Rescale on Mean": Value Change {
        n415 = event-data() -> ()  [unwired: 7 out]
        n416 = And(x=FALSE, y="Rescale on Mean") -> (x .and. y?=w756:bool)
        n417 = local write "Rescale on Mean"(w756) -> ()
        n418 = local read "Bead Mean (nm)"() -> (w761:dbl)
        n419 = Add(x="Amplitude (nm)", y=w761) -> (x+y=w759:dbl)
        n420 = Subtract(x=w761, y="Amplitude (nm)") -> (x-y=w758:dbl)
        n421 = property on="Bead Separation" class="WFChart (strict)"("YScale.Minimum"=w758) -> ()  [unwired: 2 in, 2 out]
        n422 = property on="Bead Separation" class="WFChart (strict)"("YScale.Maximum"=w759) -> ()  [unwired: 2 in, 2 out]
      }
      event "Detector Type": Value Change {
        n423 = event-data() -> ()  [unwired: 7 out]
        n424 = local read "AI labels"() -> (w762:string[])
        n425 = property on="High Res. Display" class="Ring (strict)"("Strings []"=w762) -> ()  [unwired: 2 in, 2 out]
        n426 = Build Array (concatenate)(w762, "none") -> (w763:string[])
        n427 = property on="FFT 1 Choice 1" class="Ring (strict)"("Strings []"=w763) -> ()  [unwired: 2 in, 2 out]
        n428 = property on="FFT 1 Choice 2" class="Ring (strict)"("Strings []"=w763) -> ()  [unwired: 2 in, 2 out]
        n429 = property on="FFT 2 Choice 1" class="Ring (strict)"("Strings []"=w763) -> ()  [unwired: 2 in, 2 out]
        n430 = property on="FFT 2 Choice 2" class="Ring (strict)"("Strings []"=w763) -> ()  [unwired: 2 in, 2 out]
        n431 = Bundle("APD 1", "APD 2") -> (w766:cluster{string, string})  [unwired: 1 out]
        n432 = Cluster To Array(cluster=w766) -> (array=w764:string[])
        n433 = Build Array (concatenate)(w764, w763) -> (w768:string[])
        n434 = Array Size(array=w768) -> (size(s)=w769:i32)
        n435 = property on="Signals to Plot" class="LstBox (strict)"("Item Names"=w768) -> ()  [unwired: 2 in, 2 out]
        n436 = property on="Signals to Plot" class="LstBox (strict)"("Number of Rows"=w769) -> ()  [unwired: 2 in, 2 out]
        n437 = property on="All Signals" class="WFChart (strict)"("LegNumRows"=w769) -> ()  [unwired: 2 in, 2 out]
      }
      event "Adjust Scale\nto Mean": Value Change {
        n438 = event-data() -> ()  [unwired: 7 out]
        n439 = local read "APD 1 Rate (Hz)"() -> (w778:dbl)
        n440 = Multiply(x=1000.0, y="Above (kHz)") -> (x*y=w776:dbl)
        n441 = Multiply(x=1000.0, y="Below (kHz)") -> (x*y=w774:dbl)
        n442 = Add(x=w776, y=w778) -> (x+y=w771:dbl)
        n443 = Subtract(x=w778, y=w774) -> (x-y=w772:dbl)
        n444 = property on="APD Chart" class="WFChart (strict)"("YScale.Minimum"=w772) -> ()  [unwired: 2 in, 2 out]
        n445 = property on="APD Chart" class="WFChart (strict)"("YScale.Maximum"=w771) -> ()  [unwired: 2 in, 2 out]
      }
      event "Phase adj. (AI1)", "+ phase (AI1)", "- phase (AI1)": Value Change {
        n446 = event-data() -> ()  [unwired: 7 out]
        n447 = Negate(x="Phase adj. (AI1)") -> (-x=w788:i16)
        n448 = Select(t=w788, s="- phase (AI1)", f="Phase adj. (AI1)") -> (s? t:f=w787:i16)
        n449 = xnode "Read/Write Control"("FPGA VI Reference In"=w791, "error in"=w790, "Phase count adjustment"=w787) -> ("FPGA VI Reference Out"=w786:T19, "error out"=w785:errorcluster)
        n450 = Or(x="- phase (AI1)", y="+ phase (AI1)") -> (x .or. y?=w782:bool)
        n451 = xnode "Read/Write Control"("FPGA VI Reference In"=w786, "error in"=w785, "+ phase"=w782) -> ("error out"=w781:errorcluster)  [unwired: 1 out]
      }
      event "Signals to Plot": Double Click {
        w794 = u32 9868950 ("Color Box")
        n452 = event-data() -> ("Row"=w796:i32)  [unwired: 9 out]
        n453 = property on="All Signals" class="WFChart (strict)"("Active Plot"=w796) -> (error out=w807:errorcluster)  [unwired: 2 in, 1 out]
        n454 = property on="All Signals" class="WFChart (strict)" props=["Plot", "Visible?", "Plot", "Plot Color"](error in=w807) -> (error out=w806:errorcluster, "Plot.Visible?"=w805:bool)  [unwired: 1 in, 2 out]
        n455 = Select(t=FALSE ("Plot.Visible"), s=w805, f=TRUE ("Plot.Visible")) -> (s? t:f=w800:bool)
        n456 = property on="All Signals" class="WFChart (strict)"(error in=w806, "Plot.Visible?"=w800) -> (error out=w802:errorcluster)  [unwired: 1 in, 1 out]
        n457 = property on="All Signals" class="WFChart (strict)"(error in=w802) -> (error out=w797:errorcluster, "Plot.Plot Color"=w801:u32)  [unwired: 1 in, 1 out]
        n458 = property on="Signals to Plot" class="LstBox (strict)"(error in=w797, "Active Row"=w796) -> (error out=w795:errorcluster)  [unwired: 1 in, 1 out]
        n459 = Select(t=w801, s=w800, f=u32 0) -> (s? t:f=w798:u32)
        n460 = property on="Signals to Plot" class="LstBox (strict)"(error in=w795, "CellFontColor"=w798, "SelColor"=w794, "CellBG"=w794, "CellFontSize"=u32 20 ("Active Row:Cell Font:Size"), "CellFontBold"=TRUE ("Active Row:Cell Font:Bold")) -> ()  [unwired: 1 in, 2 out]
      }
      event "BD 1 Frequency 1 (MHz)", "BD 1 Frequency 2 (MHz)", "BD 1 Frequency 3 (MHz)", "BD 2 Frequency 1 (MHz)", "BD 2 Frequency 2 (MHz)", "BD 2 Frequency 3 (MHz)", "Trap Delta (MHz)": Value Change {
        # "anytime one of the frequencies is changed, write it to the RF board UNLESS Set 2 is being oscillated. The oscillation\nscript writes the frequencies to the RF board."
        n461 = event-data() -> ("CtlRef"=w810:refnum<vi>)  [unwired: 6 out]
        n462 = control-ref of="Trap Delta (MHz)"() -> (w809:refnum<vi>)
        n463 = Equal?(x=w809, y=w810) -> (x = y?=w808:bool)
        n464 = case shown="False" "Oscillate Set 2" {
          tunnel: w813 -> [w833 _]
          tunnel: [w832 w836] -> w812
          tunnel: w811 -> [w831 w836]
          tunnel: w808 -> [w817 _]
          frame False {
            n465 = local read "BD 1 Frequency 1 (MHz)"() -> (w815:dbl)
            n466 = local read "BD 1 Frequency 2 (MHz)"() -> (w819:dbl)
            n467 = Add(x=w815, y="Trap Delta (MHz)") -> (x+y=w818:dbl)
            n468 = Select(t=w818, s=w817, f=w819) -> (s? t:f=w816:dbl)
            n469 = local read "Y RF Frequency Limits (MHz)"() -> (w821:T16)
            n470 = local read "X RF Frequency Limits (MHz)"() -> (w822:T16)
            n471 = local read "BD 1 Frequency 3 (MHz)"() -> (w834:dbl)
            n472 = local write "BD 1 Frequency 2 (MHz)"(w816) -> ()
            n473 = local read "BD 2 Frequency 1 (MHz)"() -> (w825:dbl)
            n474 = local read "BD 2 Frequency 2 (MHz)"() -> (w824:dbl)
            n475 = local read "BD 2 Frequency 3 (MHz)"() -> (w835:dbl)
            n476 = call "set RF board frequency - interlace.vi"("Board 2 Frequency Limits"=w821, "Board 1 Frequency Limits"=w822, "error in"=w831, "FPGA VI Reference In"=w833, "Board 2 Frequency 3 (MHz)"=w835, "Board 1 Frequency 3 (MHz)"=w834, "Board 2 Frequency 2 (MHz)"=w824, "Board 2 Frequency 1 (MHz)"=w825, "Board 1 Frequency 2 (MHz)"=w816, "Board 1 Frequency 1  (MHz)"=w815) -> ("error out"=w832:errorcluster)  [unwired: 1 out]
            n477 = Subtract(x=w825, y=w824) -> (x-y=w829:dbl)
            n478 = Subtract(x=w816, y=w815) -> (x-y=w830:dbl)
            n479 = Square(x=w829) -> (x^2=w827:dbl)
            n480 = Square(x=w830) -> (x^2=w828:dbl)
            n481 = Add(x=w828, y=w827) -> (x+y=w826:dbl)
            n482 = Square Root(x=w826) -> (sqrt(x)=w823:dbl)
            n483 = local write "Trap Delta (MHz)"(w823) -> ()
            n484 = property on="Initial delta (MHz)" class="DigNum (strict)"("Val(Sgnl)"=w823) -> ()  [unwired: 2 in, 2 out]
          }
          frame True {
          }
        }
      }
      event "Round T1 X": Value Change {
        n485 = event-data() -> ()  [unwired: 7 out]
        n486 = local read "BD 1 Frequency 1 (MHz)"() -> (w839:dbl)
        n487 = Round To Nearest(number=w839) -> (nearest integer value=w838:dbl)
        n488 = property on="BD 1 Frequency 1 (MHz)" class="DigNum (strict)"("Val(Sgnl)"=w838) -> ()  [unwired: 2 in, 2 out]
      }
      event "Restart RF": Value Change {
        n489 = event-data() -> ()  [unwired: 7 out]
        n490 = xnode "Read/Write Control"("FPGA VI Reference In"=w877, "error in"=w872, "FPGA Controls  RF Box"=FALSE) -> ("FPGA VI Reference Out"=w876:T19, "error out"=w871:errorcluster)
        n491 = local read "Y RF Amplitude Limits (%)"() -> (w852:T16)
        n492 = local read "X RF Amplitude Limits (%)"() -> (w853:T16)
        n493 = local read "X RF Frequency Limits (MHz)"() -> (w855:T16)
        n494 = local read "Y RF Frequency Limits (MHz)"() -> (w854:T16)
        n495 = xnode "Read/Write Control"("FPGA VI Reference In"=w876, "error in"=w871, "Direct RF Box  Communication"=TRUE) -> ("FPGA VI Reference Out"=w875:T19, "error out"=w870:errorcluster)
        n496 = local read "BD 2 Frequency 3 (MHz)"() -> (w862:dbl)
        n497 = local read "BD 2 Frequency 2 (MHz)"() -> (w863:dbl)
        n498 = local read "BD 1 Frequency 3 (MHz)"() -> (w866:dbl)
        n499 = local read "BD 1 Frequency 1 (MHz)"() -> (w867:dbl)
        n500 = local read "BD 2 Frequency 1 (MHz)"() -> (w864:dbl)
        n501 = local read "BD 1 Frequency 2 (MHz)"() -> (w865:dbl)
        n502 = call "Initialize RF boards - interlace 3.vi"("error in"=w870, "FPGA VI Reference In"=w875) -> ("error out"=w869:errorcluster, "FPGA VI Reference Out"=w874:T19)
        n503 = local read "BD 2 Amplitude 2 (%)"() -> (w857:dbl)
        n504 = local read "BD 2 Amplitude 1 (%)"() -> (w858:dbl)
        n505 = local read "BD 2 Amplitude 3 (%)"() -> (w856:dbl)
        n506 = local read "BD 1 Amplitude 3 (%)"() -> (w861:dbl)
        n507 = local read "BD 1 Amplitude 1 (%)"() -> (w860:dbl)
        n508 = local read "BD 1 Amplitude 2 (%)"() -> (w859:dbl)
        n509 = call "set RF board frequency - interlace.vi"("Board 2 Frequency Limits"=w854, "Board 1 Frequency Limits"=w855, "error in"=w869, "FPGA VI Reference In"=w874, "Board 2 Frequency 3 (MHz)"=w862, "Board 1 Frequency 3 (MHz)"=w866, "Board 2 Frequency 2 (MHz)"=w863, "Board 2 Frequency 1 (MHz)"=w864, "Board 1 Frequency 2 (MHz)"=w865, "Board 1 Frequency 1  (MHz)"=w867) -> ("error out"=w868:errorcluster, "FPGA VI Reference Out"=w873:T19)
        n510 = call "set RF board amplitude - interlace.vi"("Board 2 Amplitude Limits"=w852, "Board 1 Amplitude Limits"=w853, "error in"=w868, "FPGA VI Reference In"=w873, "Board 2 Amplitude 3 (%)"=w856, "Board 1 Amplitude 3 (%)"=w861, "Board 2 Amplitude 2 (%)"=w857, "Board 2 Amplitude 1 (%)"=w858, "Board 1 Amplitude 2 (%)"=w859, "Board 1 Amplitude 1 (%)"=w860) -> ("error out"=w845:errorcluster, "FPGA VI Reference Out"=w849:T19)
        n511 = xnode "Read/Write Control"("FPGA VI Reference In"=w849, "error in"=w845, "Direct RF Box  Communication"=FALSE) -> ("FPGA VI Reference Out"=w848:T19, "error out"=w847:errorcluster)
        n512 = flat-sequence {
          tunnel: w847 -> [w878]
          tunnel: [w878] -> w846
          frame #0 {
            n513 = Wait (ms)(milliseconds to wait=u32 50) -> ()  [unwired: 1 out]
          }
        }
        n514 = xnode "Read/Write Control"("FPGA VI Reference In"=w848, "error in"=w846, "FPGA Controls  RF Box"=TRUE) -> ("error out"=w841:errorcluster)  [unwired: 1 out]
        n515 = property on="Restart RF" class="Bool (strict)"(error in=w841, "Value"=FALSE ("Restart RF")) -> (error out=w840:errorcluster)  [unwired: 1 in, 1 out]
      }
      event "Round T2 X": Value Change {
        n516 = event-data() -> ()  [unwired: 7 out]
        n517 = local read "BD 1 Frequency 2 (MHz)"() -> (w881:dbl)
        n518 = Round To Nearest(number=w881) -> (nearest integer value=w880:dbl)
        n519 = property on="BD 1 Frequency 2 (MHz)" class="DigNum (strict)"("Val(Sgnl)"=w880) -> ()  [unwired: 2 in, 2 out]
      }
      event "Stop All": Value Change {
        n520 = event-data() -> ()  [unwired: 7 out]
        n521 = call "hamilton_controller.vi"("action"=T20."DISCONNECT") -> ()  [unwired: 10 in, 1 out]
        n522 = local read "Stop All"() -> (w884:bool)
      }
      event "Delayed Interlace Start": Value Change {
        n523 = event-data() -> ()  [unwired: 7 out]
        n524 = flat-sequence {
          frame #0 {
            n525 = Multiply(x="Delay to Interlace (s)", y=1000.0) -> (x*y=w887:dbl)
            n526 = Wait (ms)(milliseconds to wait=w887) -> ()  [unwired: 1 out]
          }
          frame #1 {
            n527 = property on="Green laser mode" class="RadioBtnsControl (strict)"("Val(Sgnl)"=enum32{"Laser ON", "Laser OFF", "Interlace"}."Interlace" ("Value (Signaling)")) -> ()  [unwired: 2 in, 2 out]
          }
        }
      }
      event "BD 1 Amplitude 1 (%)", "BD 1 Amplitude 2 (%)", "BD 1 Amplitude 3 (%)", "BD 2 Amplitude 1 (%)", "BD 2 Amplitude 2 (%)", "BD 2 Amplitude 3 (%)", "Trap 1 ON", "Trap 2 ON", "Trap 3 ON", "Feedback On/Off", "All FB On/Off": Value Change {
        w911 = i16 1 ("f")
        n528 = event-data() -> ()  [unwired: 7 out]
        n529 = local write "Trap 1 (ON/OFF)"("Trap 1 ON") -> ()
        n530 = local write "Trap 2 (ON/OFF)"("Trap 2 ON") -> ()
        n531 = Boolean To (0,1)(Boolean="Trap 3 ON") -> (0, 1=w912:i16)
        n532 = Boolean To (0,1)(Boolean="Trap 1 ON") -> (0, 1=w913:i16)
        n533 = Boolean To (0,1)(Boolean="Trap 2 ON") -> (0, 1=w914:i16)
        n534 = Select(t=w914, s="Trap ON/OFF X or Y Amp?", f=w911) -> (s? t:f=w909:i16)
        n535 = Select(t=w913, s="Trap ON/OFF X or Y Amp?", f=w911) -> (s? t:f=w910:i16)
        n536 = Select(t=w912, s="Trap ON/OFF X or Y Amp?", f=w911) -> (s? t:f=w908:i16)
        n537 = Select(t=w911, s="Trap ON/OFF X or Y Amp?", f=w914) -> (s? t:f=w906:i16)
        n538 = Select(t=w911, s="Trap ON/OFF X or Y Amp?", f=w913) -> (s? t:f=w907:i16)
        n539 = Select(t=w911, s="Trap ON/OFF X or Y Amp?", f=w912) -> (s? t:f=w905:i16)
        n540 = And(x="All FB On/Off", y="Feedback On/Off") -> (x .and. y?=w903:cluster{"Set 1":bool, "Set 2":bool})
        n541 = local read "BD 1 Amplitude 1 (%)"() -> (w923:dbl)
        n542 = local read "BD 1 Amplitude 2 (%)"() -> (w922:dbl)
        n543 = local read "BD 1 Amplitude 3 (%)"() -> (w921:dbl)
        n544 = Unbundle By Name(w903) -> ("Set 1"=w898:bool, "Set 2"=w895:bool)
        n545 = local read "Y RF Amplitude Limits (%)"() -> (w891:T16)
        n546 = local read "X RF Amplitude Limits (%)"() -> (w892:T16)
        n547 = local read "BD 2 Amplitude 1 (%)"() -> (w924:dbl)
        n548 = local read "BD 2 Amplitude 2 (%)"() -> (w925:dbl)
        n549 = local read "BD 2 Amplitude 3 (%)"() -> (w926:dbl)
        n550 = And(x="Trap 2 ON", y=w895) -> (x .and. y?=w893:bool)
        n551 = And(x="Trap 1 ON", y=w898) -> (x .and. y?=w896:bool)
        n552 = Multiply(x=w910, y=w923) -> (x*y=w918:dbl)
        n553 = Multiply(x=w922, y=w909) -> (x*y=w916:dbl)
        n554 = Multiply(x=w921, y=w908) -> (x*y=w917:dbl)
        n555 = Multiply(x=w924, y=w907) -> (x*y=w927:dbl)
        n556 = Multiply(x=w925, y=w906) -> (x*y=w928:dbl)
        n557 = Multiply(x=w926, y=w905) -> (x*y=w929:dbl)
        n558 = call "set RF board amplitude - interlace.vi"("Board 2 Amplitude Limits"=w891, "Board 1 Amplitude Limits"=w892, "error in"=w919, "FPGA VI Reference In"=w920, "Board 2 Amplitude 3 (%)"=w929, "Board 1 Amplitude 3 (%)"=w917, "Board 2 Amplitude 2 (%)"=w928, "Board 2 Amplitude 1 (%)"=w927, "Board 1 Amplitude 2 (%)"=w916, "Board 1 Amplitude 1 (%)"=w918) -> ("error out"=w900:errorcluster, "FPGA VI Reference Out"=w901:T19)
        n559 = xnode "Read/Write Control"("FPGA VI Reference In"=w901, "error in"=w900, "FB On/Off Set 1"=w896, "FB On/Off Set 2"=w893) -> ("error out"=w899:errorcluster)  [unwired: 1 out]
      }
      event "Load parameters": Value Change {
        n560 = event-data() -> ()  [unwired: 7 out]
        n561 = property on="Saved AOD Raster Scan Parameter Sets" class="Arr (strict)"() -> ("Index Values"=w940:u32[])  [unwired: 2 in, 2 out]
        n562 = Index Array(array=w940, index=0) -> (element=w937:u32)
        n563 = local write "Load parameters"(FALSE ("Load parameters")) -> ()
        n564 = Index Array(array="Saved AOD Raster Scan Parameter Sets", index=w937) -> (element=w936:T30)
        n565 = Unbundle By Name(w936) -> ("Scan Range AOD (nm) 2"=w935:dbl, "Step Size AOD (nm) 2"=w934:dbl, "Scan Speed AOD (nm/s) 2"=w933:dbl, "Number of scans (AOD) 2"=w932:u16)
        n566 = flat-sequence {
          tunnel: w935 -> [w943]
          tunnel: w934 -> [w942]
          tunnel: w933 -> [w941]
          tunnel: w932 -> [w944]
          frame #0 {
            n567 = local write "Scan Speed (nm/s)"(w941) -> ()
            n568 = local write "Scan Range (nm)"(w943) -> ()
            n569 = local write "Step Size (nm)"(w942) -> ()
          }
          frame #1 {
            n570 = property on="Number of F/B Scans (AOD)" class="DigNum (strict)"("Val(Sgnl)"=w944) -> ()  [unwired: 2 in, 2 out]
          }
        }
      }
      event "Trap 1 (ON/OFF)", "Trap 2 (ON/OFF)": Value Change {
        n571 = event-data() -> ()  [unwired: 7 out]
        n572 = property on="Trap 2 ON" class="Bool (strict)"("Val(Sgnl)"="Trap 2 (ON/OFF)") -> ()  [unwired: 2 in, 2 out]
        n573 = property on="Trap 1 ON" class="Bool (strict)"("Val(Sgnl)"="Trap 1 (ON/OFF)") -> ()  [unwired: 2 in, 2 out]
      }
      event "DIO count 1 (ticks)", "DIO count 2 (ticks)", "DIO count 3 (ticks)", "Interlace", "Number Interlace Sets", "Not-Interlacing Set": Value Change {
        n574 = event-data() -> ()  [unwired: 7 out]
        n575 = local read "DIO count 3 (ticks)"() -> (w957:u32)
        n576 = local read "DIO count 1 (ticks)"() -> (w959:u32)
        n577 = local read "DIO count 2 (ticks)"() -> (w958:u32)
        n578 = To Unsigned Byte Integer(number="Not-Interlacing Set") -> (unsigned 8bit integer=w948:u8)
        n579 = Add(x=w948, y=u8 1) -> (x+y=w952:u8)
        n580 = xnode "Read/Write Control"("FPGA VI Reference In"=w963, "error in"=w961, "DIO count 1 (ticks)"=w959, "DIO count 2 (ticks)"=w958, "DIO count 3 (ticks)"=w957, "Interlace ON/OFF"="Interlace", "Number Interlace Cycles"="Number Interlace Sets", "Interlace Off Parameters"=w952) -> ("error out"=w962:errorcluster)  [unwired: 1 out]
        n581 = Build Array(w959, w958, w957) -> (w950:u32[])
        n582 = Split 1D Array(array=w950, index="Number Interlace Sets") -> (first subarray=w960:u32[])  [unwired: 1 out]
        n583 = Index Array(array=w950, index=w948) -> (element=w949:u32)
        n584 = Add Array Elements(numeric array=w960) -> (sum=w954:u32)
        n585 = Select(t=w954, s="Interlace", f=w949) -> (s? t:f=→"Total Counts (ticks)":u32)
      }
      event "Reset Feedback": Value Change {
        n586 = event-data() -> ()  [unwired: 7 out]
        n587 = Unbundle By Name("Reset Feedback") -> ("Set 1"=w967:bool, "Set 2"=w966:bool)
        n588 = xnode "Read/Write Control"("FPGA VI Reference In"=w969, "error in"=w964, "FB Reset Set 1"=w967, "FB Reset Set 2"=w966) -> ("error out"=w965:errorcluster)  [unwired: 1 out]
      }
      event "PID Gains": Value Change {
        n589 = event-data() -> ()  [unwired: 7 out]
        n590 = Unbundle By Name("PID Gains") -> ("Set 1"=w973:T14, "Set 2"=w972:T14)
        n591 = xnode "Read/Write Control"("FPGA VI Reference In"=w974, "error in"=w970, "FB Gains Set 1"=w973, "FB Gains Set 2"=w972) -> ("error out"=w971:errorcluster)  [unwired: 1 out]
      }
      event "AI2 to Setpoint", "Trap Intensity\nSetpoints (V)": Value Change {
        n592 = event-data() -> ()  [unwired: 7 out]
        n593 = xnode "Read/Write Control"("FPGA VI Reference In"=w980, "error in"=w976) -> ("FPGA VI Reference Out"=w979:T19, "error out"=w978:errorcluster, "AI2 Y Sum Set 1"=w987:i16, "AI2 Y Sum Set 2"=w986:i16)
        n594 = Cluster To Array(cluster="AI2 to Setpoint") -> (array=w990:bool[])
        n595 = local read "AI2 (V)"() -> (w988:cluster{"Set 1":dbl, "Set 2":dbl})
        n596 = Or Array Elements(Boolean array=w990) -> (logical OR=w991:bool)
        n597 = Bundle By Name(cluster=w988, "Set 1"=w987, "Set 2"=w986) -> (w985:cluster{"Set 1":dbl, "Set 2":dbl})
        n598 = Divide(x=w985, y=3276.7) -> (x/y=w984:cluster{"Set 1":dbl, "Set 2":dbl})
        "AI2 (V)" <- w984
        n599 = case shown="True" w991 {
          tunnel: [w994 w1011] -> w983
          tunnel: "AI2 to Setpoint" -> [_ w1007]
          tunnel: "Trap Intensity\nSetpoints (V)" -> [w995 w1010]
          tunnel: w984 -> [_ w1004]
          frame False {
            n600 = Multiply(x=3276.7, y=w995) -> (x*y=w996:cluster{"Set 1":dbl, "Set 2":dbl})
            n601 = To Word Integer(number=w996) -> (16bit integer=w994:cluster{"Set 1":i16, "Set 2":i16})
          }
          frame True {
            n602 = Unbundle By Name(w1004) -> ("Set 1"=w1003:dbl, "Set 2"=w1002:dbl)
            n603 = Unbundle By Name(w1010) -> ("Set 1"=w1009:dbl, "Set 2"=w1008:dbl)
            n604 = Unbundle By Name(w1007) -> ("Set 1"=w1006:bool, "Set 2"=w1005:bool)
            n605 = Select(t=w1003, s=w1006, f=w1009) -> (s? t:f=w1001:dbl)
            n606 = Select(t=w1002, s=w1005, f=w1008) -> (s? t:f=w1000:dbl)
            n607 = Bundle By Name(cluster=w1010, "Set 1"=w1001, "Set 2"=w1000) -> (w998:cluster{"Set 1":dbl, "Set 2":dbl})
            n608 = local write "Trap Intensity\nSetpoints (V)"(w998) -> ()
            n609 = Multiply(x=3276.7, y=w998) -> (x*y=w999:cluster{"Set 1":dbl, "Set 2":dbl})
            n610 = To Word Integer(number=w999) -> (16bit integer=w1011:cluster{"Set 1":i16, "Set 2":i16})
          }
        }
        n611 = Unbundle By Name(w983) -> ("Set 1"=w982:i16, "Set 2"=w981:i16)
        n612 = xnode "Read/Write Control"("FPGA VI Reference In"=w979, "error in"=w978, "FB Setpoint Set 1"=w982, "FB Setpoint Set 2"=w981) -> ("error out"=w977:errorcluster)  [unwired: 1 out]
      }
      event "Invert GI": Value Change {
        n613 = event-data() -> ()  [unwired: 7 out]
        n614 = xnode "Read/Write Control"("FPGA VI Reference In"=w1016, "error in"=w1014, "Invert GI"="Invert GI", "Invert GI 2"="Invert GI") -> ("error out"=w1015:errorcluster)  [unwired: 1 out]
      }
      event "Green FB Setpoint (mV)", "Green FB Gains", "Green FB On/Off", "Current When FB OFF (%)", "Green int current ON count adj": Value Change {
        n615 = event-data() -> ()  [unwired: 7 out]
        n616 = local read "Green FB Setpoint (mV)"() -> (w1023:dbl)
        n617 = local read "Current When FB OFF (%)"() -> (w1026:dbl)
        n618 = Multiply(x=w1023, y=3.2767) -> (x*y=w1022:dbl)
        n619 = Multiply(x=w1026, y=655.35) -> (x*y=w1027:dbl)
        n620 = To Unsigned Word Integer(number=w1027) -> (unsigned 16bit integer=w1025:u16)
        n621 = local read "Green int current ON count adj"() -> (w1030:u32)
        n622 = local read "Green FB Gains"() -> (w1029:T14)
        n623 = local read "Green Laser ON/Interlacing"() -> (w1020:bool)
        n624 = local read "Green laser mode"() -> (w1019:enum32{"Laser ON", "Laser OFF", "Interlace"})
        n625 = local read "Green FB On/Off"() -> (w1031:bool)
        n626 = Equal?(x=w1019, y=enum32{"Laser ON", "Laser OFF", "Interlace"}."Interlace") -> (x = y?=w1017:bool)
        n627 = Compound Arithmetic op=AND(w1017, w1031, w1020) -> (w1021:bool)
        n628 = xnode "Read/Write Control"("FPGA VI Reference In"=w1034, "error in"=w1033, "Green FB Setpoint"=w1022, "Green FB On/Off"=w1021, "Current Out"=w1025, "Green int current ON count adj"=w1030, "Green FB Gains"=w1029) -> ("error out"=w1032:errorcluster)  [unwired: 1 out]
      }
      event "Green laser mode", "Green Laser ON/Interlacing": Value Change {
        n629 = event-data() -> ()  [unwired: 7 out]
        n630 = case shown="True" "Green Laser ON/Interlacing" {
          tunnel: "Green laser mode" -> [_ w1048]
          tunnel: [enum32{"Laser ON", "Laser OFF", "Interlace"}."Laser OFF" ("Green laser mode") w1048] -> w1036
          tunnel: [FALSE w1044] -> w1035
          frame False {
          }
          frame True {
            n631 = local read "Green FB On/Off"() -> (w1045:bool)
            n632 = Equal?(x=w1048, y=enum32{"Laser ON", "Laser OFF", "Interlace"}."Interlace") -> (x = y?=w1046:bool)
            n633 = And(x=w1046, y=w1045) -> (x .and. y?=w1044:bool)
          }
        }
        n634 = xnode "Read/Write Control"("FPGA VI Reference In"=w1041, "error in"=w1039, "Operating Mode"=w1036, "Operating Mode 2"=w1036, "Green FB On/Off"=w1035) -> ("error out"=w1040:errorcluster)  [unwired: 1 out]
      }
      event "- phase (APD 1 Gate)", "+ phase (APD 1 Gate)": Value Change {
        n635 = event-data() -> ()  [unwired: 7 out]
        n636 = local read "Phase Adj. (APD 1 Gate)"() -> (w1049:i16)
        n637 = Negate(x=w1049) -> (-x=w1057:i16)
        n638 = Select(t=w1057, s="- phase (APD 1 Gate)", f=w1049) -> (s? t:f=w1056:i16)
        n639 = Or(x="- phase (APD 1 Gate)", y="+ phase (APD 1 Gate)") -> (x .or. y?=w1052:bool)
        n640 = xnode "Read/Write Control"("FPGA VI Reference In"=w1059, "error in"=w1058, "Phase count adjustment (APD 1 Gate)"=w1056) -> ("FPGA VI Reference Out"=w1054:T19, "error out"=w1055:errorcluster)
        n641 = xnode "Read/Write Control"("FPGA VI Reference In"=w1054, "error in"=w1055, "+ phase (APD 1 Gate)"=w1052) -> ("error out"=w1053:errorcluster)  [unwired: 1 out]
      }
      event "+ phase (APD 2 Gate)", "- phase (APD 2 Gate)": Value Change {
        n642 = event-data() -> ()  [unwired: 7 out]
        n643 = local read "Phase Adj. (APD 2 Gate)"() -> (w1060:i16)
        n644 = Negate(x=w1060) -> (-x=w1068:i16)
        n645 = Select(t=w1068, s="- phase (APD 2 Gate)", f=w1060) -> (s? t:f=w1067:i16)
        n646 = Or(x="- phase (APD 2 Gate)", y="+ phase (APD 2 Gate)") -> (x .or. y?=w1063:bool)
        n647 = xnode "Read/Write Control"("FPGA VI Reference In"=w1070, "error in"=w1069, "Phase count adjustment (APD 2 Gate)"=w1067) -> ("FPGA VI Reference Out"=w1065:T19, "error out"=w1066:errorcluster)
        n648 = xnode "Read/Write Control"("FPGA VI Reference In"=w1065, "error in"=w1066, "+ phase (APD 2 Gate)"=w1063) -> ("error out"=w1064:errorcluster)  [unwired: 1 out]
      }
      event "Phase Adj. (APD Acq)", "+ phase (APD Acq)", "- phase (APD Acq)": Value Change {
        n649 = event-data() -> ()  [unwired: 7 out]
        n650 = local read "Phase Adj. (APD Acq)"() -> (w1073:i16)
        n651 = Negate(x=w1073) -> (-x=w1079:i16)
        n652 = Select(t=w1079, s="+ phase (APD Acq)", f=w1073) -> (s? t:f=w1078:i16)
        n653 = Or(x="+ phase (APD Acq)", y="- phase (APD Acq)") -> (x .or. y?=w1074:bool)
        n654 = xnode "Read/Write Control"("FPGA VI Reference In"=w1081, "error in"=w1080, "Phase Count Adjustment (APD Acq)"=w1078) -> ("FPGA VI Reference Out"=w1076:T19, "error out"=w1077:errorcluster)
        n655 = xnode "Read/Write Control"("FPGA VI Reference In"=w1076, "error in"=w1077, "+ phase (APD Acq)"=w1074) -> ("error out"=w1075:errorcluster)  [unwired: 1 out]
      }
      event "Phase adj. (GI)", "+ phase (GI)", "- phase (GI)": Value Change {
        n656 = event-data() -> ()  [unwired: 7 out]
        n657 = Negate(x="Phase adj. (GI)") -> (-x=w1090:i16)
        n658 = Select(t=w1090, s="+ phase (GI)", f="Phase adj. (GI)") -> (s? t:f=w1089:i16)
        n659 = Or(x="+ phase (GI)", y="- phase (GI)") -> (x .or. y?=w1085:bool)
        n660 = xnode "Read/Write Control"("FPGA VI Reference In"=w1092, "error in"=w1091, "Phase count adjustment (GI)"=w1089) -> ("FPGA VI Reference Out"=w1087:T19, "error out"=w1088:errorcluster)
        n661 = xnode "Read/Write Control"("FPGA VI Reference In"=w1087, "error in"=w1088, "+ phase (GI)"=w1085) -> ("error out"=w1086:errorcluster)  [unwired: 1 out]
      }
      event "Phase adj. (GI) 2", "+ phase (GI) 2", "- phase (GI) 2": Value Change {
        n662 = event-data() -> ()  [unwired: 7 out]
        n663 = Negate(x="Phase adj. (GI) 2") -> (-x=w1101:i16)
        n664 = Select(t=w1101, s="+ phase (GI) 2", f="Phase adj. (GI) 2") -> (s? t:f=w1100:i16)
        n665 = Or(x="+ phase (GI) 2", y="- phase (GI) 2") -> (x .or. y?=w1096:bool)
        n666 = xnode "Read/Write Control"("FPGA VI Reference In"=w1103, "error in"=w1102, "Phase count adjustment (GI) 2"=w1100) -> ("FPGA VI Reference Out"=w1098:T19, "error out"=w1099:errorcluster)
        n667 = xnode "Read/Write Control"("FPGA VI Reference In"=w1098, "error in"=w1099, "+ phase (GI) 2"=w1096) -> ("error out"=w1097:errorcluster)  [unwired: 1 out]
      }
      event "Phase adj. (Green FB)", "- phase (Green FB)", "+ phase (Green FB)": Value Change {
        n668 = event-data() -> ()  [unwired: 7 out]
        n669 = Negate(x="Phase adj. (Green FB)") -> (-x=w1112:i16)
        n670 = Select(t=w1112, s="+ phase (Green FB)", f="Phase adj. (Green FB)") -> (s? t:f=w1111:i16)
        n671 = Or(x="+ phase (Green FB)", y="- phase (Green FB)") -> (x .or. y?=w1107:bool)
        n672 = xnode "Read/Write Control"("FPGA VI Reference In"=w1114, "error in"=w1113, "Phase count adjustment (Green FB)"=w1111) -> ("FPGA VI Reference Out"=w1109:T19, "error out"=w1110:errorcluster)
        n673 = xnode "Read/Write Control"("FPGA VI Reference In"=w1109, "error in"=w1110, "+ phase (Green FB)"=w1107) -> ("error out"=w1108:errorcluster)  [unwired: 1 out]
      }
      event "Invert APD Gate", "APD Gate ON Count", "APD Gate OFF Count", "APD Gate", "APD Integration Time (s)", "APD 1 AO Mult.", "APD 2 AO Mult.": Value Change {
        n674 = event-data() -> ()  [unwired: 7 out]
        n675 = local read "APD Integration Time (s)"() -> (w1115:dbl)
        n676 = local read "APD Gate ON Count"() -> (w1128:u32)
        n677 = local read "APD Gate OFF Count"() -> (w1127:u32)
        n678 = local read "Invert APD Gate"() -> (w1129:bool)
        n679 = local read "APD Gate"() -> (w1126:enum32{"ON", "OFF", "Interlace"})
        n680 = Multiply(x=w1115, y=40000000.0) -> (x*y=w1124:dbl)
        n681 = Reciprocal(x=w1115) -> (1/x=→"APD Acq Rate (Hz)":dbl)
        n682 = To Unsigned Long Integer(number=w1124) -> (unsigned 32bit integer=w1123:u32)
        n683 = local read "DMA Update Period (s)"() -> (w1116:dbl)
        n684 = Divide(x=w1116, y=w1115) -> (x/y=w1119:dbl)
        n685 = local read "APD 1 AO Mult."() -> (w1121:i16)
        n686 = local read "APD 2 AO Mult."() -> (w1120:i16)
        n687 = Multiply(x=2.0, y=w1119) -> (x*y=w1118:dbl)
        n688 = local write "APD Samples/FIFO Acq."(w1119) -> ()
        n689 = local write "APD Elements/DMA read"(w1118) -> ()
        n690 = xnode "Read/Write Control"("FPGA VI Reference In"=w1132, "error in"=w1131, "Invert APD Gate"=w1129, "APD Gate ON Count"=w1128, "APD Gate OFF Count"=w1127, "APD Acq Rate Count"=w1123, "APD Gate Operating Mode"=w1126, "APD 1 AO scale factor"=w1121, "APD 2 AO scale factor"=w1120) -> ("error out"=w1130:errorcluster)  [unwired: 1 out]
      }
      event "GI Frequency, ON count", "Green FB Count", "GI Frequency, OFF count": Value Change {
        n691 = event-data() -> ()  [unwired: 7 out]
        n692 = xnode "Read/Write Control"("FPGA VI Reference In"=w1138, "error in"=w1136, "Green interlace ON count"="GI Frequency, ON count", "Green interlace OFF count"="GI Frequency, OFF count", "Green interlace ON count 2"="GI Frequency, ON count", "Green interlace OFF count 2"="GI Frequency, OFF count", "Green FB Count"="Green FB Count") -> ("error out"=w1137:errorcluster)  [unwired: 1 out]
      }
      event "Number of F/B Scans (AOD)", "Scan Speed (nm/s)", "Scan BD", "Initial delta (MHz)", "Step Size (nm)", "Scan Range (nm)": Value Change {
        w1200 = 123.0  # AOM cal (nm/MHz)
        n693 = event-data() -> ()  [unwired: 7 out]
        n694 = local read "BD 1 Frequency 1 (MHz)"() -> (w1183:dbl)
        n695 = local read "AOM X Cal (nm/MHz)"() -> (w1175:dbl)
        n696 = local read "X RF Frequency Limits (MHz)"() -> (w1187:T16)
        n697 = local read "Y RF Frequency Limits (MHz)"() -> (w1184:T16)
        n698 = local read "BD 2 Frequency 1 (MHz)"() -> (w1189:dbl)
        n699 = Negate(x="Scan Range (nm)") -> (-x=w1153:dbl)
        n700 = Divide(x=w1153, y=w1175) -> (x/y=w1157:dbl)
        n701 = Select(t=w1187, s="Scan BD", f=w1184) -> (s? t:f=w1186:T16)
        n702 = Select(t=w1183, s="Scan BD", f=w1189) -> (s? t:f=w1188:dbl)
        n703 = Unbundle By Name(w1186) -> ("Maximum"=w1195:dbl, "Minimum"=w1194:dbl)
        n704 = Add(x=w1157, y=w1188) -> (x+y=w1192:dbl)
        n705 = Divide(x=w1153, y="Step Size (nm)") -> (x/y=w1172:dbl)
        n706 = Divide(x="Step Size (nm)", y=w1175) -> (x/y=w1181:dbl)
        n707 = Absolute Value(x=w1172) -> (abs(x)=w1156:dbl)
        n708 = Sign(1:w1153) -> (0:w1154:dbl)
        n709 = In Range and Coerce(upper limit=w1195, x=w1192, lower limit=w1194) -> (coerced(x)=w1191:dbl, In Range?=w1193:bool)
        n710 = To Unsigned Quad Integer(1:w1156) -> (0:w1171:u64)
        "Scan steps (AOD)" <- w1171
        n711 = call "IR AOM freq to word.vi"("Frequency In (MHz)"=w1181) -> ("Frequency Word Out (double)"=w1178:dbl)
        n712 = Multiply(x=w1154, y=w1178) -> (x*y=w1155:dbl)
        n713 = Subtract(x=w1192, y=w1191) -> (x-y=w1190:dbl)
        n714 = To Quad Integer(1:w1155) -> (0:w1177:i64)
        "Incr. int (AOD)" <- w1177
        n715 = Subtract(x=w1157, y=w1190) -> (x-y=w1176:dbl)
        "Scan Range (MHz)" <- w1176
        n716 = Select(t=w1157, s=w1193, f=w1176) -> (s? t:f=w1196:dbl)
        n717 = Multiply(x=w1176, y=w1175) -> (x*y=w1174:dbl)
        n718 = Decrement(x=w1171) -> (x-1=w1224:u64)
        n719 = Negate(x=w1174) -> (-x=w1170:dbl)
        n720 = local write "Scan Range (nm)"(w1170) -> ()
        n721 = Divide(x=w1196, y=w1224) -> (x/y=w1180:dbl)
        "Scan Increment (MHz)" <- w1180
        n722 = call "IR AOM freq to word.vi"("Frequency In (MHz)"=w1180) -> ("Frequency Word Out (double)"=w1179:dbl)
        n723 = Divide(x="Step Size (nm)", y="Scan Speed (nm/s)") -> (x/y=w1167:dbl)
        n724 = To Quad Integer(1:w1179) -> ()  [unwired: 1 out]
        n725 = local read "Number Interlace Sets"() -> (w1151:u8)
        n726 = local read "AI Count (ticks)"() -> (w1152:u32)
        n727 = local read "Total Counts (ticks)"() -> (w1150:u32)
        n728 = local read "# Samples/trap"() -> (w1182:u32)
        n729 = Multiply(x=w1152, y=w1151) -> (x*y=w1149:u32)
        n730 = Divide(x=w1150, y=w1149) -> (x/y=w1148:dbl)
        n731 = Select(t=w1183, s="Scan BD", f=w1189) -> (s? t:f=w1221:dbl)
        "Initial freq. (MHz)" <- w1221
        n732 = Add(x=w1196, y=w1221) -> (x+y=→"Final freq. (MHz)":dbl)
        n733 = Divide(x=w1150, y=40000000.0) -> (x/y=w1166:dbl)
        n734 = Divide(x=w1167, y=w1166) -> (x/y=w1165:dbl)
        n735 = To Unsigned Quad Integer(1:w1165) -> (0:w1140:u64)
        n736 = Quotient & Remainder(x=w1140, y=u64 2) -> (x-y*floor(x/y)=w1144:u64)  [unwired: 1 out]
        n737 = Equal?(x=w1144, y=u64 0) -> (x = y?=w1142:bool)
        n738 = Decrement(x=w1140) -> (x-1=w1141:u64)
        n739 = Select(t=w1140, s=w1142, f=w1141) -> (s? t:f=w1139:u64)
        "Cycles/step (AOD)" <- w1139
        n740 = xnode "Read/Write Control"("FPGA VI Reference In"=w1232, "error in"=w1231, "Scan steps"=w1171, "Number of scans"="Number of F/B Scans (AOD)", "Cycles per step"=w1139, "Scan freq.  increment"=w1177, "Scan BD"="Scan BD") -> ("error out"=w1230:errorcluster)  [unwired: 1 out]
        n741 = Multiply(x=w1171, y=w1139) -> (x*y=w1225:u64)
        n742 = Multiply(x=w1225, y=u64 2) -> (x*y=w1147:u64)
        n743 = Multiply(x=w1148, y=w1147) -> (x*y=w1146:dbl)
        "Data points/scan (f/b)" <- w1146
        n744 = Multiply(x=w1146, y="Number of F/B Scans (AOD)") -> (x*y=w1228:dbl)
        "Data points/scans" <- w1228
        n745 = Divide(x=w1228, y=w1182) -> (x/y=→"N sets should be saved":dbl)
        n746 = Multiply(x=w1225, y=w1166) -> (x*y=w1164:dbl)
        "Time/Scan (s) (AOD)" <- w1164
        n747 = Select(t=w1196, s="Scan BD", f=0.0) -> (s? t:f=w1222:dbl)
        n748 = Select(t=0.0, s="Scan BD", f=w1196) -> (s? t:f=w1218:dbl)
        n749 = local read "BD 2 Frequency 2 (MHz)"() -> (w1214:dbl)
        n750 = local read "BD 1 Frequency 2 (MHz)"() -> (w1217:dbl)
        n751 = Add(x=w1218, y=w1189) -> (x+y=w1215:dbl)
        n752 = Add(x=w1183, y=w1222) -> (x+y=w1216:dbl)
        n753 = Multiply(x=w1164, y=2.0) -> (x*y=w1163:dbl)
        n754 = Multiply(x=w1163, y="Number of F/B Scans (AOD)") -> (x*y=w1160:dbl)
        n755 = Divide(x=w1160, y=60.0) -> (x/y=→"Time to Finish All (min)":dbl)
        n756 = Add(x="Trap 2 Bead Size (nm)", y="Trap 1 Bead Size (nm)") -> (x+y=w1204:dbl)
        n757 = local read "Initial delta (MHz)"() -> (w1201:dbl)
        n758 = Divide(x=w1204, y=2.0) -> (x/y=w1198:dbl)
        n759 = Subtract(x=w1215, y=w1214) -> (x-y=w1212:dbl)
        n760 = Subtract(x=w1216, y=w1217) -> (x-y=w1213:dbl)
        n761 = Square(x=w1212) -> (x^2=w1211:dbl)
        n762 = Square(x=w1213) -> (x^2=w1210:dbl)
        n763 = Add(x=w1210, y=w1211) -> (x+y=w1209:dbl)
        n764 = Square Root(x=w1209) -> (sqrt(x)=w1208:dbl)
        "Final delta (MHz)" <- w1208
        n765 = Multiply(x=w1200, y=w1208) -> (x*y=w1207:dbl)
        n766 = Multiply(x=w1201, y=w1200) -> (x*y=w1199:dbl)
        n767 = Subtract(x=w1199, y=w1198) -> (x-y=→"Initial sep (nm)":dbl)
        n768 = Subtract(x=w1207, y=w1198) -> (x-y=→"Final sep (nm)":dbl)
      }
      event "Raster Scanning...": Value Change {
        n769 = event-data() -> ("NewVal"=w1233:bool)  [unwired: 6 out]
        n770 = case shown="True" w1233 {
          frame False {
          }
          frame True {
            n771 = property on="BD 1 Frequency 1 (MHz)" class="DigNum (strict)"("Val(Sgnl)"=65.0 ("Value (Signaling)")) -> ()  [unwired: 2 in, 2 out]
          }
        }
      }
      event "Freq or Amp switch first", "Swap F1 and F2", "Freq switch delay", "Amp switch delay": Value Change {
        n772 = event-data() -> ()  [unwired: 7 out]
        n773 = local read "Freq or Amp switch first"() -> (w1235:bool)
        n774 = local read "Amp switch delay"() -> (w1236:u16)
        n775 = local read "Freq switch delay"() -> (w1238:u16)
        n776 = local read "Swap F1 and F2"() -> (w1237:bool)
        n777 = xnode "Read/Write Control"("FPGA VI Reference In"=w1241, "error in"=w1240, "Freq switch delay"=w1238, "Swap F1 and F2"=w1237, "Amp switch delay"=w1236, "Freq or Amp switch first"=w1235) -> ("error out"=w1239:errorcluster)  [unwired: 1 out]
      }
      event "Scan steps (MCL)", "Number of scans (MCL)", "Scan Range (V)\n(of steps)", "2D or 1D Scan", "N APD Samp/step", "Fast Scan Dir", "Continuous MCL Scanning", "Scan lines (y)": Value Change {
        w1243 = 32767.0 ("y")
        n778 = event-data() -> ()  [unwired: 7 out]
        n779 = Select(t="Scan lines (y)", s="2D or 1D Scan", f="Number of scans (MCL)") -> (s? t:f=w1248:u64)
        n780 = Decrement(x="Scan steps (MCL)") -> (x-1=w1264:u64)
        n781 = Divide(x="Scan Range (V)\n(of steps)", y=w1264) -> (x/y=w1263:dbl)
        "Desired Scan Incr (V)" <- w1263
        n782 = local read "APD Integration Time (s)"() -> (w1256:dbl)
        n783 = Multiply(x=w1263, y=w1243) -> (x*y=w1272:dbl)
        n784 = Divide(x=w1272, y=10.0) -> (x/y=w1262:dbl)
        "Desired incr (int)" <- w1262
        n785 = local read "Update Count (MCL)"() -> (w1268:u32)
        n786 = Round Toward -Infinity(1:w1262) -> (0:w1271:dbl)
        n787 = To Word Integer(number=w1271) -> (16bit integer=w1246:i16)
        "Actual Incr. int (MCL)" <- w1246
        n788 = Multiply(x=w1256, y=40000000.0) -> (x*y=w1269:dbl)
        n789 = Divide(x=w1269, y=w1268) -> (x/y=w1267:dbl)
        n790 = Multiply(x=i16 10, y=w1246) -> (x*y=w1244:i16)
        n791 = Multiply(x="N APD Samp/step", y=w1267) -> (x*y=w1266:dbl)
        "Cycles/step (MCL)" <- w1266
        n792 = Divide(x=w1244, y=w1243) -> (x/y=→"Actual MCL Inc (V)":dbl)
        n793 = Multiply(x="N APD Samp/step", y="Scan steps (MCL)") -> (x*y=w1258:dbl)
        n794 = local read "APD Samples/FIFO Acq."() -> (w1255:dbl)
        n795 = Multiply(x=w1258, y=u64 2) -> (x*y=w1257:dbl)
        "Data points/scan (f+b)" <- w1257
        n796 = Multiply(x=w1257, y=w1248) -> (x*y=w1275:dbl)
        "Data points/scans (MCL)" <- w1275
        n797 = Multiply(x=w1256, y=w1257) -> (x*y=w1249:dbl)
        "Time/f+b scan (s) (MCL)" <- w1249
        n798 = Divide(x=w1275, y=w1255) -> (x/y=→"N sets should be saved (MCL)":dbl)
        n799 = Multiply(x=w1249, y=w1248) -> (x*y=→"Total Time (s)":dbl)
        n800 = Not(x="Fast Scan Dir") -> (.not. x?=w1253:bool)
        n801 = xnode "Read/Write Control"("FPGA VI Reference In"=w1279, "error in"=w1278, "Scan steps (MCL)"="Scan steps (MCL)", "Number of scans (MCL)"=w1248, "Cycles per step (MCL)"=w1266, "Scan freq.  increment (MCL)"=w1246, "1D or 2D Scan?"="2D or 1D Scan", "MCL Scan Axis"=w1253, "Cont. Scan (MCL)"="Continuous MCL Scanning") -> ("error out"=w1277:errorcluster)  [unwired: 1 out]
      }
      event "Read Cal": Value Change {
        w1281 = 1000.0 ("y")
        n802 = event-data() -> ()  [unwired: 7 out]
        n803 = local read "Save file name"() -> (w1306:path)
        n804 = local write "Read Cal"(FALSE ("Read Cal")) -> ()
        n805 = Strip Path(path=w1306) -> (stripped path=w1305:path)  [unwired: 1 out]
        n806 = Path To String(path=w1305) -> (string=w1304:string)
        n807 = Concatenate Strings(w1304, "\\current.cal" ("string")) -> (w1302:string)
        n808 = String To Path(string=w1302) -> (path=w1301:path)
        n809 = Open/Create/Replace File(file path (use dialog)=w1301, operation (0:open)=T23."open", access (0:read/write)=enum16{"read/write", "read-only", "write-only"}."read-only") -> (refnum out=w1309:refnum<file>, error out=w1295:errorcluster)  [unwired: 1 in, 3 out]
        n810 = Deny Access(4:w1295, 7:w1309) -> (0:w1294:errorcluster, 3:w1300:refnum<file>)  [unwired: 1 out]
        n811 = Read from Binary File(5:0.0, 8:w1294, 9:T29."big-endian, network order" ("byte order (0:big-endian, network order)"), 10:-1 ("count (1)"), 11:w1300) -> (0:w1293:errorcluster, 2:w1291:dbl[], 3:w1296:refnum<file>)  [unwired: 2 out]
        n812 = Array To Cluster(array=w1291) -> (cluster=w1290:T31)
        n813 = Unbundle(w1290) -> ("[0]"=w1289:dbl, "[1]"=w1288:dbl, "[2]"=w1287:dbl, "[3]"=w1286:dbl, "[4]"=w1285:dbl, "[5]"=w1284:dbl)
        n814 = Close File(refnum=w1296, error in=w1293) -> (error out=→"Read cal error":errorcluster)  [unwired: 1 out]
        n815 = Multiply(x=w1284, y=w1281) -> (x*y=w1282:dbl)
        n816 = local write "T2 kappa_x (pN/nm)"(w1286) -> ()
        n817 = local write "T1 kappa_x (pN/nm)"(w1287) -> ()
        n818 = local write "T1 alpha_x (nm/V)"(w1289) -> ()
        n819 = local write "T2 alpha_x (nm/V)"(w1288) -> ()
        n820 = Multiply(x=w1285, y=w1281) -> (x*y=w1283:dbl)
        n821 = local write "T1 offset_x (mV)"(w1283) -> ()
        n822 = local write "T2 offset_x (mV)"(w1282) -> ()
      }
      event "Abort MCL Scan": Value Change {
        n823 = event-data() -> ()  [unwired: 7 out]
        n824 = local write "MCL Scanning"(FALSE ("MCL Scanning")) -> ()
        n825 = xnode "Read/Write Control"("FPGA VI Reference In"=w1314, "error in"=w1313, "Abort scan (MCL)"="Abort MCL Scan") -> ("error out"=w1312:errorcluster)  [unwired: 1 out]
      }
      event "Update Count (MCL)": Value Change {
        n826 = event-data() -> ()  [unwired: 7 out]
        n827 = xnode "Read/Write Control"("FPGA VI Reference In"=w1318, "error in"=w1317, "MCL count"="Update Count (MCL)") -> ("error out"=w1316:errorcluster)  [unwired: 1 out]
      }
      event "Phase adjust (MCL)", "+ phase (MCL)", "- phase (MCL)": Value Change {
        n828 = event-data() -> ()  [unwired: 7 out]
        n829 = Negate(x="Phase adjust (MCL)") -> (-x=w1327:i16)
        n830 = Select(t=w1327, s="- phase (MCL)", f="Phase adjust (MCL)") -> (s? t:f=w1325:i16)
        n831 = Or(x="- phase (MCL)", y="+ phase (MCL)") -> (x .or. y?=w1320:bool)
        n832 = xnode "Read/Write Control"("FPGA VI Reference In"=w1329, "error in"=w1328, "Phase count adjustment (MCL)"=w1325) -> ("FPGA VI Reference Out"=w1321:T19, "error out"=w1322:errorcluster)
        n833 = xnode "Read/Write Control"("FPGA VI Reference In"=w1321, "error in"=w1322, "+ phase (MCL)"=w1320) -> ("error out"=w1319:errorcluster)  [unwired: 1 out]
      }
      event "Abort AOD Scan": Value Change {
        n834 = event-data() -> ()  [unwired: 7 out]
        n835 = xnode "Read/Write Control"("FPGA VI Reference In"=w1333, "error in"=w1332, "Abort scan"="Abort AOD Scan") -> ("error out"=w1331:errorcluster)  [unwired: 1 out]
      }
      event "Continuous AOD Scanning": Value Change {
        n836 = event-data() -> ()  [unwired: 7 out]
        n837 = xnode "Read/Write Control"("FPGA VI Reference In"=w1337, "error in"=w1336, "Cont. Scan"="Continuous AOD Scanning") -> ("error out"=w1335:errorcluster)  [unwired: 1 out]
      }
      event "Index": Value Change {
        n838 = event-data() -> ()  [unwired: 7 out]
        n839 = call "Create new save file.vi"("Insert"="", "Ext"=".dat" ("string"), "Index In"="Index") -> ("Path Out"=→"Save file name":path, "Index Out"=w1338:dbl)
        "Save index" <- w1338
        n840 = local write "Index"(w1338) -> ()
      }
      event "AO1", "AO2": Value Change {
        w1353 = 10.0 ("y")
        w1352 = 32767.0 ("y")
        n841 = event-data() -> ()  [unwired: 7 out]
        n842 = local read "AO2"() -> (w1351:dbl)
        n843 = local read "AO1"() -> (w1348:dbl)
        n844 = Multiply(x=w1348, y=w1352) -> (x*y=w1347:dbl)
        n845 = Multiply(x=w1351, y=w1352) -> (x*y=w1350:dbl)
        n846 = Divide(x=w1347, y=w1353) -> (x/y=w1346:dbl)
        n847 = Divide(x=w1350, y=w1353) -> (x/y=w1349:dbl)
        n848 = To Word Integer(number=w1346) -> (16bit integer=w1354:i16)
        n849 = To Word Integer(number=w1349) -> (16bit integer=w1355:i16)
        n850 = xnode "Read/Write Control"("FPGA VI Reference In"=w1345, "error in"=w1344, "AO1"=w1354, "AO2"=w1355) -> ("error out"=w1343:errorcluster)  [unwired: 1 out]
      }
      event "Inject Bottom": Value Change {
        n851 = event-data() -> ()  [unwired: 7 out]
        n852 = disable-structure shown="Enabled" {
          disable-tunnel: "Inject Bottom" -> [w1357 w1397]
          frame Disabled {
            n853 = local read "Chemyx Syringe Pump Serial Port"() -> (w1358:refnum<visa-resource-name>)
            n854 = local read "Pump write delay (ms)"() -> (w1359:dbl)
            n855 = case shown="True" w1357 {
              tunnel: w1359 -> [w1365 w1379]
              tunnel: w1358 -> [w1362 w1378]
              frame False {
                n856 = flat-sequence {
                  tunnel: w1362 -> [w1366]
                  tunnel: [w1366] -> w1363
                  tunnel: w1365 -> [_]
                  tunnel: [w1369] -> w1364
                  tunnel: w1363 -> [w1369]
                  tunnel: w1364 -> [w1370]
                  tunnel: [w1370] -> w1360
                  tunnel: [w1372] -> w1361
                  tunnel: w1360 -> [w1372]
                  tunnel: w1361 -> [w1374]
                  frame #0 {
                    n857 = call "Write to pump.vi"("string"="enter pump1", "VISA resource name"=w1366) -> ()  [unwired: 1 out]
                  }
                  frame #1 {
                    n858 = Wait (ms)(milliseconds to wait="Pump pause delay (ms)") -> ()  [unwired: 1 out]
                  }
                  frame #2 {
                    n859 = call "Write to pump.vi"("string"="stop", "VISA resource name"=w1370) -> ()  [unwired: 1 out]
                  }
                  frame #3 {
                    n860 = Wait (ms)(milliseconds to wait=u32 500) -> ()  [unwired: 1 out]
                  }
                  frame #4 {
                    n861 = call "Write to pump.vi"("string"="stop", "VISA resource name"=w1374) -> ()  [unwired: 1 out]
                  }
                }
              }
              frame True {
                n862 = flat-sequence {
                  tunnel: w1378 -> [w1388]
                  tunnel: w1379 -> [w1383]
                  tunnel: w1379 -> [w1390]
                  tunnel: w1378 -> [w1391]
                  tunnel: [w1391] -> w1376
                  tunnel: [w1393] -> w1377
                  tunnel: w1376 -> [w1393]
                  tunnel: w1377 -> [w1395]
                  frame #0 {
                    n863 = local read "All Pump Parameters"() -> (w1382:T5)
                    n864 = Unbundle By Name(w1382) -> ("Pump 1"=w1389:T32)
                    n865 = call "Set pump parameters.vi"("Pump write delay (ms)"=w1383, "Volume (uL)"="Ch 2 Inject Volume (uL)", "Rate (uL/h)"="Ch 1 Inject Rate (ul/h)", "Units"=4.0, "Pump #"=1.0, "Pump Parameters In"=w1389, "VISA resource name"=w1388) -> ("Pump Parameters Out"=w1381:T32)  [unwired: 3 in]
                    n866 = Bundle By Name(cluster=w1382, "Pump 1"=w1381) -> (w1380:T5)
                    n867 = local write "All Pump Parameters"(w1380) -> ()
                  }
                  frame #1 {
                    n868 = Wait (ms)(milliseconds to wait=w1390) -> ()  [unwired: 1 out]
                  }
                  frame #2 {
                    n869 = call "Write to pump.vi"("string"="start", "VISA resource name"=w1391) -> ()  [unwired: 1 out]
                  }
                  frame #3 {
                    n870 = Wait (ms)(milliseconds to wait=u32 500) -> ()  [unwired: 1 out]
                  }
                  frame #4 {
                    n871 = call "Write to pump.vi"("string"="start", "VISA resource name"=w1395) -> ()  [unwired: 1 out]
                  }
                }
              }
            }
          }
          frame Enabled {
            n872 = call "hamilton_controller.vi"("Open?"=w1397, "valve"=enum16{"A", "B", "C", "D", "ALL"}."B", "action"=T20."MOVE VALVE") -> ()  [unwired: 8 in, 1 out]
          }
        }
      }
      event "Inject Top": Value Change {
        n873 = event-data() -> ()  [unwired: 7 out]
        n874 = disable-structure shown="Disabled" {
          disable-tunnel: "Inject Top" -> [_ w1441]
          frame Disabled {
            n875 = local read "Pump write delay (ms)"() -> (w1402:dbl)
            n876 = case shown="False" w1403 {
              tunnel: w1402 -> [w1409 w1423]
              tunnel: "Chemyx Syringe Pump Serial Port" -> [w1406 w1422]
              frame False {
                n877 = flat-sequence {
                  tunnel: w1406 -> [w1410]
                  tunnel: [w1410] -> w1407
                  tunnel: w1409 -> [_]
                  tunnel: [w1413] -> w1408
                  tunnel: w1407 -> [w1413]
                  tunnel: w1408 -> [w1414]
                  tunnel: [w1414] -> w1404
                  tunnel: [w1416] -> w1405
                  tunnel: w1404 -> [w1416]
                  tunnel: w1405 -> [w1418]
                  frame #0 {
                    n878 = call "Write to pump.vi"("string"="enter pump3", "VISA resource name"=w1410) -> ()  [unwired: 1 out]
                  }
                  frame #1 {
                    n879 = local read "Pump pause delay (ms)"() -> (w1412:u32)
                    n880 = Wait (ms)(milliseconds to wait=w1412) -> ()  [unwired: 1 out]
                  }
                  frame #2 {
                    n881 = call "Write to pump.vi"("string"="stop", "VISA resource name"=w1414) -> ()  [unwired: 1 out]
                  }
                  frame #3 {
                    n882 = Wait (ms)(milliseconds to wait=u32 0) -> ()  [unwired: 1 out]
                  }
                  frame #4 {
                    n883 = call "Write to pump.vi"("string"="stop", "VISA resource name"=w1418) -> ()  [unwired: 1 out]
                  }
                }
              }
              frame True {
                n884 = flat-sequence {
                  tunnel: w1422 -> [w1432]
                  tunnel: w1423 -> [w1427]
                  tunnel: w1423 -> [w1434]
                  tunnel: w1422 -> [w1435]
                  tunnel: [w1435] -> w1420
                  tunnel: [w1438] -> w1421
                  tunnel: w1420 -> [w1438]
                  tunnel: w1421 -> [w1439]
                  frame #0 {
                    n885 = local read "All Pump Parameters"() -> (w1426:T5)
                    n886 = Unbundle By Name(w1426) -> ("Pump 3"=w1433:T32)
                    n887 = call "Set pump parameters.vi"("Pump write delay (ms)"=w1427, "Volume (uL)"="Ch 3 Inject Volume (uL)", "Rate (uL/h)"="Ch 3 Inject Rate (ul/h)", "Units"=4.0, "Pump #"=3.0, "Pump Parameters In"=w1433, "VISA resource name"=w1432) -> ("Pump Parameters Out"=w1425:T32)  [unwired: 3 in]
                    n888 = Bundle By Name(cluster=w1426, "Pump 3"=w1425) -> (w1424:T5)
                    n889 = local write "All Pump Parameters"(w1424) -> ()
                  }
                  frame #1 {
                    n890 = Wait (ms)(milliseconds to wait=w1434) -> ()  [unwired: 1 out]
                  }
                  frame #2 {
                    n891 = call "Write to pump.vi"("string"="start", "VISA resource name"=w1435) -> ()  [unwired: 1 out]
                  }
                  frame #3 {
                    n892 = Wait (ms)(milliseconds to wait=u32 500) -> ()  [unwired: 1 out]
                  }
                  frame #4 {
                    n893 = call "Write to pump.vi"("string"="start", "VISA resource name"=w1439) -> ()  [unwired: 1 out]
                  }
                }
              }
            }
          }
          frame Enabled {
            n894 = call "hamilton_controller.vi"("Open?"=w1441, "valve"=enum16{"A", "B", "C", "D", "ALL"}."A", "action"=T20."MOVE VALVE") -> ()  [unwired: 8 in, 1 out]
          }
        }
      }
      event "Inject Valve B": Value Change {
        n895 = event-data() -> ()  [unwired: 7 out]
        n896 = disable-structure shown="Enabled" {
          disable-tunnel: "Inject Valve B" -> [w1445 w1465]
          frame Disabled {
            n897 = local read "Pump write delay (ms)"() -> (w1447:dbl)
            n898 = flat-sequence {
              tunnel: w1446 -> [w1460]
              tunnel: w1447 -> [w1456]
              tunnel: w1445 -> [_]
              tunnel: w1447 -> [w1462]
              tunnel: w1446 -> [w1463]
              frame #0 {
                n899 = local read "All Pump Parameters"() -> (w1455:T5)
                n900 = Multiply(x=60.0, y="Flush Center Ch Rate (ul/m)") -> (x*y=w1452:dbl)
                n901 = Unbundle By Name(w1455) -> ("Pump 2"=w1461:T32)
                n902 = call "Set pump parameters.vi"("Pump write delay (ms)"=w1456, "Volume (uL)"="Flush Center Ch Volume (uL)", "Rate (uL/h)"=w1452, "Units"=3.0, "Pump #"=2.0, "Pump Parameters In"=w1461, "VISA resource name"=w1460) -> ("Pump Parameters Out"=w1454:T32)  [unwired: 3 in]
                n903 = Bundle By Name(cluster=w1455, "Pump 2"=w1454) -> (w1453:T5)
                n904 = local write "All Pump Parameters"(w1453) -> ()
                n905 = Add(x="Flush Center Ch Volume (uL)", y="Total Volume\nFlushed (uL)") -> (x+y=w1449:dbl)
                n906 = local write "Total Volume\nFlushed (uL)"(w1449) -> ()
              }
              frame #1 {
                n907 = Wait (ms)(milliseconds to wait=w1462) -> ()  [unwired: 1 out]
              }
              frame #2 {
                n908 = call "Write to pump.vi"("string"="start", "VISA resource name"=w1463) -> ()  [unwired: 1 out]
              }
            }
            n909 = local read "Chemyx Syringe Pump Serial Port"() -> (w1446:refnum<visa-resource-name>)
          }
          frame Enabled {
            n910 = call "hamilton_controller.vi"("Open?"=w1465, "valve"=enum16{"A", "B", "C", "D", "ALL"}."B", "action"=T20."MOVE VALVE") -> ()  [unwired: 8 in, 1 out]
          }
        }
      }
      event "Sample Channel Flow": Value Change {
        n911 = event-data() -> ()  [unwired: 7 out]
        n912 = call "hamilton_controller.vi"("Open?"="Sample Channel Flow", "valve"=enum16{"A", "B", "C", "D", "ALL"}."C", "action"=T20."MOVE VALVE") -> ()  [unwired: 8 in, 1 out]
      }
      event "Flip Green Filter": Value Change {
        n913 = event-data() -> ()  [unwired: 7 out]
        n914 = Not(x="Flip Green Filter") -> (.not. x?=w1471:bool)
        n915 = local write "Flip Green Filter"(w1471) -> ()
        n916 = flat-sequence {
          tunnel: w1479 -> [w1484]
          tunnel: w1478 -> [w1483]
          tunnel: [w1481] -> w1476
          tunnel: [w1480] -> w1475
          tunnel: [w1486] -> w1474
          tunnel: w1476 -> [w1486]
          tunnel: [w1485] -> w1473
          tunnel: w1475 -> [w1485]
          tunnel: w1474 -> [w1490]
          tunnel: w1473 -> [w1489]
          tunnel: [w1488] -> w1477
          frame #0 {
            n917 = xnode "Read/Write Control"("FPGA VI Reference In"=w1484, "error in"=w1483, "Green Filter Flipper"=TRUE) -> ("FPGA VI Reference Out"=w1481:T19, "error out"=w1480:errorcluster)
          }
          frame #1 {
            n918 = Wait (ms)(milliseconds to wait=u32 100) -> ()  [unwired: 1 out]
          }
          frame #2 {
            n919 = xnode "Read/Write Control"("FPGA VI Reference In"=w1490, "error in"=w1489, "Green Filter Flipper"=FALSE) -> ("error out"=w1488:errorcluster)  [unwired: 1 out]
          }
        }
      }
      event "Pump 1 contents", "Pump 3 contents": Value Change {
        n920 = event-data() -> ()  [unwired: 7 out]
        n921 = local read "Pump 1 contents"() -> (→"Pump 1 cont disp":string)
        n922 = local read "Pump 3 contents"() -> (→"Pump 3 cont disp":string)
      }
      event "Reset Trap Pos. FB": Value Change {
        n923 = event-data() -> ()  [unwired: 7 out]
        n924 = xnode "Read/Write Control"("FPGA VI Reference In"=w1496, "error in"=w1495, "Trap Pos. FB Reset"="Reset Trap Pos. FB") -> ()  [unwired: 2 out]
      }
      event "Trap Pos. FB ON": Value Change {
        n925 = event-data() -> ()  [unwired: 7 out]
        n926 = xnode "Read/Write Control"("FPGA VI Reference In"=w1499, "error in"=w1498, "Force feedback"="Trap Pos. FB ON") -> ()  [unwired: 2 out]
      }
      event "Trap Pos. FB Range", "Trap Pos. FB Gains", "Trap Pos. FB Mult Factor", "Trap Pos. FB Offset Factor", "Trap Pos FB Negate Action", "Trap Pos FB Monitor\nT1 or T2": Value Change {
        n927 = event-data() -> ()  [unwired: 7 out]
        n928 = xnode "Read/Write Control"("FPGA VI Reference In"=w1508, "error in"=w1507, "Trap Pos. FB Range"="Trap Pos. FB Range", "Trap Pos. FB Gains"="Trap Pos. FB Gains", "Trap Pos. FB Mult Factor"="Trap Pos. FB Mult Factor", "Trap Pos. FB Offset Factor"="Trap Pos. FB Offset Factor", "Trap Pos FB Negate Action"="Trap Pos FB Negate Action", "Trap Pos FB Monitor T1 or T2"="Trap Pos FB Monitor\nT1 or T2", "AI1 X Scale"="Trap Pos. AI1 X Pre-scale") -> ()  [unwired: 2 out]
      }
      event "Trap Pos FB SP": Value Change {
        n929 = event-data() -> ()  [unwired: 7 out]
        n930 = xnode "Read/Write Control"("FPGA VI Reference In"=w1511, "error in"=w1510, "Trap Pos. FB SP"="Trap Pos FB SP") -> ()  [unwired: 2 out]
      }
      event "Set SP to Reading": Value Change {
        n931 = event-data() -> ()  [unwired: 7 out]
        n932 = local read "Trap Pos FB Monitor\nT1 or T2"() -> (w1519:bool)
        n933 = local read "Trap X AI1 (DMA)"() -> (w1522:T13)
        n934 = local read "Trap X (AI1)"() -> (w1525:T10)
        n935 = Unbundle By Name(w1525) -> ("Trap 1"=w1524:fxp<+/-,16,1>, "Trap 2"=w1523:fxp<+/-,16,1>)
        n936 = Unbundle By Name(w1522) -> ("Set 1"=w1521:fxp<+/-,16,1>, "Set 2"=w1520:fxp<+/-,16,1>)
        n937 = Select(t=w1524, s=w1519, f=w1523) -> (s? t:f=w1518:fxp<+/-,16,1>)
        n938 = Select(t=w1521, s=w1519, f=w1520) -> (s? t:f=w1517:fxp<+/-,16,1>)
        n939 = Not(x="Set SP Using...") -> (.not. x?=w1512:bool)
        n940 = Select(t=w1518, s=w1512, f=w1517) -> (s? t:f=w1513:fxp<+/-,16,1>)
        n941 = xnode "Read/Write Control"("FPGA VI Reference In"=w1515, "error in"=w1514, "Trap Pos. FB SP"=w1513) -> ()  [unwired: 2 out]
        n942 = local write "Trap Pos FB SP"(w1513) -> ()
      }
      event "Trap Pos. FB Out Scale 2^n": Value Change {
        n943 = event-data() -> ()  [unwired: 7 out]
        n944 = Scale By Power Of 2(n="Trap Pos. FB Out Scale 2^n", x=ext 1.0) -> (x*2^n=w1527:ext)
        n945 = property on="Trap Pos. FB Mult Factor" class="DigNum (strict)"("Val(Sgnl)"=w1527) -> ()  [unwired: 2 in, 2 out]
      }
      event "Trap Pos FB Int Count": Value Change {
        n946 = event-data() -> ()  [unwired: 7 out]
        n947 = xnode "Read/Write Control"("FPGA VI Reference In"=w1532, "error in"=w1531, "Trap Pos FB Int Count"="Trap Pos FB Int Count") -> ()  [unwired: 2 out]
      }
    }
    "error out 2" <- w715
    n948 = node-c288() -> ()  [unwired: 1 in, 1 out]
  }
  n949 = timed-loop "Run Scripts, including: stage motion" {
    timing: w69 -> [_]
    timing-out: [_] -> w68
    tunnel: w24 -> [_]
    stop <- w1534 stop-if-true
    n950 = node-c288() -> ()  [unwired: 1 in, 1 out]
    n951 = event shown="[8] \"Take Stepping Data\": Value Change" {
      selector: _ -> [_ _ _ _ _ _ _ _ _ _ _ _]
      dyn-events: _ -> [_ _ _ _ _ _ _ _ _ _ _ _]
      timeout: 50 -> [_ _ _ _ _ _ _ _ _ _ _ _]
      tunnel: ["Move Cap. 1 (DNA Top)" _ "Cal/Data Acq. Spot" "Dump Beads" "Dip for Protein" _ "Got ADig bead" "Got DNA bead" "Take Stepping Data" _ "Take Detection Laser\nImage" _] -> _
      tunnel: [_ _ _ _ _ _ _ _ _ _ _ w1742] -> w1534
      event "Move Cap. 1 (DNA Top)": Value Change {
        n952 = event-data() -> ()  [unwired: 1 in, 5 out]
        n953 = local write "Move Cap. 1 (DNA Top)"(FALSE ("Move Cap. 1 (DNA Right)")) -> ()
        n954 = flat-sequence {
          tunnel: "Cap 1 Samp Flow ON" -> [w1540]
          frame #0 {
            n955 = local write "Stage Moving"(FALSE ("Stage Moving")) -> ()
            n956 = case "stop flow" shown="True" w1540 {
              frame False {
              }
              frame True {
                n957 = call "hamilton_controller.vi"("Open?"=FALSE, "valve"=enum16{"A", "B", "C", "D", "ALL"}."C", "action"=T20."MOVE VALVE") -> ()  [unwired: 8 in, 1 out]
              }
            }
            n958 = case shown="True" TRUE {
              tunnel: "Cap 1 T ON" -> [w1549 w1550]
              frame False {
                n959 = property on="Trap 1 (ON/OFF)" class="Bool (strict)"("Val(Sgnl)"=w1549) -> ()  [unwired: 2 in, 2 out]
              }
              frame True {
                n960 = property on="Trap 2 (ON/OFF)" class="Bool (strict)"("Val(Sgnl)"=w1550) -> ()  [unwired: 2 in, 2 out]
              }
            }
            n961 = call <vilib>:"Beep.vi"() -> ()  [unwired: 3 in, 9 out]
            n962 = case shown="True" "Cap 1 Flow ON" {
              frame False {
              }
              frame True {
                n963 = property on="Inject Top" class="Bool (strict)"("Val(Sgnl)"=TRUE ("Value (Signaling)")) -> ()  [unwired: 2 in, 2 out]
              }
            }
          }
        }
      }
      event Timeout {
        n964 = event-data() -> ()  [unwired: 1 in, 2 out]
      }
      event "Cal/Data Acq. Spot": Value Change {
        # "wait for calibration file\nto be written"
        # "signal save cal true\nthis tells the data \nacquisition loop to\nstart sending the data\nto a calibration file"
        # "separate traps to\nthe desired trap delta"
        # "move stage to data acquisition spot"
        # "CHANGE FISH FOR TETHER BACK\nTO TRUE VALUE HERE."
        n965 = event-data() -> ()  [unwired: 1 in, 5 out]
        n966 = local write "Cal/Data Acq. Spot"(FALSE ("Cal/Data Acq. Spot")) -> ()
        n967 = flat-sequence {
          tunnel: ["Cal @ (MHz)"] -> w1551
          tunnel: w1551 -> [w1561]
          tunnel: w1551 -> [w1582]
          frame #0 {
            n968 = property on="Trap Delta (MHz)" class="DigNum (strict)"("Val(Sgnl)"="Cal @ (MHz)") -> ()  [unwired: 2 in, 2 out]
            n969 = call <vilib>:"Beep.vi"() -> ()  [unwired: 3 in, 9 out]
          }
          frame #1 {
            n970 = Wait (ms)(milliseconds to wait=u32 100) -> ()  [unwired: 1 out]
          }
          frame #2 {
            n971 = property on="Save Calibration" class="Bool (strict)"("Val(Sgnl)"=TRUE ("Value (Signaling)")) -> ()  [unwired: 2 in, 2 out]
          }
          frame #3 {
            n972 = Wait (ms)(milliseconds to wait=u32 4000) -> ()  [unwired: 1 out]
          }
          frame #4 {
            n973 = while {
              stop <- w1558 stop-if-true
              n974 = local read "Saving..."() -> (w1559:bool)
              n975 = Wait (ms)(milliseconds to wait=u32 100) -> ()  [unwired: 1 out]
              n976 = Not(x=w1559) -> (.not. x?=w1558:bool)
            }
          }
          frame #5 {
            n977 = case shown="True" "W/ Offset 1" {
              tunnel: w1561 -> [_ w1563]
              frame False {
              }
              frame True {
                n978 = stacked-sequence {
                  tunnel: w1563 -> [_ _ _ _ _ _ _ w1580]
                  frame #0 {
                    n979 = Replace Array Subset(array=u32[] [0] ("Index Values"), new element="Offset 1 Set", index=0) -> (w1564:u32[])
                    n980 = property on="Saved AOD Raster Scan Parameter Sets" class="Arr (strict)"("Index Values"=w1564) -> ()  [unwired: 2 in, 2 out]
                    n981 = property on="Trap Delta (MHz)" class="DigNum (strict)"("Val(Sgnl)"="Offset 1 Start (MHz)") -> ()  [unwired: 2 in, 2 out]
                  }
                  frame #1 {
                    n982 = Wait (ms)(milliseconds to wait=u32 200) -> ()  [unwired: 1 out]
                  }
                  frame #2 {
                    n983 = property on="Load parameters" class="Bool (strict)"("Val(Sgnl)"=TRUE ("Value (Signaling)")) -> ()  [unwired: 2 in, 2 out]
                  }
                  frame #3 {
                    n984 = Wait (ms)(milliseconds to wait=u32 200) -> ()  [unwired: 1 out]
                  }
                  frame #4 {
                    n985 = property on="Trap Raster Scan" class="Bool (strict)"("Val(Sgnl)"=TRUE ("Value (Signaling)")) -> ()  [unwired: 2 in, 2 out]
                  }
                  frame #5 {
                    n986 = Wait (ms)(milliseconds to wait=u32 2000) -> ()  [unwired: 1 out]
                  }
                  frame #6 {
                    n987 = while {
                      stop <- w1577 stop-if-true
                      n988 = local read "Raster Scanning..."() -> (w1579:bool)
                      n989 = local read "Saving..."() -> (w1575:bool)
                      n990 = Wait (ms)(milliseconds to wait=u32 100) -> ()  [unwired: 1 out]
                      n991 = Not(x=w1575) -> (.not. x?=w1574:bool)
                      n992 = Not(x=w1579) -> (.not. x?=w1576:bool)
                      n993 = And(x=w1576, y=w1574) -> (x .and. y?=w1577:bool)
                    }
                  }
                  frame #7 {
                    n994 = property on="Trap Delta (MHz)" class="DigNum (strict)"("Val(Sgnl)"=w1580) -> ()  [unwired: 2 in, 2 out]
                  }
                }
              }
            }
          }
          frame #6 {
            n995 = local read "Save ave N"() -> (w1581:dbl)
            n996 = case shown="True" "W/ Offset 2" {
              tunnel: w1582 -> [_ w1588]
              tunnel: w1581 -> [_ w1587]
              frame False {
                n997 = Multiply(x="Cal read wait (s)", y=u32 1000 ("milliseconds to wait")) -> (x*y=w1585:u32)
                n998 = Wait (ms)(milliseconds to wait=w1585) -> ()  [unwired: 1 out]
              }
              frame True {
                n999 = stacked-sequence {
                  tunnel: w1588 -> [_ _ _ _ _ _ _ _ _ w1609 _ _]
                  tunnel: w1587 -> [_ _ _ _ _ _ _ _ _ w1607 _ _]
                  frame #0 {
                    n1000 = property on="Save ave N" class="DigNum (strict)"("Val(Sgnl)"=1.0 ("Value (Signaling)")) -> ()  [unwired: 2 in, 2 out]
                  }
                  frame #1 {
                    n1001 = Wait (ms)(milliseconds to wait=u32 500) -> ()  [unwired: 1 out]
                  }
                  frame #2 {
                    n1002 = property on="Trap Delta (MHz)" class="DigNum (strict)"("Val(Sgnl)"="Offset 2 Start (MHz)") -> ()  [unwired: 2 in, 2 out]
                    n1003 = Replace Array Subset(array=u32[] [0] ("Index Values"), new element="Offset 2 Set", index=0) -> (w1593:u32[])
                    n1004 = property on="Saved AOD Raster Scan Parameter Sets" class="Arr (strict)"("Index Values"=w1593) -> ()  [unwired: 2 in, 2 out]
                  }
                  frame #3 {
                    n1005 = Wait (ms)(milliseconds to wait=u32 500) -> ()  [unwired: 1 out]
                  }
                  frame #4 {
                    n1006 = property on="Load parameters" class="Bool (strict)"("Val(Sgnl)"=TRUE ("Value (Signaling)")) -> ()  [unwired: 2 in, 2 out]
                  }
                  frame #5 {
                    n1007 = Wait (ms)(milliseconds to wait=u32 500) -> ()  [unwired: 1 out]
                  }
                  frame #6 {
                    n1008 = property on="Trap Raster Scan" class="Bool (strict)"("Val(Sgnl)"=TRUE ("Value (Signaling)")) -> ()  [unwired: 2 in, 2 out]
                  }
                  frame #7 {
                    n1009 = Wait (ms)(milliseconds to wait=u32 2000) -> ()  [unwired: 1 out]
                  }
                  frame #8 {
                    n1010 = while {
                      stop <- w1602 stop-if-true
                      n1011 = local read "Raster Scanning..."() -> (w1605:bool)
                      n1012 = local read "Saving..."() -> (w1603:bool)
                      n1013 = Wait (ms)(milliseconds to wait=u32 100) -> ()  [unwired: 1 out]
                      n1014 = Not(x=w1603) -> (.not. x?=w1601:bool)
                      n1015 = Not(x=w1605) -> (.not. x?=w1604:bool)
                      n1016 = And(x=w1604, y=w1601) -> (x .and. y?=w1602:bool)
                    }
                  }
                  frame #9 {
                    n1017 = property on="Trap Delta (MHz)" class="DigNum (strict)"("Val(Sgnl)"=w1609) -> ()  [unwired: 2 in, 2 out]
                    n1018 = property on="Saved AOD Raster Scan Parameter Sets" class="Arr (strict)"("Index Values"=u32[] [0]) -> ()  [unwired: 2 in, 2 out]
                    n1019 = property on="Save ave N" class="DigNum (strict)"("Val(Sgnl)"=w1607) -> ()  [unwired: 2 in, 2 out]
                  }
                  frame #10 {
                    n1020 = Wait (ms)(milliseconds to wait=u32 500) -> ()  [unwired: 1 out]
                  }
                  frame #11 {
                    n1021 = property on="Load parameters" class="Bool (strict)"("Val(Sgnl)"=TRUE ("Value (Signaling)")) -> ()  [unwired: 2 in, 2 out]
                  }
                }
              }
            }
          }
          frame #7 {
            n1022 = property on="Read Cal" class="Bool (strict)"("Val(Sgnl)"=TRUE ("Value (Signaling)")) -> ()  [unwired: 2 in, 2 out]
          }
          frame #8 {
            n1023 = Wait (ms)(milliseconds to wait=u32 500) -> ()  [unwired: 1 out]
          }
          frame #9 {
            n1024 = property on="Fish for Tether" class="Bool (strict)"("Val(Sgnl)"=FALSE ("Value (Signaling)")) -> ()  [unwired: 2 in, 2 out]
          }
        }
      }
      event "Dump Beads": Value Change {
        # "SCRIPT TO REMOVE BOTH BEADS FROM THE TRAPS. TURNS ON LIGHT WHICH INDICATES THAT STAGE IS MOVING. THEN STOPS SAVING DATA. \nSETS Sample Channel Flow TO TRUE. STOPS INTERLACING GREEN FLUORESCENCE. TURNS OFF Tether INDICATOR BECAUSE WE ARE THROWING IT\nAWAY. SHUTS OFF TRAP POSITION FEEDBACK."
        n1025 = event-data() -> ()  [unwired: 1 in, 5 out]
        n1026 = flat-sequence {
          frame #0 {
            w1616 = FALSE ("Fl. Triggered...")
            w1617 = TRUE ("Stage Moving")
            n1027 = local read "Saving..."() -> (w1618:bool)
            n1028 = local write "Fl. Triggered..."(w1616) -> ()
            n1029 = local write "Stage Moving"(w1617) -> ()
            n1030 = local write "Tether"(w1616) -> ()
            n1031 = property on="Green Laser ON/Interlacing" class="Bool (strict)"("Val(Sgnl)"=w1616) -> ()  [unwired: 2 in, 2 out]
            n1032 = property on="Trap Pos. FB ON" class="Bool (strict)"("Val(Sgnl)"=w1616) -> ()  [unwired: 2 in, 2 out]
            n1033 = property on="Sample Channel Flow" class="Bool (strict)"("Val(Sgnl)"=w1617) -> ()  [unwired: 2 in, 2 out]
            n1034 = local write "Stop Saving"(w1618) -> ()
          }
          frame #1 {
            w1619 = FALSE ("Value (Signaling)")
            # "TURNS TRAPS OFF SO THAT\nBEADS REMAIN AT DUMP \nBEADS POSITION"
            n1035 = property on="Trap 1 (ON/OFF)" class="Bool (strict)"("Val(Sgnl)"=w1619) -> ()  [unwired: 2 in, 2 out]
            n1036 = property on="Trap 2 (ON/OFF)" class="Bool (strict)"("Val(Sgnl)"=w1619) -> ()  [unwired: 2 in, 2 out]
            n1037 = call <vilib>:"Beep.vi"() -> ()  [unwired: 3 in, 9 out]
          }
          frame #2 {
            n1038 = property on="Goto Bottom (F7)" class="Bool (strict)"("Val(Sgnl)"=TRUE ("Value (Signaling)")) -> ()  [unwired: 2 in, 2 out]
          }
          frame #3 {
            n1039 = Wait (ms)(milliseconds to wait=u32 8000) -> ()  [unwired: 1 out]
          }
          frame #4 {
            n1040 = property on="Trap Delta (MHz)" class="DigNum (strict)"("Val(Sgnl)"=20.0 ("Value (Signaling)")) -> ()  [unwired: 2 in, 2 out]
          }
          frame #5 {
            n1041 = property on="Trap 2 (ON/OFF)" class="Bool (strict)"("Val(Sgnl)"=TRUE ("Value (Signaling)")) -> ()  [unwired: 2 in, 2 out]
          }
          frame #6 {
            n1042 = property on="Sample Channel Flow" class="Bool (strict)"("Val(Sgnl)"=FALSE ("Value (Signaling)")) -> ()  [unwired: 2 in, 2 out]
          }
        }
      }
      event "Dip for Protein": Value Change {
        n1043 = event-data() -> ()  [unwired: 1 in, 5 out]
        n1044 = flat-sequence {
          frame #0 {
            n1045 = case shown="True" "Move Trap Before?" {
              frame False {
              }
              frame True {
                n1046 = property on="Trap Delta (MHz)" class="DigNum (strict)"("Val(Sgnl)"="Dip Trap Delta 1 (MHz)") -> ()  [unwired: 2 in, 2 out]
              }
            }
          }
          frame #1 {
            n1047 = Multiply(x="Duration (s)", y=1000.0) -> (x*y=w1628:dbl)
            n1048 = Wait (ms)(milliseconds to wait=w1628) -> ()  [unwired: 1 out]
          }
          frame #2 {
            n1049 = case shown="True" "Move Trap After?" {
              frame False {
              }
              frame True {
                n1050 = property on="Trap Delta (MHz)" class="DigNum (strict)"("Val(Sgnl)"="Dip Trap Delta 2 (MHz)") -> ()  [unwired: 2 in, 2 out]
              }
            }
          }
          frame #3 {
            n1051 = case shown="True" "Green ON After?" {
              frame False {
              }
              frame True {
                n1052 = property on="Green Laser ON/Interlacing" class="Bool (strict)"("Val(Sgnl)"=TRUE ("Value (Signaling)")) -> ()  [unwired: 2 in, 2 out]
              }
            }
          }
          frame #4 {
            n1053 = Wait (ms)(milliseconds to wait=u32 500) -> ()  [unwired: 1 out]
          }
          frame #5 {
            n1054 = case shown="True" "Save Data After?" {
              frame False {
              }
              frame True {
                n1055 = property on="Start Saving" class="Bool (strict)"("Val(Sgnl)"=TRUE ("Value (Signaling)")) -> ()  [unwired: 2 in, 2 out]
              }
            }
          }
        }
      }
      event "Profile": Value Change {
        n1056 = event-data() -> ()  [unwired: 1 in, 5 out]
        n1057 = flat-sequence {
          frame #0 {
            w1638 = 0.0 ("element")
            n1058 = Build Array(w1638, "Y change (mm)", w1638) -> ()  [unwired: 1 out]
          }
          frame #1 {
            # "stop saving"
            n1059 = local write "Stop Saving"(TRUE ("Stop Saving")) -> ()
            n1060 = local write "Stage Moving"(FALSE ("Stage Moving")) -> ()
          }
        }
      }
      event "Got ADig bead": Value Change {
        n1061 = event-data() -> ()  [unwired: 1 in, 5 out]
        n1062 = property on="Move Cap. 1 (DNA Top)" class="Bool (strict)"("Val(Sgnl)"=TRUE ("Value (Signaling)")) -> ()  [unwired: 2 in, 2 out]
        n1063 = property on="Inject Bottom" class="Bool (strict)"("Val(Sgnl)"=FALSE ("Value (Signaling)")) -> ()  [unwired: 2 in, 2 out]
      }
      event "Got DNA bead": Value Change {
        n1064 = event-data() -> ()  [unwired: 1 in, 5 out]
        n1065 = property on="Cal/Data Acq. Spot" class="Bool (strict)"("Val(Sgnl)"=TRUE ("Value (Signaling)")) -> ()  [unwired: 2 in, 2 out]
        n1066 = property on="Inject Top" class="Bool (strict)"("Val(Sgnl)"=FALSE ("Value (Signaling)")) -> ()  [unwired: 2 in, 2 out]
      }
      event "Take Stepping Data": Value Change {
        n1067 = event-data() -> ()  [unwired: 1 in, 5 out]
        n1068 = local read "Save ave N"() -> (w1656:dbl)
        n1069 = flat-sequence {
          tunnel: w1656 -> [w1658]
          tunnel: [w1658] -> w1651
          tunnel: [w1660] -> w1652
          tunnel: w1651 -> [w1660]
          tunnel: [w1662] -> w1653
          tunnel: w1652 -> [w1662]
          tunnel: [w1665] -> w1654
          tunnel: w1653 -> [w1665]
          tunnel: [w1667] -> w1655
          tunnel: w1654 -> [w1667]
          tunnel: [w1669] -> w1649
          tunnel: w1655 -> [w1669]
          tunnel: w1649 -> [w1672]
          tunnel: [w1672] -> w1648
          tunnel: w1648 -> [w1673]
          tunnel: [w1673] -> w1650
          tunnel: w1650 -> [w1679]
          frame #0 {
            n1070 = property on="Save ave N" class="DigNum (strict)"("Val(Sgnl)"="Save ave factor") -> ()  [unwired: 2 in, 2 out]
          }
          frame #1 {
            n1071 = Wait (ms)(milliseconds to wait=u32 100) -> ()  [unwired: 1 out]
          }
          frame #2 {
            n1072 = local read "Offset 2 Start (MHz)"() -> (w1664:dbl)
            n1073 = property on="Saved AOD Raster Scan Parameter Sets" class="Arr (strict)"("Index Values"=u32[] [2]) -> ()  [unwired: 2 in, 2 out]
            n1074 = property on="Trap Delta (MHz)" class="DigNum (strict)"("Val(Sgnl)"=w1664) -> ()  [unwired: 2 in, 2 out]
          }
          frame #3 {
            n1075 = property on="Load parameters" class="Bool (strict)"("Val(Sgnl)"=TRUE ("Value (Signaling)")) -> ()  [unwired: 2 in, 2 out]
          }
          frame #4 {
            n1076 = Wait (ms)(milliseconds to wait=u32 100) -> ()  [unwired: 1 out]
          }
          frame #5 {
            n1077 = property on="Trap Raster Scan" class="Bool (strict)"("Val(Sgnl)"=TRUE ("Value (Signaling)")) -> ()  [unwired: 2 in, 2 out]
          }
          frame #6 {
            n1078 = Wait (ms)(milliseconds to wait=u32 1000) -> ()  [unwired: 1 out]
          }
          frame #7 {
            n1079 = while {
              stop <- w1676 stop-if-true
              n1080 = local read "Raster Scanning..."() -> (w1678:bool)
              n1081 = local read "Saving..."() -> (w1677:bool)
              n1082 = Not(x=w1677) -> (.not. x?=w1674:bool)
              n1083 = Not(x=w1678) -> (.not. x?=w1675:bool)
              n1084 = And(x=w1675, y=w1674) -> (x .and. y?=w1676:bool)
            }
          }
          frame #8 {
            n1085 = property on="Save ave N" class="DigNum (strict)"("Val(Sgnl)"=w1679) -> ()  [unwired: 2 in, 2 out]
          }
        }
      }
      event "Step Size (nm)": Value Change {
        n1086 = event-data() -> ()  [unwired: 1 in, 5 out]
        n1087 = flat-sequence {
          frame #0 {
            n1088 = property on="Saved AOD Raster Scan Parameter Sets" class="Arr (strict)"("Index Values"=u32[] [1]) -> ()  [unwired: 2 in, 2 out]
          }
          frame #1 {
            n1089 = Multiply(x="N Steps", y="Step Size (nm)") -> (x*y=w1681:dbl)
            n1090 = property on="Scan Speed AOD (nm/s) 2" class="DigNum (strict)"("Value"="Step Size (nm)") -> ()  [unwired: 2 in, 2 out]
            n1091 = property on="Step Size AOD (nm) 2" class="DigNum (strict)"("Value"="Step Size (nm)") -> ()  [unwired: 2 in, 2 out]
            n1092 = property on="Scan Range AOD (nm) 2" class="DigNum (strict)"("Value"=w1681) -> ()  [unwired: 2 in, 2 out]
          }
        }
      }
      event "Take Detection Laser\nImage": Value Change {
        n1093 = event-data() -> ()  [unwired: 1 in, 5 out]
        n1094 = flat-sequence {
          tunnel: [w1709] -> w1699
          tunnel: [w1708] -> w1692
          tunnel: [w1707] -> w1684
          tunnel: [w1712] -> w1700
          tunnel: w1699 -> [w1712]
          tunnel: [w1711] -> w1693
          tunnel: w1692 -> [w1711]
          tunnel: [w1710] -> w1685
          tunnel: w1684 -> [w1710]
          tunnel: [w1716] -> w1701
          tunnel: w1700 -> [w1716]
          tunnel: [w1715] -> w1694
          tunnel: w1693 -> [w1715]
          tunnel: [w1714] -> w1686
          tunnel: w1685 -> [w1714]
          tunnel: [w1722] -> w1702
          tunnel: w1701 -> [w1722]
          tunnel: [w1721] -> w1695
          tunnel: w1694 -> [w1721]
          tunnel: [w1720] -> w1687
          tunnel: w1686 -> [w1720]
          tunnel: [w1726] -> w1703
          tunnel: w1702 -> [w1726]
          tunnel: [w1725] -> w1696
          tunnel: w1695 -> [w1725]
          tunnel: [w1724] -> w1688
          tunnel: w1687 -> [w1724]
          tunnel: [w1730] -> w1704
          tunnel: w1703 -> [w1730]
          tunnel: [w1729] -> w1697
          tunnel: w1696 -> [w1729]
          tunnel: [w1728] -> w1689
          tunnel: w1688 -> [w1728]
          tunnel: [w1734] -> w1705
          tunnel: w1704 -> [w1734]
          tunnel: [w1733] -> w1698
          tunnel: w1697 -> [w1733]
          tunnel: [w1732] -> w1690
          tunnel: w1689 -> [w1732]
          tunnel: w1705 -> [w1740]
          tunnel: w1698 -> [w1739]
          tunnel: [w1737] -> w1691
          tunnel: w1690 -> [w1737]
          tunnel: w1691 -> [w1741]
          frame #0 {
            n1095 = local read "Green Laser ON/Interlacing"() -> (w1709:bool)
            n1096 = local read "Green laser mode"() -> (w1708:enum32{"Laser ON", "Laser OFF", "Interlace"})
            n1097 = local read "Green FB On/Off"() -> (w1707:bool)
          }
          frame #1 {
            n1098 = property on="Green FB On/Off" class="Bool (strict)"("Val(Sgnl)"=FALSE ("Value (Signaling)")) -> ()  [unwired: 2 in, 2 out]
          }
          frame #2 {
            n1099 = property on="Green Laser ON/Interlacing" class="Bool (strict)"("Val(Sgnl)"=TRUE ("Value (Signaling)")) -> ()  [unwired: 2 in, 2 out]
            n1100 = property on="Flip Green Filter" class="Bool (strict)"("Val(Sgnl)"=TRUE ("Value (Signaling)")) -> ()  [unwired: 2 in, 2 out]
            n1101 = property on="Green laser mode" class="RadioBtnsControl (strict)"("Val(Sgnl)"=enum32{"Laser ON", "Laser OFF", "Interlace"}."Laser ON" ("Value (Signaling)")) -> ()  [unwired: 2 in, 2 out]
          }
          frame #3 {
            n1102 = Wait (ms)(milliseconds to wait=u32 500) -> ()  [unwired: 1 out]
          }
          frame #4 {
            n1103 = property on="Confocal Image" class="Bool (strict)"("Val(Sgnl)"=TRUE ("Value (Signaling)")) -> ()  [unwired: 2 in, 2 out]
          }
          frame #5 {
            n1104 = Wait (ms)(milliseconds to wait=u32 2000) -> ()  [unwired: 1 out]
          }
          frame #6 {
            n1105 = while {
              stop <- w1735 stop-if-true
              n1106 = local read "Saving..."() -> (w1736:bool)
              n1107 = Not(x=w1736) -> (.not. x?=w1735:bool)
            }
          }
          frame #7 {
            n1108 = property on="Flip Green Filter" class="Bool (strict)"("Val(Sgnl)"=TRUE ("Value (Signaling)")) -> ()  [unwired: 2 in, 2 out]
            n1109 = property on="Green Laser ON/Interlacing" class="Bool (strict)"("Val(Sgnl)"=w1740) -> ()  [unwired: 2 in, 2 out]
            n1110 = property on="Green laser mode" class="RadioBtnsControl (strict)"("Val(Sgnl)"=w1739) -> ()  [unwired: 2 in, 2 out]
          }
          frame #8 {
            n1111 = property on="Green FB On/Off" class="Bool (strict)"("Val(Sgnl)"=w1741) -> ()  [unwired: 2 in, 2 out]
          }
        }
      }
      event "Stop All": Value Change {
        n1112 = event-data() -> ()  [unwired: 1 in, 5 out]
        n1113 = local read "Stop All"() -> (w1742:bool)
      }
    }
    n1114 = node-c288() -> ()  [unwired: 1 in, 1 out]
  }
  n1115 = node-c288() -> (w76:T24)  [unwired: 4 out]
  n1116 = timed-loop "Mouse control: trap position (AOM deflection), set confocal spot from image" {
    tunnel: [w1744] -> w34
    tunnel: w24 -> [w1743]
    timing: w76 -> [_]
    timing-out: [_] -> w75
    stop <- w1744 stop-if-true
    n1117 = node-c288() -> ()  [unwired: 2 out]
    n1118 = event shown="[0] \"Pane\": Mouse Down" {
      selector: _ -> [_ _]
      dyn-events: _ -> [_ _]
      timeout: _ -> [_ _]
      tunnel: w1743 -> [w1747 _]
      event Mouse Down {
        n1119 = event-data() -> ("Time"=w1749:u32, "Coords"=w1748:T7, "Button"=w1750:u16)  [unwired: 6 out]
        n1120 = case shown="1" w1750 {
          tunnel: w1749 -> [_ _ w1853]
          tunnel: w1748 -> [_ w1787 w1851]
          tunnel: w1747 -> [_ _ w1849]
          frame 0, Default {
          }
          frame 1 {
            n1121 = property on="APD 2" class="ImageControl"() -> ("Displayed Image Position"=w1757:cluster{"Left":i32, "Top":i32})  [unwired: 2 in, 2 out]
            n1122 = property on="APD 1" class="ImageControl"() -> ("Displayed Image Position"=w1786:cluster{"Left":i32, "Top":i32})  [unwired: 2 in, 2 out]
            n1123 = property on="Detection Laser X" class="ImageControl"() -> ("Displayed Image Position"=w1783:cluster{"Left":i32, "Top":i32})  [unwired: 2 in, 2 out]
            n1124 = property on="Detection Laser Y" class="ImageControl"() -> ("Displayed Image Position"=w1782:cluster{"Left":i32, "Top":i32})  [unwired: 2 in, 2 out]
            n1125 = property on="APD 2" class="ImageControl"() -> ("Displayed Image Size"=w1756:cluster{"Width":u32, "Height":u32})  [unwired: 2 in, 2 out]
            n1126 = property on="APD 1" class="ImageControl"() -> ("Displayed Image Size"=w1784:cluster{"Width":u32, "Height":u32})  [unwired: 2 in, 2 out]
            n1127 = property on="Detection Laser X" class="ImageControl"() -> ("Displayed Image Size"=w1785:cluster{"Width":u32, "Height":u32})  [unwired: 2 in, 2 out]
            n1128 = property on="Detection Laser Y" class="ImageControl"() -> ("Displayed Image Size"=w1781:cluster{"Width":u32, "Height":u32})  [unwired: 2 in, 2 out]
            n1129 = Unbundle By Name(w1756) -> ("Width"=w1753:u32, "Height"=w1752:u32)
            n1130 = Unbundle By Name(w1757) -> ("Left"=w1755:i32, "Top"=w1754:i32)
            n1131 = Unbundle By Name(w1784) -> ("Width"=w1778:u32, "Height"=w1777:u32)
            n1132 = Unbundle By Name(w1785) -> ("Width"=w1774:u32, "Height"=w1773:u32)
            n1133 = Unbundle By Name(w1781) -> ("Width"=w1770:u32, "Height"=w1769:u32)
            n1134 = Unbundle By Name(w1786) -> ("Left"=w1780:i32, "Top"=w1779:i32)
            n1135 = Unbundle By Name(w1783) -> ("Left"=w1776:i32, "Top"=w1775:i32)
            n1136 = Unbundle By Name(w1782) -> ("Left"=w1772:i32, "Top"=w1771:i32)
            n1137 = Bundle("Left"=w1755, "Top"=w1754, "Width"=w1753, "Height"=w1752) -> (w1751:T33)  [unwired: 1 in]
            n1138 = Bundle("Left"=w1780, "Top"=w1779, "Width"=w1778, "Height"=w1777) -> (w1768:T33)  [unwired: 1 in]
            n1139 = Bundle("Left"=w1776, "Top"=w1775, "Width"=w1774, "Height"=w1773) -> (w1767:T33)  [unwired: 1 in]
            n1140 = Bundle("Left"=w1772, "Top"=w1771, "Width"=w1770, "Height"=w1769) -> (w1766:T33)  [unwired: 1 in]
            n1141 = Build Cluster Array(w1751, w1768, w1767, w1766) -> (w1765:T34)
            n1142 = for {
              tunnel: w1787 -> [w1798]
              tunnel: w1765 -> [w1799] mode=indexing
              shift-right: [w1796] -> w1763
              shift-left: TRUE -> [w1797]
              shift-right: [w1795] -> w1761
              shift-left: _ -> [w1791]
              shift-right: [w1794] -> w1760
              shift-left: _ -> [w1790]
              shift-right: [w1793] -> w1759
              shift-left: _ -> [w1789]
              shift-right: [w1792] -> w1758
              shift-left: _ -> [w1788]
              n1143 = case shown="True" w1797 {
                selector: w1797 -> [w1804 _]
                tunnel: w1799 -> [_ w1813]
                tunnel: w1798 -> [_ w1811]
                tunnel: [w1804 w1809] -> w1796
                tunnel: [w1803 w1808] -> w1795
                tunnel: [w1802 w1807] -> w1794
                tunnel: [w1801 w1806] -> w1793
                tunnel: [w1800 w1805] -> w1792
                tunnel: w1791 -> [w1803 _]
                tunnel: w1790 -> [w1802 _]
                tunnel: w1789 -> [w1801 _]
                tunnel: w1788 -> [w1800 _]
                frame False {
                }
                frame True {
                  n1144 = Unbundle(w1813) -> (w1812:T33)
                  n1145 = call "isclickinwindow.vi"("Image Param"=w1812, "Point32"=w1811) -> ("4 Y"=w1805:i32, "3 Height"=w1806:i32, "2 X"=w1807:i32, "1 Width"=w1808:i32, "In image?"=w1810:bool)  [unwired: 1 in]
                  n1146 = Not(x=w1810) -> (.not. x?=w1809:bool)
                }
              }
            }
            n1147 = Not(x=w1763) -> (.not. x?=w1762:bool)
            n1148 = case shown="True" w1762 {
              tunnel: w1760 -> [_ w1826]
              tunnel: w1758 -> [_ w1825]
              tunnel: w1761 -> [_ w1824]
              tunnel: w1759 -> [_ w1823]
              frame False {
              }
              frame True {
                w1819 = FALSE ("Get Point")
                n1149 = local read "Scan lines (y)"() -> (w1828:u64)
                n1150 = local read "Actual MCL Inc (V)"() -> (w1820:dbl)
                n1151 = local read "Scan steps (MCL)"() -> (w1827:u64)
                n1152 = Divide "Y Pix/step"(x=w1823, y=w1828) -> (x/y=w1835:dbl)
                n1153 = Divide "Y V/pix"(x=w1820, y=w1835) -> (x/y=w1834:dbl)
                n1154 = Divide "Y half step offset"(x=w1820, y=2.0) -> (x/y=w1836:dbl)
                n1155 = Divide "X pix/step"(x=w1824, y=w1827) -> (x/y=w1833:dbl)
                n1156 = Negate(x=w1836) -> (-x=w1837:dbl)
                n1157 = local read "Initial Y"() -> (w1843:dbl)
                n1158 = Multiply(x=w1825, y=w1834) -> (x*y=w1844:dbl)
                n1159 = Divide "X half step offset"(x=w1820, y=2.0) -> (x/y=w1830:dbl)
                n1160 = Divide "X V/pix"(x=w1820, y=w1833) -> (x/y=w1832:dbl)
                n1161 = Multiply(x=w1820, y=w1827) -> (x*y=w1839:dbl)
                n1162 = Compound Arithmetic op=ADD(w1837, w1844, w1843) -> (w1821:dbl)
                "Pointer Y (V)" <- w1821
                n1163 = Multiply(x=w1832, y=w1826) -> (x*y=w1841:dbl)
                n1164 = Negate(x=w1830) -> (-x=w1829:dbl)
                n1165 = local read "Initial X"() -> (w1842:dbl)
                n1166 = Negate(x=w1841) -> (-x=w1840:dbl)
                n1167 = Compound Arithmetic op=ADD(w1829, w1839, w1842, w1840) -> (w1822:dbl)
                "Pointer X (V)" <- w1822
                n1168 = Or(x="Set X Only", y="Set Confocal Spot (X-Y)") -> (x .or. y?=w1815:bool)
                n1169 = Or(x="Set Confocal Spot (X-Y)", y="Set Y Only") -> (x .or. y?=w1814:bool)
                n1170 = case shown="True" w1815 {
                  tunnel: w1822 -> [_ w1845]
                  frame False {
                  }
                  frame True {
                    n1171 = property on="AO2" class="Slide (strict)"("Val(Sgnl)"=w1845) -> ()  [unwired: 2 in, 2 out]
                  }
                }
                n1172 = case shown="True" w1814 {
                  tunnel: w1821 -> [_ w1846]
                  frame False {
                  }
                  frame True {
                    n1173 = property on="AO1" class="Slide (strict)"("Val(Sgnl)"=w1846) -> ()  [unwired: 2 in, 2 out]
                  }
                }
                n1174 = local write "Set Confocal Spot (X-Y)"(w1819) -> ()
                n1175 = local write "Set X Only"(w1819) -> ()
                n1176 = local write "Set Y Only"(w1819) -> ()
              }
            }
          }
          frame 3 {
            n1177 = local read "BD 2 Frequency 1 (MHz)"() -> (w1847:dbl)
            n1178 = local read "BD 1 Frequency 1 (MHz)"() -> (w1848:dbl)
            n1179 = local write "Manipulating Trap"(TRUE ("Manipulating Trap")) -> ()
            n1180 = local write "Coords"(T7 {"Horizontal"=0, "Vertical"=0} ("Coords")) -> ()
            n1181 = while {
              tunnel: w1853 -> [w1858]
              tunnel: w1851 -> [w1857]
              tunnel: w1849 -> [w1856]
              tunnel: w1848 -> [w1855]
              tunnel: w1847 -> [w1854]
              stop <- w1859 stop-if-true
              n1182 = event shown="[0] \"Pane\": Mouse Move" {
                selector: _ -> [_ _]
                dyn-events: _ -> [_ _]
                timeout: _ -> [_ _]
                tunnel: ["Force Manip Abort" w1923] -> w1859
                tunnel: w1858 -> [w1866 _]
                tunnel: w1857 -> [w1864 _]
                tunnel: w1856 -> [w1863 _]
                tunnel: w1855 -> [w1862 _]
                tunnel: w1854 -> [w1861 _]
                event Mouse Move {
                  n1183 = event-data() -> ("Time"=w1867:u32, "Coords"=w1868:T7)  [unwired: 3 out]
                  n1184 = Less?(x=w1867, y=w1866) -> (x < y?=w1865:bool)
                  n1185 = case "Makes sure old motion events prior to mouse click aren't used" shown="False" w1865 {
                    tunnel: w1868 -> [w1910 _]
                    tunnel: w1864 -> [w1911 _]
                    tunnel: w1863 -> [w1888 _]
                    tunnel: w1862 -> [w1884 _]
                    tunnel: w1861 -> [w1883 _]
                    frame False {
                      n1186 = Subtract(x=w1910, y=w1911) -> (x-y=w1909:T7)
                      "Coords" <- w1909
                      n1187 = local read "Y RF Frequency Limits (MHz)"() -> (w1869:T16)
                      n1188 = To Double Precision Float(number=w1909) -> (double precision float=w1908:cluster{"Horizontal":dbl, "Vertical":dbl})
                      n1189 = Multiply(x=cluster{"Horizontal":dbl, "Vertical":dbl} {"Horizontal"=-1.0, "Vertical"=1.0}, y="Manipulation Scaling") -> (x*y=w1904:cluster{"Horizontal":dbl, "Vertical":dbl})
                      n1190 = local read "X RF Frequency Limits (MHz)"() -> (w1870:T16)
                      n1191 = Multiply(x=w1908, y=w1904) -> (x*y=w1906:cluster{"Horizontal":dbl, "Vertical":dbl})
                      n1192 = Unbundle By Name(w1906) -> ("Horizontal"=w1901:dbl, "Vertical"=w1905:dbl)
                      n1193 = Unbundle By Name(w1869) -> ("Maximum"=w1872:dbl, "Minimum"=w1871:dbl)
                      n1194 = Boolean To (0,1)(Boolean="Manip. X?") -> (0, 1=w1899:i16)
                      n1195 = Boolean To (0,1)(Boolean="Manip. Y?") -> (0, 1=w1896:i16)
                      n1196 = local read "BD 1 Frequency 2 (MHz)"() -> (w1886:dbl)
                      n1197 = Multiply(x=w1905, y=w1896) -> (x*y=w1898:dbl)
                      n1198 = Multiply(x=w1899, y=w1901) -> (x*y=w1902:dbl)
                      n1199 = local read "BD 2 Frequency 2 (MHz)"() -> (w1885:dbl)
                      n1200 = Unbundle By Name(w1870) -> ("Maximum"=w1874:dbl, "Minimum"=w1873:dbl)
                      n1201 = Add(x=w1883, y=w1898) -> (x+y=w1876:dbl)
                      n1202 = Add(x=w1884, y=w1902) -> (x+y=w1878:dbl)
                      n1203 = In Range and Coerce(upper limit=w1874, x=w1878, lower limit=w1873) -> (coerced(x)=w1877:dbl)  [unwired: 1 out]
                      n1204 = In Range and Coerce(upper limit=w1872, x=w1876, lower limit=w1871) -> (coerced(x)=w1875:dbl)  [unwired: 1 out]
                      n1205 = Subtract(x=w1877, y=w1886) -> (x-y=w1895:dbl)
                      n1206 = Subtract(x=w1875, y=w1885) -> (x-y=w1894:dbl)
                      n1207 = Square(x=w1895) -> (x^2=w1893:dbl)
                      n1208 = Square(x=w1894) -> (x^2=w1892:dbl)
                      n1209 = Add(x=w1893, y=w1892) -> (x+y=w1891:dbl)
                      n1210 = Square Root(x=w1891) -> (sqrt(x)=w1887:dbl)
                      n1211 = In Range and Coerce(upper limit="Limit Max (MHz)", x=w1887, lower limit="Limit Min (MHz)") -> (In Range?=w1880:bool)  [unwired: 1 out]
                      n1212 = Not(x="Limits Enable") -> (.not. x?=w1879:bool)
                      n1213 = Or(x=w1880, y=w1879) -> (x .or. y?=w1881:bool)
                      n1214 = case shown="True" w1881 {
                        tunnel: w1888 -> [_ w1921]
                        tunnel: w1887 -> [_ w1912]
                        tunnel: w1877 -> [_ w1919]
                        tunnel: w1886 -> [_ w1918]
                        tunnel: w1875 -> [_ w1917]
                        tunnel: w1885 -> [_ w1916]
                        tunnel: w1870 -> [_ w1914]
                        tunnel: w1869 -> [_ w1913]
                        frame False {
                        }
                        frame True {
                          n1215 = local read "BD 1 Frequency 3 (MHz)"() -> (w1920:dbl)
                          n1216 = local read "BD 2 Frequency 3 (MHz)"() -> (w1915:dbl)
                          n1217 = local write "Trap Delta (MHz)"(w1912) -> ()
                          n1218 = property on="Initial delta (MHz)" class="DigNum (strict)"("Val(Sgnl)"=w1912) -> ()  [unwired: 2 in, 2 out]
                          n1219 = call "set RF board frequency - interlace.vi"("Board 2 Frequency Limits"=w1913, "Board 1 Frequency Limits"=w1914, "FPGA VI Reference In"=w1921, "Board 2 Frequency 3 (MHz)"=w1915, "Board 1 Frequency 3 (MHz)"=w1920, "Board 2 Frequency 2 (MHz)"=w1916, "Board 2 Frequency 1 (MHz)"=w1917, "Board 1 Frequency 2 (MHz)"=w1918, "Board 1 Frequency 1  (MHz)"=w1919) -> ()  [unwired: 1 in, 2 out]
                          n1220 = local write "BD 2 Frequency 1 (MHz)"(w1917) -> ()
                          n1221 = local write "BD 1 Frequency 1 (MHz)"(w1919) -> ()
                        }
                      }
                    }
                    frame True {
                    }
                  }
                }
                event Mouse Up {
                  n1222 = event-data() -> ("Button"=w1922:u16)  [unwired: 8 out]
                  n1223 = case shown="3" w1922 {
                    tunnel: [FALSE TRUE] -> w1923
                    frame 0, Default {
                    }
                    frame 3 {
                      n1224 = local write "Manipulating Trap"(FALSE ("Manipulating Trap")) -> ()
                    }
                  }
                }
              }
            }
          }
        }
      }
      event Mouse Move {
        n1225 = event-data() -> ()  [unwired: 6 out]
      }
    }
    n1226 = local read "Stop All"() -> (w1744:bool)
    n1227 = node-c288() -> ()  [unwired: 2 out]
  }
  n1228 = node-c288(i64 1 ("Period"), 1 ("Processor")) -> (w164:T24)  [unwired: 2 out]
  n1229 = timed-loop "Acquire Data" {
    tunnel: w24 -> [w2181]
    tunnel: w40 -> [w2180]
    tunnel: [w2211] -> w33
    tunnel: [w2205] -> w32
    timing: w164 -> [_]
    timing-out: [_] -> w163
    tunnel: w59 -> [w2009]
    stop <- "Stop All" stop-if-true
    (unwired) u32 0 ("Number of Elements")
    w1996 = "NI_ChannelName" ("name")
    n1230 = node-c288() -> ()  [unwired: 2 out]
    n1231 = First Call?() -> (First Call?: T/F=w1962:bool)
    n1232 = Or(x="Reset", y=w1962) -> (x .or. y?=w1963:bool)
    n1233 = case "Reset data stream" shown="True" w1963 {
      tunnel: w2181 -> [w2227 w2235]
      tunnel: w2180 -> [w2226 w2234]
      tunnel: [w2227 w2229] -> w2176
      tunnel: [w2226 w2228] -> w2175
      frame False {
      }
      frame True {
        w2232 = TRUE ("AI to FIFO")
        n1234 = local write "Overflow (data lost)"(FALSE ("Overflow (data lost)")) -> ()
        n1235 = call "reset FPGA DMA.vi"("error in"=w2234, "FPGA VI Reference In"=w2235) -> ("error out"=w2230:errorcluster, "FPGA VI Reference Out"=w2231:T19)
        n1236 = xnode "Read/Write Control"("FPGA VI Reference In"=w2231, "error in"=w2230, "AI to FIFO"=w2232, "APD to FIFO"=w2232) -> ("FPGA VI Reference Out"=w2229:T19, "error out"=w2228:errorcluster)
      }
    }
    n1237 = Or(x="Start AOD Scan", y="Trap Raster Scan") -> (x .or. y?=w2126:bool)
    n1238 = case "Start AOM raster scan" shown="True" w2126 {
      tunnel: w2176 -> [w2964 w2974]
      tunnel: w2175 -> [w2963 w2973]
      tunnel: [w2964 w2967] -> w2174
      tunnel: [w2963 w2966] -> w2173
      frame False {
      }
      frame True {
        n1239 = case shown="True" "Restart DMA? (AOD)" {
          tunnel: [w3012 w3014] -> w2968
          tunnel: [w3011 w3013] -> w2969
          tunnel: w2974 -> [w3012 w3016]
          tunnel: w2973 -> [w3011 w3015]
          frame False {
          }
          frame True {
            n1240 = local write "Overflow (data lost)"(FALSE ("Overflow (data lost)")) -> ()
            n1241 = call "reset FPGA DMA.vi"("error in"=w3015, "FPGA VI Reference In"=w3016) -> ("error out"=w3013:errorcluster, "FPGA VI Reference Out"=w3014:T19)
          }
        }
        n1242 = local write "Trap Raster Scan"(FALSE ("Trap Raster Scan")) -> ()
        n1243 = case shown="False" "Move MCL Also?" {
          tunnel: w2969 -> [w2977 w3006]
          tunnel: w2968 -> [w2978 w3007]
          tunnel: [w2976 w3010] -> w2967
          tunnel: [w2975 w3009] -> w2966
          frame False {
            w2979 = TRUE ("AI to FIFO")
            n1244 = xnode "Read/Write Control"("FPGA VI Reference In"=w2978, "error in"=w2977, "AI to FIFO"=w2979, "APD to FIFO"=w2979, "Start scan"=w2979) -> ("FPGA VI Reference Out"=w2976:T19, "error out"=w2975:errorcluster)
          }
          frame True {
            w3003 = FALSE ("1D or 2D Scan?")
            w3008 = TRUE ("AI to FIFO")
            # "Count for MCL loop"
            # "N total cycles"
            # "N steps"
            # "V_int"
            n1245 = local read "Scan Range (nm)"() -> (w2985:dbl)
            n1246 = local read "Number of F/B Scans (AOD)"() -> (w3002:u16)
            n1247 = Sign(1:w2985) -> (0:w2984:dbl)
            n1248 = Compound Arithmetic op=MULTIPLY(w2985, "MCL Step Position Ratio", "MCL/AOM Scale Tweak") -> (w2989:dbl)
            n1249 = Negate(x=w2984) -> (-x=w2981:dbl)
            n1250 = Multiply(x=w2981, y="MCL Step Increment (V_int)") -> (x*y=w2983:dbl)
            n1251 = Divide(x=w2989, y="MCL X Cal (nm/V)") -> (x/y=w2995:dbl)
            n1252 = Multiply(x=32767.0 ("y"), y=w2995) -> (x*y=w3001:dbl)
            n1253 = local read "Total Counts (ticks)"() -> (w2986:u32)
            n1254 = local read "Cycles/step (AOD)"() -> (w2997:u64)
            n1255 = local read "Scan steps (AOD)"() -> (w2998:u64)
            n1256 = Divide(x=w3001, y=10.0) -> (x/y=w2994:dbl)
            n1257 = Divide(x=w2994, y="MCL Step Increment (V_int)") -> (x/y=w2992:dbl)
            n1258 = Absolute Value(x=w2992) -> (abs(x)=w2980:dbl)
            n1259 = Compound Arithmetic op=MULTIPLY(w2998, w2997, w2986) -> (w2993:u64)
            n1260 = local write "wait to reset values"(w3008) -> ()
            n1261 = local write "MCL Scanning"(w3008) -> ()
            n1262 = Divide(x=w2993, y=w2980) -> (x/y=w2990:dbl)
            "MCL Count" <- w2990
            n1263 = xnode "Read/Write Control"("FPGA VI Reference In"=w3007, "error in"=w3006, "Scan steps (MCL)"=w2980, "Number of scans (MCL)"=w3002, "Cycles per step (MCL)"=u64 1, "Scan freq.  increment (MCL)"=w2983, "1D or 2D Scan?"=w3003, "MCL Scan Axis"=w3003, "Cont. Scan (MCL)"=w3003, "MCL count"=w2990) -> ("FPGA VI Reference Out"=w3005:T19, "error out"=w3004:errorcluster)
            n1264 = xnode "Read/Write Control"("FPGA VI Reference In"=w3005, "error in"=w3004, "AI to FIFO"=w3008, "APD to FIFO"=w3008, "Start scan"=w3008, "Start scan (MCL)"=w3008) -> ("FPGA VI Reference Out"=w3010:T19, "error out"=w3009:errorcluster)
          }
        }
        "Raster Scanning..." <- TRUE ("Scanning...")
      }
    }
    n1265 = And(x="Save scans", y=w2126) -> (x .and. y?=w2172:bool)
    n1266 = Compound Arithmetic op=OR("Start MCL Scan", "Confocal Image", "Confocal Linescan") -> (w2124:bool)
    n1267 = And(x="Save Data (MCL)", y=w2124) -> (x .and. y?=w2171:bool)
    n1268 = case "Start MCL raster scan" shown="True" w2124 {
      tunnel: w2174 -> [w2518 w2533]
      tunnel: w2173 -> [w2517 w2532]
      tunnel: [w2518 w2528] -> w1931
      tunnel: [w2517 w2527] -> w1930
      tunnel: [FALSE w2526] -> w2157
      tunnel: "Start MCL Scan" -> [_ w2521]
      tunnel: "Confocal Image" -> [_ w2520]
      tunnel: "Confocal Linescan" -> [_ _]
      frame False {
      }
      frame True {
        w2526 = TRUE
        n1269 = case shown="True" "Restart DMA? (MCL)" {
          tunnel: [w2578 w2580] -> w2531
          tunnel: [w2577 w2579] -> w2530
          tunnel: w2533 -> [w2578 w2583]
          tunnel: w2532 -> [w2577 w2582]
          frame False {
          }
          frame True {
            n1270 = call "reset FPGA DMA.vi"("error in"=w2582, "FPGA VI Reference In"=w2583) -> ("error out"=w2579:errorcluster, "FPGA VI Reference Out"=w2580:T19)
            n1271 = local write "Overflow (data lost)"(FALSE ("Overflow (data lost)")) -> ()
          }
        }
        n1272 = case shown="False" w2521 {
          selector: w2521 -> [_ w2537]
          tunnel: w2520 -> [w2536 _]
          tunnel: [w2536 w2537] -> w2519
          frame False {
            n1273 = property on="2D or 1D Scan" class="Bool (strict)"("Val(Sgnl)"=w2536) -> ()  [unwired: 2 in, 2 out]
            n1274 = property on="Confocal Image" class="Bool (strict)"("Value"=FALSE ("Start Confocal Map")) -> ()  [unwired: 2 in, 2 out]
          }
          frame True {
          }
        }
        n1275 = local write "MCL Scanning"(w2526) -> ()
        n1276 = local read "AO1"() -> (w2523:dbl)
        n1277 = local read "AO2"() -> (w2522:dbl)
        n1278 = case shown="True" "Center Scan" {
          tunnel: w2531 -> [w2544 w2576]
          tunnel: w2530 -> [w2543 w2575]
          tunnel: [w2542 w2574] -> w2528
          tunnel: [w2541 w2573] -> w2527
          tunnel: [w2539 w2560] -> w2525
          tunnel: [w2538 w2559] -> w2524
          tunnel: w2523 -> [w2539 w2565]
          tunnel: w2522 -> [w2538 w2568]
          tunnel: w2519 -> [_ _]
          frame False {
            w2540 = TRUE ("AI to FIFO")
            n1279 = xnode "Read/Write Control"("FPGA VI Reference In"=w2544, "error in"=w2543, "AI to FIFO"=w2540, "APD to FIFO"=w2540, "Start scan (MCL)"=w2540) -> ("FPGA VI Reference Out"=w2542:T19, "error out"=w2541:errorcluster)
          }
          frame True {
            w2572 = TRUE ("AI to FIFO")
            n1280 = local read "Scan steps (MCL)"() -> (w2551:u64)
            n1281 = local read "Scan lines (y)"() -> (w2547:u64)
            n1282 = local read "Fast Scan Dir"() -> (w2558:bool)
            n1283 = local read "Actual MCL Inc (V)"() -> (w2548:dbl)
            n1284 = Decrement(x=w2547) -> (x-1=w2546:u64)
            n1285 = Decrement(x=w2551) -> (x-1=w2550:u64)
            n1286 = Multiply(x=w2548, y=w2546) -> (x*y=w2545:dbl)
            n1287 = Divide(x=w2545, y=2.0) -> (x/y=w2555:dbl)
            n1288 = Multiply(x=w2548, y=w2550) -> (x*y=w2549:dbl)
            n1289 = Divide(x=w2549, y=2.0) -> (x/y=w2554:dbl)
            n1290 = Select(t=w2554, s=w2558, f=w2555) -> (s? t:f=w2553:dbl)
            n1291 = Select(t=w2555, s=w2558, f=w2554) -> (s? t:f=w2557:dbl)
            n1292 = Subtract(x=w2565, y=w2557) -> (x-y=w2556:dbl)
            n1293 = Subtract(x=w2568, y=w2553) -> (x-y=w2552:dbl)
            n1294 = local read "2D or 1D Scan"() -> (w2570:bool)
            n1295 = Not(x=w2558) -> (.not. x?=w2564:bool)
            n1296 = Not(x=w2570) -> (.not. x?=w2566:bool)
            n1297 = And(x=w2558, y=w2566) -> (x .and. y?=w2567:bool)
            n1298 = And(x=w2566, y=w2564) -> (x .and. y?=w2569:bool)
            n1299 = Select(t=w2568, s=w2569, f=w2552) -> (s? t:f=w2559:dbl)
            n1300 = Select(t=w2565, s=w2567, f=w2556) -> (s? t:f=w2560:dbl)
            n1301 = call "Volt to I16.vi"("Voltage In"=w2560) -> ("I16 Voltage Out"=w2563:i16)
            n1302 = call "Volt to I16.vi"("Voltage In"=w2559) -> ("I16 Voltage Out"=w2562:i16)
            n1303 = xnode "Read/Write Control"("FPGA VI Reference In"=w2576, "error in"=w2575, "AI to FIFO"=w2572, "APD to FIFO"=w2572, "Start scan (MCL)"=w2572, "AO1"=w2563, "AO2"=w2562) -> ("FPGA VI Reference Out"=w2574:T19, "error out"=w2573:errorcluster)
          }
        }
        "Initial Y" <- w2525
        "Initial X" <- w2524
        "wait to reset values" <- w2526
      }
    }
    n1304 = local read "Trap Pos Elements/DMA read"() -> (w2005:u32)
    n1305 = local read "Trap AI Elements/DMA read"() -> (w1929:u32)
    n1306 = local read "APD Elements/DMA read"() -> (w2048:u32)
    n1307 = local read "Trap AI FIFO Depth"() -> (w2221:u32)
    n1308 = xnode "Invoke Method"("FPGA VI Reference In"=w1931, "error in"=w1930, "Number of Elements"=w2005, "Timeout (ms)"=-1) -> ("Data"=w1969:u16[], "Elements Remaining"=→"Trap Pos FIFO El Remaining":u32)  [unwired: 2 out]
    n1309 = xnode "Invoke Method"("FPGA VI Reference In"=w1931, "error in"=w1930, "Number of Elements"=w1929, "Timeout (ms)"=-1 ("Timeout")) -> ("FPGA VI Reference Out"=w1933:T19, "error out"=w1932:errorcluster, "Data"=w1928:i16[], "Elements Remaining"=w1934:u32)
    "Trap AI FIFO El. Rem." <- w1934
    n1310 = xnode "Get APD Data"("FPGA VI Reference In"=w1931, "error in"=w1930, "Number of Elements"=w2048, "Timeout (ms)"=-1) -> ("Data"=w2047:u32[], "Elements Remaining"=→"APD FIFO Elements Remaining":u32)  [unwired: 2 out]
    n1311 = Subtract(x=w2221, y=w1929) -> (x-y=w2220:u32)
    n1312 = Decimate 1D Array(w1969) -> (w1966:u16[], w1968:u16[], w1967:u16[])
    n1313 = Divide(x=w1934, y=w2220) -> (x/y=w2219:dbl)
    "Buffer Status" <- w2219
    n1314 = To Unsigned Long Integer(number=w1966) -> (unsigned 32bit integer=w1965:u32[])
    n1315 = Join Numbers(hi=w1968, lo=w1967) -> ((hi.lo)=w1964:u32[])
    n1316 = Equal?(x=w2219, y=1.0) -> (x = y?=w2217:bool)
    n1317 = Join Numbers(hi=w1965, lo=w1964) -> ((hi.lo)=w1958:u64[])
    n1318 = call "IR AOM word to freq - vec.vi"("Frequency Word In (double vec)"=w1958) -> ("Frequency Out"=w2004:dbl[])
    n1319 = case "Alert buffer overflow" shown="True" w2217 {
      frame False {
      }
      frame True {
        n1320 = call <vilib>:"Beep.vi"() -> ()  [unwired: 3 in, 9 out]
        "Overflow (data lost)" <- TRUE ("Overflow (data lost)")
      }
    }
    n1321 = Decimate 1D Array(w2004) -> (w2003:dbl[], w2002:dbl[])
    n1322 = Array Size(array=w1928) -> (size(s)=→"Waveform Chart":i32)
    n1323 = Build Array(w2003, w2002) -> (w2001:dbl[][])
    n1324 = local read "Trap Sets"() -> (w2085:u32)
    n1325 = case "Deinterlace trap data, average down PSD" shown="2" w2085 {
      tunnel: w1928 -> [w2613 w2678]
      tunnel: [w2610 w2675] -> w2078
      tunnel: [w2613 w2677] -> w1961
      tunnel: "Detector Type" -> [w2612 w2673]
      tunnel: [w2611 w2676] -> w2077
      tunnel: [w2609 w2674] -> w2192
      frame 1, Default {
        n1326 = Divide(x=w2613, y=3276.7) -> (x/y=w2614:dbl[])
        n1327 = Decimate 1D Array(w2614) -> (w2623:dbl[], w2622:dbl[], w2621:dbl[], w2620:dbl[], w2619:dbl[], w2618:dbl[], w2617:dbl[], w2616:dbl[])
        n1328 = case shown="\"IR-QPD + PSD + FB-QPD position\"" w2612 {
          tunnel: w2623 -> [w2647 w2672]
          tunnel: w2622 -> [w2646 w2671]
          tunnel: w2621 -> [w2631 w2649]
          tunnel: w2620 -> [w2632 w2659]
          tunnel: w2619 -> [w2645 w2670]
          tunnel: w2618 -> [w2644 w2669]
          tunnel: w2617 -> [w2628 w2650]
          tunnel: w2616 -> [w2627 w2648]
          tunnel: [w2626 w2656] -> w2611
          tunnel: [w2625 w2655] -> w2610
          tunnel: [w2624 w2654] -> w2609
          frame "IR-QPD + PSD + FB-QPD", Default {
            w2624 = 0  # Channel pattern
            n1329 = Divide(x=w2647, y=w2632) -> (x/y=w2634:dbl[])
            n1330 = Divide(x=w2646, y=w2632) -> (x/y=w2633:dbl[])
            n1331 = Divide(x=w2645, y=w2628) -> (x/y=w2630:dbl[])
            n1332 = Divide(x=w2644, y=w2627) -> (x/y=w2629:dbl[])
            n1333 = Build Array(w2634, w2633, w2632, w2631, w2630, w2629, w2628, w2627) -> (w2625:dbl[][])
            n1334 = Bundle("T1 Y", "T1 X", "T1 Sum", "FB Sum", "PSD Y", "PSD X", "PSD Y Sum", "PSD X Sum") -> (w2643:T41)  [unwired: 1 out]
            n1335 = Cluster To Array(cluster=w2643) -> (array=w2626:string[])
          }
          frame "IR-QPD + PSD + FB-QPD position" {
            w2654 = 3  # Channel pattern
            n1336 = Negate(x=w2650) -> (-x=w2651:dbl[])
            n1337 = Divide(x=w2672, y=w2659) -> (x/y=w2661:dbl[])
            n1338 = Divide(x=w2671, y=w2659) -> (x/y=w2660:dbl[])
            n1339 = Divide(x=w2670, y=w2650) -> (x/y=w2658:dbl[])
            n1340 = Divide(x=w2669, y=w2651) -> (x/y=w2657:dbl[])
            n1341 = Build Array(w2661, w2660, w2659, w2648, w2649, w2658, w2657, w2650) -> (w2655:dbl[][])
            n1342 = Bundle("T1 Y", "T1 X", "T1 Sum", "FB X", "FB Sum", "PSD Y", "PSD X", "PSD Y Sum") -> (w2668:T41)  [unwired: 1 out]
            n1343 = Cluster To Array(cluster=w2668) -> (array=w2656:string[])
          }
        }
      }
      frame 2 {
        n1344 = case shown="\"UCB Fleezers 052511\"" w2673 {
          tunnel: w2678 -> [w2740 w2807 w2835 w2942]
          tunnel: [w2679 w2799 w2830 w2873] -> w2677
          tunnel: [w2706 w2790 w2832 w2920] -> w2676
          tunnel: [w2705 w2754 w2809 w2887] -> w2675
          tunnel: [w2699 w2789 w2872 w2918] -> w2674
          frame "IR-QPD + PSD + FB-QPD", Default {
            w2699 = 1  # Channel pattern
            # "time average x2 the 4th signal and the 4 psd signals (detection laser)"
            # "deinterlace 3 signals from qpd"
            n1345 = Decimate 1D Array(w2740) -> (w2739:i16[], w2738:i16[], w2704:i16[], w2737:i16[], w2727:i16[], w2725:i16[], w2724:i16[], w2722:i16[])
            n1346 = call "downsample 1D array - double.vi"("Ave N"=2.0, "Array In"=w2727) -> ("Array Out"=w2726:dbl[])  [unwired: 1 out]
            n1347 = call "downsample 1D array - double.vi"("Ave N"=2.0, "Array In"=w2722) -> ("Array Out"=w2721:dbl[])  [unwired: 1 out]
            n1348 = call "downsample 1D array - double.vi"("Ave N"=2.0, "Array In"=w2724) -> ("Array Out"=w2723:dbl[])  [unwired: 1 out]
            n1349 = call "downsample 1D array - double.vi"("Ave N"=2.0, "Array In"=w2725) -> ("Array Out"=w2707:dbl[])  [unwired: 1 out]
            n1350 = Decimate 1D Array(w2739) -> (w2736:i16[], w2708:i16[])
            n1351 = Decimate 1D Array(w2738) -> (w2735:i16[], w2733:i16[])
            n1352 = Decimate 1D Array(w2737) -> (w2734:i16[], w2732:i16[])
            n1353 = Decimate 1D Array(w2704) -> (w2703:i16[], w2702:i16[])
            n1354 = Interleave 1D Arrays(w2736, w2735, w2734, w2708, w2733, w2732, w2703, w2702, w2726, w2707, w2723, w2721) -> (w2720:dbl[])
            n1355 = To Word Integer(number=w2720) -> (16bit integer=w2679:i16[])
            n1356 = Divide(x=w2720, y=3276.7) -> (x/y=w2719:dbl[])
            n1357 = Decimate 1D Array(w2719) -> (w2718:dbl[], w2717:dbl[], w2716:dbl[], w2715:dbl[], w2714:dbl[], w2713:dbl[], w2701:dbl[], w2700:dbl[], w2712:dbl[], w2711:dbl[], w2710:dbl[], w2709:dbl[])
            n1358 = Divide(x=w2718, y=w2716) -> (x/y=w2686:dbl[])
            n1359 = Divide(x=w2717, y=w2716) -> (x/y=w2685:dbl[])
            n1360 = Divide(x=w2715, y=w2713) -> (x/y=w2684:dbl[])
            n1361 = Divide(x=w2714, y=w2713) -> (x/y=w2683:dbl[])
            n1362 = Divide(x=w2712, y=w2710) -> (x/y=w2682:dbl[])
            n1363 = Divide(x=w2711, y=w2709) -> (x/y=w2681:dbl[])
            n1364 = Bundle("T1 Y", "T1 X", "T1 Sum", "T2 Y", "T2 X", "T2 Sum", "T1 FB Sum", "T2 FB Sum", "PSD Y", "PSD X", "PSD Y Sum", "PSD X Sum") -> (w2687:T42)  [unwired: 1 out]
            n1365 = Build Array(w2686, w2685, w2716, w2684, w2683, w2713, w2701, w2700, w2682, w2681, w2710, w2709) -> (w2705:dbl[][])
            n1366 = Cluster To Array(cluster=w2687) -> (array=w2706:string[])
          }
          frame "IR-QPD + PSD + FB-QPD X position" {
            w2789 = 2  # Channel pattern
            # "convert\nADC numbers\nto volts"
            # "time average x2 the 3 psd signals (detection laser)"
            # "deinterlace 3 signals from qpds"
            n1367 = Decimate 1D Array(w2807) -> (w2806:i16[], w2805:i16[], w2742:i16[], w2743:i16[], w2752:i16[], w2749:i16[], w2746:i16[], w2777:i16[])
            n1368 = Decimate 1D Array(w2806) -> (w2804:i16[], w2791:i16[])
            n1369 = call "downsample 1D array - I16.vi"("Ave N"=2.0, "Array In"=w2752) -> ("Array Out"=w2750:i16[])  [unwired: 1 in]
            n1370 = call "downsample 1D array - I16.vi"("Ave N"=2.0, "Array In"=w2749) -> ("Array Out"=w2747:i16[])  [unwired: 1 in]
            n1371 = Decimate 1D Array(w2805) -> (w2803:i16[], w2801:i16[])
            n1372 = Decimate 1D Array(w2743) -> (w2802:i16[], w2800:i16[])
            n1373 = Decimate 1D Array(w2777) -> (w2776:i16[], w2774:i16[])
            n1374 = Decimate 1D Array(w2742) -> (w2775:i16[], w2773:i16[])
            n1375 = call "downsample 1D array - I16.vi"("Ave N"=2.0, "Array In"=w2746) -> ("Array Out"=w2744:i16[])  [unwired: 1 in]
            n1376 = Interleave 1D Arrays(w2804, w2803, w2802, w2791, w2801, w2800, w2776, w2775, w2774, w2773, w2750, w2747, w2744) -> (w2799:i16[])
            n1377 = Divide(x=w2799, y=3276.7) -> (x/y=w2798:dbl[])
            n1378 = Decimate 1D Array(w2798) -> (w2797:dbl[], w2796:dbl[], w2795:dbl[], w2794:dbl[], w2793:dbl[], w2792:dbl[], w2765:dbl[], w2763:dbl[], w2762:dbl[], w2760:dbl[], w2759:dbl[], w2758:dbl[], w2755:dbl[])
            n1379 = Divide(x=w2797, y=w2795) -> (x/y=w2781:dbl[])
            n1380 = Divide(x=w2796, y=w2795) -> (x/y=w2780:dbl[])
            n1381 = Divide(x=w2794, y=w2792) -> (x/y=w2779:dbl[])
            n1382 = Divide(x=w2793, y=w2792) -> (x/y=w2778:dbl[])
            n1383 = Divide(x=w2765, y=w2763) -> (x/y=w2764:dbl[])
            n1384 = Divide(x=w2762, y=w2760) -> (x/y=w2761:dbl[])
            n1385 = Divide(x=w2759, y=w2755) -> (x/y=w2757:dbl[])
            n1386 = Negate(x=w2755) -> (-x=w2753:dbl[])
            n1387 = Divide(x=w2758, y=w2753) -> (x/y=w2756:dbl[])
            n1388 = Bundle("T1 Y", "T1 X", "T1 Sum", "T2 Y", "T2 X", "T2 Sum", "T1 FB X", "T1 FB Sum", "T2 FB X", "T2 FB Sum", "PSD Y", "PSD X", "PSD Y Sum") -> (w2782:T43)  [unwired: 1 out]
            n1389 = Build Array(w2781, w2780, w2795, w2779, w2778, w2792, w2764, w2763, w2761, w2760, w2757, w2756, w2755) -> (w2754:dbl[][])
            n1390 = Cluster To Array(cluster=w2782) -> (array=w2790:string[])
          }
          frame "UCB Fleezers 052511" {
            w2872 = 2  # Channel pattern
            n1391 = Decimate 1D Array(w2835) -> (w2870:i16[], w2869:i16[], w2834:i16[], w2833:i16[], w2827:i16[], w2824:i16[], w2823:i16[], w2822:i16[])
            n1392 = Decimate 1D Array(w2870) -> (w2868:i16[], w2853:i16[])
            n1393 = Decimate 1D Array(w2869) -> (w2867:i16[], w2865:i16[])
            n1394 = Decimate 1D Array(w2834) -> (w2866:i16[], w2864:i16[])
            n1395 = Decimate 1D Array(w2833) -> (w2829:i16[], w2828:i16[])
            n1396 = Decimate 1D Array(w2827) -> (w2826:i16[], w2825:i16[])
            n1397 = call "downsample 1D array - I16.vi"("Ave N"=2.0, "Array In"=w2824) -> ("Array Out"=w2821:i16[])  [unwired: 1 in]
            n1398 = call "downsample 1D array - I16.vi"("Ave N"=2.0, "Array In"=w2823) -> ("Array Out"=w2820:i16[])  [unwired: 1 in]
            n1399 = call "downsample 1D array - I16.vi"("Ave N"=2.0, "Array In"=w2822) -> ("Array Out"=w2819:i16[])  [unwired: 1 in]
            n1400 = Interleave 1D Arrays(w2868, w2867, w2866, w2853, w2865, w2864, w2829, w2826, w2828, w2825, w2821, w2820, w2819) -> (w2830:i16[])
            n1401 = Divide(x=w2830, y=3276.7) -> (x/y=w2860:dbl[])
            n1402 = Decimate 1D Array(w2860) -> (w2859:dbl[], w2858:dbl[], w2857:dbl[], w2856:dbl[], w2855:dbl[], w2854:dbl[], w2818:dbl[], w2816:dbl[], w2815:dbl[], w2813:dbl[], w2812:dbl[], w2811:dbl[], w2810:dbl[])
            n1403 = Divide(x=w2859, y=w2857) -> (x/y=w2840:dbl[])
            n1404 = Divide(x=w2858, y=w2857) -> (x/y=w2839:dbl[])
            n1405 = Divide(x=w2856, y=w2854) -> (x/y=w2838:dbl[])
            n1406 = Divide(x=w2855, y=w2854) -> (x/y=w2837:dbl[])
            n1407 = Divide(x=w2818, y=w2816) -> (x/y=w2817:dbl[])
            n1408 = Divide(x=w2815, y=w2813) -> (x/y=w2814:dbl[])
            n1409 = Bundle("T1 Y", "T1 X", "T1 Sum", "T2 Y", "T2 X", "T2 Sum", "T1 FB X", "T2 FB Sum", "T2 FB X", "T2 FB Sum", "PSD Y", "PSD X", "PSD Sum") -> (w2841:T43)  [unwired: 1 out]
            n1410 = Build Array(w2840, w2839, w2857, w2838, w2837, w2854, w2817, w2816, w2814, w2813, w2812, w2811, w2810) -> (w2809:dbl[][])
            n1411 = Cluster To Array(cluster=w2841) -> (array=w2832:string[])
          }
          frame "IR-QPD + PSD + FB-QPD XY positions" {
            w2918 = 4  # Channel pattern
            # "time average x2 the 3 psd signals (detection laser)"
            # "deinterlace 3 signals from qpds"
            n1412 = Decimate 1D Array(w2942) -> (w2941:i16[], w2940:i16[], w2919:i16[], w2939:i16[], w2885:i16[], w2931:i16[], w2930:i16[], w2907:i16[])
            n1413 = Decimate 1D Array "QPD Y"(w2941) -> (w2938:i16[], w2921:i16[])
            n1414 = call "downsample 1D array - double.vi"("Ave N"=2.0, "Array In"=w2931) -> ("Array Out"=w2906:dbl[])  [unwired: 1 out]
            n1415 = call "downsample 1D array - double.vi"("Ave N"=2.0, "Array In"=w2930) -> ("Array Out"=w2905:dbl[])  [unwired: 1 out]
            n1416 = Decimate 1D Array "Feedback Sum"(w2919) -> (w2903:i16[], w2901:i16[])
            n1417 = Decimate 1D Array "Feedback Y"(w2885) -> (w2884:i16[], w2883:i16[])
            n1418 = Decimate 1D Array "Feedback X"(w2907) -> (w2904:i16[], w2902:i16[])
            n1419 = Decimate 1D Array "QPD Sum"(w2939) -> (w2936:i16[], w2934:i16[])
            n1420 = Decimate 1D Array "QPD X"(w2940) -> (w2937:i16[], w2935:i16[])
            n1421 = Interleave 1D Arrays(w2938, w2937, w2936, w2921, w2935, w2934, w2884, w2904, w2903, w2883, w2902, w2901, w2906, w2905) -> (w2929:dbl[])
            n1422 = To Word Integer(number=w2929) -> (16bit integer=w2873:i16[])
            n1423 = Divide(x=w2929, y=3276.7) -> (x/y=w2928:dbl[])
            n1424 = Decimate 1D Array(w2928) -> (w2927:dbl[], w2926:dbl[], w2925:dbl[], w2924:dbl[], w2923:dbl[], w2922:dbl[], w2880:dbl[], w2894:dbl[], w2878:dbl[], w2879:dbl[], w2892:dbl[], w2876:dbl[], w2890:dbl[], w2888:dbl[])
            n1425 = Divide(x=w2927, y=w2925) -> (x/y=w2911:dbl[])
            n1426 = Divide(x=w2926, y=w2925) -> (x/y=w2910:dbl[])
            n1427 = Divide(x=w2924, y=w2922) -> (x/y=w2909:dbl[])
            n1428 = Divide(x=w2923, y=w2922) -> (x/y=w2908:dbl[])
            n1429 = Divide(x=w2880, y=w2878) -> (x/y=w2877:dbl[])
            n1430 = Divide(x=w2894, y=w2878) -> (x/y=w2893:dbl[])
            n1431 = Divide(x=w2879, y=w2876) -> (x/y=w2875:dbl[])
            n1432 = Divide(x=w2892, y=w2876) -> (x/y=w2891:dbl[])
            n1433 = Negate(x=w2888) -> (-x=w2886:dbl[])
            n1434 = Divide(x=w2890, y=w2886) -> (x/y=w2889:dbl[])
            n1435 = Bundle("T1 Y", "T1 X", "T1 Sum", "T2 Y", "T2 X", "T2 Sum", "T1 FB Y", "T1 FB X", "T1 FB Sum", "T2 FB Y", "T2 FB X", "T2 FB Sum", "PSD X", "PSD Y Sum") -> (w2874:T44)  [unwired: 1 out]
            n1436 = Build Array(w2911, w2910, w2925, w2909, w2908, w2922, w2877, w2893, w2878, w2875, w2891, w2876, w2889, w2888) -> (w2887:dbl[][])
            n1437 = Cluster To Array(cluster=w2874) -> (array=w2920:string[])
          }
        }
      }
    }
    "AI labels" <- w2077
    n1438 = Decimate 1D Array(w2047) -> (w2075:u32[], w2011:u32[])
    n1439 = local read "DMA Update Period (s)"() -> (w2086:dbl)
    n1440 = local read "BD 1 Frequency 2 (MHz)"() -> (w1953:dbl)
    n1441 = local read "BD 1 Frequency 1 (MHz)"() -> (w1954:dbl)
    n1442 = Build Array(w2075, w2011) -> (w2154:u32[][])
    n1443 = local read "Data Period (s)"() -> (w2060:dbl)
    n1444 = Decimate 1D Array(w1961) -> (w1984:i16[], w1983:i16[], w1981:i16[], w1980:i16[])  [unwired: 9 out]
    n1445 = To Double Precision Float(number=w2154) -> (double precision float=w2155:dbl[][])
    n1446 = local read "APD Integration Time (s)"() -> (w2024:dbl)
    n1447 = Divide(x=w1984, y=w1983) -> (x/y=w1985:dbl[])
    n1448 = Divide(x=w1981, y=w1980) -> (x/y=w1982:dbl[])
    n1449 = feedback #1(0.0) -> (w1998:dbl)
    n1450 = Add(x=w2086, y=w1998) -> (x+y=w2194:dbl)
    n1451 = feedback-in #1(w2194) -> ()
    n1452 = local read "AOM X Cal (nm/MHz)"() -> (w1951:dbl)
    n1453 = To Time Stamp(1:w1998) -> (0:w1997:timestamp)
    n1454 = Split 1D Array(array=w1985, index="N El. to Ave.") -> (second subarray=w1988:dbl[])  [unwired: 1 out]
    n1455 = Split 1D Array(array=w1982, index="N El. to Ave.") -> (second subarray=w1987:dbl[])  [unwired: 1 out]
    n1456 = local read "Trap X AI1 (DMA)"() -> (w1986:T13)
    n1457 = Multiply(x=w2060, y="Trap Disp. Downsample") -> (x*y=w1999:dbl)
    "Display Period (s)" <- w1999
    n1458 = Bundle("BD 1 Frequency 1 (MHz)"=w1954, "BD 1 Frequency 2 (MHz)"=w1953) -> (w1955:T45)  [unwired: 1 out]
    n1459 = for "Trap AI" {
      tunnel: [w2608] -> w2188 mode=indexing
      tunnel: w1997 -> [w2598]
      tunnel: "Trap Disp. Downsample" -> [w2606]
      tunnel: w2078 -> [w2604] mode=indexing
      tunnel: w2060 -> [w2603]
      tunnel: w2077 -> [w2602] mode=indexing
      tunnel: w1996 -> [w2601]
      tunnel: [w2600] -> w2035 mode=indexing
      tunnel: w1999 -> [w2599]
      n1460 = Bundle By Name("Y"=w2604, "dt"=w2603) -> (w2605:waveform(dbl))  [unwired: 1 out]
      n1461 = Set Waveform Attribute(5:w2602, 6:w2601, 7:w2605) -> (3:w2600:waveform(dbl))  [unwired: 1 in, 2 out]
      n1462 = call "downsample 1D array - double.vi"("Ave N"=w2606, "Array In"=w2604) -> ("Array Out"=w2607:dbl[])  [unwired: 1 out]
      n1463 = Bundle By Name(cluster=w2600, "t0"=w2598, "Y"=w2607, "dt"=w2599) -> (w2608:waveform(dbl))
    }
    n1464 = call-poly <vilib>:"Mean.vi"("X"=w1987) -> ("mean"=w1975:dbl)  [unwired: 1 out]
    n1465 = call-poly <vilib>:"Mean.vi"("X"=w1988) -> ("mean"=w1976:dbl)  [unwired: 1 out]
    n1466 = Cluster To Array(cluster=w1955) -> (array=w1952:dbl[])
    n1467 = Reciprocal(x=w1999) -> (1/x=→"Trap Disp. Freq. (Hz)":dbl)
    n1468 = local read "Data points/scans (MCL)"() -> (w2166:dbl)
    n1469 = To Fixed-Point(number=w1975) -> (fixed-point=w1973:fxp<+/-,16,1>)  [unwired: 1 in]
    n1470 = To Fixed-Point(number=w1976) -> (fixed-point=w1974:fxp<+/-,16,1>)  [unwired: 1 in]
    n1471 = Bundle("Trap 1 Pos.", "Trap 2 Pos.") -> (w1995:cluster{string, string})  [unwired: 1 out]
    n1472 = Bundle By Name(cluster=w1986, "Set 1"=w1974, "Set 2"=w1973) -> (→"Trap X AI1 (DMA)":T13)
    n1473 = Cluster To Array(cluster=w1995) -> (array=w1992:string[])
    n1474 = for "Trap Position" {
      tunnel: w2001 -> [w2248] mode=indexing
      tunnel: "Trap Disp. Downsample" -> [w2247]
      tunnel: w1999 -> [w2245]
      tunnel: w1997 -> [w2244]
      tunnel: w1996 -> [w2242]
      tunnel: w1992 -> [w2241] mode=indexing
      tunnel: [w2240] -> w1950 mode=indexing
      tunnel: w1952 -> [w2238] mode=indexing
      tunnel: w1951 -> [w2236]
      n1475 = call "downsample 1D array - double.vi"("Ave N"=w2247, "Array In"=w2248) -> ("Array Out"=w2246:dbl[])  [unwired: 1 out]
      n1476 = Subtract(x=w2246, y=w2238) -> (x-y=w2239:dbl[])
      n1477 = Multiply(x=w2236, y=w2239) -> (x*y=w2237:dbl[])
      n1478 = Bundle By Name("Y"=w2237, "dt"=w2245, "t0"=w2244) -> (w2243:waveform(dbl))  [unwired: 1 out]
      n1479 = Set Waveform Attribute(5:w2241, 6:w2242, 7:w2243) -> (3:w2240:waveform(dbl))  [unwired: 1 in, 2 out]
    }
    "Trap Positions" <- w1950
    n1480 = Bundle("APD 1", "APD 2") -> (w2187:cluster{string, string})  [unwired: 1 out]
    n1481 = Cluster To Array(cluster=w2187) -> (array=w2184:string[])
    n1482 = for "APD" {
      tunnel: w2155 -> [w2587] mode=indexing
      tunnel: w2024 -> [w2595]
      tunnel: [w2591] -> w2031 mode=indexing
      tunnel: "APD Disp. Scale" -> [w2592]
      tunnel: w1996 -> [w2590]
      tunnel: w2184 -> [w2589] mode=indexing
      tunnel: "APD Disp. Downsample" -> [w2585]
      tunnel: [w2588] -> w2183
      tunnel: w1997 -> [w2584]
      n1483 = call "integrate 1D array interval - double.vi"("Ave N"=w2585, "Array In"=w2587) -> ("Array Out"=w2586:dbl[])  [unwired: 1 out]
      n1484 = Multiply(x=w2595, y=w2585) -> (x*y=w2588:dbl)
      n1485 = Divide(x=w2586, y=w2592) -> (x/y=w2593:dbl[])
      n1486 = Bundle By Name("t0"=w2584, "Y"=w2593, "dt"=w2588) -> (w2594:waveform(dbl))  [unwired: 1 out]
      n1487 = Set Waveform Attribute(5:w2589, 6:w2590, 7:w2594) -> (3:w2591:waveform(dbl))  [unwired: 1 in, 2 out]
    }
    "APD Display Period (s)" <- w2183
    n1488 = Reciprocal(x=w2183) -> (1/x=→"APD Display Freq. (Hz)":dbl)
    n1489 = local read "Display Period (s)"() -> (w2059:dbl)
    n1490 = Increment(x=w2166) -> (x+1=w2167:dbl)
    n1491 = Index Array(array=w1950, index=0) -> (element=w1948:waveform(dbl))
    n1492 = To Double Precision Float(number=w2075) -> (double precision float=w2074:dbl[])
    n1493 = feedback #2(w2167) -> (w2170:dbl)
    n1494 = Select(t=0, s=w2157, f=w2170) -> (s? t:f=w2163:dbl)
    n1495 = Array Size(array=w2074) -> (size(s)=w2169:i32)
    n1496 = Add(x=w2169, y=w2163) -> (x+y=w2164:dbl)
    n1497 = Unbundle By Name(w1948) -> ("Y"=w1946:dbl[])
    n1498 = feedback #3(w2075) -> (w2153:u32[])
    n1499 = Build Array (concatenate)(w2153, w2075) -> (w2150:u32[])
    n1500 = feedback #4(w2011) -> (w2030:u32[])
    n1501 = Divide(x="Bead Sep. Int. Time (s)", y=w2059) -> (x/y=w1944:dbl)
    n1502 = Build Array (concatenate)(w2030, w2011) -> (w2029:u32[])
    n1503 = Greater?(x=w2164, y=w2166) -> (0:w2165:bool)
    n1504 = feedback #5(w1946) -> (w1947:dbl[])
    n1505 = Build Array (concatenate)(w1946, w1947) -> (w1945:dbl[])
    n1506 = Select(t=w2163, s=w2165, f=w2164) -> (s? t:f=w2162:dbl)
    n1507 = feedback-in #2(w2162) -> ()
    n1508 = Array Size(array=w2150) -> (size(s)=w2147:i32)
    n1509 = Array Size(array=w2075) -> (size(s)=w2149:i32)
    n1510 = local read "MCL Scanning"() -> (w2160:bool)
    n1511 = local read "APD Integration Time (s)"() -> (w2038:dbl)
    n1512 = Build Array (concatenate)(w2031, w2188) -> (w2033:waveform(dbl)[])
    "All Signals" <- w2033
    n1513 = Split 1D Array(array=w1945, index=w1944) -> (first subarray=w1938:dbl[])  [unwired: 1 out]
    n1514 = feedback-in #5(w1938) -> ()
    n1515 = Multiply(x=w2149, y="APD Ave N") -> (x*y=w2148:dbl)
    n1516 = Greater?(x=w2147, y=w2148) -> (0:w2151:bool)
    n1517 = Not(x=w2165) -> (.not. x?=w2159:bool)
    n1518 = To Double Precision Float(number=w2011) -> (double precision float=w2010:dbl[])
    n1519 = call-poly <vilib>:"Mean.vi"("X"=w1938) -> ("mean"=w1937:dbl)  [unwired: 1 out]
    "Mean T1 Position (nm)" <- w1937
    n1520 = Subtract(x=w1938, y=w1937) -> (x-y=w1943:dbl[])
    n1521 = Square(x=w1943) -> (x^2=w1942:dbl[])
    n1522 = And(x=w2159, y=w2160) -> (x .and. y?=w2161:bool)
    n1523 = call-poly <vilib>:"Mean.vi"("X"=w1942) -> ("mean"=w1941:dbl)  [unwired: 1 out]
    n1524 = case shown="True" w2151 {
      tunnel: w2150 -> [w2368 w2375]
      tunnel: [w2368 w2373] -> w2091
      tunnel: w2148 -> [_ w2370]
      tunnel: w2147 -> [_ w2374]
      tunnel: w2029 -> [w2367 w2372]
      tunnel: [w2367 w2369] -> w2026
      frame False {
      }
      frame True {
        n1525 = Subtract(x=w2374, y=w2370) -> (x-y=w2371:dbl)
        n1526 = Array Subset(array=w2375, index=w2371, length=w2370) -> (w2373:u32[])
        n1527 = Array Subset(array=w2372, index=w2371, length=w2370) -> (w2369:u32[])
      }
    }
    n1528 = feedback-in #3(w2091) -> ()
    n1529 = feedback-in #4(w2026) -> ()
    n1530 = Or(x=w2161, y=w2157) -> (x .or. y?=w2158:bool)
    n1531 = Square Root(x=w1941) -> (sqrt(x)=w1940:dbl)
    n1532 = Equal?(x="Tab Control 6", y=T35."High Res Display") -> (x = y?=w2081:bool)
    n1533 = Multiply(x="APD Disp. Scale", y=w2031) -> (x*y=w2040:waveform(dbl)[])
    n1534 = Multiply(x="APD Disp. Downsample", y=w2038) -> (x*y=w2036:dbl)
    n1535 = Multiply(x=10.0, y=w1940) -> (x*y=→"Trap 1 Position RMS (A)":dbl)
    n1536 = Divide(x=w2040, y=w2036) -> (x/y=w2008:waveform(dbl)[])
    n1537 = Index Array(array=w2008, index=0) -> (element=w2018:waveform(dbl))
    n1538 = case "For computing FFTs for display" shown="True" "Compute FFT" {
      tunnel: w2035 -> [_ w3045]
      frame False {
      }
      frame True {
        n1539 = Build Array("FFT 1 Choice 1", "FFT 1 Choice 2", "FFT 2 Choice 1", "FFT 2 Choice 2") -> (w3038:u16[])
        n1540 = Array Size(array=w3045) -> (size(s)=w3044:i32)
        n1541 = feedback-in #6(w3038) -> ()
        n1542 = feedback #6(u16[] [100, 100, 100, 100]) -> (w3039:u16[])
        n1543 = feedback-in #7("# Spectra to Ave.") -> ()
        n1544 = feedback #7("# Spectra to Ave.") -> (w3036:dbl)
        n1545 = Not Equal?(x="# Spectra to Ave.", y=w3036) -> (x != y?=w3035:bool)
        n1546 = Not Equal?(x=w3038, y=w3039) -> (x != y?=w3037:bool)
        n1547 = feedback #8(1.0) -> (w3022:dbl)
        n1548 = Compound Arithmetic op=OR("Reset FFT", w3037, w3035) -> (w3020:bool)
        n1549 = Select(t=1.0, s=w3020, f=w3022) -> (s? t:f=w3024:dbl)
        n1550 = Greater?(x=w3024, y="# Spectra to Ave.") -> (0:w3043:bool)
        n1551 = Increment(x=w3024) -> (x+1=w3023:dbl)
        n1552 = feedback-in #8(w3023) -> ()
        n1553 = local read "DMA Update Period (s)"() -> (w3018:dbl)
        n1554 = Multiply(x="# Spectra to Ave.", y=w3018) -> (x*y=→"Ave. Time (s)":dbl)
        n1555 = Build Array(cluster{"f0":dbl, "df":dbl, "magnitude":dbl[]} {"f0"=0.0, "df"=0.0, "magnitude"=[]} ("PSD")) -> (w3027:cluster{"f0":dbl, "df":dbl, "magnitude":dbl[]}[])
        n1556 = Build Array(w3027, w3027, w3027, w3027) -> (w3029:T46)
        n1557 = feedback #9(w3029) -> (w3034:T46)
        n1558 = for {
          N: 4 -> [_]
          tunnel: w3038 -> [w3067] mode=indexing
          tunnel: w3045 -> [w3068]
          tunnel: w3044 -> [w3070]
          tunnel: w3020 -> [w3063]
          tunnel: w3043 -> [w3062]
          tunnel: "# Spectra to Ave." -> [w3061]
          tunnel: [w3060] -> w3033 mode=indexing
          tunnel: w3034 -> [w3065] mode=indexing
          tunnel: [w3064] -> w3021 mode=indexing
          tunnel: w3024 -> [w3059]
          n1559 = Less?(x=w3067, y=w3070) -> (x < y?=w3069:bool)
          n1560 = Index Array(array=w3068, index=w3067) -> (element=w3066:waveform(dbl))
          n1561 = case shown="True" w3069 {
            tunnel: w3066 -> [_ w3087]
            tunnel: w3065 -> [w3072 w3085]
            tunnel: [w3072 w3073] -> w3064
            tunnel: w3063 -> [_ w3084]
            tunnel: w3062 -> [_ w3077]
            tunnel: w3061 -> [_ w3076]
            tunnel: [cluster{"f0":dbl, "df":dbl, "magnitude":dbl[]} {"f0"=0.0, "df"=0.0, "magnitude"=[]} ("PSD") w3078] -> w3060
            tunnel: w3059 -> [_ w3075]
            frame False {
            }
            frame True {
              n1562 = call <vilib>:"Std Deviation and Variance.vi"("X"=w3087) -> ("mean"=w3088:dbl)  [unwired: 1 in, 2 out]
              n1563 = Subtract(x=w3087, y=w3088) -> (x-y=w3086:waveform(dbl))
              n1564 = xnode "Spectral Measurements"("Signals"=w3086) -> ("PSD"=w3080:cluster{"f0":dbl, "df":dbl, "magnitude":dbl[]})  [unwired: 1 in, 1 out]
              n1565 = case shown="False" w3084 {
                tunnel: w3085 -> [w3097 _]
                tunnel: [w3093 w3102] -> w3073
                tunnel: w3080 -> [w3096 w3103]
                tunnel: w3077 -> [w3095 _]
                frame False {
                  n1566 = Build Array (concatenate)(w3097, w3096) -> (w3094:cluster{"f0":dbl, "df":dbl, "magnitude":dbl[]}[])
                  n1567 = case shown="True" w3095 {
                    tunnel: w3094 -> [w3098 w3101]
                    tunnel: [w3098 w3099] -> w3093
                    frame False {
                    }
                    frame True {
                      n1568 = Delete From Array(array=w3101, index=0) -> (array with subset deleted=w3099:cluster{"f0":dbl, "df":dbl, "magnitude":dbl[]}[])  [unwired: 1 in, 1 out]
                    }
                  }
                }
                frame True {
                  n1569 = Build Array(w3103) -> (w3102:cluster{"f0":dbl, "df":dbl, "magnitude":dbl[]}[])
                }
              }
              n1570 = for {
                tunnel: w3073 -> [w3092] mode=indexing
                tunnel: [w3091] -> w3083 mode=indexing
                workers-P: _ -> [_]
                n1571 = Unbundle By Name(w3092) -> ("magnitude"=w3091:dbl[])
              }
              n1572 = Transpose 2D Array(2D array=w3083) -> (transposed array=w3082:dbl[][])
              n1573 = for {
                tunnel: w3082 -> [w3090] mode=indexing
                tunnel: [w3089] -> w3081 mode=indexing
                workers-P: _ -> [_]
                n1574 = Add Array Elements(numeric array=w3090) -> (sum=w3089:dbl)
              }
              n1575 = Select(t=w3076, s=w3077, f=w3075) -> (s? t:f=w3074:dbl)
              n1576 = Divide(x=w3081, y=w3074) -> (x/y=w3079:dbl[])
              n1577 = Bundle By Name(cluster=w3080, "magnitude"=w3079) -> (w3078:cluster{"f0":dbl, "df":dbl, "magnitude":dbl[]})
            }
          }
        }
        n1578 = case shown="True" w3020 {
          tunnel: w3021 -> [w3052 w3058]
          tunnel: [w3052 w3053] -> w3019
          frame False {
          }
          frame True {
            n1579 = Array Subset(array=w3058, index (row)=0 ("index"), length (row)=4 ("length"), index (col)=0 ("index"), length (col)=1 ("length")) -> (w3053:T46)
          }
        }
        n1580 = feedback-in #9(w3019) -> ()
        n1581 = Split 1D Array(array=w3033, index=2) -> (first subarray=→"FFT 1":cluster{"f0":dbl, "df":dbl, "magnitude":dbl[]}[], second subarray=→"FFT 2":cluster{"f0":dbl, "df":dbl, "magnitude":dbl[]}[])
      }
    }
    n1582 = Index Array(array=w2008, index=1) -> (element=w2016:waveform(dbl))
    n1583 = case "For displaying the high resolution display (no downsampling)" shown="True" w2081 {
      tunnel: w2035 -> [_ w2268]
      frame False {
      }
      frame True {
        n1584 = Index Array(array=w2268, index="High Res. Display") -> (element=w2269:waveform(dbl))
        n1585 = call <vilib>:"Std Deviation and Variance.vi"("X"=w2269) -> ("mean"=w2276:dbl, "standard deviation"=w2281:dbl)  [unwired: 1 in, 1 out]
        "Mean Intensity" <- w2276
        "Sigma" <- w2281
        n1586 = Subtract(x=w2269, y=w2276) -> (x-y=w2275:waveform(dbl))
        n1587 = Select(t=w2275, s="Subtract mean", f=w2269) -> (s? t:f=→"1 Channel":waveform(dbl))
        n1588 = Divide(x=w2281, y=w2276) -> (x/y=→"Sigma/Mean":dbl)
        n1589 = feedback #10(1) -> (w2270:i32)
        n1590 = Greater Or Equal?(x=w2270, y="Slow mean N ave.") -> (x >= y?=w2283:bool)
        n1591 = Increment(x=w2270) -> (x+1=w2285:i32)
        n1592 = Select(t=1, s=w2283, f=w2285) -> (s? t:f=w2272:i32)
        n1593 = feedback-in #10(w2272) -> ()
        n1594 = feedback #11() -> (w2273:waveform(dbl))  [unwired: 1 out]
        n1595 = case shown="Default" w2270 {
          tunnel: [w2288 w2291] -> w2274
          tunnel: w2273 -> [w2290 _]
          tunnel: w2269 -> [w2289 w2291]
          frame Default {
            n1596 = call-poly <vilib>:"Append Waveforms.vi"("waveform B"=w2289, "waveform A"=w2290) -> ("waveform out"=w2288:waveform(dbl))  [unwired: 1 in, 8 out]
          }
          frame 1 {
          }
        }
        n1597 = feedback-in #11(w2274) -> ()
        n1598 = case shown="True" w2283 {
          tunnel: w2274 -> [_ w2287]
          frame False {
          }
          frame True {
            n1599 = call-poly <vilib>:"Mean.vi"("X"=w2287) -> ("mean"=→"Slow mean":dbl)  [unwired: 1 out]
          }
        }
      }
    }
    n1600 = case "For plotting results of scanning MCL" shown="True" w2158 {
      tunnel: w2157 -> [_ w2408]
      tunnel: w2074 -> [_ w2504]
      tunnel: w2166 -> [_ _]
      tunnel: w2035 -> [_ w2478]
      tunnel: w2010 -> [_ w2409]
      tunnel: w2009 -> [_ w2382]
      frame False {
      }
      frame True {
        w2389 = u32 0 items=["Horizontal", "Vertical", "Central", "1st Diagonal", "2nd Diagonal"] ("Type of Symmetry")
        w2417 = u32 0 items=["Horizontal", "Vertical", "Central", "1st Diagonal", "2nd Diagonal"] ("Type of Symmetry")
        w2420 = u32 0 items=["Horizontal", "Vertical", "Central", "1st Diagonal", "2nd Diagonal"] ("Type of Symmetry")
        w2449 = u32 0 items=["Horizontal", "Vertical", "Central", "1st Diagonal", "2nd Diagonal"] ("Type of Symmetry")
        n1601 = Index Array(array=w2478, index=10) -> (element=w2484:waveform(dbl))
        n1602 = Index Array(array=w2478, index=11) -> (element=w2481:waveform(dbl))
        n1603 = local read "Cycles/step (MCL)"() -> (w2434:u64)
        n1604 = Index Array(array=w2478, index="Channel") -> (element=w2480:waveform(dbl))
        n1605 = Unbundle(w2382) -> ("New Image"=w2381:T2, "New Image"=w2380:T2, "New Image"=w2379:T2, "New Image"=w2378:T2)
        n1606 = Unbundle By Name(w2484) -> ("Y"=w2436:dbl[])
        n1607 = Unbundle By Name(w2481) -> ("Y"=w2438:dbl[])
        n1608 = Unbundle By Name(w2480) -> ("Y"=w2443:dbl[])
        n1609 = call "downsample 1D array - double.vi"("Ave N"=w2434, "Array In"=w2436) -> ("Array Out"=w2435:dbl[])  [unwired: 1 out]
        n1610 = call "downsample 1D array - double.vi"("Ave N"=w2434, "Array In"=w2438) -> ("Array Out"=w2437:dbl[])  [unwired: 1 out]
        n1611 = call "downsample 1D array - double.vi"("Ave N"=w2434, "Array In"=w2443) -> ("Array Out"=w2442:dbl[])  [unwired: 1 out]
        n1612 = feedback #12(w2504) -> (w2505:dbl[])
        n1613 = Build Array (concatenate)(w2505, w2504) -> (w2486:dbl[])
        n1614 = feedback #13(w2409) -> (w2411:dbl[])
        n1615 = Build Array (concatenate)(w2411, w2409) -> (w2410:dbl[])
        n1616 = local read "Scan steps (MCL)"() -> (w2391:u64)
        n1617 = Select(t=w2504, s=w2408, f=w2486) -> (s? t:f=w2490:dbl[])
        n1618 = feedback-in #12(w2490) -> ()
        n1619 = Select(t=w2409, s=w2408, f=w2410) -> (s? t:f=w2392:dbl[])
        n1620 = feedback-in #13(w2392) -> ()
        n1621 = local read "Scan lines (y)"() -> (w2377:u64)
        n1622 = local read "N APD Samp/step"() -> (w2393:dbl)
        n1623 = feedback #14(w2435) -> (w2492:dbl[])
        n1624 = Build Array (concatenate)(w2492, w2435) -> (w2483:dbl[])
        n1625 = feedback #15(w2442) -> (w2502:dbl[])
        n1626 = Build Array (concatenate)(w2502, w2442) -> (w2501:dbl[])
        n1627 = feedback #16(w2437) -> (w2494:dbl[])
        n1628 = Build Array (concatenate)(w2494, w2437) -> (w2495:dbl[])
        n1629 = Select(t=w2435, s=w2408, f=w2483) -> (s? t:f=w2439:dbl[])
        n1630 = feedback-in #14(w2439) -> ()
        n1631 = Select(t=w2442, s=w2408, f=w2501) -> (s? t:f=w2441:dbl[])
        n1632 = feedback-in #15(w2441) -> ()
        n1633 = Select(t=w2437, s=w2408, f=w2495) -> (s? t:f=w2440:dbl[])
        n1634 = feedback-in #16(w2440) -> ()
        n1635 = Multiply(x=w2391, y=u64 2) -> (x*y=w2376:u64)
        n1636 = call "integrate 1D array interval - double.vi"("Ave N"=w2393, "Array In"=w2392) -> ("Array Out"=w2404:dbl[])  [unwired: 1 out]
        n1637 = call "integrate 1D array interval - double.vi"("Ave N"=w2393, "Array In"=w2490) -> ("Array Out"=w2489:dbl[])  [unwired: 1 out]
        n1638 = Array Size(array=w2404) -> (size(s)=w2405:i32)
        n1639 = Array Size(array=w2489) -> (size(s)=w2491:i32)
        n1640 = Multiply(x=w2377, y=w2376) -> (x*y=w2407:u64)
        n1641 = Multiply(x=w2377, y=w2376) -> (x*y=w2499:u64)
        n1642 = call-poly <vilib>:"Mean.vi"("X"=w2439) -> ("mean"=w2423:dbl)  [unwired: 1 out]
        n1643 = Subtract(x=w2407, y=w2405) -> (x-y=w2398:u64)
        n1644 = call-poly <vilib>:"Mean.vi"("X"=w2441) -> ("mean"=w2428:dbl)  [unwired: 1 out]
        n1645 = call-poly <vilib>:"Mean.vi"("X"=w2440) -> ("mean"=w2426:dbl)  [unwired: 1 out]
        n1646 = call-poly <vilib>:"Mean.vi"("X"=w2404) -> ("mean"=w2395:dbl)  [unwired: 1 out]
        n1647 = Subtract(x=w2499, y=w2491) -> (x-y=w2433:u64)
        n1648 = call-poly <vilib>:"Mean.vi"("X"=w2489) -> ("mean"=w2430:dbl)  [unwired: 1 out]
        n1649 = Initialize Array(1.0 ("element"), w2398) -> (w2394:dbl[])
        n1650 = Initialize Array(1.0 ("element"), w2433) -> (w2424:dbl[])
        n1651 = Multiply(x=w2394, y=w2395) -> (x*y=w2396:dbl[])
        n1652 = Multiply(x=w2424, y=w2426) -> (x*y=w2427:dbl[])
        n1653 = Multiply(x=w2424, y=w2428) -> (x*y=w2429:dbl[])
        n1654 = Multiply(x=w2424, y=w2423) -> (x*y=w2425:dbl[])
        n1655 = Multiply(x=w2424, y=w2430) -> (x*y=w2431:dbl[])
        n1656 = Build Array (concatenate)(w2439, w2425) -> (w2493:dbl[])
        n1657 = Build Array (concatenate)(w2441, w2429) -> (w2497:dbl[])
        n1658 = Build Array (concatenate)(w2440, w2427) -> (w2496:dbl[])
        n1659 = Build Array (concatenate)(w2404, w2396) -> (w2406:dbl[])
        n1660 = Build Array (concatenate)(w2489, w2431) -> (w2498:dbl[])
        n1661 = Reshape Array(w2493, w2377, w2376) -> (w2459:dbl[][])
        n1662 = Reshape Array(w2406, w2377, w2376) -> (w2402:dbl[][])
        n1663 = Reshape Array(w2497, w2377, w2376) -> (w2451:dbl[][])
        n1664 = Reshape Array(w2496, w2377, w2376) -> (w2466:dbl[][])
        n1665 = Reshape Array(w2498, w2377, w2376) -> (w2476:dbl[][])
        n1666 = Array Subset(array=w2466, index (col)=0 ("index"), length (col)=w2391) -> (w2471:dbl[][])  [unwired: 2 in]
        n1667 = Array Subset(array=w2466, index (col)=w2391) -> (w2469:dbl[][])  [unwired: 3 in]
        n1668 = Array Subset(array=w2451, index (col)=0 ("index"), length (col)=w2391) -> (w2457:dbl[][])  [unwired: 2 in]
        n1669 = Array Subset(array=w2451, index (col)=w2391) -> (w2455:dbl[][])  [unwired: 3 in]
        n1670 = Array Subset(array=w2402, index (col)=0 ("index"), length (col)=w2391) -> (w2401:dbl[][])  [unwired: 2 in]
        n1671 = Array Subset(array=w2402, index (col)=w2391) -> (w2399:dbl[][])  [unwired: 3 in]
        n1672 = Array Subset(array=w2476, index (col)=0 ("index"), length (col)=w2391) -> (w2475:dbl[][])  [unwired: 2 in]
        n1673 = Array Subset(array=w2476, index (col)=w2391) -> (w2473:dbl[][])  [unwired: 3 in]
        n1674 = Array Subset(array=w2459, index (col)=0 ("index"), length (col)=w2391) -> (w2464:dbl[][])  [unwired: 2 in]
        n1675 = Array Subset(array=w2459, index (col)=w2391) -> (w2462:dbl[][])  [unwired: 3 in]
        n1676 = for {
          tunnel: w2471 -> [w2513] mode=indexing
          tunnel: [w2512] -> w2470 mode=indexing
          workers-P: _ -> [_]
          n1677 = Reverse 1D Array(array=w2513) -> (reversed array=w2512:dbl[])
        }
        n1678 = for {
          tunnel: w2457 -> [w2509] mode=indexing
          tunnel: [w2508] -> w2456 mode=indexing
          workers-P: _ -> [_]
          n1679 = Reverse 1D Array(array=w2509) -> (reversed array=w2508:dbl[])
        }
        n1680 = for {
          tunnel: w2401 -> [w2507] mode=indexing
          tunnel: [w2506] -> w2400 mode=indexing
          workers-P: _ -> [_]
          n1681 = Reverse 1D Array(array=w2507) -> (reversed array=w2506:dbl[])
        }
        n1682 = for {
          tunnel: w2475 -> [w2515] mode=indexing
          tunnel: [w2514] -> w2474 mode=indexing
          workers-P: _ -> [_]
          n1683 = Reverse 1D Array(array=w2515) -> (reversed array=w2514:dbl[])
        }
        n1684 = for {
          tunnel: w2464 -> [w2511] mode=indexing
          tunnel: [w2510] -> w2463 mode=indexing
          workers-P: _ -> [_]
          n1685 = Reverse 1D Array(array=w2511) -> (reversed array=w2510:dbl[])
        }
        n1686 = Index Array(array=w2476, index (row)=0) -> (element=→"Waveform Graph":dbl[])  [unwired: 1 in]
        n1687 = Add(x=w2470, y=w2469) -> (x+y=w2468:dbl[][])
        n1688 = Add(x=w2456, y=w2455) -> (x+y=w2454:dbl[][])
        n1689 = Add(x=w2400, y=w2399) -> (x+y=w2384:dbl[][])
        n1690 = Add(x=w2474, y=w2473) -> (x+y=w2448:dbl[][])
        n1691 = Add(x=w2463, y=w2462) -> (x+y=w2461:dbl[][])
        n1692 = Divide(x=w2454, y=2) -> (x/y=w2452:dbl[][])
        n1693 = Divide(x=w2468, y=2) -> (x/y=w2413:dbl[][])
        n1694 = Divide(x=w2461, y=2) -> (x/y=w2415:dbl[][])
        n1695 = To Single Precision Float(number=w2448) -> (single precision float=w2447:sgl[][])
        n1696 = Transpose 2D Array(2D array=w2452) -> (transposed array=→"Data map":dbl[][])
        n1697 = To Single Precision Float(number=w2384) -> (single precision float=w2388:sgl[][])
        n1698 = To Single Precision Float(number=w2413) -> (single precision float=w2419:sgl[][])
        n1699 = To Single Precision Float(number=w2415) -> (single precision float=w2416:sgl[][])
        n1700 = call "IMAQ ArrayToImage"("Image Pixels (Float)"=w2447, "Image"=w2381) -> ("Image Out"=w2450:T2)  [unwired: 8 in, 1 out]
        n1701 = call "IMAQ ArrayToImage"("Image Pixels (Float)"=w2388, "Image"=w2380) -> ("Image Out"=w2390:T2)  [unwired: 8 in, 1 out]
        n1702 = call "IMAQ ArrayToImage"("Image Pixels (Float)"=w2419, "Image"=w2379) -> ("Image Out"=w2421:T2)  [unwired: 8 in, 1 out]
        n1703 = call "IMAQ ArrayToImage"("Image Pixels (Float)"=w2416, "Image"=w2378) -> ("Image Out"=w2418:T2)  [unwired: 8 in, 1 out]
        n1704 = call "IMAQ Symmetry"("Type of Symmetry"=w2449, "Image Src"=w2450) -> ("Image Dst Out"=w2445:T2)  [unwired: 3 in, 1 out]
        n1705 = call "IMAQ Symmetry"("Type of Symmetry"=w2389, "Image Src"=w2390) -> ("Image Dst Out"=w2386:T2)  [unwired: 3 in, 1 out]
        n1706 = call "IMAQ Symmetry"("Type of Symmetry"=w2420, "Image Src"=w2421) -> ("Image Dst Out"=→"Detection Laser X":T2)  [unwired: 3 in, 1 out]
        n1707 = call "IMAQ Symmetry"("Type of Symmetry"=w2417, "Image Src"=w2418) -> ("Image Dst Out"=→"Detection Laser Y":T2)  [unwired: 3 in, 1 out]
        n1708 = call "IMAQ Set Simple Calibration"("Calibration Axis Info"=T36 {"Origin Pixel"={"X"=0.0, "Y"=0.0}, "Angle Relative to Horizontal (deg)"=0.0, "Axis Reference"=0}, "Grid Descriptor"=T37 {"X Step"=0.3, "Y Step"=0.3, "Unit"=enum."Undefined"}, "Image"=w2445) -> ("Calibrated Image"=→"APD 1":T2)  [unwired: 7 in, 1 out]
        n1709 = call "IMAQ Set Simple Calibration"("Calibration Axis Info"=T36 {"Origin Pixel"={"X"=0.0, "Y"=0.0}, "Angle Relative to Horizontal (deg)"=0.0, "Axis Reference"=0}, "Grid Descriptor"=T37 {"X Step"=0.3, "Y Step"=0.3, "Unit"=enum."Undefined"}, "Image"=w2386) -> ("Calibrated Image"=→"APD 2":T2)  [unwired: 7 in, 1 out]
      }
    }
    n1710 = Subtract(x=w2016, y="APD 2 Offset") -> (x-y=w2013:waveform(dbl))
    n1711 = Subtract(x=w2018, y="APD 1 Offset") -> (x-y=w2014:waveform(dbl))
    n1712 = Index Array(array=w2033, index=3) -> (element=w2102:waveform(dbl))
    n1713 = Index Array(array=w2033, index=6) -> (element=w2099:waveform(dbl))
    n1714 = Build Array(w2014, w2013) -> (→"APD Chart":waveform(dbl)[])
    n1715 = Array Size(array=w2091) -> (size(s)=w2146:i32)
    n1716 = call <vilib>:"Std Deviation and Variance.vi"("X"=w2026) -> ("standard deviation"=w2025:dbl)  [unwired: 1 in, 2 out]
    n1717 = Add Array Elements(numeric array=w2026) -> (sum=w2028:u32)
    n1718 = Add Array Elements(numeric array=w2091) -> (sum=w2156:u32)
    n1719 = call <vilib>:"Std Deviation and Variance.vi"("X"=w2091) -> ("standard deviation"=w2090:dbl)  [unwired: 1 in, 2 out]
    n1720 = Divide(x="T1 offset_x (mV)", y=1000.0) -> (x/y=w2103:dbl)
    n1721 = Divide(x=w2025, y=w2024) -> (x/y=w2021:dbl)
    "Rate sigma (Hz) 2" <- w2021
    n1722 = Multiply(x=w2024, y=w2146) -> (x*y=w2027:dbl)
    "Int. Time (s)" <- w2027
    n1723 = Divide(x=w2028, y=w2027) -> (x/y=w2022:dbl)
    "APD 2 Rate (Hz)" <- w2022
    n1724 = Divide(x=w2156, y=w2027) -> (x/y=w2088:dbl)
    "APD 1 Rate (Hz)" <- w2088
    n1725 = Divide(x=w2090, y=w2024) -> (x/y=w2089:dbl)
    "Rate sigma (Hz)" <- w2089
    n1726 = Divide(x=w2021, y=w2022) -> (x/y=→"Sigma/Mean 2":dbl)
    n1727 = Divide(x=w2089, y=w2088) -> (x/y=→"Sigma/Mean":dbl)
    n1728 = Divide(x="T2 offset_x (mV)", y=1000.0) -> (x/y=w2101:dbl)
    n1729 = case shown="1" "Calibration" {
      tunnel: "T1 alpha_x (nm/V)" -> [_ w2344 w2365]
      tunnel: "T1 kappa_x (pN/nm)" -> [_ _ w2355]
      tunnel: "T2 alpha_x (nm/V)" -> [_ w2343 w2363]
      tunnel: "T2 kappa_x (pN/nm)" -> [_ _ w2356]
      tunnel: w2102 -> [w2326 w2341 w2361]
      tunnel: w2099 -> [w2325 w2339 w2359]
      tunnel: [w2326 w2338 w2358] -> w2132
      tunnel: [w2325 w2337 w2357] -> w2131
      tunnel: ["T1 X (V)" ("Label.Text") "T1 X (nm)" ("Label.Text") "T1 X (pN)" ("Label.Text")] -> w2120
      tunnel: ["T2 X (V)" ("Label.Text") "T2 X (nm)" ("Label.Text") "T2 X (pN)" ("Label.Text")] -> w2119
      tunnel: ["Position (V)" ("Label.Text") "Position (nm)" ("Label.Text") "Force (pN)" ("Label.Text")] -> w2121
      tunnel: w2101 -> [_ w2329 w2348]
      tunnel: w2103 -> [_ w2332 w2350]
      tunnel: ["Mean (V)" ("Label.Text") "Mean (nm)" ("Label.Text") "Mean (pN)" ("Label.Text")] -> w2116
      tunnel: ["Difference (V)" ("Label.Text") "Difference (nm)" ("Label.Text") "Difference (pN)" ("Label.Text")] -> w2041
      frame 0, Default {
      }
      frame 1 {
        # "position"
        n1730 = Unbundle By Name(w2341) -> ("Y"=w2345:dbl[])
        n1731 = Unbundle By Name(w2339) -> ("Y"=w2330:dbl[])
        n1732 = Subtract(x=w2345, y=w2332) -> (x-y=w2333:dbl[])
        n1733 = Subtract(x=w2330, y=w2329) -> (x-y=w2331:dbl[])
        n1734 = Multiply(x=w2331, y=w2343) -> (x*y=w2340:dbl[])
        n1735 = Multiply(x=w2344, y=w2333) -> (x*y=w2342:dbl[])
        n1736 = Bundle By Name(cluster=w2339, "Y"=w2340) -> (w2337:waveform(dbl))
        n1737 = Bundle By Name(cluster=w2341, "Y"=w2342) -> (w2338:waveform(dbl))
      }
      frame 2 {
        # "force"
        n1738 = Unbundle By Name(w2361) -> ("Y"=w2366:dbl[])
        n1739 = Unbundle By Name(w2359) -> ("Y"=w2364:dbl[])
        n1740 = Subtract(x=w2364, y=w2348) -> (x-y=w2349:dbl[])
        n1741 = Subtract(x=w2366, y=w2350) -> (x-y=w2351:dbl[])
        n1742 = Compound Arithmetic op=MULTIPLY(w2349, w2363, w2356) -> (w2360:dbl[])
        n1743 = Compound Arithmetic op=MULTIPLY(w2355, w2365, w2351) -> (w2362:dbl[])
        n1744 = Bundle By Name(cluster=w2359, "Y"=w2360) -> (w2357:waveform(dbl))
        n1745 = Bundle By Name(cluster=w2361, "Y"=w2362) -> (w2358:waveform(dbl))
      }
    }
    n1746 = feedback-in #17("Calibration") -> ()
    n1747 = feedback #17(u16 1 ("Calibration")) -> (w2123:u16)
    n1748 = Not Equal?(x=w2123, y="Calibration") -> (x != y?=w2079:bool)
    n1749 = Unbundle By Name(w2102) -> ("Y"=w2105:dbl[])
    n1750 = Unbundle By Name(w2099) -> ("Y"=w2108:dbl[])
    n1751 = Subtract(x=w2105, y=w2103) -> (x-y=w2106:dbl[])
    n1752 = Subtract(x=w2108, y=w2101) -> (x-y=w2107:dbl[])
    n1753 = disable-structure shown="Enabled" {
      disable-tunnel: [-1.0 ("y") 1.0] -> w2109
      frame Disabled {
      }
      frame Enabled {
      }
    }
    n1754 = Multiply(x=w2107, y="T2 alpha_x (nm/V)") -> (x*y=w2098:dbl[])
    n1755 = Multiply(x="T1 alpha_x (nm/V)", y=w2106) -> (x*y=w2097:dbl[])
    n1756 = Multiply(x=w2131, y=w2109) -> (x*y=w2110:waveform(dbl))
    n1757 = case shown="True" "Read Lateness and Rel Phase" {
      tunnel: w1933 -> [w2292 w2314]
      tunnel: w1932 -> [w2293 w2313]
      tunnel: [w2292 w2312] -> w2094
      tunnel: [w2293 w2311] -> w2093
      frame False {
      }
      frame True {
        n1758 = xnode "Read/Write Control"("FPGA VI Reference In"=w2314, "error in"=w2313) -> ("FPGA VI Reference Out"=w2312:T19, "error out"=w2311:errorcluster, "GI Relative phase"=→"GI relative phase":i16, "Relative phase"=→"Relative phase (AI1)":i16, "AI Late Counter"=→"Late Counter (AI1)":u16, "GI Late Counter"=→"GI Late Counter":u16, "MCL Late Counter"=→"MCL Late Counter":u16, "MCL Relative Phase"=→"Relative Phase (MCL)":i16, "APD Acq Relative Phase"=→"APD Acq Relative Phase":i16, "APD 1 Gate Relative Phase"=→"APD 1 Gate Relative Phase":i16, "APD 2 Gate Relative Phase"=→"APD 2 Gate Relative Phase":i16, "APD Acq Late Counter"=→"APD Acq Late Counter":u16, "APD 1 Gate Late Counter"=→"APD 1 Gate Late Counter":u16, "APD 2 Gate Late Counter"=→"APD 2 Gate Late Counter":u16, "Green FB Relative Phase"=→"Relative phase (Green FB)":i16, "GI Relative phase 2"=→"GI relative phase 2":i16, "GI Late Counter 2"=→"GI Late Counter 2":u16, "Trap Pos FIFO Timeout"=→"Trap Pos FIFO Timeout":u16, "Trap AI FIFO Timeout"=→"Trap AI FIFO Timeout":u16)
      }
    }
    n1759 = Subtract(x=w2098, y=w2097) -> (x-y=w2096:dbl[])
    n1760 = Unbundle By Name(w2131) -> ("Y"=w2066:dbl[])
    n1761 = Unbundle By Name(w2132) -> ("Y"=w2067:dbl[])
    n1762 = Build Array(w2132, w2110) -> (→"Force":waveform(dbl)[])
    n1763 = Subtract(x=w2096, y="Offset (nm)") -> (x-y=w2064:dbl[])
    n1764 = call-poly <vilib>:"Mean.vi"("X"=w2066) -> ("mean"=w2045:dbl)  [unwired: 1 out]
    "T2 X" <- w2045
    n1765 = Absolute Value(x=w2067) -> (abs(x)=w2068:dbl[])
    n1766 = Absolute Value(x=w2066) -> (abs(x)=w2069:dbl[])
    n1767 = call-poly <vilib>:"Mean.vi"("X"=w2067) -> ("mean"=w2046:dbl)  [unwired: 1 out]
    "T1 X" <- w2046
    n1768 = Add(x=w2068, y=w2069) -> (x+y=w2070:dbl[])
    n1769 = Bundle By Name(cluster=w2102, "Y"=w2064) -> (w2032:waveform(dbl))
    "Bead Separation" <- w2032
    n1770 = Divide(x=w2070, y=2.0) -> (x/y=→"Vec Mean of T1 T2":dbl[])
    n1771 = case shown="True" w2079 {
      tunnel: w2121 -> [_ w2319]
      tunnel: w2120 -> [_ w2318]
      tunnel: w2119 -> [_ w2317]
      tunnel: w2116 -> [_ w2316]
      tunnel: w2041 -> [_ w2315]
      frame False {
      }
      frame True {
        n1772 = property on="Force" class="WFChart (strict)"("YScale.NameLbl.Text"=w2319) -> ()  [unwired: 2 in, 2 out]
        n1773 = property on="T2 X" class="DigNum (strict)"("Caption.Text"=w2317) -> ()  [unwired: 2 in, 2 out]
        n1774 = property on="T1 X" class="DigNum (strict)"("Caption.Text"=w2318) -> ()  [unwired: 2 in, 2 out]
        n1775 = property on="Mean" class="DigNum (strict)"("Caption.Text"=w2316) -> ()  [unwired: 2 in, 2 out]
        n1776 = property on="Difference" class="DigNum (strict)"("Caption.Text"=w2315) -> ()  [unwired: 2 in, 2 out]
      }
    }
    n1777 = local read "Tether"() -> (w2073:bool)
    n1778 = Absolute Value(x=w2046) -> (abs(x)=w2043:dbl)
    n1779 = Absolute Value(x=w2045) -> (abs(x)=w2042:dbl)
    n1780 = Add(x=w2043, y=w2042) -> (x+y=w2118:dbl)
    n1781 = Subtract(x=w2043, y=w2042) -> (x-y=→"Difference":dbl)
    n1782 = feedback #18(w2064) -> (w2063:dbl[])
    n1783 = Divide(x=w2118, y=2.0) -> (x/y=w2072:dbl)
    "Mean" <- w2072
    n1784 = case shown="True" w2073 {
      tunnel: w2072 -> [_ w2251]
      frame False {
      }
      frame True {
        n1785 = Greater?(x="Lost Tether Alarm Threshold (pN)", y=w2251) -> (0:w2249:bool)
        n1786 = case shown="True" w2249 {
          frame False {
          }
          frame True {
            n1787 = flat-sequence {
              frame #0 {
                # "stop only if saving"
                n1788 = local read "Saving..."() -> (w2264:bool)
                n1789 = And(x=w2264, y="TA Cancel Save?") -> (x .and. y?=w2263:bool)
                n1790 = local write "Stop Saving"(w2263) -> ()
              }
              frame #1 {
                n1791 = case shown="True" "TA Green Off?" {
                  frame False {
                  }
                  frame True {
                    w2267 = FALSE ("Fl. Triggered...")
                    n1792 = local write "Fl. Triggered..."(w2267) -> ()
                    n1793 = property on="Green Laser ON/Interlacing" class="Bool (strict)"("Val(Sgnl)"=w2267) -> ()  [unwired: 2 in, 2 out]
                  }
                }
              }
            }
            n1794 = local read "Time tether formed"() -> (w2258:timestamp)
            n1795 = Get Date/Time In Seconds() -> (seconds since 1Jan1904=w2259:timestamp)
            n1796 = Subtract(x=w2259, y=w2258) -> (x-y=w2257:dbl)
            n1797 = Number To Decimal String(number=w2257) -> (decimal integer string=w2254:string)  [unwired: 1 out]
            n1798 = local read "Messages"() -> (w2261:string)
            n1799 = call <vilib>:"Beep.vi"() -> ()  [unwired: 3 in, 9 out]
            n1800 = Concatenate Strings("Lost tether (" ("Message to add"), w2254, " s)." ("string")) -> (w2256:string)
            n1801 = local write "Tether"(FALSE ("Tether")) -> ()
            n1802 = call "Update messages.vi"("Message to add"=w2256, "Old message string"=w2261) -> ("New message string"=w2260:string)
            n1803 = local write "Messages"(w2260) -> ()
            n1804 = property on="Trap Pos. FB ON" class="Bool (strict)"("Val(Sgnl)"=FALSE ("Value (Signaling)")) -> ()  [unwired: 2 in, 2 out]
          }
        }
      }
    }
    n1805 = Build Array (concatenate)(w2064, w2063) -> (w2062:dbl[])
    n1806 = Split 1D Array(array=w2062, index=w1944) -> (first subarray=w2058:dbl[])  [unwired: 1 out]
    n1807 = feedback-in #18(w2058) -> ()
    n1808 = call-poly <vilib>:"Mean.vi"("X"=w2058) -> ("mean"=w2057:dbl)  [unwired: 1 out]
    "Bead Mean (nm)" <- w2057
    n1809 = Subtract(x=w2058, y=w2057) -> (x-y=w2056:dbl[])
    n1810 = Square(x=w2056) -> (x^2=w2055:dbl[])
    n1811 = call-poly <vilib>:"Mean.vi"("X"=w2055) -> ("mean"=w2054:dbl)  [unwired: 1 out]
    n1812 = Square Root(x=w2054) -> (sqrt(x)=w2053:dbl)
    n1813 = Multiply(x=10.0, y=w2053) -> (x*y=→"RMS (Ang)":dbl)
    n1814 = xnode "Read/Write Control"("FPGA VI Reference In"=w2094, "error in"=w2093) -> ("FPGA VI Reference Out"=w2212:T19, "error out"=w2206:errorcluster, "AI2 Y Sum Set 1"=w2202:i16, "AI2 Y Sum Set 2"=w2201:i16, "AI1 X Set 1"=w1978:fxp<+/-,16,1>, "AI1 X Set 2"=w1977:fxp<+/-,16,1>, "Trap Pos FB Int Signal"=→"Trap Pos FB Int Signal":fxp<+/-,24,9>, "Trap Pos FB Int-Norm Signal"=→"Trap Pos FB Int-Norm Signal":fxp<+/-,16,1>, "Trap Pos FB Action"=w1971:i64, "Scanning"=→"AOD Scanning":bool, "Scan I"=→"AOD Scan I":u64, "Scanning MCL"=w2204:bool, "Scan I (MCL)"=→"MCL Scan I":u64, "Green FB Signals"=w2141:T47)  [unwired: 1 out]
    "MCL Scanning" <- w2204
    "Trap Pos FB Action" <- w1971
    n1815 = local read "AI2 (V)"() -> (w2203:cluster{"Set 1":dbl, "Set 2":dbl})
    n1816 = Bundle By Name(cluster=w2203, "Set 1"=w2202, "Set 2"=w2201) -> (w2199:cluster{"Set 1":dbl, "Set 2":dbl})
    n1817 = Divide(x=w1971, y=327.67) -> (x/y=→"Action (%)":dbl)
    n1818 = local read "Trap X (AI1)"() -> (w1991:T10)
    n1819 = Divide(x=w2199, y=3276.7) -> (x/y=w2198:cluster{"Set 1":dbl, "Set 2":dbl})
    n1820 = local write "AI2 (V)"(w2198) -> ()
    n1821 = Bundle(cluster=w1991, "Trap 1"=w1978, "Trap 2"=w1977) -> (→"Trap X (AI1)":T10)
    n1822 = Divide(x=w2141, y=3276.7) -> (x/y=w2137:T48)
    n1823 = Unbundle By Name(w2137) -> ("Green FB Ch 0"=w2140:dbl, "Green FB Ch 1"=w2139:dbl, "Green FB Ch 2"=w2138:dbl)
    n1824 = Divide(x=w2140, y=w2138) -> (x/y=w2136:dbl)
    n1825 = Divide(x=w2139, y=w2138) -> (x/y=w2135:dbl)
    n1826 = flat-sequence "To save data" {
      tunnel: [w3141] -> w2223
      tunnel: [w3142] -> w2222
      tunnel: w2172 -> [w3135]
      tunnel: w2060 -> [w3139]
      tunnel: ["Save Calibration"] -> w2195
      tunnel: w2192 -> [w3138]
      tunnel: [w3131] -> w2191
      tunnel: [w3128] -> w2190
      tunnel: [w3125] -> w2189
      tunnel: w2171 -> [w3127]
      tunnel: w2077 -> [w3121]
      tunnel: [w3121] -> w2076
      tunnel: ["Start Saving"] -> w2034
      tunnel: [w3115] -> w1960
      tunnel: [w3114] -> w1959
      tunnel: w2223 -> [w3376]
      tunnel: w2222 -> [w3375]
      tunnel: w1961 -> [w3374]
      tunnel: w2195 -> [w3373]
      tunnel: w2191 -> [w3371]
      tunnel: w2190 -> [w3370]
      tunnel: w2189 -> [w3369]
      tunnel: w2047 -> [w3368]
      tunnel: w2086 -> [w3367]
      tunnel: w2076 -> [w3366]
      tunnel: w2034 -> [w3365]
      tunnel: w2032 -> [w3364]
      tunnel: w2008 -> [w3363]
      tunnel: w1960 -> [w3362]
      tunnel: w1959 -> [w3361]
      tunnel: w1958 -> [w3360]
      frame #0 {
        n1827 = Or(x="Save N Sets", y="Start Saving") -> (x .or. y?=w3122:bool)
        n1828 = To Double Precision Float(number=w3138) -> (double precision float=w3132:dbl)
        n1829 = Build Array(w3122, "Save Calibration", w3135, w3127) -> (w3137:bool[])
        n1830 = Compound Arithmetic op=OR("Save Calibration", w3135, w3122, w3127) -> (w3140:bool)
        n1831 = Boolean Array To Number(Boolean array=w3137) -> (number=w3134:u32)
        n1832 = feedback #19(FALSE ("Save APD Data\nwith Trap Data")) -> (w3116:bool)
        n1833 = feedback #20(refnum<k0> refnum) -> (w3143:refnum<file>)
        n1834 = feedback #21(refnum<k0> refnum) -> (w3118:refnum<file>)
        n1835 = feedback #22(FALSE ("Save APD Data\nwith Trap Data")) -> (w3126:bool)
        n1836 = feedback #23(refnum<k0> refnum) -> (w3129:refnum<file>)
        n1837 = feedback #24(0) -> (w3145:i32)
        n1838 = feedback #25() -> (w3133:u32)  [unwired: 1 out]
        n1839 = case shown="True" w3140 {
          tunnel: [w3152 1] -> w3141
          tunnel: w3145 -> [w3154 _]
          tunnel: [w3153 w3172] -> w3142
          tunnel: w3143 -> [w3153 _]
          tunnel: w3139 -> [_ w3192]
          tunnel: w3132 -> [_ w3190]
          tunnel: w3134 -> [_ w3193]
          tunnel: [w3151 w3171] -> w3131
          tunnel: w3133 -> [w3151 _]
          tunnel: [w3150 w3169] -> w3128
          tunnel: w3129 -> [w3150 _]
          tunnel: [w3149 w3168] -> w3125
          tunnel: w3126 -> [w3149 _]
          tunnel: "Start Saving" -> [_ w3166]
          tunnel: w3121 -> [_ w3165]
          tunnel: [w3148 w3156] -> w3114
          tunnel: w3118 -> [w3148 _]
          tunnel: [w3147 w3155] -> w3115
          tunnel: w3116 -> [w3147 _]
          frame False {
            n1840 = Increment(x=w3154) -> (x+1=w3152:i32)
          }
          frame True {
            w3162 = FALSE ("Start Saving")
            w3167 = 9.0  # File Version
            w3175 = FALSE ("prepend array or string size? (T)")
            w3173 = T29."big-endian, network order" ("byte order (0:big-endian, network order)")
            # "write file headers"
            n1841 = local read "BD 1 Frequency 1 (MHz)"() -> (w3189:dbl)
            n1842 = local read "BD 2 Frequency 1 (MHz)"() -> (w3188:dbl)
            n1843 = local read "BD 1 Frequency 2 (MHz)"() -> (w3187:dbl)
            n1844 = local read "BD 2 Frequency 2 (MHz)"() -> (w3186:dbl)
            n1845 = local read "BD 1 Frequency 3 (MHz)"() -> (w3185:dbl)
            n1846 = local read "BD 2 Frequency 3 (MHz)"() -> (w3184:dbl)
            n1847 = Array Size(array=w3165) -> (size(s)=w3164:i32)
            n1848 = To Double Precision Float(number=w3164) -> (double precision float=w3163:dbl)
            n1849 = local write "Save Calibration"(w3162) -> ()
            n1850 = local write "Start Saving"(w3162) -> ()
            n1851 = Build Array("Save APD Data\nwith Trap Data", "Save Trap Pos. Data") -> (w3159:bool[])
            n1852 = Boolean Array To Number(Boolean array=w3159) -> (number=w3158:u32)
            n1853 = Build Array(w3189, w3188, w3187, w3186, w3185, w3184) -> (w3183:dbl[])
            n1854 = case shown="4" w3193 {
              tunnel: w3192 -> [w3264 w3284 w3300 w3338]
              tunnel: w3163 -> [w3269 w3291 w3320 w3357]
              tunnel: w3190 -> [w3268 w3290 w3319 w3356]
              tunnel: [w3265 w3286 w3311 w3348] -> w3181
              tunnel: [w3256 "Cal sets to save" w3301 w3339] -> w3171
              tunnel: w3183 -> [w3266 w3287 w3313 w3350]
              tunnel: "Save APD Data\nwith Trap Data" -> [w3263 _ w3297 w3336]
              tunnel: [w3263 w3278 w3297 w3336] -> w3168
              tunnel: w3167 -> [w3259 w3279 w3295 w3334]
              tunnel: w3166 -> [w3258 _ _ _]
              tunnel: [w3249 w3278 w3294 w3324] -> w3155
              tunnel: "Save Trap Pos. Data" -> [w3249 _ w3294 w3324]
              tunnel: w3158 -> [w3248 _ w3293 w3323]
              frame 1, Default {
                # "timeseries"
                n1855 = case shown="True" "Profile" {
                  tunnel: [w3272 w3275] -> w3253
                  tunnel: [w3272 w3274] -> w3252
                  tunnel: [w3272 w3273] -> w3251
                  tunnel: [w3272 w3277] -> w3250
                  frame False {
                    w3272 = 0.0 ("f")
                  }
                  frame True {
                    n1856 = local read "Current Position"() -> (w3276:dbl[])
                    n1857 = local read "Y change (mm)"() -> (w3277:dbl)
                    n1858 = call "subVI_explode3array.vi"("Array"=w3276) -> ("x"=w3275:dbl, "y"=w3274:dbl, "z"=w3273:dbl)  [unwired: 12 in]
                  }
                }
                n1859 = local read "Save ave N"() -> (w3271:dbl)
                n1860 = Multiply(x=w3271, y=w3264) -> (x*y=w3270:dbl)
                n1861 = To Double Precision Float(number=w3248) -> (double precision float=w3262:dbl)
                n1862 = Build Array(w3259, w3264, w3270, w3269, w3268, 0.0 ("f")) -> (w3267:dbl[])
                n1863 = Build Array(w3262, w3253, w3252, w3251, w3250) -> (w3260:dbl[])
                n1864 = Select(t=u32 4000000000, s=w3258, f="N sets to save") -> (s? t:f=w3256:u32)
                n1865 = Build Array (concatenate)(w3267, w3266, w3260) -> (w3265:dbl[])
              }
              frame 2 {
                w3281 = 0.0 ("f")
                w3278 = FALSE ("Save APD Data\nwith Trap Data")
                # "calibration"
                n1866 = Boolean To (0,1)(Boolean=w3278) -> (0, 1=w3283:i16)
                n1867 = To Double Precision Float(number=w3283) -> (double precision float=w3282:dbl)
                n1868 = Build Array(w3282, w3281, w3281, w3281, w3281) -> (w3280:dbl[])
                n1869 = Build Array(w3279, w3284, w3284, w3291, w3290, 1.0 ("t")) -> (w3288:dbl[])
                n1870 = Build Array (concatenate)(w3288, w3287, w3280) -> (w3286:dbl[])
                "Calibrating Trap..." <- TRUE ("Calibrating...")
              }
              frame 4 {
                w3298 = 0.0 ("f")
                # "write file header for a trap \nraster scan"
                # "scan dir (x/y = 0/1)"
                # "cycles/step"
                # "n scans (f/b)"
                # "steps"
                # "freq. range"
                # "AOD raster scan"
                n1871 = local read "Number of F/B Scans (AOD)"() -> (w3305:u16)
                n1872 = local read "Cycles/step (AOD)"() -> (w3307:u64)
                n1873 = local read "Scan Range (MHz)"() -> (w3310:dbl)
                n1874 = local read "Scan steps (AOD)"() -> (w3309:u64)
                n1875 = local read "Scan BD"() -> (w3317:bool)
                n1876 = local read "Save ave N"() -> (w3322:dbl)
                n1877 = Boolean To (0,1)(Boolean=w3317) -> (0, 1=w3316:i16)
                n1878 = To Double Precision Float(number=w3305) -> (double precision float=w3304:dbl)
                n1879 = To Double Precision Float(number=w3309) -> (double precision float=w3308:dbl)
                n1880 = To Double Precision Float(number=w3307) -> (double precision float=w3306:dbl)
                n1881 = To Double Precision Float(number=w3316) -> (double precision float=w3315:dbl)
                n1882 = Multiply(x=w3322, y=w3300) -> (x*y=w3321:dbl)
                n1883 = To Double Precision Float(number=w3293) -> (double precision float=w3299:dbl)
                n1884 = Build Array(w3299, w3298, w3298, w3298, w3298) -> (w3296:dbl[])
                n1885 = local read "N sets should be saved"() -> (w3302:dbl)
                n1886 = Build Array(w3315, w3310, w3308, w3306, w3304) -> (w3312:dbl[])
                n1887 = Build Array(w3295, w3300, w3321, w3320, w3319, 2.0 ("t")) -> (w3314:dbl[])
                n1888 = Round Toward +Infinity(x=w3302) -> (ceil(x): smallest int >= x=w3303:dbl)
                n1889 = Build Array (concatenate)(w3314, w3313, w3296, w3312) -> (w3311:dbl[])
                n1890 = To Unsigned Long Integer(number=w3303) -> (unsigned 32bit integer=w3301:u32)
              }
              frame 8 {
                w3331 = 0.0 ("f")
                # "MCL raster scan"
                n1891 = local read "Number of scans (MCL)"() -> (w3326:u64)
                n1892 = local read "Scan lines (y)"() -> (w3325:u64)
                n1893 = local read "2D or 1D Scan"() -> (w3328:bool)
                n1894 = local read "Scan Range (V)\n(of steps)"() -> (w3347:dbl)
                n1895 = local read "Fast Scan Dir"() -> (w3354:bool)
                n1896 = local read "Cycles/step (MCL)"() -> (w3344:u64)
                n1897 = local read "Scan steps (MCL)"() -> (w3346:u64)
                n1898 = Select(t=w3325, s=w3328, f=w3326) -> (s? t:f=w3327:u64)
                n1899 = Boolean To (0,1)(Boolean=w3328) -> (0, 1=w3330:i16)
                n1900 = local read "Save ave N"() -> (w3359:dbl)
                n1901 = local read "Initial X"() -> (w3333:dbl)
                n1902 = local read "Initial Y"() -> (w3332:dbl)
                n1903 = To Double Precision Float(number=w3330) -> (double precision float=w3329:dbl)
                n1904 = Boolean To (0,1)(Boolean=w3354) -> (0, 1=w3353:i16)
                n1905 = To Double Precision Float(number=w3327) -> (double precision float=w3342:dbl)
                n1906 = To Double Precision Float(number=w3346) -> (double precision float=w3345:dbl)
                n1907 = To Double Precision Float(number=w3344) -> (double precision float=w3343:dbl)
                n1908 = To Double Precision Float(number=w3353) -> (double precision float=w3352:dbl)
                n1909 = Multiply(x=w3359, y=w3338) -> (x*y=w3358:dbl)
                n1910 = To Double Precision Float(number=w3323) -> (double precision float=w3337:dbl)
                n1911 = local read "N sets should be saved (MCL)"() -> (w3340:dbl)
                n1912 = Build Array(w3337, w3329, w3331, w3331, w3331) -> (w3335:dbl[])
                n1913 = Build Array(w3352, w3347, w3345, w3343, w3342, w3333, w3332) -> (w3349:dbl[])
                n1914 = Build Array(w3334, w3338, w3358, w3357, w3356, 3.0 ("t")) -> (w3351:dbl[])
                n1915 = Round Toward +Infinity(x=w3340) -> (ceil(x): smallest int >= x=w3341:dbl)
                n1916 = Build Array (concatenate)(w3351, w3350, w3335, w3349) -> (w3348:dbl[])
                n1917 = To Unsigned Long Integer(number=w3341) -> (unsigned 32bit integer=w3339:u32)
              }
            }
            n1918 = local read "Index"() -> (w3198:dbl)
            n1919 = call "Create new save file.vi"("Insert"="", "Ext"=".dat", "Index In"=w3198) -> ("Path Out"=w3157:path, "Index Out"=w3170:dbl)
            n1920 = local write "Save file name"(w3157) -> ()
            n1921 = local write "Index"(w3170) -> ()
            n1922 = local write "Save index"(w3170) -> ()
            n1923 = Array Size(array=w3181) -> (size(s)=w3182:i32)
            n1924 = Open/Create/Replace File(file path (use dialog)=w3157, operation (0:open)=T23."create", access (0:read/write)=enum16{"read/write", "read-only", "write-only"}."write-only") -> (refnum out=w3195:refnum<file>)  [unwired: 1 in, 4 out]
            n1925 = local write "Saving..."(TRUE ("Saving...")) -> ()
            n1926 = To Double Precision Float(number=w3182) -> (double precision float=w3180:dbl)
            n1927 = String Length(string="Comment (data description)") -> (length=w3178:i32)
            n1928 = To Double Precision Float(number=w3178) -> (double precision float=w3177:dbl)
            n1929 = Deny Access(7:w3195) -> (3:w3194:refnum<file>)  [unwired: 1 in, 2 out]
            n1930 = Build Array (concatenate)(w3180, w3181, w3177) -> (w3179:dbl[])
            n1931 = case "If fluorescence data to be saved" shown="True" w3168 {
              tunnel: w3157 -> [_ w3247]
              tunnel: [refnum<k0> refnum w3227] -> w3169
              frame False {
              }
              frame True {
                w3226 = 0.0
                n1932 = local read "APD Integration Time (s)"() -> (w3232:dbl)
                n1933 = local read "N APD Samp/step"() -> (w3225:dbl)
                n1934 = Path To String(path=w3247) -> (string=w3246:string)
                n1935 = String Length(string=w3246) -> (length=w3245:i32)
                n1936 = Subtract(x=w3245, y=4) -> (x-y=w3243:i32)
                n1937 = String Subset(string=w3246, length (rest)=w3243) -> (substring=w3242:string)  [unwired: 1 out]
                n1938 = Build Array(w3232, w3225, w3226, w3226, w3226, w3226, w3226, w3226) -> (w3229:dbl[])
                n1939 = Concatenate Strings(w3242, "_fl.dat" ("string")) -> (w3240:string)
                n1940 = Array Size(array=w3229) -> (size(s)=w3231:i32)
                n1941 = String To Path(string=w3240) -> (path=w3236:path)
                n1942 = Open/Create/Replace File(file path (use dialog)=w3236, operation (0:open)=T23."create", access (0:read/write)=enum16{"read/write", "read-only", "write-only"}."write-only") -> (refnum out=w3237:refnum<file>)  [unwired: 1 in, 4 out]
                n1943 = Deny Access(7:w3237) -> (3:w3233:refnum<file>)  [unwired: 1 in, 2 out]
                n1944 = To Double Precision Float(number=w3231) -> (double precision float=w3230:dbl)
                n1945 = Build Array (concatenate)(w3230, w3229) -> (w3228:dbl[])
                n1946 = Write to Binary File(file (use dialog)=w3233, data=w3228, 5:FALSE ("prepend array or string size? (T)"), 9:T29."big-endian, network order" ("byte order (0:big-endian, network order)")) -> (refnum out=w3227:refnum<file>)  [unwired: 1 in, 3 out]
              }
            }
            n1947 = case shown="True" w3155 {
              tunnel: w3157 -> [_ w3209]
              tunnel: [refnum<k0> refnum w3208] -> w3156
              frame False {
              }
              frame True {
                w3204 = 0.0 ("element")
                n1948 = Path To String(path=w3209) -> (string=w3223:string)
                n1949 = Build Array(w3204, w3204, w3204, w3204, w3204, w3204, w3204, w3204) -> (w3205:dbl[])
                n1950 = String Length(string=w3223) -> (length=w3222:i32)
                n1951 = Subtract(x=w3222, y=4) -> (x-y=w3220:i32)
                n1952 = Array Size(array=w3205) -> (size(s)=w3207:i32)
                n1953 = String Subset(string=w3223, length (rest)=w3220) -> (substring=w3219:string)  [unwired: 1 out]
                n1954 = To Double Precision Float(number=w3207) -> (double precision float=w3206:dbl)
                n1955 = Concatenate Strings(w3219, "_pos.dat" ("string")) -> (w3217:string)
                n1956 = Build Array (concatenate)(w3206, w3205) -> (w3203:dbl[])
                n1957 = String To Path(string=w3217) -> (path=w3213:path)
                n1958 = Open/Create/Replace File(file path (use dialog)=w3213, operation (0:open)=T23."create", access (0:read/write)=enum16{"read/write", "read-only", "write-only"}."write-only") -> (refnum out=w3214:refnum<file>)  [unwired: 1 in, 4 out]
                n1959 = Deny Access(7:w3214) -> (3:w3210:refnum<file>)  [unwired: 1 in, 2 out]
                n1960 = Write to Binary File(file (use dialog)=w3210, data=w3203, 5:FALSE ("prepend array or string size? (T)"), 9:T29."big-endian, network order" ("byte order (0:big-endian, network order)")) -> (refnum out=w3208:refnum<file>)  [unwired: 1 in, 3 out]
              }
            }
            n1961 = Write to Binary File(file (use dialog)=w3194, data=w3179, 5:w3175, 9:w3173) -> (refnum out=w3176:refnum<file>)  [unwired: 1 in, 3 out]
            n1962 = Write to Binary File(file (use dialog)=w3176, data="Comment (data description)", 5:w3175, 9:w3173) -> (refnum out=w3172:refnum<file>)  [unwired: 1 in, 3 out]
          }
        }
        n1963 = feedback-in #19(w3115) -> ()
        n1964 = feedback-in #20(w3142) -> ()
        n1965 = feedback-in #21(w3114) -> ()
        n1966 = feedback-in #22(w3125) -> ()
        n1967 = feedback-in #23(w3128) -> ()
        n1968 = feedback-in #24(w3141) -> ()
        n1969 = feedback-in #25(w3131) -> ()
      }
      frame #1 {
        n1970 = local read "Saving..."() -> (w3372:bool)
        n1971 = case shown="True" w3372 {
          tunnel: w3376 -> [_ w3386]
          tunnel: w3375 -> [_ w3400]
          tunnel: w3374 -> [_ w3396]
          tunnel: w3373 -> [_ w3395]
          tunnel: w3371 -> [_ w3394]
          tunnel: w3370 -> [_ w3389]
          tunnel: w3369 -> [_ w3388]
          tunnel: w3368 -> [_ w3387]
          tunnel: w3367 -> [_ w3385]
          tunnel: w3366 -> [_ w3383]
          tunnel: w3365 -> [_ w3382]
          tunnel: w3364 -> [_ w3381]
          tunnel: w3363 -> [_ w3380]
          tunnel: w3362 -> [_ w3379]
          tunnel: w3361 -> [_ w3378]
          tunnel: w3360 -> [_ w3377]
          frame False {
          }
          frame True {
            n1972 = Multiply(x=w3386, y=w3385) -> (x*y=→"Time (s)":dbl)
            n1973 = Less Or Equal?(x=w3386, y=w3394) -> (x <= y?=w3398:bool)
            n1974 = Or(x="Stop Saving", y="Abort save 2") -> (x .or. y?=w3390:bool)
            n1975 = Not(x=w3390) -> (.not. x?=w3399:bool)
            n1976 = And(x=w3398, y=w3399) -> (x .and. y?=w3397:bool)
            n1977 = case shown="False" w3397 {
              tunnel: w3400 -> [w3407 w3475]
              tunnel: [0.0 w3478] -> w3393
              tunnel: w3386 -> [_ w3476]
              tunnel: w3394 -> [_ w3477]
              tunnel: w3396 -> [_ w3472]
              tunnel: w3395 -> [_ _]
              tunnel: w3389 -> [w3405 w3465]
              tunnel: w3388 -> [w3404 w3466]
              tunnel: w3387 -> [_ w3464]
              tunnel: w3383 -> [_ w3463]
              tunnel: w3382 -> [_ w3417]
              tunnel: w3381 -> [_ w3456]
              tunnel: w3380 -> [_ w3434]
              tunnel: w3379 -> [w3402 w3415]
              tunnel: w3378 -> [w3403 w3414]
              tunnel: w3377 -> [_ w3411]
              frame False {
                w3401 = FALSE
                n1978 = Close File(refnum=w3407) -> ()  [unwired: 1 in, 2 out]
                n1979 = case shown="True" w3404 {
                  tunnel: w3405 -> [_ w3409]
                  frame False {
                  }
                  frame True {
                    n1980 = Close File(refnum=w3409) -> ()  [unwired: 1 in, 2 out]
                  }
                }
                n1981 = case shown="True" w3402 {
                  tunnel: w3403 -> [_ w3408]
                  frame False {
                  }
                  frame True {
                    n1982 = Close File(refnum=w3408) -> ()  [unwired: 1 in, 2 out]
                  }
                }
                n1983 = local write "Calibrating Trap..."(w3401) -> ()
                n1984 = call <vilib>:"Beep.vi"() -> ()  [unwired: 3 in, 9 out]
                n1985 = local write "Stop Saving"(w3401) -> ()
                n1986 = property on="Raster Scanning..." class="Bool (strict)"("Val(Sgnl)"=w3401) -> ()  [unwired: 2 in, 2 out]
                "Saving..." <- w3401
              }
              frame True {
                n1987 = local read "Calibrating Trap..."() -> (w3467:bool)
                n1988 = case "Write fl. data" shown="True" w3466 {
                  tunnel: w3465 -> [_ w3501]
                  tunnel: w3464 -> [_ w3500]
                  frame False {
                  }
                  frame True {
                    n1989 = Write to Binary File(file (use dialog)=w3501, data=w3500, 5:FALSE ("prepend array or string size? (T)"), 9:T29."big-endian, network order" ("byte order (0:big-endian, network order)")) -> ()  [unwired: 1 in, 4 out]
                  }
                }
                n1990 = Greater?(x="Save ave N", y=1.0) -> (0:w3470:bool)
                n1991 = Not(x=w3467) -> (.not. x?=w3469:bool)
                n1992 = And(x=w3469, y=w3470) -> (x .and. y?=w3412:bool)
                n1993 = case shown="True" w3412 {
                  tunnel: w3411 -> [w3481 w3492]
                  tunnel: [w3481 w3484] -> w3410
                  tunnel: "Save ave N" -> [_ w3485]
                  frame False {
                  }
                  frame True {
                    w3482 = 2 ("dimension size")
                    n1994 = Array Size(array=w3492) -> (size(s)=w3486:i32)
                    n1995 = Divide(x=w3486, y=w3482) -> (x/y=w3490:dbl)
                    n1996 = Reshape Array(w3492, w3490, w3482) -> (w3491:u64[][])
                    n1997 = Transpose 2D Array(2D array=w3491) -> (transposed array=w3489:u64[][])
                    n1998 = for {
                      tunnel: w3489 -> [w3494] mode=indexing
                      tunnel: [w3493] -> w3483 mode=indexing
                      tunnel: w3485 -> [w3495]
                      workers-P: _ -> [_]
                      n1999 = call "downsample 1D array - U64.vi"("Ave N"=w3495, "Array In"=w3494) -> ("Array Out"=w3493:u64[])  [unwired: 1 in]
                    }
                    n2000 = Transpose 2D Array(2D array=w3483) -> (transposed array=w3488:u64[][])
                    n2001 = Divide(x=w3486, y=w3485) -> (x/y=w3487:dbl)
                    n2002 = Reshape Array(w3488, w3487) -> (w3484:u64[])
                  }
                }
                n2003 = case shown="True" w3412 {
                  tunnel: w3472 -> [w3504 w3516]
                  tunnel: [w3504 w3508] -> w3468
                  tunnel: "Save ave N" -> [_ w3509]
                  tunnel: w3463 -> [_ w3507]
                  frame False {
                    # "don't downsample data for trap calibration"
                  }
                  frame True {
                    n2004 = Array Size(array=w3516) -> (size(s)=w3510:i32)
                    n2005 = Array Size(array=w3507) -> (size(s)=w3506:i32)
                    n2006 = Divide(x=w3510, y=w3506) -> (x/y=w3514:dbl)
                    n2007 = Reshape Array(w3516, w3514, w3506) -> (w3515:i16[][])
                    n2008 = Transpose 2D Array(2D array=w3515) -> (transposed array=w3513:i16[][])
                    n2009 = for {
                      tunnel: w3513 -> [w3519] mode=indexing
                      tunnel: [w3518] -> w3505 mode=indexing
                      tunnel: w3509 -> [w3517]
                      workers-P: _ -> [_]
                      n2010 = call "downsample 1D array - I16.vi"("Ave N"=w3517, "Array In"=w3519) -> ("Array Out"=w3518:i16[])  [unwired: 1 out]
                    }
                    n2011 = Transpose 2D Array(2D array=w3505) -> (transposed array=w3512:i16[][])
                    n2012 = Divide(x=w3510, y=w3509) -> (x/y=w3511:dbl)
                    n2013 = Reshape Array(w3512, w3511) -> (w3508:i16[])
                  }
                }
                n2014 = Index Array(array=w3434, index=1) -> (element=w3437:waveform(dbl))
                n2015 = Index Array(array=w3434, index=0) -> (element=w3439:waveform(dbl))
                n2016 = Unbundle By Name(w3437) -> ("Y"=w3441:dbl[])
                n2017 = Unbundle By Name(w3439) -> ("Y"=w3449:dbl[])
                n2018 = case "Write trap pos. data" shown="True" w3415 {
                  tunnel: w3414 -> [_ w3497]
                  tunnel: w3410 -> [_ w3496]
                  frame False {
                  }
                  frame True {
                    n2019 = Write to Binary File(file (use dialog)=w3497, data=w3496, 5:FALSE ("prepend array or string size? (T)"), 9:T29."big-endian, network order" ("byte order (0:big-endian, network order)")) -> ()  [unwired: 1 in, 4 out]
                  }
                }
                n2020 = Write to Binary File(file (use dialog)=w3475, data=w3468, 5:FALSE ("prepend array or string size? (T)"), 9:T29."big-endian, network order" ("byte order (0:big-endian, network order)")) -> ()  [unwired: 1 in, 4 out]
                n2021 = feedback #26(w3441) -> (w3443:dbl[])
                n2022 = Build Array (concatenate)(w3443, w3441) -> (w3442:dbl[])
                n2023 = Select(t=w3441, s=w3417, f=w3442) -> (s? t:f=w3427:dbl[])
                n2024 = feedback-in #26(w3427) -> ()
                n2025 = feedback #27(w3449) -> (w3462:dbl[])
                n2026 = Build Array (concatenate)(w3462, w3449) -> (w3461:dbl[])
                n2027 = Select(t=w3449, s=w3417, f=w3461) -> (s? t:f=w3436:dbl[])
                n2028 = feedback-in #27(w3436) -> ()
                n2029 = Divide(x=w3476, y=w3477) -> (x/y=w3479:dbl)
                n2030 = Multiply(x=w3479, y=100.0) -> (x*y=w3478:dbl)
                n2031 = Build Array(w3436, w3427) -> (→"Saved APD":dbl[][])
                n2032 = Array Size(array=w3436) -> (size(s)=w3454:i32)
                n2033 = Unbundle By Name(w3456) -> ("Y"=w3460:dbl[])
                n2034 = Subtract(x=w3454, y="N pts to average") -> (x-y=w3430:i32)
                n2035 = Multiply(x="N pts to average", y=u16 2) -> (x*y=w3431:u16)
                n2036 = Subtract(x=w3454, y=w3431) -> (x-y=w3429:i32)
                n2037 = feedback #28(w3460) -> (w3459:dbl[])
                n2038 = Build Array (concatenate)(w3459, w3460) -> (w3458:dbl[])
                n2039 = Select(t=w3460, s=w3417, f=w3458) -> (s? t:f=w3457:dbl[])
                "Trap Delta Graph" <- w3457
                n2040 = feedback-in #28(w3457) -> ()
                n2041 = Array Subset(array=w3436, index=w3430, length="N pts to average") -> (w3453:dbl[])
                n2042 = Array Subset(array=w3436, index=w3429, length="N pts to average") -> (w3452:dbl[])
                n2043 = Array Subset(array=w3427, index=w3430, length="N pts to average") -> (w3433:dbl[])
                n2044 = Array Subset(array=w3427, index=w3429, length="N pts to average") -> (w3432:dbl[])
                n2045 = call-poly <vilib>:"Mean.vi"("X"=w3453) -> ("mean"=w3451:dbl)  [unwired: 1 out]
                n2046 = call-poly <vilib>:"Mean.vi"("X"=w3433) -> ("mean"=w3426:dbl)  [unwired: 1 out]
                n2047 = call-poly <vilib>:"Mean.vi"("X"=w3452) -> ("mean"=w3450:dbl)  [unwired: 1 out]
                n2048 = call-poly <vilib>:"Mean.vi"("X"=w3432) -> ("mean"=w3425:dbl)  [unwired: 1 out]
                n2049 = Subtract(x=w3426, y=w3425) -> (x-y=w3416:dbl)
                "Delta Fl. 2" <- w3416
                n2050 = Subtract(x=w3451, y=w3450) -> (x-y=w3448:dbl)
                "Delta Fl. 1" <- w3448
                n2051 = Initialize Array(w3448, 1 ("dimension size")) -> (w3445:dbl[])
                n2052 = Initialize Array(w3416, 1 ("dimension size")) -> (w3422:dbl[])
                n2053 = feedback #29(w3445) -> (w3446:dbl[])
                n2054 = Build Array (concatenate)(w3446, w3445) -> (w3444:dbl[])
                n2055 = feedback #30(w3422) -> (w3423:dbl[])
                n2056 = Build Array (concatenate)(w3423, w3422) -> (w3421:dbl[])
                n2057 = Select(t=w3445, s=w3417, f=w3444) -> (s? t:f=w3420:dbl[])
                n2058 = feedback-in #29(w3420) -> ()
                n2059 = Select(t=w3422, s=w3417, f=w3421) -> (s? t:f=w3419:dbl[])
                n2060 = feedback-in #30(w3419) -> ()
                n2061 = Build Array(w3420, w3419) -> (→"Save APD Deriv":dbl[][])
              }
            }
            "Progress" <- w3393
            "Progress 2" <- w3393
          }
        }
      }
    }
    n2062 = Bundle By Name(cluster=w2137, "Green FB Ch 0"=w2136, "Green FB Ch 1"=w2135) -> (w2115:T48)
    "Green FB Signals (V)" <- w2115
    n2063 = Unbundle By Name(w2115) -> ("Green FB Ch 2"=→"Green FB Plot":dbl)
    n2064 = local read "wait to reset values"() -> (w2207:bool)
    n2065 = Not(x=w2204) -> (.not. x?=w2208:bool)
    n2066 = And(x=w2208, y=w2207) -> (x .and. y?=w2209:bool)
    n2067 = case "Part of MCL raster scanning: returns to initial positions after scan done" shown="True" w2209 {
      tunnel: w2212 -> [w2945 w2952]
      tunnel: [w2945 w2951] -> w2211
      tunnel: w2206 -> [w2944 w2950]
      tunnel: [w2944 w2949] -> w2205
      frame False {
      }
      frame True {
        w2960 = 10.0 ("y")
        w2959 = 32767.0 ("y")
        # "to return scan values\nafter a synchronous \nAOM scan"
        n2068 = local read "AO2"() -> (w2953:dbl)
        n2069 = local read "AO1"() -> (w2954:dbl)
        n2070 = local write "wait to reset values"(FALSE ("wait to reset values")) -> ()
        n2071 = Multiply(x=w2954, y=w2959) -> (x*y=w2956:dbl)
        n2072 = Multiply(x=w2953, y=w2959) -> (x*y=w2958:dbl)
        n2073 = Divide(x=w2956, y=w2960) -> (x/y=w2955:dbl)
        n2074 = Divide(x=w2958, y=w2960) -> (x/y=w2957:dbl)
        n2075 = To Word Integer(number=w2955) -> (16bit integer=w2961:i16)
        n2076 = To Word Integer(number=w2957) -> (16bit integer=w2962:i16)
        n2077 = local read "Total Counts (ticks)"() -> (w2946:u32)
        n2078 = xnode "Read/Write Control"("FPGA VI Reference In"=w2952, "error in"=w2950, "AO1"=w2961, "AO2"=w2962, "MCL count"=w2946) -> ("FPGA VI Reference Out"=w2951:T19, "error out"=w2949:errorcluster)
        n2079 = local read "Scan Range (V)\n(of steps)"() -> (w2947:dbl)
        n2080 = property on="Scan Range (V)\n(of steps)" class="DigNum (strict)"("Val(Sgnl)"=w2947) -> ()  [unwired: 2 in, 2 out]
      }
    }
    n2081 = node-c288() -> ()  [unwired: 2 out]
  }
  n2082 = node-c288(3 ("Processor")) -> (w74:T24)  [unwired: 3 out]
  n2083 = timed-loop "Oscillate AOD (debugging)" {
    tunnel: w24 -> [w3521]
    tunnel: [w3520] -> w36
    timing: w74 -> [_]
    timing-out: [_] -> w73
    stop <- w3520 stop-if-true
    n2084 = node-c288() -> ()  [unwired: 2 out]
    n2085 = event shown="[0] \"Oscillate Set 2\", \"Fish for Tether\": Value Change" {
      selector: _ -> [_ _ _]
      dyn-events: _ -> [_ _ _]
      timeout: _ -> [_ _ _]
      tunnel: w3521 -> [w3528 _ _]
      tunnel: [FALSE ("Stop All") _ w3796] -> w3520
      event "Oscillate Set 2", "Fish for Tether": Value Change {
        n2086 = event-data() -> ()  [unwired: 6 out]
        n2087 = local read "Oscillate Set 2"() -> (w3527:bool)
        n2088 = Or(x=w3527, y="Fish for Tether") -> (x .or. y?=w3525:bool)
        n2089 = case shown="True" w3525 {
          tunnel: w3528 -> [_ w3531]
          tunnel: "Fish for Tether" -> [_ w3530]
          frame False {
          }
          frame True {
            n2090 = case shown="True" w3530 {
              frame False {
              }
              frame True {
                n2091 = local write "Scan axis 2"(TRUE) -> ()
                n2092 = local write "Tether"(FALSE ("Tether")) -> ()
              }
            }
            n2093 = node-c288("Period") -> (w3533:T24)  [unwired: 3 out]
            n2094 = timed-loop "Oscillate AOD" {
              timing: w3533 -> [_]
              timing-out: [_] -> w3532
              tunnel: w3531 -> [w3543]
              tunnel: w3530 -> [w3542]
              i -> [w3545]
              stop <- w3541 stop-if-true
              n2095 = node-c288() -> (w3544:i64)  [unwired: 1 out]
              n2096 = flat-sequence {
                tunnel: w3545 -> [w3571]
                tunnel: w3544 -> [w3570]
                tunnel: w3543 -> [w3554]
                tunnel: w3542 -> [w3556]
                tunnel: [w3556] -> w3540
                tunnel: [w3555] -> w3539
                tunnel: [w3553] -> w3538
                tunnel: [w3550] -> w3536
                tunnel: w3540 -> [w3607]
                tunnel: w3539 -> [w3605]
                tunnel: w3538 -> [w3604]
                tunnel: [w3603] -> w3537
                tunnel: w3536 -> [w3602]
                tunnel: [w3671] -> w3541
                tunnel: w3537 -> [w3669]
                frame #0 {
                  n2097 = Divide(x=w3570, y=i64 1000) -> (x/y=w3565:dbl)
                  n2098 = Multiply(x=w3565, y=w3571) -> (x*y=w3567:dbl)
                  n2099 = Multiply(x="Osc. freq. (Hz)", y=6.283185307179586) -> (x*y=w3568:dbl)
                  n2100 = Multiply(x=w3568, y=w3567) -> (x*y=w3552:dbl)
                  n2101 = local read "BD 1 Frequency 2 (MHz)"() -> (w3549:dbl)
                  n2102 = local read "BD 1 Frequency 1 (MHz)"() -> (w3546:dbl)
                  n2103 = case shown="True" w3556 {
                    tunnel: w3552 -> [w3577 w3584]
                    tunnel: w3549 -> [_ w3594]
                    tunnel: [w3574 w3578] -> w3557
                    tunnel: [FALSE w3587] -> w3553
                    tunnel: [0.0 w3580] -> w3550
                    tunnel: w3546 -> [_ w3579]
                    frame False {
                      n2104 = Sine(x=w3577) -> (sin(x)=w3575:dbl)
                      n2105 = Multiply(x=w3575, y="Osc. amp. (MHz)") -> (x*y=w3574:dbl)
                    }
                    frame True {
                      n2106 = Cosine(x=w3584) -> (cos(x)=w3597:dbl)
                      n2107 = Subtract(x=w3594, y=w3579) -> (x-y=w3593:dbl)
                      n2108 = Decrement(x=w3597) -> (x-1=w3596:dbl)
                      n2109 = Subtract(x=w3593, y="Closest Delta (MHz)") -> (x-y=w3590:dbl)
                      n2110 = Divide(x=w3596, y=2.0) -> (x/y=w3591:dbl)
                      n2111 = Multiply(x=w3591, y=w3590) -> (x*y=w3578:dbl)
                      n2112 = local read "Vec Mean of T1 T2"() -> (w3586:dbl[])
                      n2113 = Greater?(x=w3586, y="Stop F (pN)") -> (0:w3588:bool[])
                      n2114 = Or Array Elements(Boolean array=w3588) -> (logical OR=w3587:bool)
                      n2115 = Divide(x=w3584, y=6.283185307179586) -> (x/y=w3583:dbl)
                      n2116 = Round Toward +Infinity(x=w3583) -> (ceil(x): smallest int >= x=w3580:dbl)
                      "Attempts" <- w3580
                      n2117 = Greater?(x=w3580, y="Attempt Limit") -> (0:w3582:bool)
                      n2118 = case shown="True" w3582 {
                        frame False {
                        }
                        frame True {
                          n2119 = local write "Fish for Tether"(FALSE ("Fish for Tether")) -> ()
                          n2120 = call <vilib>:"Beep.vi"() -> ()  [unwired: 3 in, 9 out]
                          n2121 = local read "Messages"() -> (w3599:string)
                          n2122 = call "Update messages.vi"("Message to add"="Tether fishing timeout." ("Messages"), "Old message string"=w3599) -> ("New message string"=→"Messages":string)
                        }
                      }
                    }
                  }
                  n2123 = local read "Y RF Frequency Limits (MHz)"() -> (w3558:T16)
                  n2124 = local read "X RF Frequency Limits (MHz)"() -> (w3559:T16)
                  n2125 = local read "BD 1 Frequency 3 (MHz)"() -> (w3564:dbl)
                  n2126 = local read "BD 2 Frequency 2 (MHz)"() -> (w3548:dbl)
                  n2127 = Select(t=w3549, s="Scan axis 2", f=w3548) -> (s? t:f=w3560:dbl)
                  n2128 = Add(x=w3557, y=w3560) -> (x+y=w3555:dbl)
                  n2129 = Select(t=w3555, s="Scan axis 2", f=w3549) -> (s? t:f=w3547:dbl)
                  n2130 = Select(t=w3548, s="Scan axis 2", f=w3555) -> (s? t:f=w3562:dbl)
                  n2131 = local read "BD 2 Frequency 3 (MHz)"() -> (w3563:dbl)
                  n2132 = call "set RF board frequency - interlace.vi"("Board 2 Frequency Limits"=w3558, "Board 1 Frequency Limits"=w3559, "FPGA VI Reference In"=w3554, "Board 2 Frequency 3 (MHz)"=w3563, "Board 1 Frequency 3 (MHz)"=w3564, "Board 2 Frequency 2 (MHz)"=w3548, "Board 2 Frequency 1 (MHz)"=w3562, "Board 1 Frequency 2 (MHz)"=w3547, "Board 1 Frequency 1  (MHz)"=w3546) -> ()  [unwired: 1 in, 2 out]
                }
                frame #1 {
                  n2133 = And(x=w3607, y=w3604) -> (x .and. y?=w3606:bool)
                  n2134 = case "Only if were fishing and now formed tether" shown="True" w3606 {
                    tunnel: w3605 -> [w3609 w3621]
                    tunnel: [w3608 w3620] -> w3603
                    tunnel: w3602 -> [_ w3616]
                    frame False {
                      n2135 = local read "Fish for Tether"() -> (w3608:bool)
                      n2136 = case shown="True" w3608 {
                        tunnel: w3609 -> [_ _]
                        frame False {
                        }
                        frame True {
                        }
                      }
                    }
                    frame True {
                      w3620 = FALSE ("Fish for Tether")
                      n2137 = call <vilib>:"Beep.vi"() -> ()  [unwired: 3 in, 9 out]
                      n2138 = Number To Decimal String(number=w3616, width (-)=i16 1) -> (decimal integer string=w3614:string)
                      n2139 = case shown="\"2\", \"3\", \"4\", \"5\", \"6\"" "Then..." {
                        selector: "Then..." -> [_ w3624]
                        tunnel: w3621 -> [w3623 _]
                        frame "1", Default {
                          # "do nothing"
                          n2140 = property on="BD 1 Frequency 1 (MHz)" class="DigNum (strict)"("Val(Sgnl)"=w3623) -> ()  [unwired: 2 in, 2 out]
                        }
                        frame "2", "3", "4", "5", "6" {
                          n2141 = flat-sequence {
                            tunnel: w3624 -> [w3626]
                            frame #0 {
                              n2142 = property on="Trap Delta (MHz)" class="DigNum (strict)"("Val(Sgnl)"="Move to Delta 1 (MHz)") -> ()  [unwired: 2 in, 2 out]
                            }
                            frame #1 {
                              n2143 = case shown="\"5\", \"6\"" w3626 {
                                selector: w3626 -> [w3629 w3639 _]
                                frame "3", "4" {
                                n2144 = flat-sequence {
                                tunnel: w3629 -> [w3630]
                                tunnel: [w3630] -> w3627
                                tunnel: [w3632] -> w3628
                                tunnel: w3627 -> [w3632]
                                tunnel: w3628 -> [w3636]
                                frame #0 {
                                n2145 = property on="Green Laser ON/Interlacing" class="Bool (strict)"("Val(Sgnl)"=TRUE ("Value (Signaling)")) -> ()  [unwired: 2 in, 2 out]
                                }
                                frame #1 {
                                n2146 = Multiply(x="Wait Before Save (s)", y=u32 1000 ("x")) -> (x*y=w3634:u32)
                                n2147 = Wait (ms)(milliseconds to wait=w3634) -> ()  [unwired: 1 out]
                                }
                                frame #2 {
                                n2148 = property on="Start Saving" class="Bool (strict)"("Value"=TRUE ("Start Saving")) -> ()  [unwired: 2 in, 2 out]
                                n2149 = case shown="Default" w3636 {
                                frame Default {
                                }
                                frame "4" {
                                n2150 = property on="Fl. Triggered..." class="Bool (strict)"("Val(Sgnl)"=TRUE ("Value (Signaling)")) -> ()  [unwired: 2 in, 2 out]
                                }
                                }
                                }
                                }
                                }
                                frame "5", "6" {
                                n2151 = stacked-sequence {
                                tunnel: w3639 -> [_ _ _ _ _ _ _ _ w3656 _ _]
                                frame #0 {
                                n2152 = Replace Array Subset(array=u32[] [0] ("Index Values"), new element="Raster Set Upon Tether", index=0) -> (w3640:u32[])
                                n2153 = property on="Saved AOD Raster Scan Parameter Sets" class="Arr (strict)"("Index Values"=w3640) -> ()  [unwired: 2 in, 2 out]
                                }
                                frame #1 {
                                n2154 = Wait (ms)(milliseconds to wait=u32 500) -> ()  [unwired: 1 out]
                                }
                                frame #2 {
                                n2155 = property on="Load parameters" class="Bool (strict)"("Val(Sgnl)"=TRUE ("Value (Signaling)")) -> ()  [unwired: 2 in, 2 out]
                                }
                                frame #3 {
                                n2156 = Wait (ms)(milliseconds to wait=u32 500) -> ()  [unwired: 1 out]
                                }
                                frame #4 {
                                n2157 = property on="Trap Raster Scan" class="Bool (strict)"("Val(Sgnl)"=TRUE ("Value (Signaling)")) -> ()  [unwired: 2 in, 2 out]
                                }
                                frame #5 {
                                n2158 = Wait (ms)(milliseconds to wait=u32 2000) -> ()  [unwired: 1 out]
                                }
                                frame #6 {
                                n2159 = while {
                                stop <- w3651 stop-if-true
                                n2160 = local read "Raster Scanning..."() -> (w3650:bool)
                                n2161 = local read "Saving..."() -> (w3653:bool)
                                n2162 = Wait (ms)(milliseconds to wait=u32 100) -> ()  [unwired: 1 out]
                                n2163 = Not(x=w3653) -> (.not. x?=w3652:bool)
                                n2164 = Not(x=w3650) -> (.not. x?=w3649:bool)
                                n2165 = And(x=w3652, y=w3649) -> (x .and. y?=w3651:bool)
                                }
                                }
                                frame #7 {
                                n2166 = property on="Trap Delta (MHz)" class="DigNum (strict)"("Val(Sgnl)"="Move to Delta 2 (MHz)") -> ()  [unwired: 2 in, 2 out]
                                }
                                frame #8 {
                                n2167 = local read "Tether"() -> (w3657:bool)
                                n2168 = case shown="True" w3657 {
                                tunnel: w3656 -> [_ w3658]
                                frame False {
                                }
                                frame True {
                                n2169 = flat-sequence {
                                tunnel: w3658 -> [w3660]
                                frame #0 {
                                n2170 = Wait (ms)(milliseconds to wait=u32 500) -> ()  [unwired: 1 out]
                                }
                                frame #1 {
                                n2171 = case shown="\"6\"" w3660 {
                                frame Default {
                                }
                                frame "6" {
                                n2172 = property on="Green Laser ON/Interlacing" class="Bool (strict)"("Val(Sgnl)"=TRUE ("Green Laser ON/Interlacing")) -> ()  [unwired: 2 in, 2 out]
                                }
                                }
                                }
                                frame #2 {
                                n2173 = Wait (ms)(milliseconds to wait=u32 500) -> ()  [unwired: 1 out]
                                }
                                frame #3 {
                                n2174 = local write "Start Saving"("Save at end (5, 6)") -> ()
                                }
                                }
                                }
                                }
                                }
                                frame #9 {
                                n2175 = local read "Bead Sep. Int. Time (s)"() -> (w3666:dbl)
                                n2176 = Multiply(x=w3666, y=1000.0) -> (x*y=w3665:dbl)
                                n2177 = Wait (ms)(milliseconds to wait=w3665) -> ()  [unwired: 1 out]
                                }
                                frame #10 {
                                n2178 = property on="Rescale on Mean" class="Bool (strict)"("Val(Sgnl)"=TRUE ("Value (Signaling)")) -> ()  [unwired: 2 in, 2 out]
                                }
                                }
                                }
                                frame "2", Default {
                                }
                              }
                            }
                          }
                        }
                      }
                      n2179 = Concatenate Strings("Formed tether in ", w3614, " attempt(s)." ("string")) -> (w3611:string)
                      n2180 = local read "Messages"() -> (w3618:string)
                      n2181 = local write "Fish for Tether"(w3620) -> ()
                      n2182 = call "Update messages.vi"("Message to add"=w3611, "Old message string"=w3618) -> ("New message string"=w3617:string)
                      n2183 = local write "Messages"(w3617) -> ()
                      n2184 = Get Date/Time In Seconds() -> (seconds since 1Jan1904=→"Time tether formed":timestamp)
                      "Tether" <- "Tether Alarm?"
                    }
                  }
                }
                frame #2 {
                  n2185 = local read "Oscillate Set 2"() -> (w3670:bool)
                  n2186 = local read "Stop All"() -> (w3672:bool)
                  n2187 = Not Or(1:w3669, 2:w3670) -> (0:w3668:bool)
                  n2188 = Compound Arithmetic op=OR(w3672, w3668) -> (w3671:bool)
                }
              }
              n2189 = node-c288() -> ()  [unwired: 2 out]
            }
            n2190 = node-c288(w3532) -> ()  [unwired: 1 out]
          }
        }
      }
      event "Fl. Triggered...": Value Change {
        n2191 = event-data() -> ()  [unwired: 7 out]
        n2192 = case shown="True" "Fl. Triggered..." {
          frame False {
          }
          frame True {
            n2193 = node-c288() -> (w3684:T24)  [unwired: 4 out]
            n2194 = timed-loop {
              timing: w3684 -> [_]
              timing-out: [_] -> w3683
              tunnel: "Action" -> [w3688]
              shift-right: [w3685] -> _
              shift-left: u8 255 -> [w3687]
              stop <- w3689 stop-if-true
              n2195 = node-c288() -> ()  [unwired: 2 out]
              n2196 = flat-sequence {
                tunnel: w3688 -> [w3701]
                tunnel: w3687 -> [w3698]
                tunnel: [w3697] -> w3686
                tunnel: [w3787] -> w3689
                tunnel: w3686 -> [w3786]
                tunnel: [w3786] -> w3685
                frame #0 {
                  n2197 = local read "Delta Fl. 2"() -> (w3692:dbl)
                  n2198 = local read "Delta Fl. 1"() -> (w3693:dbl)
                  n2199 = Select(t=w3693, s="APD to Watch", f=w3692) -> (s? t:f=w3691:dbl)
                  n2200 = Multiply(x="Fl. Delta Thresh. (kHz)", y=1000.0) -> (x*y=w3700:dbl)
                  n2201 = Greater?(x=w3691, y=w3700) -> (0:w3695:bool)
                  n2202 = Or(x="Force Yank", y=w3695) -> (x .or. y?=w3696:bool)
                  n2203 = case shown="True" w3696 {
                    tunnel: w3701 -> [_ w3711]
                    tunnel: w3698 -> [w3703 w3707]
                    tunnel: [w3703 w3704] -> w3697
                    frame False {
                    }
                    frame True {
                      n2204 = flat-sequence {
                        tunnel: w3708 -> [w3717]
                        tunnel: [w3717] -> w3712
                        tunnel: w3711 -> [w3716]
                        tunnel: [w3716] -> w3710
                        tunnel: [w3715] -> w3709
                        tunnel: w3707 -> [w3714]
                        tunnel: [w3713] -> w3706
                        tunnel: w3712 -> [w3742]
                        tunnel: w3710 -> [w3741]
                        tunnel: w3709 -> [w3740]
                        tunnel: w3706 -> [w3739]
                        tunnel: [w3739] -> w3705
                        tunnel: w3705 -> [w3784]
                        tunnel: [w3784] -> w3704
                        frame #0 {
                          n2205 = call <vilib>:"Beep.vi"() -> ()  [unwired: 3 in, 9 out]
                          n2206 = local write "Waiting"(FALSE ("Waiting")) -> ()
                          n2207 = Increment(x=w3714) -> (x+1=w3713:u8)
                          n2208 = case shown="\"Yank\"" w3716 {
                            tunnel: w3713 -> [_ _ w3723]
                            frame "Image" {
                              n2209 = property on="Confocal Image" class="Bool (strict)"("Val(Sgnl)"=TRUE ("Value (Signaling)")) -> ()  [unwired: 2 in, 2 out]
                            }
                            frame "Alarm", Default {
                            }
                            frame "Yank" {
                              n2210 = flat-sequence {
                                tunnel: w3723 -> [w3726]
                                tunnel: [w3725] -> w3722
                                tunnel: ["N Array El"] -> w3721
                                tunnel: w3722 -> [w3736]
                                tunnel: w3721 -> [w3732]
                                frame #0 {
                                n2211 = Multiply(x="Yank Delay (s)", y=1000.0) -> (x*y=w3729:dbl)
                                n2212 = Quotient & Remainder(x=w3726, y="N Array El") -> (x-y*floor(x/y)=w3725:u8)  [unwired: 1 out]
                                n2213 = Wait (ms)(milliseconds to wait=w3729) -> ()  [unwired: 1 out]
                                }
                                frame #1 {
                                n2214 = Random Number (0-1)() -> (number: 0 to 1=w3733:dbl)
                                n2215 = Multiply(x=w3732, y=w3733) -> (x*y=w3731:dbl)
                                n2216 = Round Toward -Infinity(1:w3731) -> (0:w3730:dbl)
                                n2217 = Select(t=w3730, s="Random Choice", f=w3736) -> (s? t:f=w3734:dbl)
                                n2218 = Index Array(array="Yank to Delta Array (MHz)", index=w3734) -> (element=w3737:dbl)
                                n2219 = property on="Trap Delta (MHz)" class="DigNum (strict)"("Val(Sgnl)"=w3737) -> ()  [unwired: 2 in, 2 out]
                                }
                              }
                            }
                          }
                          n2220 = local read "Time (s)"() -> (w3715:dbl)
                          "Fl. High" <- TRUE ("Yanking")
                        }
                        frame #1 {
                          n2221 = node-c288() -> (w3744:T24)  [unwired: 4 out]
                          n2222 = timed-loop {
                            timing: w3744 -> [_]
                            timing-out: [_] -> w3743
                            tunnel: w3742 -> [w3760]
                            tunnel: w3741 -> [w3758]
                            tunnel: w3740 -> [w3757]
                            stop <- w3759 stop-if-true
                            n2223 = node-c288() -> ()  [unwired: 2 out]
                            n2224 = local read "Fl. Delta Thresh. (kHz)"() -> (w3752:dbl)
                            n2225 = local read "Fl. Triggered..."() -> (w3761:bool)
                            n2226 = local read "Delta Fl. 1"() -> (w3748:dbl)
                            n2227 = local read "Delta Fl. 2"() -> (w3746:dbl)
                            n2228 = local read "Stop All"() -> (w3755:bool)
                            n2229 = local read "APD to Watch"() -> (w3747:bool)
                            n2230 = Select(t=w3748, s=w3747, f=w3746) -> (s? t:f=w3745:dbl)
                            n2231 = Not(x=w3761) -> (.not. x?=w3756:bool)
                            n2232 = Multiply(x=w3752, y=1000.0) -> (x*y=w3751:dbl)
                            n2233 = Negate(x=w3751) -> (-x=w3750:dbl)
                            n2234 = Less?(x=w3745, y=w3750) -> (x < y?=w3754:bool)
                            n2235 = Compound Arithmetic op=OR(w3754, w3755, w3756, "Force Reset") -> (w3759:bool)
                            n2236 = case shown="True" w3759 {
                              tunnel: w3760 -> [_ w3772]
                              tunnel: w3758 -> [_ w3771]
                              tunnel: w3757 -> [_ w3769]
                              frame False {
                              }
                              frame True {
                                n2237 = case shown="\"Yank\"" w3771 {
                                tunnel: w3772 -> [_ w3773]
                                frame "Image", Default {
                                }
                                frame "Yank" {
                                n2238 = flat-sequence {
                                tunnel: [w3778] -> w3774
                                tunnel: w3773 -> [w3778]
                                tunnel: w3774 -> [w3779]
                                frame #0 {
                                n2239 = local read "Yank Delay (s)"() -> (w3777:dbl)
                                n2240 = Multiply(x=w3777, y=1000.0) -> (x*y=w3775:dbl)
                                n2241 = Wait (ms)(milliseconds to wait=w3775) -> ()  [unwired: 1 out]
                                }
                                frame #1 {
                                n2242 = property on="Trap Delta (MHz)" class="DigNum (strict)"("Val(Sgnl)"=w3779) -> ()  [unwired: 2 in, 2 out]
                                }
                                }
                                }
                                }
                                n2243 = local read "Time (s)"() -> (w3770:dbl)
                                n2244 = Subtract(x=w3770, y=w3769) -> (x-y=w3766:dbl)
                                "Duration (s)" <- w3766
                                n2245 = Number To Decimal String(number=w3766, width (-)=i16 0) -> (decimal integer string=w3764:string)
                                n2246 = Concatenate Strings(w3764, " s fluorescence event." ("string")) -> (w3762:string)
                                n2247 = local read "Messages"() -> (w3768:string)
                                n2248 = call "Update messages.vi"("Message to add"=w3762, "Old message string"=w3768) -> ("New message string"=w3767:string)
                                n2249 = call <vilib>:"Beep.vi"() -> ()  [unwired: 3 in, 9 out]
                                n2250 = local write "Messages"(w3767) -> ()
                              }
                            }
                            n2251 = node-c288() -> ()  [unwired: 2 out]
                          }
                          n2252 = node-c288(w3743) -> ()  [unwired: 1 out]
                        }
                        frame #2 {
                          n2253 = local write "Fl. High"(FALSE ("Yanking")) -> ()
                        }
                      }
                      n2254 = local read "Trap Delta (MHz)"() -> (w3708:dbl)
                    }
                  }
                }
                frame #1 {
                  n2255 = local read "Stop All"() -> (w3790:bool)
                  n2256 = local read "Fl. Triggered..."() -> (w3788:bool)
                  n2257 = Not(x=w3788) -> (.not. x?=w3789:bool)
                  n2258 = Or(x=w3789, y=w3790) -> (x .or. y?=w3787:bool)
                  n2259 = Not(x=w3787) -> (.not. x?=→"Waiting":bool)
                }
              }
              n2260 = node-c288() -> ()  [unwired: 2 out]
            }
            n2261 = node-c288(w3683) -> ()  [unwired: 1 out]
          }
        }
      }
      event "Stop All": Value Change {
        n2262 = event-data() -> ()  [unwired: 7 out]
        n2263 = local read "Stop All"() -> (w3796:bool)
      }
    }
    n2264 = node-c288() -> ()  [unwired: 2 out]
  }
  n2265 = node-c288(w14) -> ()  [unwired: 1 out]
  n2266 = node-c288(w68) -> ()  [unwired: 1 out]
  n2267 = node-c288(w75) -> ()  [unwired: 1 out]
  n2268 = node-c288(w73) -> ()  [unwired: 1 out]
  n2269 = node-c288(w163) -> ()  [unwired: 1 out]
  n2270 = flat-sequence {
    tunnel: w33 -> [w3801]
    tunnel: [w3800] -> w39
    tunnel: [w3797] -> w38
    tunnel: w37 -> [_]
    tunnel: w36 -> [_]
    tunnel: w35 -> [_]
    tunnel: w34 -> [_]
    tunnel: w32 -> [w3798]
    tunnel: w39 -> [w3804]
    tunnel: w38 -> [w3803]
    frame #0 {
      w3799 = FALSE ("APD to FIFO")
      n2271 = xnode "Read/Write Control"("FPGA VI Reference In"=w3801, "error in"=w3798, "APD to FIFO"=w3799, "AI to FIFO"=w3799) -> ("FPGA VI Reference Out"=w3800:T19, "error out"=w3797:errorcluster)
    }
    frame #1 {
      n2272 = xnode "Invoke Method"("FPGA VI Reference In"=w3804, "error in"=w3803) -> ("FPGA VI Reference Out"=w3802:T19)  [unwired: 1 out]
      n2273 = xnode "Close FPGA VI Reference"("FPGA VI Reference In"=w3802) -> ()  [unwired: 1 in, 1 out]
    }
  }
